vi "UNITEST MAIN v2.0.vi"() -> ()   [LabVIEW 2025]
uses:
  controls/LAB-IQ UI Data.ctl
  <vilib>/Platform/TimedLoop/XDataNode/timing_clust.ctl
  <vilib>/Platform/TimedLoop/XDataNode/nitl_modes.ctl
  <vilib>/Platform/TimedLoop/XDataNode/wakeup.ctl
  HEAVE vi's/Heave Write enum.ctl
  SWAY vi's/Sway Write enum.ctl
  SWAY vi's/Sway Right enum.ctl
  HEAVE vi's/Heave Right enum.ctl
  d081153b-36ca-4bc4-8478-749476f82ba4.vi
  1202965f-721d-4349-8d61-5de826f379ef.vi
  785ec975-e53d-4ed4-be48-2cc128d7a91f.vi
  02c5850b-52e8-4ed5-91f8-6f0ad62f4994.vi
  1223eb78-e4c4-4b69-bf80-185c82055158.vi
  e5651a45-6a49-4a3f-b503-ff1eaf449b4a.vi
  <vilib>/Utility/error.llb/Trim Whitespace One-Sided.vi
  support/Message Queue/Enqueue Message (Single).vi
  <vilib>/Utility/error.llb/Error Cluster From Error Code.vi
  <vilib>/Utility/file.llb/Read Delimited Spreadsheet (string).vi
  <vilib>/Utility/file.llb/Write Delimited Spreadsheet (string).vi
  <vilib>/ErrorRing/Error Ring.xnode
  <vilib>/platform/TimedLoop/XDataNode/XDataNode.xnode
  support/Message Queue/LAB-IQ Message Queue.lvlib
  support/User Event - Stop/LAB-IQ User Event - Stop.lvlib
  <vilib>/Platform/TimedLoop/XDataNode/XDNodeRunTimeDep.lvlib
panel:
  in  "DEPTH TRIP   ENABLE":bool
  in  "DEPTH TRIP VALUE":dbl
  in  "LOAD TRIP  ENABLE":bool
  in  "LOAD TRIP VALUE":dbl
  in  "CYCLIC COF TRIP  ENABLE":bool
  in  "CYCLIC FF TRIP  ENABLE":bool
  in  "FF TRIP  ENABLE":bool
  in  "COF TRIP  ENABLE":bool
  in  "CYCLIC CoF TRIP VALUE":dbl
  in  "CYCLIC FF TRIP VALUE":dbl
  in  "FF TRIP VALUE":dbl
  in  "COF TRIP VALUE":dbl
  in  "Dummy Run":bool
  in  "AutoTune":bool
  in  "reinit 3":bool=TRUE
  in  "output range delay":cluster{"output high":dbl, "output low":dbl}={"output high"=100.0, "output low"=-100.0} {"output low" format="%.2f"; "output high" format="%.2f"}
  in  "PID gains out delay":T1={"proportional gain (Kc)"=30.0, "integral time (Ti, min)"=0.00101, "derivative time (Td, min)"=0.0} {"derivative time (Td, min)" format="%.3f"; "integral time (Ti, min)" min=1e-05 max=100.0 step=0.0001 format="%.4f"; "proportional gain (Kc)" format="%.3f"}
  in  "PID gains out delay (microForce)":T1={"proportional gain (Kc)"=300.0, "integral time (Ti, min)"=0.00011, "derivative time (Td, min)"=0.0} {"derivative time (Td, min)" format="%.3f"; "integral time (Ti, min)" min=1e-05 max=100.0 step=1e-06 format="%.6f"; "proportional gain (Kc)" format="%.3f"}
  in  "Gain 2":dbl=0.016
  in  "Offset  3":dbl=1.5
  in  "Ramp MulFac":dbl=2.0
  out "actpid":dbl
  in  "pulses LoadDiffRamp(2..10)":dbl=9.0
  in  "PulseControlRamp(diff<=3N)":dbl=5.0 min=1.0 max=1000.0 step=1.0 format="%#.1f"
  in  "SetLoadDeadband(%) Load(0-10N)":dbl=0.1 min=0.0001 max=100.0 step=0.0001 format="%#.6f"
  in  "pulses LoadDiff(2..10)":dbl=10.0
  in  "pulses LoadDiff(11..50)":dbl=40.0
  in  "PulseControl(diff<=3N)":dbl=1.0 min=1.0 max=1000.0 step=1.0 format="%#.1f"
  out "SetLoadDeadband(%)  2":dbl=1.0 min=0.001 max=100.0 step=0.001 format="%#.6f"
  in  "pulsesSent":dbl=200.0
  out "pulses":dbl
  in  "pulses LoadDiff(21..1000)":dbl=40.0
  in  "Delay":dbl=1.5 min=0.001 max=5.0 step=0.001 format="%#.6f"
  in  "deadband":dbl=0.2
  in  "Checkbox 2":bool
  in  "Checkbox":bool=TRUE
  out "Scratch Start Recording":bool
  in  "SwaySpeed Set":bool
  in  "Update":bool
  in  "Analysis Home":bool
  in  "Installation/Replacement completed":bool
  in  "Loahead":bool
  in  "Heave and Surge COM Port:":refnum<visa-resource-name>="COM9"
  in  "Sway COM Port:":refnum<visa-resource-name>="COM10"
  out "Test Trip":bool
  out "Hymidity":bool
  in  "Humidity Disable trip":bool=TRUE
  in  "CoF Trip  2":dbl=540.0 min=100.0 max=540.0 step=1.0
  in  "File Path :  2":path
  out "Wear Track Diameter":dbl
  in  "Stribeck table":bool
  in  "seq":bool=TRUE
  out "Drive Error":string
  out "mm/s  Surge":dbl=7.0 caption="Jog" min=0.001 max=50.0 step=0.0001 format="%.2f"
  in  "Update Surge Speed":bool
  out "mm/s  Sway":dbl=7.0 caption="Jog" min=0.001 max=50.0 step=0.0001 format="%.2f"
  in  "Update Sway Speed":bool
  in  "Update Heave Speed":bool
  out "mm/s Heave":dbl=7.0 caption="Jog" min=0.001 max=30.0 step=0.0001 format="%.2f"
  in  "mm/sec":dbl=1.0 caption="Jog" min=0.001 max=50.0 step=0.001 format="%.2f"
  out "Scratch Start Test":bool
  in  "HomeScratch":bool
  in  "TEST SELECTION":enum32{"Time", "Cycle"}(radio)
  out "HEAVE ENABLE":bool
  in  "SPARE  5":u8
  in  "Manual Write SWAY":bool
  out "SWAY WRITE":string
  in  "SPARE  4":u8
  in  "SPARE  3":u8
  in  "SPARE 2":u8
  in  "SPARE 1":u8
  out "Spare 15":u8
  out "Spare 14":u8
  out "Spare 13":u8
  out "Spare 12":u8
  out "Spare 11":u8
  out "Spare 10":u8
  out "Spare 9":u8
  out "Spare 8":u8
  out "Spare 7":u8
  out "Spare 6":u8
  out "Spare 5":u8
  out "Spare 4":u8
  out "Spare 3":u8
  out "Spare 2":u8
  out "Spare 1":u8
  out "Node Id":u8
  out "Read SWAY Temp":bool
  out "fwMinor":u8
  out "fwMajor":u8
  out "faultCode":u16
  out "Rotary POSE":sgl format="%#.6f"
  out "SWAY POSE":sgl format="%#.6f"
  out "Homed":u8
  out "State":u8
  out "Ack ID":u16
  in  "SPEED":sgl=10000.0
  in  "Distance":sgl=10000.0
  in  "Mode Command":u8=2
  out "Sequence ID":u16
  out "error out Read SWAY":errorcluster
  out "error out Write  SWAY":errorcluster
  out "SWAY READ":string
  out "Start Test Temp":bool
  in  "AppLoadSeq scratch":bool
  in  "PID Delay (sec)":dbl=1.0 format="%#_6p"
  in  "Manual Write Heave & Surge":bool
  out "Heave and Surge Write":string
  in  "SPARE 4":u8
  in  "SPARE 3":u8
  in  "SPARE 2":u8
  in  "SPARE 1":u8
  out "Spare 15":u8
  out "Spare 14":u8
  out "Spare 13":u8
  out "Spare 12":u8
  out "Spare 11":u8
  out "Spare 10":u8
  out "Spare 9":u8
  out "Spare 8":u8
  out "Spare 7":u8
  out "Spare 6":u8
  out "Spare 5":u8
  out "Spare 4":u8
  out "Spare 3":u8
  out "Spare 2":u8
  out "Spare 1":u8
  out "Node Id":u8
  out "Read Heave Temp":bool
  out "fwMinor":u8
  out "fwMajor":u8
  out "faultCode":u16
  out "SURGE POSE":sgl format="%#.6f"
  out "HEAVE POSE":sgl format="%#.6f"
  out "Homed":u8
  out "State":u8
  out "Ack ID":u16
  in  "SPEED":sgl=10000.0
  in  "Distance":sgl=10000.0
  in  "Mode Command":u8=2
  out "Sequence ID":u16
  out "error out Read":errorcluster
  out "error out Write":errorcluster
  out "Heave and Surge Read":string
  out "Load Cell Temp":bool
  in  "Stop Scratch":bool
  in  "Enter Fixed SRR 2":dbl min=0.0 max=0.0 format="%.3f"
  in  "E.Velocity 2":bool=TRUE caption="SRR"
  in  "Tab Control 3":T2(tab)
  in  "Tab Control 5":enum32{""}(tab)
  in  "Tab Control 14":T3(tab)=enum."Motor Load"
  in  "Ramp":bool
  in  "apply load":bool
  in  "Enter ByPass Load":dbl
  in  "Bypass Load":bool
  out "gFF Rot 7":cluster{dbl, dbl, dbl}(graph)
  in  "Current Load":dbl
  in  "Set Load":dbl
  out "Current Position":dbl
  in  "Kp":dbl=1.0
  in  "Ki":dbl
  in  "Kd":dbl
  in  "Deadband":dbl=0.1
  in  "pct_scale":dbl=100.0
  in  "Init Step":dbl=10.0
  in  "Max Step Linit":dbl=10.0
  in  "i_limit":dbl=10.0
  in  "Min_pos_limit":dbl
  in  "Max_pos_limit":dbl=50000000.0
  in  "Fine Tune Zone":dbl=10.0
  in  "fine_tune_pct":dbl=100.0
  in  "min_deadband_floor":dbl=0.05
  in  "min_finetune_floor":dbl=0.15
  out "Pulse delta":dbl
  out "Vertical load (N)":dbl format="%#.3f"
  in  "Tab Control 26":enum32{"Page 1", "Page 2"}(tab)
  in  "ClearAll":bool
  out "Mz(Nm)":dbl[](array[numeric])
  out "My(Nm)":dbl[](array[numeric])
  out "Mx(Nm)":dbl[](array[numeric])
  in  "Save Dwell":dbl=0.015 caption="Save Dwell (sec)" min=0.0 max=5.0 step=0.001 format="%.3f"
  out "Mx":dbl[](graph)
  out "My":dbl[](graph)
  out "Mz":dbl[](graph)
  out "Fy(N)":dbl[](graph)
  out "Fz(N)":dbl[](graph)
  in  "ZeroAll":bool
  in  "Acq Delay (ms)":dbl=10.0
  in  "Burst Delay (ms)":dbl=10.0
  out "model":string
  out "SN":i32
  out "FFx(N)":dbl[](array[numeric])
  in  "Sensor IP":string="192.168.1.100"
  in  "Port":i32=8080
  out "FFy(N)":dbl[](array[numeric])
  out "Load(N)":dbl[](array[numeric])
  out "Fx(N)":dbl[](graph)
  out "AE":bool
  in  "delete Handle":bool
  in  "Create Handle":bool=TRUE
  out "ft_data":dbl[](array[numeric])=[1.0, 1.0, 1.0, 1.0, 1.0, 1.0]
  out "ft_range":dbl[](array[numeric])=[1.0, 1.0, 1.0, 1.0, 1.0, 1.0]
  in  "stop 6":bool
  out "running_flag":bool
  out "ft_udp_handle":i32
  out "get-data-return":i32
  out "get-range-return":i32
  out "zero-return":i32
  out "filter-return":i32
  out "initial-return":i32
  out "deleteHandle-result":i32
  in  "Tab Control 19":enum32{"Platform COM", "Config ", "DevInfo"}(tab)=enum."Config "
  in  "SAMPLES":dbl=100.0
  in  "Re-initilaize":bool
  in  "Filter ON/OFF":bool=TRUE
  in  "TracHomeSurgeOffsetCounts 10MM":dbl=505100.0
  in  "TracHomeSwayOffsetCounts 10MM":dbl=1432.0
  in  "Acoustic Emission:":dbl=1.0 min=0.0001 max=200.0 step=0.0001 format="%.4f"
  in  "Apply Filter (FF)":bool
  in  "Filter% 2":dbl=50.0 min=50.0 max=100.0 step=0.1 format="%.1f"
  in  "Apply Filter (Load)":bool=TRUE
  in  "Filter%":dbl=80.0 min=50.0 max=100.0 step=0.1 format="%.1f"
  in  "Sway distance (mm)":dbl=245.0
  in  "Surge distance (mm)":dbl=370.0
  in  "DataSavingLoopDelay(ms)":dbl=15.0
  in  "SAVE  2":bool
  in  "Enter Distance":bool caption="Enter Counts"
  in  "Sway Counts:":dbl=100.0 min=0.0 max=100000000.0 step=1.0 format="%.2f"
  in  "Distance (mm): 3":dbl=100.0 caption="Distance (mm):" min=0.0 max=1500.0 step=0.001 format="%.5f"
  in  "Surge Counts:":dbl=100.0 min=0.0 max=100000000.0 step=1.0 format="%.1f"
  in  "Distance (mm): 2":dbl=100.0 caption="Distance (mm):" min=0.0 max=1500.0 step=0.0001 format="%.3f"
  in  "Distance (mm):":dbl=100.0 min=0.0 max=1500.0 step=0.001 format="%.5f"
  in  "Heave Counts:":dbl=100.0 min=0.0 max=100000000.0 step=1.0
  in  "LRMHomeSurgeOffsetCounts":dbl=307197.0
  in  "LRMHomeSwayOffsetCounts":dbl=26880.0
  in  "TracHomeSurgeOffsetCounts 20MM":dbl=505100.0
  in  "TracHomeSwayOffsetCounts 20MM":dbl=1432.0
  in  "RotHomeSwayOffsetCounts":dbl=14656.0
  in  "RotHomeSurgeOffsetCounts":dbl=311465.0
  in  "Heave distance":dbl=340.0
  out "Zmm":dbl=1600.0
  out "Heave Pulses/mm":dbl=1600.0
  out "Surge Pulses/mm":dbl=1600.0
  out "Sway Pulses/mm":dbl=320.0
  in  "Heave Pitch":dbl=4.0
  in  "Surge Pitch":dbl=3.0
  in  "Sway Pitch":dbl=2.0
  in  "Heave PPR":dbl=6400.0
  in  "Surge PPR":dbl=6400.0
  in  "Sway PPR":dbl=6400.0
  in  "Heave Jog Speed":dbl=15.0
  in  "Surge Jog Speed":dbl=1.0 format="%.4f"
  in  "Heave PID Speed":dbl=15.0
  in  "Heave Loop Delay":dbl
  in  "Sway Jog Speed":dbl=1.0 format="%.4f"
  in  "Sway PID Speed":dbl=1.0 format="%.4f"
  in  "Sway Loop Delay":dbl
  in  "GUI":T4(tab)
  in  "Platform Settings":bool caption="Password"
  in  "Configure":bool caption="Password"
  in  "Home":bool caption="Password"
  in  "EXIT":bool
  in  "Analysis":bool caption="Password"
  in  "service 2":bool caption="Password"
  in  "MainPage":T5(tab)=enum."HOME"
  in  "Select Load Head":bool
  in  "Notes :":string
  in  "FILE":string
  in  "Sample ID :":string
  in  "Operator ID :":string
  in  "Operator Name :":string
  in  "Auto":bool caption="Power Status"
  in  "Disable Axis Jog Soft Limits m":bool
  out "Sway and Surge COM Status":bool=TRUE caption="Load COM Status"
  out "Heave COM Status":bool=TRUE caption="Load COM Status"
  in  "Enable Platform":bool
  in  "Surge Forward Main":bool
  in  "Surge Backward Main":bool
  in  "Sway Right Main":bool
  in  "Sway Left Main":bool
  in  "Heave Down Main":bool
  in  "Heave Up main":bool
  in  "mm":dbl=0.001 caption="Jog" min=1.0 max=100.0 step=0.01 format="%#.3f"
  in  "Surface Analysis":bool
  in  "Imaging":bool
  in  "Image Analysis":bool
  in  "Post Analysis":bool
  in  "SSP 0.75":bool
  in  "SSP 0.5":bool
  in  "SSP 0.3":bool
  in  "Warning":enum32{"Page 2"}(tab)
  in  "gui GIF":enum32{"Check", "Deca", "kilo", "Micro"}(tab)
  out "Communication is established":bool=TRUE caption="Load COM Status"
  in  "Reference Sample":u16(ring) items=["None", "Brass", "Aluminium", "Mild Steel"]
  out "Load Cell Communication Slide":u8(slide)=1 min=1 max=10 step=1 scale=0.0..10.0
  in  "com 3":bool
  out "com":bool
  out "DecaForce COM Status":bool caption="Load COM Status"
  in  "Loading Mode":u16(ring) items=["Constant", "Ramp", "Steps", "Indentation"]
  in  "Enter the CoF Trip":dbl=1.0
  in  "Enter the Friction Force Trip":dbl=520.0 min=500.0 max=500.0 step=1.0 format="%#.1f"
  in  "Enter the Normal load Trip":dbl=520.0 min=500.0 max=500.0 step=0.001 format="%.3f"
  in  "KiloForce":bool
  in  "DecaForce":bool
  in  "MicroForce":bool
  in  "LHBack":bool
  in  "LHNext":bool
  in  "Load Selection":T6(tab)
  in  "Enter the Load  (N)":dbl=2.0 caption="Enter the Load (N)" min=2.0 max=200.0 step=0.1 format="%#.4f"
  in  "Enter the Final Load (N)":dbl=1.0 min=0.0 max=500.0 step=1.0 format="%#.0f"
  in  "Enter the Loading Rate (N/min)":dbl=60.0 min=1.0 max=1200.0 step=0.1 format="%.2f"
  out "Warning 2":bool
  in  "Stribeck Table  For loading":string[][](table)
  in  "Clear 3":bool
  out "Message":string="Load Entered is out of range!!!"
  in  "Indentation":string[][](table)=[["Detection", "5", "2"], ["Unload", "0", "5"], ["Load", "10", "2"], ["Unload", "0", "5"], ["Detection", "5", "2"], ["Unload", "0", "5"]]
  in  "Multipoint":bool caption="Singlepoint"
  in  "AppLoad 4":bool
  in  "zNL":bool
  out "NL disp":dbl caption="Normal Load ( N )" min=-2000.0 max=2000.0 step=0.0001 format="%.1f"
  in  "Traction":bool
  in  "Surge Forward MM":bool
  in  "Surge Backward MM":bool
  in  "M3 Image":enum32{"Page 1", "Page 2"}(tab)
  in  "String 39":string="Jog heave to bring the upper sample closer to the lower sample within 1mm."
  in  "Sway Left MM":bool
  in  "Sway Right MM":bool
  in  "Disable Axis Jog Soft Limits":bool
  in  "mm":dbl=0.001 caption="Jog" min=0.001 max=5.0 step=0.0001 format="%#.3f"
  in  "Heave Down MM":bool
  in  "Heave Up MM":bool
  in  "Wear Track Diameter (mm)":dbl=30.0 caption="Wear Track Diameter (mm):" min=1.0 max=30.0 step=1.0 format="%.2f"
  in  "Set WTD":bool
  in  "HomeScratch":bool
  in  "HomeRot":bool
  in  "PlaceModule":bool
  in  "Motion Mode:":u16(ring) items=["Uniform Rotation", "Angular Oscillation", "Stribeck ", "Steps"]
  in  "LR Sway":bool
  in  "Rot Hor":bool
  in  "Rot Ver":bool
  in  "Scratch":bool
  in  "LR Cam":bool
  in  "MMBack":bool
  in  "MMNext":bool
  in  "Rotary Module Selection":T7(tab)
  in  "SPEED SELECTION :":enum32{"Speed in RPM", "Speed in m/sec"}(radio)=enum."Speed in m/sec"
  in  "Enter the Speed(mm/sec)":dbl=0.1 min=0.1 max=10.0 step=0.1 format="%.3f"
  in  "Enter the Speed (RPM)":dbl=45.0 min=1.0 max=3000.0 step=1.0
  in  "Enter the Frequency (Hz)":dbl=1.0 min=0.1 max=10.0 step=0.1 format="%.1f"
  in  "Enter the Angle (Deg)":dbl=45.0 min=5.0 max=300.0 step=1.0
  in  "Angular Oscillation Set":bool
  in  "Rotary Tab":enum32{"Page 1", "Page 2"}(tab)
  out "e.v/ssr 2":enum32{"E.V", "SSR"}(tab)
  in  "Enter the Final E.Velocity (m/s) 2":dbl=1.0 min=0.001 max=4.0 step=0.001 format="%.3f"
  in  "Enter initial E.Velocity (m/s) 2":dbl=2.0 min=0.001 max=4.0 step=0.001 format="%.3f"
  in  "Enter Fixed E.Velocity 2":dbl=1.0 min=0.001 max=2.0 step=0.001 format="%.3f"
  in  "Enter Final SRR 2":dbl=1.0 min=0.001 max=1.0 step=0.001 format="%.2f"
  in  "Enter initial SRR 2":dbl=1.0 min=0.001 max=1.0 step=0.001 format="%.2f"
  out "Final Speed (RPM) 3":dbl=1.0 min=0.1 max=3000.0 step=0.1 format="%.1f"
  out "Initial Speed (RPM) 2":dbl=100.0 min=0.1 max=3000.0 step=0.1 format="%.1f"
  in  "Enter the Final Velocity (m/s) 3":dbl=1.0 min=0.001 max=2.0 step=0.001 format="%.3f"
  in  "Enter initial Velocity (m/s)  3":dbl=2.0 min=0.001 max=2.0 step=0.001 format="%.3f"
  out "Ramp Up 2":bool caption="Ramp Down"
  in  "Import 2":bool
  in  "Save 2":bool
  in  "SPEED SELECTION : rotary":enum32{"Speed in Rpm", "Speed in m/sec"}(radio)=enum."Speed in m/sec"
  in  "calculate rotary":bool
  in  "String 45":string="File Path Location : C:-->LAB-IQ 150 --> User Defined\n                                       Protocol-->File.txt"
  in  "Step Speed":enum32{"Step Speed", "Step (load-Speed)"}(tab)
  in  "StepTable For Speed":string[][](table)
  in  "StepTable For Load-Speed":string[][](table)=[["", "", ""], ["", "", ""], ["", "", ""], ["", "", ""]]
  in  "StepTable For Speed 3":string[][](table)=[["", "", ""], ["", "", ""], ["", "", ""], ["", "", ""]]
  in  "Motion Direction:  3":u16(ring) items=["Clockwise", "Counter Clockwise"]
  in  "Enter Scratch length (mm):":dbl=1.0 min=1.0 max=50.0 step=0.0001 format="%.4f"
  in  "Enter Scratch Speed (mm/s):":dbl=1.0 min=0.003 max=10.0 step=0.0031 format="%.5f"
  in  "Scartch Offset":dbl=1.0 caption="Scratch Offset: (mm)" min=0.1 max=5.0 step=0.1 format="%.1f"
  in  "Motion type:":u16(ring) items=["Unidirection", "Bidirection"]
  in  "Scratch Mode":u16(ring) items=["Scratch", "Pre-Post Scan", "Multi Scratch"]
  in  "Rotary Speed Exced":string="Motor Speed Out of Range"
  in  "No of Scratch":dbl=1.0 min=1.0 max=50.0 step=0.0001
  out "Humidity  Status  3":bool caption="Communication Status"
  out "Low Temp  Status  2":bool=TRUE caption="Communication Status"
  out "TK4 status 2":bool=TRUE caption="Communication Status"
  in  "String 40":string="Before selecting Acoustic make sure the sensor output pin is connected to A4."
  in  "Stage Temperature":dbl[](array[numeric])=[150.0, 230.0, 300.0, 350.0, 400.0, 450.0, 500.0]
  in  "Sample Temperature":dbl[](array[numeric])=[100.0, 150.0, 200.0, 250.0, 300.0, 350.0, 400.0]
  in  "Humidity (Amb)":bool
  in  "Clear List":bool
  out "Sensors Picked":string
  in  "Add to list":bool
  in  "Wear":bool
  in  "Vibration":bool
  in  "Humidity (Chamber)":bool
  in  "Temperature (Chamber)":bool
  in  "ECR":bool
  in  "Temperature (Amb)":bool
  in  "Microphone":bool
  in  "Acoustic Emission 3":bool
  in  "SNext":bool
  in  "APBack":bool
  in  "Enter the Temperature (°C):":dbl
  in  "Enter the Stage \nTemperature (°C):":dbl=20.0 min=20.0 max=150.0 step=1.0 format="%#.0f"
  in  "Enter the Humidity (%Rh):":dbl=30.0 min=30.0 max=85.0 step=1.0
  in  "Low Temp":bool
  in  "High Temp":bool
  in  "Humidity":bool
  in  "Main Screen Tab":T8(tab)
  in  "ClrLog":bool
  out "Trip Log":string
  in  "Start Test":bool
  out "Test status":bool caption="Test Status"
  out "AR Led":bool caption="AR"
  out "Data":bool=TRUE
  out "Health":bool=TRUE
  out "Sway COM Status":bool=TRUE caption="Load COM Status"
  out "Heave COM Status":bool=TRUE caption="Load COM Status"
  in  "Grp Tab":enum32{"Rot/LRM", "FBT"}(tab)
  out "Depth Trip":dbl=600.0
  in  "Depth Trip":bool=TRUE
  out "Weart Deapth":bool
  in  "Depth Reset Graph":bool
  out "Weart":bool
  in  "Depthz":bool
  out "Depth (µm)":dbl min=-200.0 max=200.0 step=0.1 format="%.1f"
  out "WearGp":dbl(graph)=0.13298760003255525
  out "NL Trip 2":dbl=600.0
  out "Load pid":bool
  in  "Load Disable Trip":bool=TRUE
  in  "Load Reset Graph":bool
  out "NL Display 4":dbl caption="Normal Load ( N )" min=-2000.0 max=2000.0 step=0.0001 format="%.1f"
  out "Main Chart 3":cluster{dbl, "NL disp":dbl, dbl}(graph)
  in  "FF Tab":T9(tab)
  in  "COF Reset Graph":bool
  in  "COF Disable Trip":bool=TRUE
  out "COF TRIP":dbl=600.0
  out "Coefficient of Friction":dbl(graph)=0.13298760003255525
  in  "zFF":bool
  in  "FF Reset Graph":bool
  in  "FF Disable Trip":bool=TRUE
  out "FF TRIP":dbl=600.0
  out "Friction Force (N)":dbl min=-2000.0 max=2000.0 step=0.0001 format="%.3f"
  out "Friction Force (N) Graph":dbl(graph)=0.13298760003255525
  out "Cyclic FF TRIP":dbl=600.0
  in  "Cyclic FF Disable Trip":bool=TRUE
  in  "Cyclic FF Reset Graph":bool
  in  "CZ FF":bool
  out "Cyclic Friction Force (N) Graph":dbl(graph)=0.13298760003255525
  out "Cyclic Friction Force (N)":dbl min=-2000.0 max=2000.0 step=0.0001 format="%.3f"
  out "cyclic COF TRIP":dbl=600.0
  in  "cyclic COF Disable Trip":bool=TRUE
  in  "cyclic COF Reset Graph":bool
  out "Cyclic Coefficient of Friction":dbl(graph)=0.13298760003255525
  in  "Sub Graph":T10(tab)
  in  "Speed Tab":enum32{" Rotary Disc", "MTM Ball", "MTM Disc"}(tab)
  out "speed mm/sec":dbl(graph)=0.13298760003255525
  in  "Speed Reset Graph":bool
  out "MTM BALL SPEED":dbl(graph)=0.13298760003255525
  out "MTM DISC  SPEED":dbl(graph)=0.13298760003255525
  in  "Temperature Reset":bool
  out "Temperature (deg c)":dbl(graph)=0.13298760003255525
  in  "ECR RESET":bool
  out "ECR":dbl(graph)=0.13298760003255525
  out "Acoustic Emission (mV)":dbl min=0.0 max=5000.0 step=0.1
  in  "Aqucostic Reset Graph":bool
  out "gACQUOS":dbl(graph)=0.13298760003255525
  in  "Humidity Reset Graph":bool
  out "HumrGp":dbl(graph)=0.13298760003255525
  out "SD (mm)":dbl caption="Sliding Distance ( mm )" min=-200.0 max=200.0 step=0.1 format="%.4f"
  in  "Siliding distance Reset Graph":bool
  out "SDGp":dbl(graph)=0.13298760003255525
  in  "BACK":bool
  out "Ambient \nTemperature":dbl min=0.0 max=5000.0 step=0.1 format="%.1f"
  out "Ambient\n Humidity":dbl min=0.0 max=5000.0 step=0.1 format="%.2f"
  out "NL disp 2":dbl caption="Normal Load ( N )" min=-2000.0 max=2000.0 step=0.0001 format="%.1f"
  out "Set Humidity":dbl caption="Set Humidity  (% Rh)" min=-2000.0 max=2000.0 step=1.0 format="%.1f"
  out "humidity disp":dbl caption="Humidity (% Rh)" min=-2000.0 max=2000.0 step=1.0 format="%.1f"
  in  "Humidity On":bool
  in  "zNL 2":bool
  out "NLt":bool
  in  "Load En":bool
  out "Freq (Hz)":dbl min=0.0 max=5000.0 step=0.1 format="%.4f"
  out "HumCOMStatus":bool caption="Communication Status"
  out "Load Communication":bool
  in  "Temp Tabs":enum32{"Low Temp", "High Temp"}(tab)=enum."High Temp"
  out "Controller  Status":bool
  out "ChamberTemp":dbl format="%#.1f"
  in  "SetTmp":dbl=-190.0 caption="Set Temperature (Deg C)" min=-190.0 max=100.0 step=1.0 format="%.1f"
  in  "Cooling":bool
  in  "Heater":bool
  out "TK4 status":bool caption="Controller  Status"
  out "ChamberTemp":dbl format="%#.1f"
  in  "SetTmp":dbl caption="Set Temperature (Deg C)" min=0.0 max=1000.0 step=1.0 format="%.1f"
  in  "Set Load (N)":dbl=100.0 min=0.01 max=1500.0 step=0.01 format="%.1f"
  in  "Time Tab":enum32{"cycles", "duration"}(tab)=enum."duration"
  out "Test Duration 4":dbl=600.0 caption="Test Duration\n(HH:MM:SS)" min=0.0083 max=180000.0 step=0.0001 format="%<%H:%M:%S>t"
  out "TEST CYCLE":dbl min=0.0 max=5000.0 step=0.01 format="%.2f"
  in  "TOTAL CYCLES":dbl min=0.0 max=5000.0 step=0.1 format="%.4f"
  out "Time ( HH:MM:SS ) 2":dbl min=0.0 max=144000.0 step=1.0 format="%<%H:%M:%S>t"
  in  "Test Duration":dbl=600.0 caption="Test Duration\n(HH:MM:SS)" min=0.0083 max=180000.0 step=0.0001 format="%<%H:%M:%S>t"
  in  "Main Speed Tab":enum32{"ROTARY", "TRACTION"}(tab)
  in  "SPEED TAB":enum32{"RPM", "m/sec"}(tab)
  out "Speed (RPM)":dbl min=0.0 max=5000.0 step=0.1 format="%.1f"
  out "Set Speed":dbl caption="Set Speed (RPM)" min=0.0 max=1500.0 step=0.1 format="%.1f"
  out "Speed (m/sec)":dbl min=0.0 max=5000.0 step=0.001 format="%.4f"
  out "Set Speed (m/sec)":dbl min=0.0 max=1500.0 step=0.001 format="%.4f"
  in  "MTM MOTOR DISPLAY":enum32{"MTM RPM", "MTM m/sec"}(tab)
  out "Disc Speed (RPM)":dbl min=0.0 max=1500.0 step=0.1 format="%.1f"
  out "Ball Speed (RPM)":dbl min=0.0 max=1500.0 step=0.1 format="%.1f"
  out "Disc Speed (m/sec)":dbl min=0.0 max=1500.0 step=0.1 format="%.1f"
  out "Ball Speed (m/sec)":dbl min=0.0 max=1500.0 step=0.1 format="%.1f"
  in  "Angle and Frequency":enum32{"angular", "lrm"}(tab)
  out "Angle (Deg)":dbl min=0.0 max=5000.0 step=0.01 format="%.2f"
  out "Stroke (mm)":dbl min=0.0 max=5000.0 step=0.01 format="%.2f"
  in  "STOP":bool
  out "Multi Scratch Pass":dbl min=0.0 max=5000.0 step=0.1
  in  "X-AXIS":u16(ring) items=["None", "Time ( Sec )", "Normal Load ( N )", "Frictional Force ( N )", "Coefficient of Friction", "Depth ( Microns )", "Speed ( RPM )", "Frequency ( Hz )", "Angle ( Degree )", "Cyclic Friction Force ( N )", "Cyclic Co efficient Friction ", "Stage temperature ( Degree celcius )", "Sample temperature ( Degree celcius )", "Stroke Length ( mm )", "Scratch Speed ( mm/sec )", "Amb Humidity ( % Rh ) ", "Amb Temperature (Deg C)", "Acoustic (mV)", "Mx (Nm)", "My (Nm)", "Mz (Nm)", "Humidity ( % Rh )", "Sliding Distance (mm)", "Wear Track Diameter (mm)", "Fx(N)", "Fy(N)", "MTM BallSpeed (RPM)", "MTM DiscSpeed (RPM)", "Entrainment Speed", "Slide Role", "Slip(%)", "Rotary Speed (m/sec)", "MTM Ball Speed (m/sec)", "MTM Disc Speed (m/sec)", "ECR (ohms)"]
  in  "Y-AXIS":u16(ring) items=["None", "Time ( Sec )", "Normal Load ( N )", "Frictional Force ( N )", "Coefficient of Friction", "Depth ( Microns )", "Speed ( RPM )", "Frequency ( Hz )", "Angle ( Degree )", "Cyclic Friction Force ( N )", "Cyclic Co efficient Friction ", "Stage temperature ( Degree celcius )", "Sample temperature ( Degree celcius )", "Stroke Length ( mm )", "Scratch Speed ( mm/sec )", "Amb Humidity ( % Rh ) ", "Amb Temperature (Deg C)", "Acoustic (mV)", "Mx (Nm)", "My (Nm)", "Mz (Nm)", "Humidity ( % Rh )", "Sliding Distance (mm)", "Wear Track Diameter (mm)", "Fx(N)", "Fy(N)", "MTM BallSpeed (RPM)", "MTM DiscSpeed (RPM)", "Entrainment Speed", "Slide Role", "Slip(%)", "Rotary Speed (m/sec)", "MTM Ball Speed (m/sec)", "MTM Disc Speed (m/sec)", "ECR (ohms)"]
  out "XY Graph":cluster{"Array 2":dbl[], "Array 2":dbl[]}[](graph) caption="XY Graph 20"
  out "VARIANCE":dbl=-0.0 format="%0.2f"
  out "SD":dbl=-0.0 format="%.3f"
  out "MEAN":dbl format="%.3f"
  out "VARIANCE":dbl=-0.0 format="%0.2f"
  out "SD":dbl=-0.0 format="%.3f"
  out "MEAN":dbl format="%.3f"
  out "VARIANCE":dbl=-0.0 format="%0.2f"
  out "SD":dbl=-0.0 format="%.3f"
  out "MEAN":dbl format="%.3f"
  out "VARIANCE":dbl=-0.0 format="%0.2f"
  out "SD":dbl=-0.0 format="%.3f"
  out "MEAN":dbl format="%.3f"
  in  "Analysis Home new":bool
  out "File 2 Discription":string="\r"
  out "File 1 Discription":string="\r"
  in  "OPEN 1":bool
  in  "OPEN 2":bool
  out "File Name 1":string
  out "File Name 2":string
  in  "Refresh 2":bool
  in  "OPEN 3":bool
  out "File Name 3":string
  out "File Name 4":string
  in  "OPEN 4":bool
  out "File 4 Discription":string="\r"
  out "File 3 Discription":string="\r"
  in  "File Format":u16(ring) items=["csv", "txt", "duf"]
  in  "Export":bool
  in  "Report":bool
  in  "Password":string
  in  "Home Service":bool
  in  "Advanced Setting":bool
  in  "About Tab":enum32{"Primary"}(tab)
  in  "ECR Port:":refnum<visa-resource-name>="COM10"
  in  "Ramp Port:":refnum<visa-resource-name>="COM10"
  in  "Temp Modbus:":refnum<visa-resource-name>="COM14"
  in  "Humidity Port:":refnum<visa-resource-name>="COM10"
  in  "Edit Gain Constants":bool
  in  "Save Gain Constants":bool
  in  "Service About":bool
  # "SET JOG SPEED"
  # "Speed Exceed the limit of the Motor"
  # "Motor Speed Out of Range"
  # "NOTE: This operation needs to be done only when the machine is ON."
  # "load Aquisition off"
  # "load Aquisition On"
  # "Configuration"
  # "Limits for Heave Surge and Sway"
  # "Modules Offset Parameters"
  # "Counts-Distance Calculator"
  # "File Name :"
  # "Ensure the traction module is aligned\n horizontally with the stage before ENABLE."
  # "JOG MODE"
  # "Module Selection"
  # "Positioning Control"
  # "Connect the controller\ncable to M3"
  # "Environment"
  # "Sensors"
  # "Data Points"
  # "Data Points"
  # "Data Points"
  # "Data Points"
  # "ohms"
  # "Data Points"
  # "Data Points"
  # "Data Points"
  # "LAB-IQ 150 / UNITEST / WO2456 / UT150  v05 / AUGUST 2025"
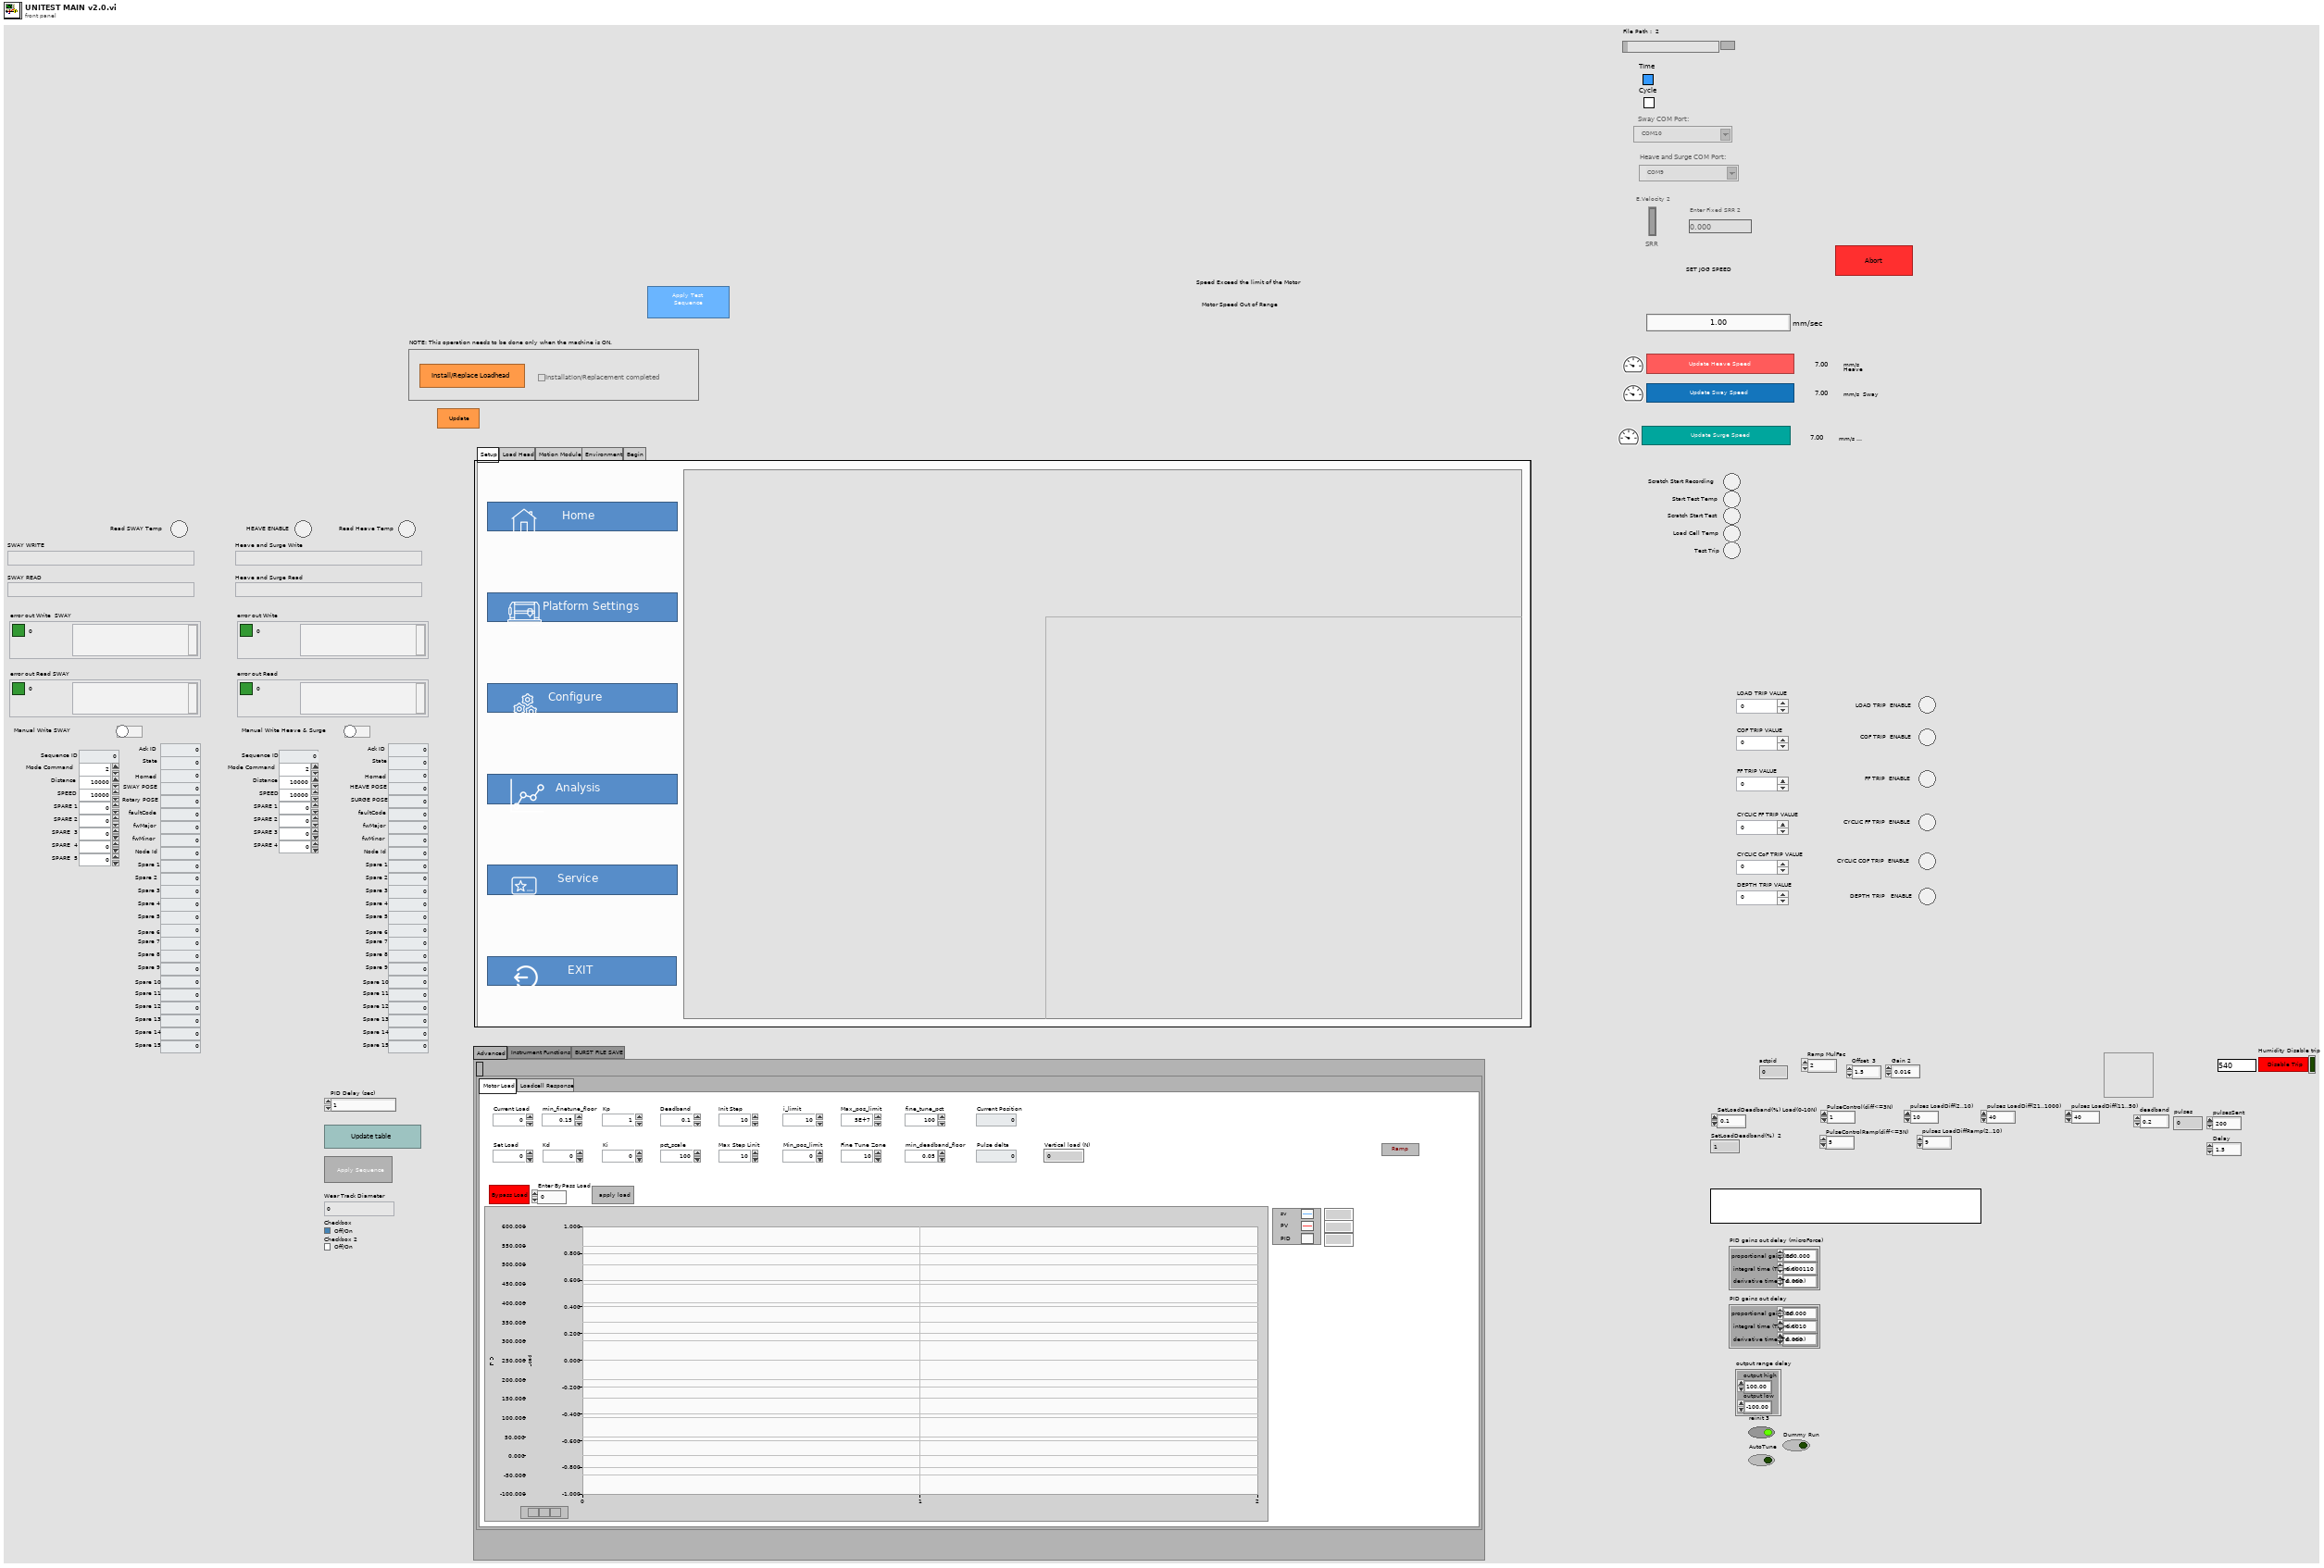
[diagram p1: front panel]
types:
  T1 = cluster{"proportional gain (Kc)":dbl, "integral time (Ti, min)":dbl, "derivative time (Td, min)":dbl}
  T2 = enum32{"Advanced", "Motor", "Depth_graph", "UIO Communicator", "Add to list parametrs", "Instrument Functions", "BURST FILE SAVE"}
  T3 = enum32{"LRM heating", "FBT_Heating", "Motor Load", "Loadcell Response", "Voice Load", "Step loading and speed ", "Depth"}
  T4 = enum32{"Setup", "Load Head", "Motion Module", "Environment", "Begin"}
  T5 = enum32{"Details", "PlatformSetting", "Analysis", "HOME"}
  T6 = enum32{"Constant", "Ramp", "Step", "Indentation"}
  T7 = enum32{"Uniform Rotation", "Angular Oscillation", "Speed Ramp", "Speed Step"}
  T8 = enum32{"  Acquire  ", "Compare Files Rot", "About", "Service"}
  T9 = enum32{"Coefficient of Friction ", "Friction Force (N)", "Cyclic Friction Force (N)", "Cyclic Coefficient of Friction "}
  T10 = enum32{"Speed", "Temperature", "ECR", "Acoustic Emission", "Humidity", "Sliding Distance"}
  T11 = typedef "LAB-IQ UI Data.ctl" = cluster{"Main Home Screen":cluster{"GUI":refnum<vi>, "Platform Settings":refnum<vi>, "Configure":refnum<vi>, "Home":refnum<vi>, "EXIT":refnum<vi>, "service 2":refnum<vi>, "MainPage":refnum<vi>, "Analysis":refnum<vi>}, "Platform Settings":cluster{"mm/s  Surge":refnum<vi>, "Update Surge Speed":refnum<vi>, "Drive Error":refnum<vi>, "Disable Axis Jog Soft Limits":refnum<vi>, "mm/s  Sway":refnum<vi>, "Sway and Surge COM Status":refnum<vi>, "Heave COM Status":refnum<vi>, "Enable Platform":refnum<vi>, "Surge Forward Main":refnum<vi>, "Sway Right Main":refnum<vi>, "Sway Left Main":refnum<vi>, "Heave Down Main":refnum<vi>, "Heave Up main":refnum<vi>, "Update Sway Speed":refnum<vi>, "Update Heave Speed":refnum<vi>, "mm/s Heave":refnum<vi>, "mm/sec":refnum<vi>, "mm":refnum<vi>, "Surge Backward Main":refnum<vi>}, "Analysis Screen":cluster{"Analysis Home":refnum<vi>, "Surface Analysis":refnum<vi>, "Imaging":refnum<vi>, "Image Analysis":refnum<vi>, "Post Analysis":refnum<vi>}, "Config Screen":cluster{"Select Load Head":refnum<vi>, "Notes :":refnum<vi>, "FILE":refnum<vi>, "Sample ID :":refnum<vi>, "Operator ID :":refnum<vi>, "Operator Name :":refnum<vi>, "Auto":refnum<vi>}, "Motion Module":cluster{"zNL":refnum<vi>, "NL disp":refnum<vi>, "Rotary Tab":refnum<vi>, "Motion Direction:  3":refnum<vi>, "E.Velocity 2":refnum<vi>, "e.v/ssr 2":refnum<vi>, "Enter Fixed E.Velocity 2":refnum<vi>, "Enter Final SRR 2":refnum<vi>, "Enter initial SRR 2":refnum<vi>, "Enter Fixed SRR 2":refnum<vi>, "Enter the Final E.Velocity (m/s) 2":refnum<vi>, "Enter initial E.Velocity (m/s) 2":refnum<vi>, "Final Speed (RPM) 3":refnum<vi>, "Initial Speed (RPM) 2":refnum<vi>, "Enter the Final Velocity (m/s) 3":refnum<vi>, "Enter initial Velocity (m/s)  3":refnum<vi>, "Ramp Up 2":refnum<vi>, "TEST SELECTION":refnum<vi>, "SPEED SELECTION : ":refnum<vi>, "Angular Oscillation Set":refnum<vi>, "Traction":refnum<vi>, "Step Speed":refnum<vi>, "StepTable For Load-Speed":refnum<vi>, "StepTable For Speed":refnum<vi>, "Surge Forward MM":refnum<vi>, "Surge Backward MM":refnum<vi>, "M3 Image":refnum<vi>, "String 39":refnum<vi>, "Sway Left MM":refnum<vi>, "Sway Right MM":refnum<vi>, "Disable Axis Jog Soft Limits":refnum<vi>, "mm":refnum<vi>, "Heave Down MM":refnum<vi>, "Heave Up MM":refnum<vi>, "Wear Track Diameter (mm)":refnum<vi>, "Set WTD":refnum<vi>, "HomeScratch":refnum<vi>, "HomeRot":refnum<vi>, "PlaceModule":refnum<vi>, "Enter the Angle (Deg)":refnum<vi>, "Enter the Frequency (Hz)":refnum<vi>, "Motion Mode:":refnum<vi>, "LR Sway":refnum<vi>, "Rot Hor":refnum<vi>, "Scratch":refnum<vi>, "LR Cam":refnum<vi>, "MMBack":refnum<vi>, "MMNext":refnum<vi>, "Rot Ver":refnum<vi>, "Rotary Module Selection":refnum<vi>, "calculate rotary":refnum<vi>, "SPEED SELECTION : rotary":refnum<vi>, "Import 2":refnum<vi>, "Save 2":refnum<vi>, "File Path :  2":refnum<vi>, "String 45":refnum<vi>, "StepTable For Speed 3":refnum<vi>, "Enter the Speed(mm/sec)":refnum<vi>, "Enter the Speed(RPM)":refnum<vi>, "Enter Scratch Speed (mm/s):":refnum<vi>, "SwaySpeed Set":refnum<vi>, "Scartch Offset":refnum<vi>, "Motion type:":refnum<vi>, "HomeScratch 2":refnum<vi>, "Enter Scratch length (mm):":refnum<vi>, "Wear Track Diameter":refnum<vi>, "Rotary Speed Exced":refnum<vi>, "Scratch Mode":refnum<vi>, "No of Scratch":refnum<vi>}, "Environmental control":cluster{"Humidity  Status  3":refnum<vi>, "Low Temp  Status  2":refnum<vi>, "TK4 status 2":refnum<vi>, "Stage Temperature":refnum<vi>, "Sample Temperature":refnum<vi>, "Humidity (Amb)":refnum<vi>, "Clear List":refnum<vi>, "Add to list":refnum<vi>, "Wear":refnum<vi>, "Vibration":refnum<vi>, "Humidity (Chamber)":refnum<vi>, "Temperature (Chamber)":refnum<vi>, "ECR ":refnum<vi>, "Temperature (Amb)":refnum<vi>, "Microphone":refnum<vi>, "Acoustic Emission 3":refnum<vi>, "SNext":refnum<vi>, "APBack":refnum<vi>, "Enter the Temperature (°C):":refnum<vi>, "Enter the Stage \nTemperature (°C):":refnum<vi>, "Enter the Humidity (%Rh):":refnum<vi>, "Low Temp":refnum<vi>, "High Temp":refnum<vi>, "Humidity":refnum<vi>, "Sensors Picked":refnum<vi>}, "About Screen":cluster{"Password":refnum<vi>, "Home Service":refnum<vi>, "Advanced Setting":refnum<vi>, "About Tab":refnum<vi>, "ECR Port:":refnum<vi>, "Ramp Port:":refnum<vi>, "Installation/Replacement completed":refnum<vi>, "Loahead":refnum<vi>, "Heave and Surge COM Port:":refnum<vi>, "Sway COM Port:":refnum<vi>, "Temp Modbus:":refnum<vi>, "Humidity Port:":refnum<vi>, "Edit Gain Constants":refnum<vi>, "Save Gain Constants":refnum<vi>}, "Main Screen":cluster{"Main Screen Tab":refnum<vi>, "Angle and Frequency":refnum<vi>, "Stroke (mm)":refnum<vi>, "Angle (Deg)":refnum<vi>, "Main Speed Tab":refnum<vi>, "MTM MOTOR DISPLAY":refnum<vi>, "Disc Speed (m/sec)":refnum<vi>, "Ball Speed (m/sec)":refnum<vi>, "Disc Speed (RPM)":refnum<vi>, "Ball Speed (RPM)":refnum<vi>, "SPEED TAB":refnum<vi>, "Speed (m/sec)":refnum<vi>, "Set Speed (m/sec)":refnum<vi>, "Speed (RPM)":refnum<vi>, "Set Speed":refnum<vi>, "Time Tab":refnum<vi>, "Time ( HH:MM:SS ) 2":refnum<vi>, "Test Duration":refnum<vi>, "Test Duration 4":refnum<vi>, "TEST CYCLE":refnum<vi>, "TOTAL CYCLES":refnum<vi>, "Set Load (N)":refnum<vi>, "Temp Tabs":refnum<vi>, "Heater":refnum<vi>, "TK4 status":refnum<vi>, "ChamberTemp":refnum<vi>, "SetTmp":refnum<vi>, "Controller  Status":refnum<vi>, "ChamberTemp 2":refnum<vi>, "SetTmp 2":refnum<vi>, "Controller  Status 2":refnum<vi>, "ChamberTemp 3":refnum<vi>, "SetTmp 3":refnum<vi>, "Cooling":refnum<vi>, "Load Communication":refnum<vi>, "Ambient \nTemperature":refnum<vi>, "HumCOMStatus":refnum<vi>, "Ambient\n Humidity":refnum<vi>, "Freq (Hz)":refnum<vi>, "Load En":refnum<vi>, "NLt":refnum<vi>, "zNL 2":refnum<vi>, "Humidity On":refnum<vi>, "humidity disp":refnum<vi>, "Set Humidity":refnum<vi>, "NL disp 2":refnum<vi>, "Humidity On 2":refnum<vi>, "humidity disp 2":refnum<vi>, "Set Humidity 2":refnum<vi>, "NL disp 3":refnum<vi>, "AppLoadSeq scratch":refnum<vi>, "Stop Scratch":refnum<vi>, "ClrLog":refnum<vi>, "Trip Log":refnum<vi>, "STOP":refnum<vi>, "Start Test":refnum<vi>, "Test status":refnum<vi>, "AR Led":refnum<vi>, "Data":refnum<vi>, "Health":refnum<vi>, "Sway COM Status":refnum<vi>, "Heave COM Status":refnum<vi>, "Grp Tab":refnum<vi>, "Sub Graph":refnum<vi>, "SD (mm)":refnum<vi>, "Siliding distance Reset Graph":refnum<vi>, "SDGp":refnum<vi>, "Humidity Reset Graph":refnum<vi>, "HumrGp":refnum<vi>, "Acoustic Emission (mV)":refnum<vi>, "Aqucostic Reset Graph":refnum<vi>, "gACQUOS":refnum<vi>, "ECR RESET":refnum<vi>, "ECR":refnum<vi>, "Temperature Reset":refnum<vi>, "Acoustic Emission (mV) 2":refnum<vi>, "Aqucostic Reset Graph 2":refnum<vi>, "gACQUOS 2":refnum<vi>, "ECR RESET 2":refnum<vi>, "ECR 2":refnum<vi>, "Temperature Reset 2":refnum<vi>, "Temperature (deg c)":refnum<vi>, "Speed Reset Graph":refnum<vi>, "Speed Tab":refnum<vi>, "MTM DISC  SPEED":refnum<vi>, "MTM BALL SPEED":refnum<vi>, "speed mm/sec":refnum<vi>, "Hymidity":refnum<vi>, "Humidity Disable trip":refnum<vi>, "CoF Trip  2":refnum<vi>, "Depth Trip":refnum<vi>, "Weart Deapth":refnum<vi>, "Depth Reset Graph":refnum<vi>, "Weart":refnum<vi>, "Depthz":refnum<vi>, "Depth (µm)":refnum<vi>, "WearGp":refnum<vi>, "NL Trip 2":refnum<vi>, "Load pid":refnum<vi>, "Load Disable Trip":refnum<vi>, "Load Reset Graph":refnum<vi>, "NL Display 4":refnum<vi>, "Main Chart 3":refnum<vi>, "BACK":refnum<vi>, "Depth Trip 2":refnum<vi>, "COF TRIP ":refnum<vi>, "Friction Force (N)":refnum<vi>, "FF Reset Graph":refnum<vi>, "FF Disable Trip":refnum<vi>, "FF TRIP":refnum<vi>, "COF Disable Trip":refnum<vi>, "COF Reset Graph":refnum<vi>, "Start Test Temp":refnum<vi>, "zFF":refnum<vi>, "Friction Force (N) Graph":refnum<vi>, "Coefficient of Friction":refnum<vi>, "Scratch Start Test":refnum<vi>, "FF Tab":refnum<vi>, "Cyclic Friction Force (N)":refnum<vi>, "CZ FF":refnum<vi>, "Cyclic Friction Force (N) Graph":refnum<vi>, "Cyclic Coefficient of Friction":refnum<vi>, "Cyclic FF TRIP":refnum<vi>, "Cyclic FF Disable Trip":refnum<vi>, "cyclic COF Disable Trip":refnum<vi>, "cyclic COF TRIP":refnum<vi>, "cyclic COF Reset Graph":refnum<vi>, "Cyclic FF Reset Graph":refnum<vi>, "Test Trip":refnum<vi>, "Multi Scratch Pass":refnum<vi>, "Scratch Start Recording":refnum<vi>}, "Loading":cluster{"Indentation":refnum<vi>, "Reference Sample":refnum<vi>, "Load Cell Communication Slide":refnum<vi>, "com 3":refnum<vi>, "com":refnum<vi>, "DecaForce COM Status":refnum<vi>, "Update":refnum<vi>, "Clear 3":refnum<vi>, "seq":refnum<vi>, "Stribeck table":refnum<vi>, "Stribeck Table  For loading":refnum<vi>, "Loading Mode":refnum<vi>, "Enter the Final Load (N)":refnum<vi>, "Enter the CoF Trip":refnum<vi>, "Enter the Friction Force Trip":refnum<vi>, "Enter the Normal load Trip":refnum<vi>, "Enter the Load  (N)":refnum<vi>, "KiloForce":refnum<vi>, "DecaForce ":refnum<vi>, "MicroForce":refnum<vi>, "LHBack":refnum<vi>, "LHNext":refnum<vi>, "Enter the Loading Rate (N/min)":refnum<vi>, "Message":refnum<vi>, "Warning 2":refnum<vi>, "SSP 0.75":refnum<vi>, "SSP 0.5":refnum<vi>, "SSP 0.3":refnum<vi>, "Warning":refnum<vi>, "gui GIF":refnum<vi>, "Communication is established":refnum<vi>, "AppLoad 4":refnum<vi>, "Multipoint":refnum<vi>, "Load Selection":refnum<vi>}, "PID":cluster{"Ramp MulFac":refnum<vi>, "pulses LoadDiffRamp(2..10)":refnum<vi>, "PulseControlRamp(diff<=3N)":refnum<vi>, "SetLoadDeadband(%) Load(0-10N)":refnum<vi>, "PID gains out delay (microForce)":refnum<vi>, "Ramp":refnum<vi>, "Gain 2":refnum<vi>, "pulses LoadDiff(2..10)":refnum<vi>, "pulses LoadDiff(11..50)":refnum<vi>, "PulseControl(diff<=3N)":refnum<vi>, "SetLoadDeadband(%)  2":refnum<vi>, "Dummy Run":refnum<vi>, "Vertical load (N)":refnum<vi>, "AutoTune":refnum<vi>, "Offset 3 ":refnum<vi>, "apply load":refnum<vi>, "Offset  3":refnum<vi>, "apply load 2":refnum<vi>, "Enter ByPass Load":refnum<vi>, "reinit 3":refnum<vi>, "output range delay":refnum<vi>, "PID gains out delay":refnum<vi>, "Bypass Load":refnum<vi>, "pulsesSent":refnum<vi>, "pulses ":refnum<vi>, "actpid":refnum<vi>, "gFF Rot":refnum<vi>, "pulses LoadDiff(21..1000)":refnum<vi>, "Delay":refnum<vi>, "deadband":refnum<vi>}, "Config Parameters":cluster{"Tab Control 3":refnum<vi>, "Tab Control 19":refnum<vi>, "SAMPLES":refnum<vi>, "Re-initilaize":refnum<vi>, "Filter ON/OFF":refnum<vi>, "TracHomeSurgeOffsetCounts 10MM":refnum<vi>, "TracHomeSwayOffsetCounts 10MM":refnum<vi>, "Acoustic Emission:":refnum<vi>, "Apply Filter (FF)":refnum<vi>, "Filter% 2":refnum<vi>, "Apply Filter (Load)":refnum<vi>, "Filter% ":refnum<vi>, "Sway distance (mm)":refnum<vi>, "Surge distance (mm)":refnum<vi>, "DataSavingLoopDelay(ms)":refnum<vi>, "SAVE 2":refnum<vi>, "Enter Distance":refnum<vi>, "Sway Counts:":refnum<vi>, "Distance (mm): 3":refnum<vi>, "Surge Counts:":refnum<vi>, "Distance (mm): 2":refnum<vi>, "Distance (mm):":refnum<vi>, "Heave Counts:":refnum<vi>, "LRMHomeSurgeOffsetCounts":refnum<vi>, "LRMHomeSwayOffsetCounts":refnum<vi>, "TracHomeSurgeOffsetCounts 20MM":refnum<vi>, "TracHomeSwayOffsetCounts 20MM":refnum<vi>, "RotHomeSwayOffsetCounts":refnum<vi>, "RotHomeSurgeOffsetCounts":refnum<vi>, "Heave distance":refnum<vi>, "Zmm":refnum<vi>, "Heave Pulses/mm":refnum<vi>, "Surge Pulses/mm":refnum<vi>, "Sway Pulses/mm":refnum<vi>, "Heave Pitch":refnum<vi>, "Surge Pitch":refnum<vi>, "Sway Pitch":refnum<vi>, "Heave PPR":refnum<vi>, "Surge PPR":refnum<vi>, "Sway PPR":refnum<vi>, "Tab Control 5":refnum<vi>, "Tab Control 14":refnum<vi>, "Tab Control 26":refnum<vi>, "AE":refnum<vi>, "Heave Loop Delay":refnum<vi>, "Heave PID Speed":refnum<vi>, "Surge Jog Speed":refnum<vi>, "Heave Jog Speed":refnum<vi>, "Sway Loop Delay":refnum<vi>, "Sway PID Speed":refnum<vi>, "Sway Jog Speed":refnum<vi>, "DEPTH TRIP VALUE":refnum<vi>, "LOAD TRIP VALUE":refnum<vi>, "DEPTH TRIP   ENABLE":refnum<vi>, "LOAD TRIP  ENABLE":refnum<vi>, "CYCLIC FF TRIP VALUE":refnum<vi>, "FF TRIP VALUE":refnum<vi>, "CYCLIC CoF TRIP VALUE":refnum<vi>, "COF TRIP VALUE":refnum<vi>, "CYCLIC COF TRIP  ENABLE":refnum<vi>, "CYCLIC FF TRIP  ENABLE":refnum<vi>, "FF TRIP  ENABLE":refnum<vi>, "COF TRIP  ENABLE":refnum<vi>}, "Loading Com Port":cluster{"ClearAll":refnum<vi>, "Mz(Nm)":refnum<vi>, "My(Nm)":refnum<vi>, "Mx(Nm)":refnum<vi>, "Save Dwell":refnum<vi>, "Mx ":refnum<vi>, "My ":refnum<vi>, "Mz":refnum<vi>, "Fx(N)":refnum<vi>, "Fy(N)":refnum<vi>, "Fz(N)":refnum<vi>, "ZeroAll":refnum<vi>, "Acq Delay (ms)":refnum<vi>, "Burst Delay (ms)":refnum<vi>, "model":refnum<vi>, "SN":refnum<vi>, "FFx(N)":refnum<vi>, "Sensor IP":refnum<vi>, "Port":refnum<vi>, "FFy(N)":refnum<vi>, "Load(N)":refnum<vi>, "delete Handle":refnum<vi>, "Create Handle":refnum<vi>, "ft_data":refnum<vi>, "ft_range":refnum<vi>, "ft_data 2":refnum<vi>, "stop 6":refnum<vi>, "running_flag":refnum<vi>, "ft_udp_handle":refnum<vi>, "get-data-return":refnum<vi>, "get-range-return":refnum<vi>, "zero-return":refnum<vi>, "filter-return":refnum<vi>, "initial-return":refnum<vi>, "deleteHandle-result":refnum<vi>, "Load Cell Temp":refnum<vi>}, "Heave AND Surge":cluster{"SURGE POSE":refnum<vi>, "error out Read":refnum<vi>, "HEAVE POSE":refnum<vi>, "State":refnum<vi>, "Homed":refnum<vi>, "Sequence ID":refnum<vi>, "error out Write":refnum<vi>, "faultCode":refnum<vi>, "Ack ID":refnum<vi>, "SPEED":refnum<vi>, "Distance":refnum<vi>, "Mode Command":refnum<vi>, "Heave and Surge Read":refnum<vi>, "Read Heave Temp":refnum<vi>, "Spare 15":refnum<vi>, "Spare 14":refnum<vi>, "Spare 13":refnum<vi>, "Spare 12":refnum<vi>, "Spare 11":refnum<vi>, "Spare 10":refnum<vi>, "Spare 9":refnum<vi>, "Spare 8":refnum<vi>, "Spare 7":refnum<vi>, "Spare 6":refnum<vi>, "Spare 5":refnum<vi>, "Spare 4":refnum<vi>, "Spare 2":refnum<vi>, "Spare 1":refnum<vi>, "Node Id":refnum<vi>, "Spare 3":refnum<vi>, "SPARE 4":refnum<vi>, "SPARE 3":refnum<vi>, "SPARE 2":refnum<vi>, "SPARE 1":refnum<vi>, "fwMajor":refnum<vi>, "fwMinor":refnum<vi>, "Manual Write":refnum<vi>, "Heave and Surge Write":refnum<vi>}, "New PID LOGIC":cluster{"Fine Tune Zone":refnum<vi>, "PID SDelay":refnum<vi>, "Max_pos_limit":refnum<vi>, "Min_pos_limit":refnum<vi>, "i_limit":refnum<vi>, "pct_scale":refnum<vi>, "Deadband":refnum<vi>, "Kd":refnum<vi>, "Ki":refnum<vi>, "Kp":refnum<vi>, "Current Position":refnum<vi>, "Set Load":refnum<vi>, "Current Load":refnum<vi>, "Pulse delta":refnum<vi>, "Init Step":refnum<vi>, "Max Step Linit":refnum<vi>}, "SWAY ":cluster{"fwMajor":refnum<vi>, "Homed":refnum<vi>, "Rotary POSE":refnum<vi>, "State":refnum<vi>, "SWAY POSE":refnum<vi>, "Ack ID":refnum<vi>, "faultCode":refnum<vi>, "Node Id":refnum<vi>, "fwMinor":refnum<vi>, "Spare 6":refnum<vi>, "Spare 5":refnum<vi>, "Spare 4":refnum<vi>, "Spare 3":refnum<vi>, "Spare 2":refnum<vi>, "Spare 1":refnum<vi>, "Spare 7":refnum<vi>, "SPARE  5":refnum<vi>, "error out Write  SWAY ":refnum<vi>, "error out Read SWAY ":refnum<vi>, "Manual Write SWAY ":refnum<vi>, "SWAY WRITE":refnum<vi>, "SPARE  4":refnum<vi>, "SPARE  3":refnum<vi>, "SPARE 2":refnum<vi>, "SPARE 1":refnum<vi>, "Spare 15":refnum<vi>, "Spare 14":refnum<vi>, "Spare 13":refnum<vi>, "Spare 12":refnum<vi>, "Spare 11":refnum<vi>, "Spare 9":refnum<vi>, "Spare 8":refnum<vi>, "SPEED":refnum<vi>, "Distance":refnum<vi>, "Mode Command":refnum<vi>, "Sequence ID":refnum<vi>, "SWAY READ":refnum<vi>, "Spare 10":refnum<vi>, "Read SWAY Temp":refnum<vi>}, "Analysis Screen":cluster{"Analysis Home":refnum<vi>, "Refresh 2":refnum<vi>, "MEAN 4":refnum<vi>, "SD 4":refnum<vi>, "VARIANCE 4":refnum<vi>, "MEAN  3":refnum<vi>, "SD  3":refnum<vi>, "VARIANCE  3":refnum<vi>, "MEAN 2":refnum<vi>, "SD  2":refnum<vi>, "VARIANCE 2":refnum<vi>, "MEAN":refnum<vi>, "SD":refnum<vi>, "VARIANCE":refnum<vi>, "File 4 Discription":refnum<vi>, "OPEN 4":refnum<vi>, "File Name 4":refnum<vi>, "OPEN 3":refnum<vi>, "File 3 Discription":refnum<vi>, "File Name 3":refnum<vi>, "Y-AXIS":refnum<vi>, "X-AXIS":refnum<vi>, "XY Graph":refnum<vi>, "File Name 2":refnum<vi>, "File Name 1":refnum<vi>, "OPEN 2":refnum<vi>, "OPEN 1":refnum<vi>, "File 1 Discription ":refnum<vi>, "File 2 Discription":refnum<vi>, "Export":refnum<vi>, "File Format":refnum<vi>}}
  T12 = typedef "init queue out loop.ctl" = cluster{"UI Loop":refnum<queue>, "LOAD COM LOOP ":refnum<queue>, "SWAY MOTOR COM LOOP":refnum<queue>, "HEAVE MOTOR COM LOOP":refnum<queue>, "TEMPERATURE COM LOOP":refnum<queue>, "RAMP MOTOR COM LOOP":refnum<queue>, "ECR PORT":refnum<queue>, "HUMIDITY COM PORT":refnum<queue>, "PROGRAM LOOP":refnum<queue>, "MONITOR LOOP":refnum<queue>, "REPORT":refnum<queue>, "LOAD PID":refnum<queue>}
  T13 = typedef "XDNodeRunTimeDep.lvlib/timing_clust.ctl" = cluster{"Expected End [f-1]":u64, "Actual End [f-1]":u64, "Finished Late? [f-1]":bool, "Expected End [i-1]":u64, "Actual End [i-1]":u64, "Finished Late? [i-1]":bool, "Expected Start [i]":u64, "Actual Start [i]":u64, "Expected Start [f]":u64, "Actual Start [f]":u64, "Source Name":string, "Structure Name":string, "Period":i64, "Deadline":i64, "Offset":i64, "Start":i64, "Priority":i32, "Timeout":i32, "Mode":T14, "Wakeup Reason":T15, "Error":errorcluster, "Source Type":string, "Secondary Source Type":string, "Global End Time":u64, "Global Start Time":u64, "Frame Duration":u64, "Iteration Duration":u64, "Assigned CPU":i32, "I/O Scan Engine Mode":u32}
  T14 = typedef "XDNodeRunTimeDep.lvlib/nitl_modes.ctl" = enum32{"No Change", "Process missed periods, maintain original phase", "Discard missed periods, maintain original phase", "Process missed periods, ignore original phase", "Discard missed periods, ignore original phase"}
  T15 = typedef "XDNodeRunTimeDep.lvlib/wakeup.ctl" = enum32{"Normal", "Aborted", "Asynchronous wakeup", "Timing source error", "Timed loop error", "Timeout"}
  T16 = enum8{"Enabled", "Disabled", "Disabled and Grayed Out"}
  T17 = enum16{"INIT", "SETLOWPASSFILTER", "SETZERO", "GETSENSORINFO", "GETRANGE", "ZEROALL", "READDATA", "UNINITIAL", "DELETEHANDLE"}
  T18 = typedef "Heave Write enum.ctl" = enum16{"INIT", "WRITE", "CLOSE", "REINIT"}
  T19 = typedef "Sway Write enum.ctl" = enum16{"INIT", "WRITE", "CLOSE", "REINIT"}
  T20 = typedef "Sway Right enum.ctl" = enum16{"INIT", "READ", "CLOSE", "REINIT", ""}
  T21 = typedef "Heave Right enum.ctl" = enum16{"INIT", "READ", "CLOSE", "REINIT", ""}
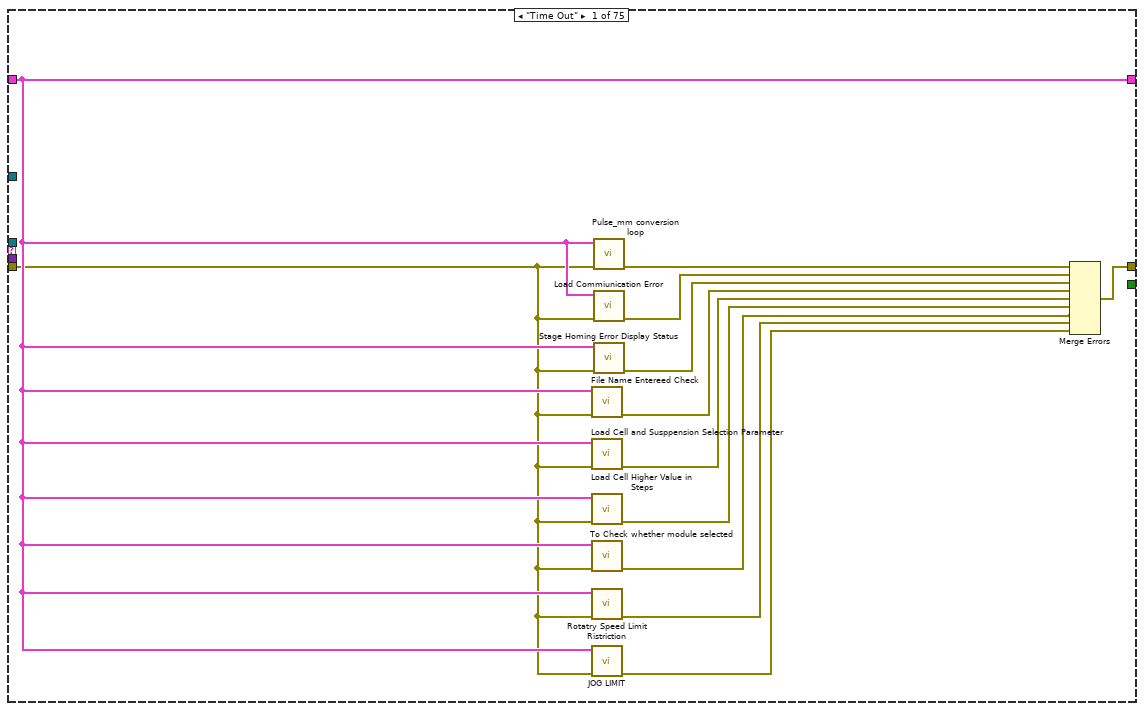
[diagram p2: hidden frame]
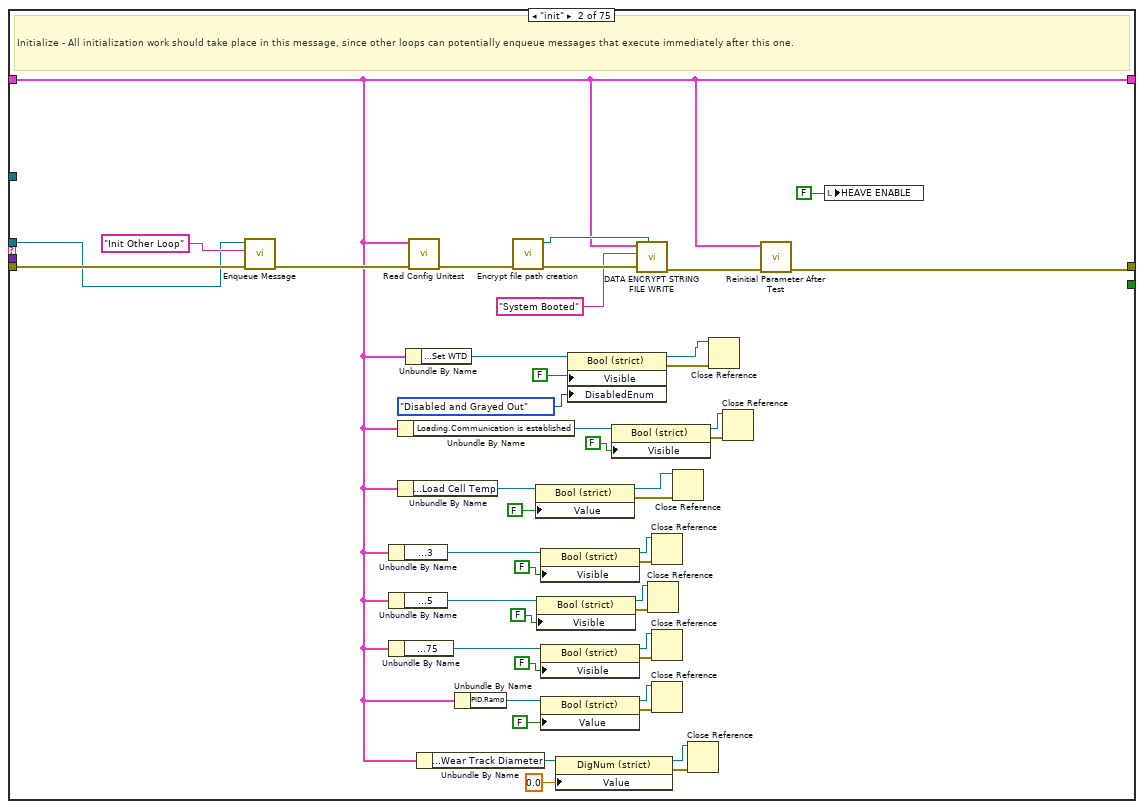
[diagram p3: hidden frame]
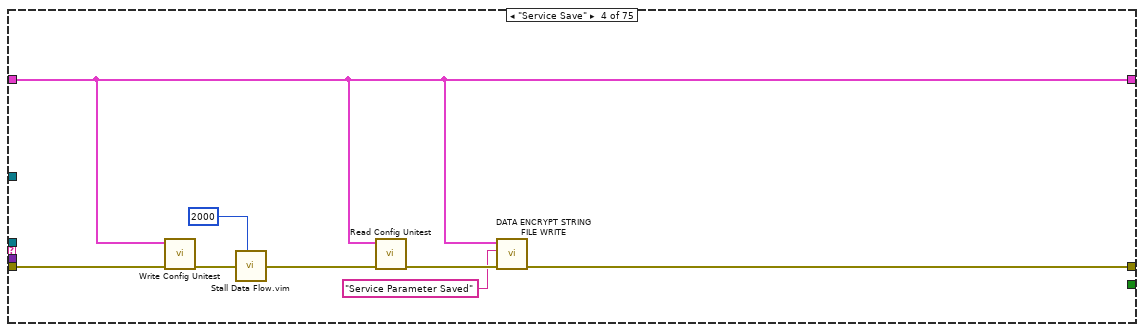
[diagram p5: hidden frame]
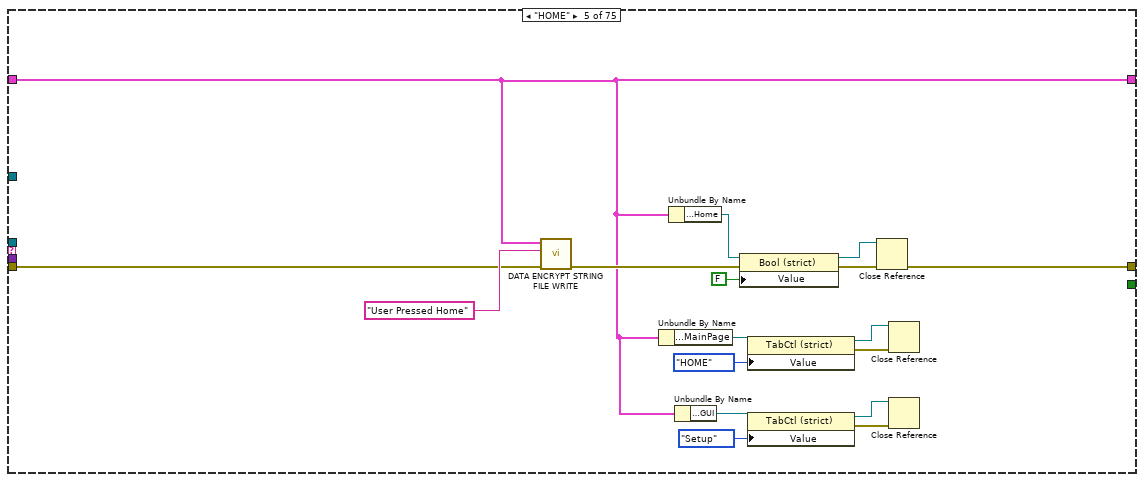
[diagram p6: hidden frame]
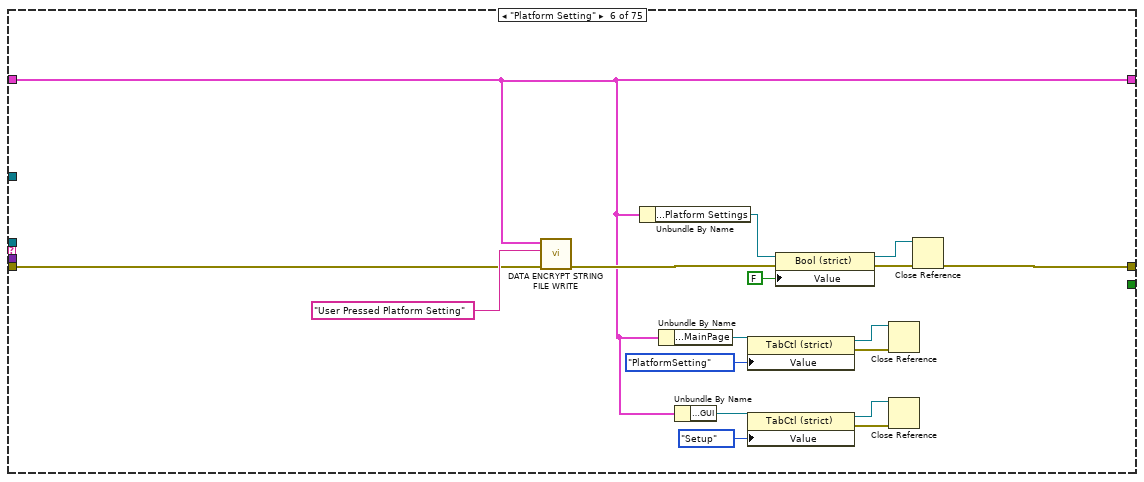
[diagram p7: hidden frame]
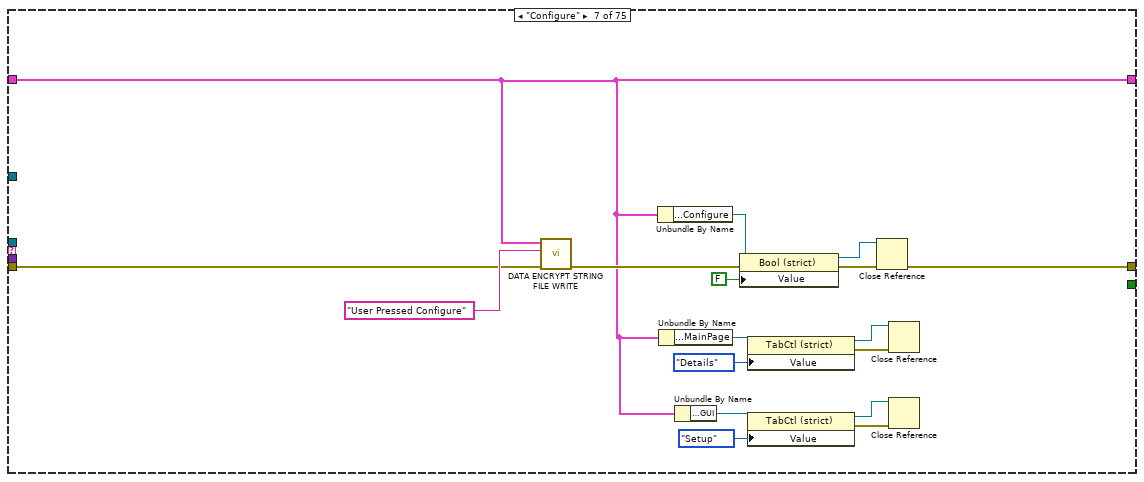
[diagram p8: hidden frame]
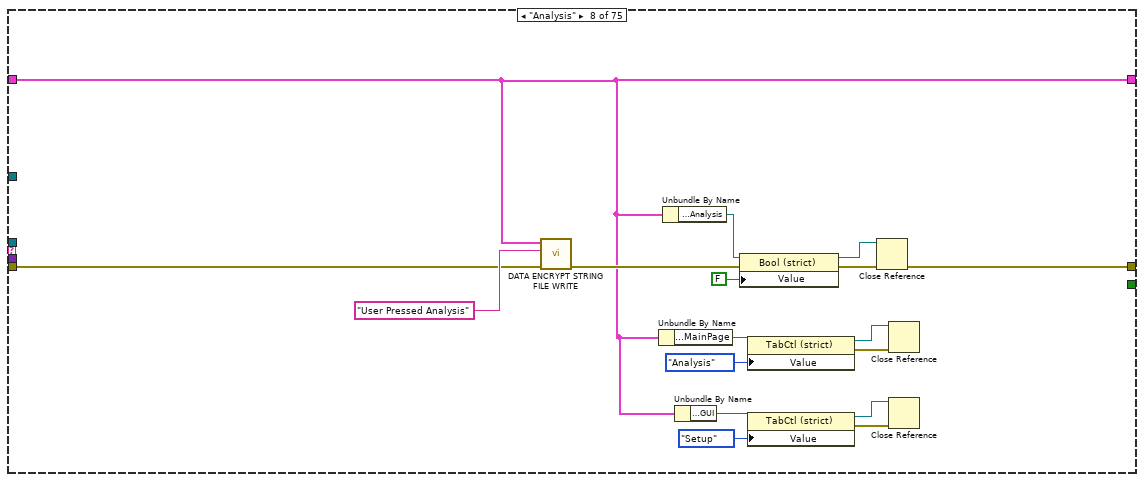
[diagram p9: hidden frame]
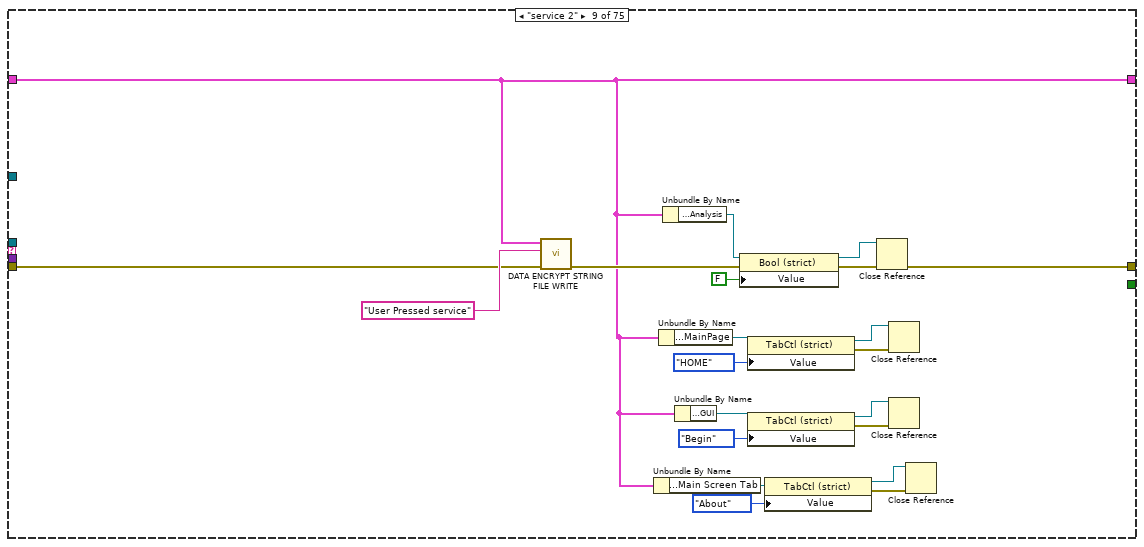
[diagram p10: hidden frame]
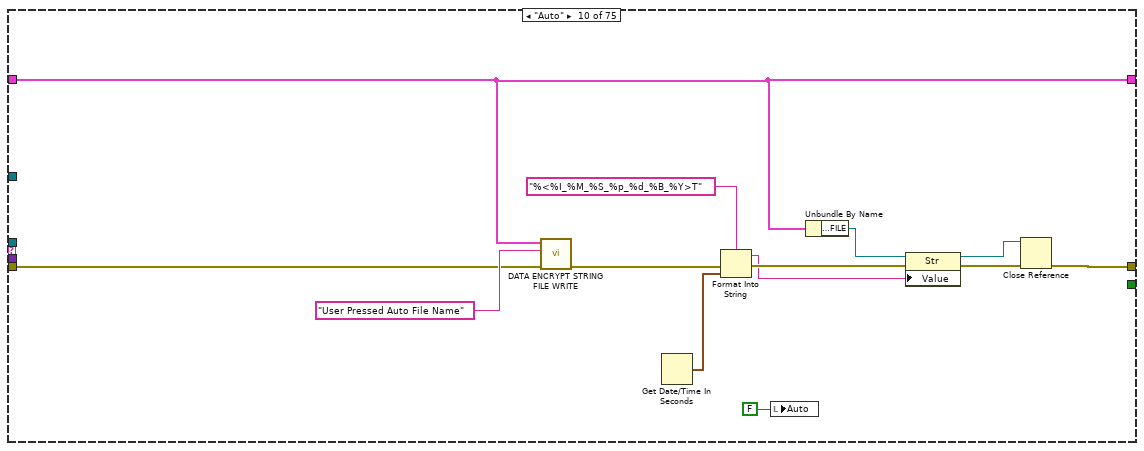
[diagram p11: hidden frame]
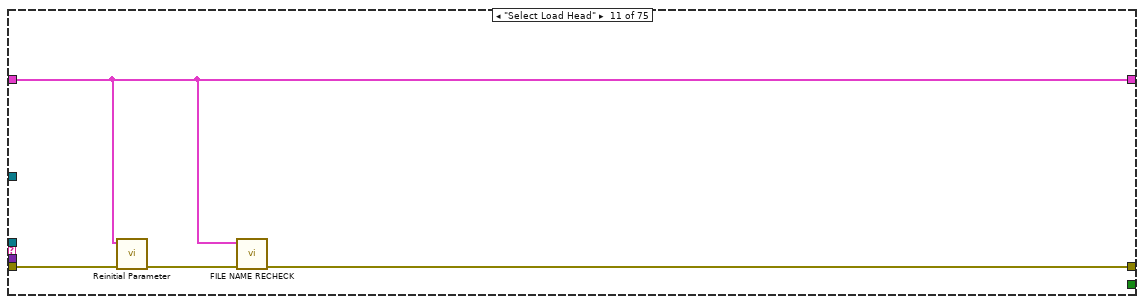
[diagram p12: hidden frame]
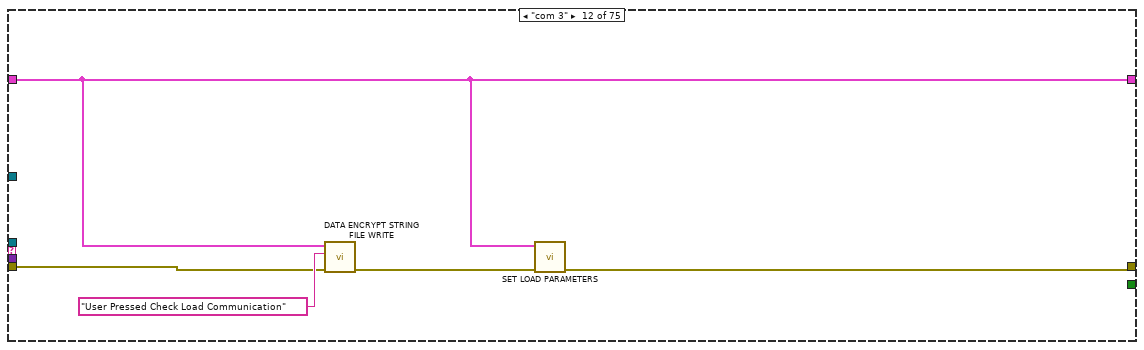
[diagram p13: hidden frame]
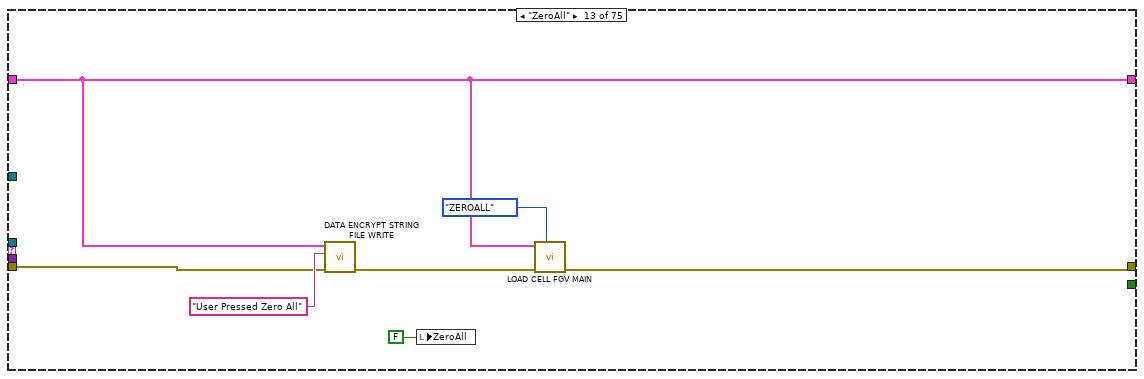
[diagram p14: hidden frame]
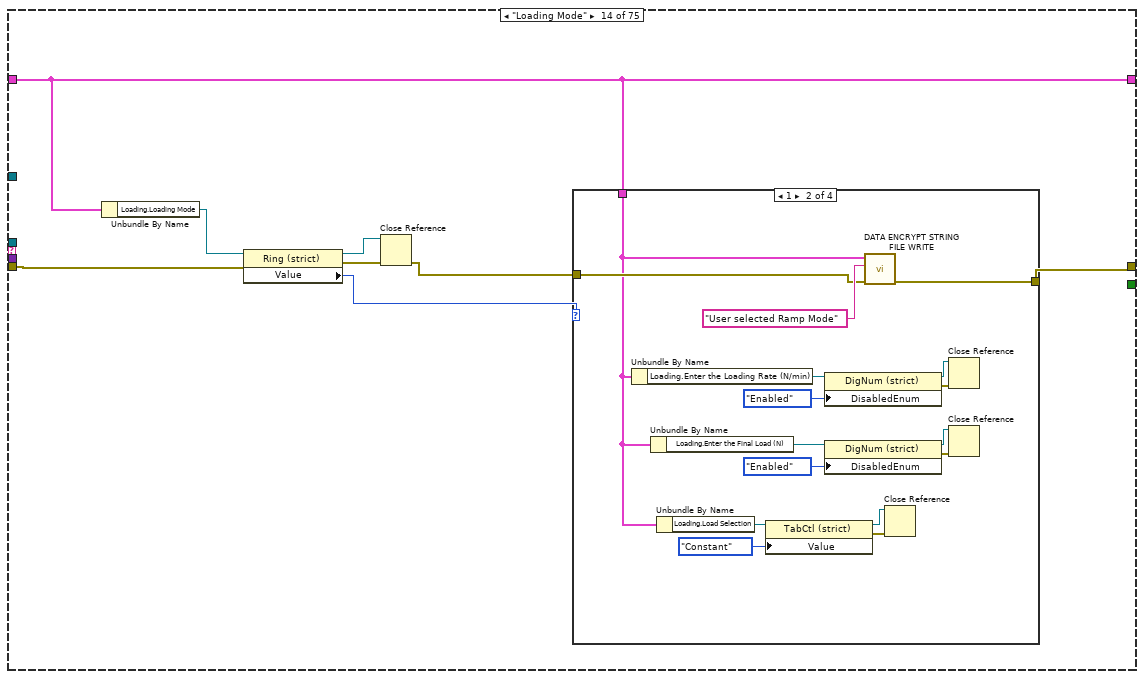
[diagram p15: hidden frame]
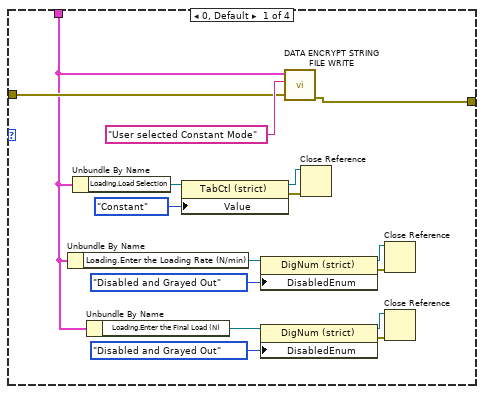
[diagram p16: hidden frame]
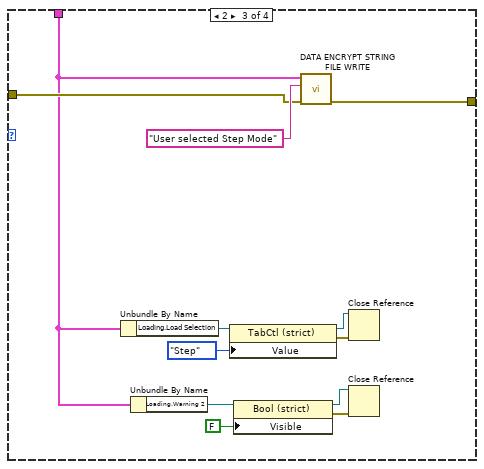
[diagram p17: hidden frame]
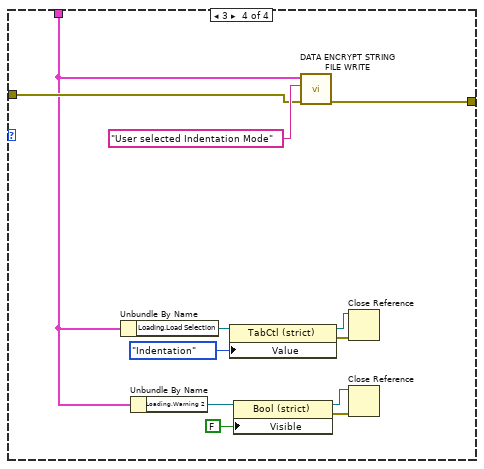
[diagram p18: hidden frame]
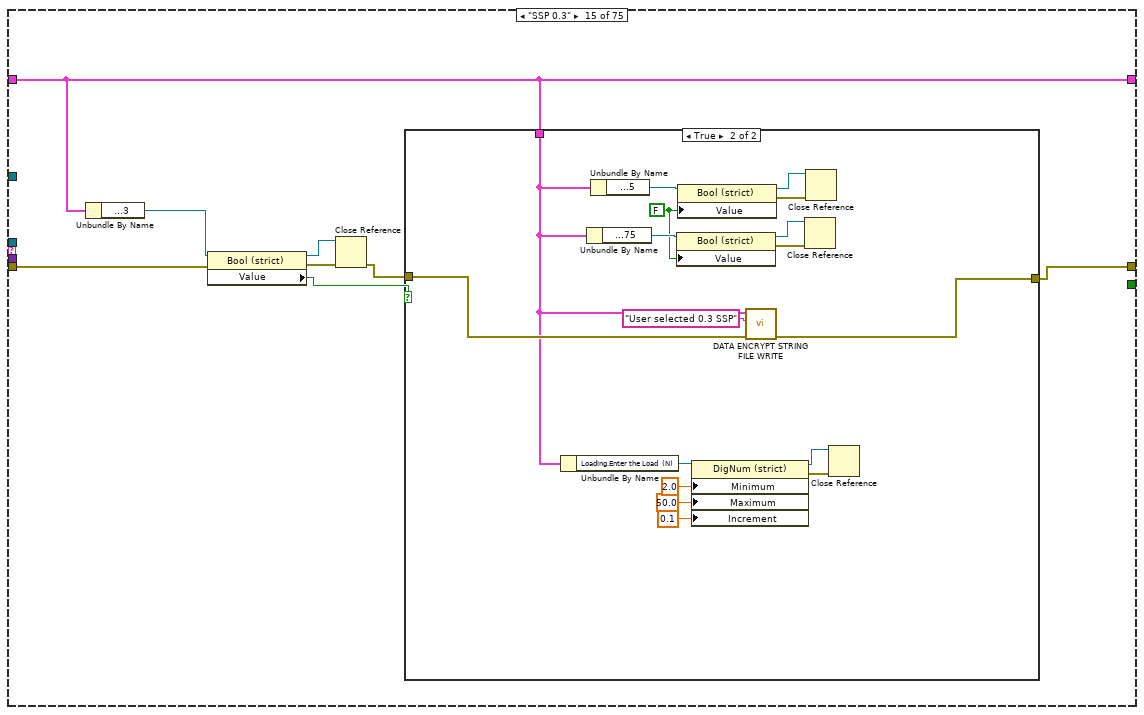
[diagram p19: hidden frame]
diagram:
  w1 = 0.0 ("prev_error_out")
  n1 = flat-sequence {
    tunnel: [w69] -> w56
    tunnel: T11 {"Main Home Screen"={"GUI"=refnum, "Platform Settings"=refnum, "Configure"=refnum, "Home"=refnum, "EXIT"=refnum, "service 2"=refnum, "MainPage"=refnum, "Analysis"=refnum}, "Platform Settings"={"mm/s  Surge"=refnum, "Update Surge Speed"=refnum, "Drive Error"=refnum, "Disable Axis Jog Soft Limits"=refnum, "mm/s  Sway"=refnum, "Sway and Surge COM Status"=refnum, "Heave COM Status"=refnum, "Enable Platform"=refnum, "Surge Forward Main"=refnum, "Sway Right Main"=refnum, "Sway Left Main"=refnum, "Heave Down Main"=refnum, "Heave Up main"=refnum, "Update Sway Speed"=refnum, "Update Heave Speed"=refnum, "mm/s Heave"=refnum, "mm/sec"=refnum, "mm"=refnum, "Surge Backward Main"=refnum}, "Analysis Screen"={"Analysis Home"=refnum, "Surface Analysis"=refnum, "Imaging"=refnum, "Image Analysis"=refnum, "Post Analysis"=refnum}, "Config Screen"={"Select Load Head"=refnum, "Notes :"=refnum, "FILE"=refnum, "Sample ID :"=refnum, "Operator ID :"=refnum, "Operator Name :"=refnum, "Auto"=refnum}, "Motion Module"={"zNL"=refnum, "NL disp"=refnum, "Rotary Tab"=refnum, "Motion Direction:  3"=refnum, "E.Velocity 2"=refnum, "e.v/ssr 2"=refnum, "Enter Fixed E.Velocity 2"=refnum, "Enter Final SRR 2"=refnum, "Enter initial SRR 2"=refnum, "Enter Fixed SRR 2"=refnum, "Enter the Final E.Velocity (m/s) 2"=refnum, "Enter initial E.Velocity (m/s) 2"=refnum, "Final Speed (RPM) 3"=refnum, "Initial Speed (RPM) 2"=refnum, "Enter the Final Velocity (m/s) 3"=refnum, "Enter initial Velocity (m/s)  3"=refnum, "Ramp Up 2"=refnum, "TEST SELECTION"=refnum, "SPEED SELECTION : "=refnum, "Angular Oscillation Set"=refnum, "Traction"=refnum, "Step Speed"=refnum, "StepTable For Load-Speed"=refnum, "StepTable For Speed"=refnum, "Surge Forward MM"=refnum, "Surge Backward MM"=refnum, "M3 Image"=refnum, "String 39"=refnum, "Sway Left MM"=refnum, "Sway Right MM"=refnum, "Disable Axis Jog Soft Limits"=refnum, "mm"=refnum, "Heave Down MM"=refnum, "Heave Up MM"=refnum, "Wear Track Diameter (mm)"=refnum, "Set WTD"=refnum, "HomeScratch"=refnum, "HomeRot"=refnum, "PlaceModule"=refnum, "Enter the Angle (Deg)"=refnum, "Enter the Frequency (Hz)"=refnum, "Motion Mode:"=refnum, "LR Sway"=refnum, "Rot Hor"=refnum, "Scratch"=refnum, "LR Cam"=refnum, "MMBack"=refnum, "MMNext"=refnum, "Rot Ver"=refnum, "Rotary Module Selection"=refnum, "calculate rotary"=refnum, "SPEED SELECTION : rotary"=refnum, "Import 2"=refnum, "Save 2"=refnum, "File Path :  2"=refnum, "String 45"=refnum, "StepTable For Speed 3"=refnum, "Enter the Speed(mm/sec)"=refnum, "Enter the Speed(RPM)"=refnum, "Enter Scratch Speed (mm/s):"=refnum, "SwaySpeed Set"=refnum, "Scartch Offset"=refnum, "Motion type:"=refnum, "HomeScratch 2"=refnum, "Enter Scratch length (mm):"=refnum, "Wear Track Diameter"=refnum, "Rotary Speed Exced"=refnum, "Scratch Mode"=refnum, "No of Scratch"=refnum}, "Environmental control"={"Humidity  Status  3"=refnum, "Low Temp  Status  2"=refnum, "TK4 status 2"=refnum, "Stage Temperature"=refnum, "Sample Temperature"=refnum, "Humidity (Amb)"=refnum, "Clear List"=refnum, "Add to list"=refnum, "Wear"=refnum, "Vibration"=refnum, "Humidity (Chamber)"=refnum, "Temperature (Chamber)"=refnum, "ECR "=refnum, "Temperature (Amb)"=refnum, "Microphone"=refnum, "Acoustic Emission 3"=refnum, "SNext"=refnum, "APBack"=refnum, "Enter the Temperature (°C):"=refnum, "Enter the Stage \nTemperature (°C):"=refnum, "Enter the Humidity (%Rh):"=refnum, "Low Temp"=refnum, "High Temp"=refnum, "Humidity"=refnum, "Sensors Picked"=refnum}, "About Screen"={"Password"=refnum, "Home Service"=refnum, "Advanced Setting"=refnum, "About Tab"=refnum, "ECR Port:"=refnum, "Ramp Port:"=refnum, "Installation/Replacement completed"=refnum, "Loahead"=refnum, "Heave and Surge COM Port:"=refnum, "Sway COM Port:"=refnum, "Temp Modbus:"=refnum, "Humidity Port:"=refnum, "Edit Gain Constants"=refnum, "Save Gain Constants"=refnum}, "Main Screen"={"Main Screen Tab"=refnum, "Angle and Frequency"=refnum, "Stroke (mm)"=refnum, "Angle (Deg)"=refnum, "Main Speed Tab"=refnum, "MTM MOTOR DISPLAY"=refnum, "Disc Speed (m/sec)"=refnum, "Ball Speed (m/sec)"=refnum, "Disc Speed (RPM)"=refnum, "Ball Speed (RPM)"=refnum, "SPEED TAB"=refnum, "Speed (m/sec)"=refnum, "Set Speed (m/sec)"=refnum, "Speed (RPM)"=refnum, "Set Speed"=refnum, "Time Tab"=refnum, "Time ( HH:MM:SS ) 2"=refnum, "Test Duration"=refnum, "Test Duration 4"=refnum, "TEST CYCLE"=refnum, "TOTAL CYCLES"=refnum, "Set Load (N)"=refnum, "Temp Tabs"=refnum, "Heater"=refnum, "TK4 status"=refnum, "ChamberTemp"=refnum, "SetTmp"=refnum, "Controller  Status"=refnum, "ChamberTemp 2"=refnum, "SetTmp 2"=refnum, "Controller  Status 2"=refnum, "ChamberTemp 3"=refnum, "SetTmp 3"=refnum, "Cooling"=refnum, "Load Communication"=refnum, "Ambient \nTemperature"=refnum, "HumCOMStatus"=refnum, "Ambient\n Humidity"=refnum, "Freq (Hz)"=refnum, "Load En"=refnum, "NLt"=refnum, "zNL 2"=refnum, "Humidity On"=refnum, "humidity disp"=refnum, "Set Humidity"=refnum, "NL disp 2"=refnum, "Humidity On 2"=refnum, "humidity disp 2"=refnum, "Set Humidity 2"=refnum, "NL disp 3"=refnum, "AppLoadSeq scratch"=refnum, "Stop Scratch"=refnum, "ClrLog"=refnum, "Trip Log"=refnum, "STOP"=refnum, "Start Test"=refnum, "Test status"=refnum, "AR Led"=refnum, "Data"=refnum, "Health"=refnum, "Sway COM Status"=refnum, "Heave COM Status"=refnum, "Grp Tab"=refnum, "Sub Graph"=refnum, "SD (mm)"=refnum, "Siliding distance Reset Graph"=refnum, "SDGp"=refnum, "Humidity Reset Graph"=refnum, "HumrGp"=refnum, "Acoustic Emission (mV)"=refnum, "Aqucostic Reset Graph"=refnum, "gACQUOS"=refnum, "ECR RESET"=refnum, "ECR"=refnum, "Temperature Reset"=refnum, "Acoustic Emission (mV) 2"=refnum, "Aqucostic Reset Graph 2"=refnum, "gACQUOS 2"=refnum, "ECR RESET 2"=refnum, "ECR 2"=refnum, "Temperature Reset 2"=refnum, "Temperature (deg c)"=refnum, "Speed Reset Graph"=refnum, "Speed Tab"=refnum, "MTM DISC  SPEED"=refnum, "MTM BALL SPEED"=refnum, "speed mm/sec"=refnum, "Hymidity"=refnum, "Humidity Disable trip"=refnum, "CoF Trip  2"=refnum, "Depth Trip"=refnum, "Weart Deapth"=refnum, "Depth Reset Graph"=refnum, "Weart"=refnum, "Depthz"=refnum, "Depth (µm)"=refnum, "WearGp"=refnum, "NL Trip 2"=refnum, "Load pid"=refnum, "Load Disable Trip"=refnum, "Load Reset Graph"=refnum, "NL Display 4"=refnum, "Main Chart 3"=refnum, "BACK"=refnum, "Depth Trip 2"=refnum, "COF TRIP "=refnum, "Friction Force (N)"=refnum, "FF Reset Graph"=refnum, "FF Disable Trip"=refnum, "FF TRIP"=refnum, "COF Disable Trip"=refnum, "COF Reset Graph"=refnum, "Start Test Temp"=refnum, "zFF"=refnum, "Friction Force (N) Graph"=refnum, "Coefficient of Friction"=refnum, "Scratch Start Test"=refnum, "FF Tab"=refnum, "Cyclic Friction Force (N)"=refnum, "CZ FF"=refnum, "Cyclic Friction Force (N) Graph"=refnum, "Cyclic Coefficient of Friction"=refnum, "Cyclic FF TRIP"=refnum, "Cyclic FF Disable Trip"=refnum, "cyclic COF Disable Trip"=refnum, "cyclic COF TRIP"=refnum, "cyclic COF Reset Graph"=refnum, "Cyclic FF Reset Graph"=refnum, "Test Trip"=refnum, "Multi Scratch Pass"=refnum, "Scratch Start Recording"=refnum}, "Loading"={"Indentation"=refnum, "Reference Sample"=refnum, "Load Cell Communication Slide"=refnum, "com 3"=refnum, "com"=refnum, "DecaForce COM Status"=refnum, "Update"=refnum, "Clear 3"=refnum, "seq"=refnum, "Stribeck table"=refnum, "Stribeck Table  For loading"=refnum, "Loading Mode"=refnum, "Enter the Final Load (N)"=refnum, "Enter the CoF Trip"=refnum, "Enter the Friction Force Trip"=refnum, "Enter the Normal load Trip"=refnum, "Enter the Load  (N)"=refnum, "KiloForce"=refnum, "DecaForce "=refnum, "MicroForce"=refnum, "LHBack"=refnum, "LHNext"=refnum, "Enter the Loading Rate (N/min)"=refnum, "Message"=refnum, "Warning 2"=refnum, "SSP 0.75"=refnum, "SSP 0.5"=refnum, "SSP 0.3"=refnum, "Warning"=refnum, "gui GIF"=refnum, "Communication is established"=refnum, "AppLoad 4"=refnum, "Multipoint"=refnum, "Load Selection"=refnum}, "PID"={"Ramp MulFac"=refnum, "pulses LoadDiffRamp(2..10)"=refnum, "PulseControlRamp(diff<=3N)"=refnum, "SetLoadDeadband(%) Load(0-10N)"=refnum, "PID gains out delay (microForce)"=refnum, "Ramp"=refnum, "Gain 2"=refnum, "pulses LoadDiff(2..10)"=refnum, "pulses LoadDiff(11..50)"=refnum, "PulseControl(diff<=3N)"=refnum, "SetLoadDeadband(%)  2"=refnum, "Dummy Run"=refnum, "Vertical load (N)"=refnum, "AutoTune"=refnum, "Offset 3 "=refnum, "apply load"=refnum, "Offset  3"=refnum, "apply load 2"=refnum, "Enter ByPass Load"=refnum, "reinit 3"=refnum, "output range delay"=refnum, "PID gains out delay"=refnum, "Bypass Load"=refnum, "pulsesSent"=refnum, "pulses "=refnum, "actpid"=refnum, "gFF Rot"=refnum, "pulses LoadDiff(21..1000)"=refnum, "Delay"=refnum, "deadband"=refnum}, "Config Parameters"={"Tab Control 3"=refnum, "Tab Control 19"=refnum, "SAMPLES"=refnum, "Re-initilaize"=refnum, "Filter ON/OFF"=refnum, "TracHomeSurgeOffsetCounts 10MM"=refnum, "TracHomeSwayOffsetCounts 10MM"=refnum, "Acoustic Emission:"=refnum, "Apply Filter (FF)"=refnum, "Filter% 2"=refnum, "Apply Filter (Load)"=refnum, "Filter% "=refnum, "Sway distance (mm)"=refnum, "Surge distance (mm)"=refnum, "DataSavingLoopDelay(ms)"=refnum, "SAVE 2"=refnum, "Enter Distance"=refnum, "Sway Counts:"=refnum, "Distance (mm): 3"=refnum, "Surge Counts:"=refnum, "Distance (mm): 2"=refnum, "Distance (mm):"=refnum, "Heave Counts:"=refnum, "LRMHomeSurgeOffsetCounts"=refnum, "LRMHomeSwayOffsetCounts"=refnum, "TracHomeSurgeOffsetCounts 20MM"=refnum, "TracHomeSwayOffsetCounts 20MM"=refnum, "RotHomeSwayOffsetCounts"=refnum, "RotHomeSurgeOffsetCounts"=refnum, "Heave distance"=refnum, "Zmm"=refnum, "Heave Pulses/mm"=refnum, "Surge Pulses/mm"=refnum, "Sway Pulses/mm"=refnum, "Heave Pitch"=refnum, "Surge Pitch"=refnum, "Sway Pitch"=refnum, "Heave PPR"=refnum, "Surge PPR"=refnum, "Sway PPR"=refnum, "Tab Control 5"=refnum, "Tab Control 14"=refnum, "Tab Control 26"=refnum, "AE"=refnum, "Heave Loop Delay"=refnum, "Heave PID Speed"=refnum, "Surge Jog Speed"=refnum, "Heave Jog Speed"=refnum, "Sway Loop Delay"=refnum, "Sway PID Speed"=refnum, "Sway Jog Speed"=refnum, "DEPTH TRIP VALUE"=refnum, "LOAD TRIP VALUE"=refnum, "DEPTH TRIP   ENABLE"=refnum, "LOAD TRIP  ENABLE"=refnum, "CYCLIC FF TRIP VALUE"=refnum, "FF TRIP VALUE"=refnum, "CYCLIC CoF TRIP VALUE"=refnum, "COF TRIP VALUE"=refnum, "CYCLIC COF TRIP  ENABLE"=refnum, "CYCLIC FF TRIP  ENABLE"=refnum, "FF TRIP  ENABLE"=refnum, "COF TRIP  ENABLE"=refnum}, "Loading Com Port"={"ClearAll"=refnum, "Mz(Nm)"=refnum, "My(Nm)"=refnum, "Mx(Nm)"=refnum, "Save Dwell"=refnum, "Mx "=refnum, "My "=refnum, "Mz"=refnum, "Fx(N)"=refnum, "Fy(N)"=refnum, "Fz(N)"=refnum, "ZeroAll"=refnum, "Acq Delay (ms)"=refnum, "Burst Delay (ms)"=refnum, "model"=refnum, "SN"=refnum, "FFx(N)"=refnum, "Sensor IP"=refnum, "Port"=refnum, "FFy(N)"=refnum, "Load(N)"=refnum, "delete Handle"=refnum, "Create Handle"=refnum, "ft_data"=refnum, "ft_range"=refnum, "ft_data 2"=refnum, "stop 6"=refnum, "running_flag"=refnum, "ft_udp_handle"=refnum, "get-data-return"=refnum, "get-range-return"=refnum, "zero-return"=refnum, "filter-return"=refnum, "initial-return"=refnum, "deleteHandle-result"=refnum, "Load Cell Temp"=refnum}, "Heave AND Surge"={"SURGE POSE"=refnum, "error out Read"=refnum, "HEAVE POSE"=refnum, "State"=refnum, "Homed"=refnum, "Sequence ID"=refnum, "error out Write"=refnum, "faultCode"=refnum, "Ack ID"=refnum, "SPEED"=refnum, "Distance"=refnum, "Mode Command"=refnum, "Heave and Surge Read"=refnum, "Read Heave Temp"=refnum, "Spare 15"=refnum, "Spare 14"=refnum, "Spare 13"=refnum, "Spare 12"=refnum, "Spare 11"=refnum, "Spare 10"=refnum, "Spare 9"=refnum, "Spare 8"=refnum, "Spare 7"=refnum, "Spare 6"=refnum, "Spare 5"=refnum, "Spare 4"=refnum, "Spare 2"=refnum, "Spare 1"=refnum, "Node Id"=refnum, "Spare 3"=refnum, "SPARE 4"=refnum, "SPARE 3"=refnum, "SPARE 2"=refnum, "SPARE 1"=refnum, "fwMajor"=refnum, "fwMinor"=refnum, "Manual Write"=refnum, "Heave and Surge Write"=refnum}, "New PID LOGIC"={"Fine Tune Zone"=refnum, "PID SDelay"=refnum, "Max_pos_limit"=refnum, "Min_pos_limit"=refnum, "i_limit"=refnum, "pct_scale"=refnum, "Deadband"=refnum, "Kd"=refnum, "Ki"=refnum, "Kp"=refnum, "Current Position"=refnum, "Set Load"=refnum, "Current Load"=refnum, "Pulse delta"=refnum, "Init Step"=refnum, "Max Step Linit"=refnum}, "SWAY "={"fwMajor"=refnum, "Homed"=refnum, "Rotary POSE"=refnum, "State"=refnum, "SWAY POSE"=refnum, "Ack ID"=refnum, "faultCode"=refnum, "Node Id"=refnum, "fwMinor"=refnum, "Spare 6"=refnum, "Spare 5"=refnum, "Spare 4"=refnum, "Spare 3"=refnum, "Spare 2"=refnum, "Spare 1"=refnum, "Spare 7"=refnum, "SPARE  5"=refnum, "error out Write  SWAY "=refnum, "error out Read SWAY "=refnum, "Manual Write SWAY "=refnum, "SWAY WRITE"=refnum, "SPARE  4"=refnum, "SPARE  3"=refnum, "SPARE 2"=refnum, "SPARE 1"=refnum, "Spare 15"=refnum, "Spare 14"=refnum, "Spare 13"=refnum, "Spare 12"=refnum, "Spare 11"=refnum, "Spare 9"=refnum, "Spare 8"=refnum, "SPEED"=refnum, "Distance"=refnum, "Mode Command"=refnum, "Sequence ID"=refnum, "SWAY READ"=refnum, "Spare 10"=refnum, "Read SWAY Temp"=refnum}, "Analysis Screen"={"Analysis Home"=refnum, "Refresh 2"=refnum, "MEAN 4"=refnum, "SD 4"=refnum, "VARIANCE 4"=refnum, "MEAN  3"=refnum, "SD  3"=refnum, "VARIANCE  3"=refnum, "MEAN 2"=refnum, "SD  2"=refnum, "VARIANCE 2"=refnum, "MEAN"=refnum, "SD"=refnum, "VARIANCE"=refnum, "File 4 Discription"=refnum, "OPEN 4"=refnum, "File Name 4"=refnum, "OPEN 3"=refnum, "File 3 Discription"=refnum, "File Name 3"=refnum, "Y-AXIS"=refnum, "X-AXIS"=refnum, "XY Graph"=refnum, "File Name 2"=refnum, "File Name 1"=refnum, "OPEN 2"=refnum, "OPEN 1"=refnum, "File 1 Discription "=refnum, "File 2 Discription"=refnum, "Export"=refnum, "File Format"=refnum}} ("Data Cluster") -> [w68]
    tunnel: w56 -> [w98]
    tunnel: [w78] -> w55
    tunnel: w55 -> [w105]
    tunnel: [w99] -> w54
    tunnel: w54 -> [w114]
    tunnel: [w113] -> w53
    tunnel: w53 -> [w150]
    tunnel: [w149] -> w51
    tunnel: w51 -> [w221]
    tunnel: [w220] -> w50
    tunnel: w50 -> [w248]
    tunnel: [w247] -> w49
    tunnel: w49 -> [w264]
    tunnel: [w263] -> w48
    tunnel: w48 -> [w384]
    tunnel: [w383] -> w23
    tunnel: w23 -> [w414]
    tunnel: [w413] -> w22
    tunnel: w22 -> [w479]
    tunnel: [w478] -> w21
    tunnel: w21 -> [w516]
    tunnel: [w515] -> w20
    tunnel: w20 -> [w556]
    tunnel: [w555] -> w17
    tunnel: w17 -> [w574]
    tunnel: [w573] -> w16
    tunnel: w16 -> [w615]
    tunnel: [w614] -> w14
    tunnel: [w647] -> w28
    tunnel: w14 -> [w648]
    frame #0 {
      n2 = control-ref of="GUI"() -> (w77:refnum<vi>)
      n3 = control-ref of="MainPage"() -> (w71:refnum<vi>)
      n4 = control-ref of="Platform Settings"() -> (w76:refnum<vi>)
      n5 = control-ref of="Configure"() -> (w75:refnum<vi>)
      n6 = control-ref of="Home"() -> (w74:refnum<vi>)
      n7 = control-ref of="EXIT"() -> (w73:refnum<vi>)
      n8 = control-ref of="service 2"() -> (w72:refnum<vi>)
      n9 = control-ref of="Analysis"() -> (w70:refnum<vi>)
      n10 = Bundle By Name(cluster=w68, "Main Home Screen.GUI"=w77, "Main Home Screen.Platform Settings"=w76, "Main Home Screen.Configure"=w75, "Main Home Screen.Home"=w74, "Main Home Screen.EXIT"=w73, "Main Home Screen.service 2"=w72, "Main Home Screen.MainPage"=w71, "Main Home Screen.Analysis"=w70) -> (w69:T11)
    }
    frame #1 {
      n11 = control-ref of="Sway Right Main"() -> (w88:refnum<vi>)
      n12 = control-ref of="Sway Left Main"() -> (w87:refnum<vi>)
      n13 = control-ref of="Heave Down Main"() -> (w86:refnum<vi>)
      n14 = control-ref of="Heave Up main"() -> (w85:refnum<vi>)
      n15 = control-ref of="Update Sway Speed"() -> (w84:refnum<vi>)
      n16 = control-ref of="Update Heave Speed"() -> (w83:refnum<vi>)
      n17 = control-ref of="Surge Backward Main"() -> (w79:refnum<vi>)
      n18 = control-ref of="Update Surge Speed"() -> (w96:refnum<vi>)
      n19 = control-ref of="Disable Axis Jog Soft Limits m"() -> (w94:refnum<vi>)
      n20 = control-ref of="Sway and Surge COM Status"() -> (w92:refnum<vi>)
      n21 = control-ref of="Heave COM Status"() -> (w91:refnum<vi>)
      n22 = control-ref of="Enable Platform"() -> (w90:refnum<vi>)
      n23 = control-ref of="Surge Forward Main"() -> (w89:refnum<vi>)
      n24 = control-ref of="mm/s Heave"() -> (w82:refnum<vi>)
      n25 = control-ref of="mm/sec"() -> (w81:refnum<vi>)
      n26 = control-ref of="mm"() -> (w80:refnum<vi>)
      n27 = control-ref of="mm/s  Surge"() -> (w97:refnum<vi>)
      n28 = control-ref of="mm/s  Sway"() -> (w93:refnum<vi>)
      n29 = control-ref of="Drive Error"() -> (w95:refnum<vi>)
      n30 = Bundle By Name(cluster=w98, "Platform Settings.mm/s  Surge"=w97, "Platform Settings.Update Surge Speed"=w96, "Platform Settings.Drive Error"=w95, "Platform Settings.Disable Axis Jog Soft Limits"=w94, "Platform Settings.mm/s  Sway"=w93, "Platform Settings.Sway and Surge COM Status"=w92, "Platform Settings.Heave COM Status"=w91, "Platform Settings.Enable Platform"=w90, "Platform Settings.Surge Forward Main"=w89, "Platform Settings.Sway Right Main"=w88, "Platform Settings.Sway Left Main"=w87, "Platform Settings.Heave Down Main"=w86, "Platform Settings.Heave Up main"=w85, "Platform Settings.Update Sway Speed"=w84, "Platform Settings.Update Heave Speed"=w83, "Platform Settings.mm/s Heave"=w82, "Platform Settings.mm/sec"=w81, "Platform Settings.mm"=w80, "Platform Settings.Surge Backward Main"=w79) -> (w78:T11)
    }
    frame #2 {
      n31 = control-ref of="Analysis Home"() -> (w104:refnum<vi>)
      n32 = control-ref of="Surface Analysis"() -> (w103:refnum<vi>)
      n33 = control-ref of="Imaging"() -> (w102:refnum<vi>)
      n34 = control-ref of="Image Analysis"() -> (w101:refnum<vi>)
      n35 = control-ref of="Post Analysis"() -> (w100:refnum<vi>)
      n36 = Bundle By Name(cluster=w105, "Analysis Screen.Analysis Home"=w104, "Analysis Screen.Surface Analysis"=w103, "Analysis Screen.Imaging"=w102, "Analysis Screen.Image Analysis"=w101, "Analysis Screen.Post Analysis"=w100) -> (w99:T11)
    }
    frame #3 {
      n37 = control-ref of="Select Load Head"() -> (w112:refnum<vi>)
      n38 = control-ref of="Auto"() -> (w106:refnum<vi>)
      n39 = control-ref of="Notes :"() -> (w111:refnum<vi>)
      n40 = control-ref of="FILE"() -> (w110:refnum<vi>)
      n41 = control-ref of="Sample ID :"() -> (w109:refnum<vi>)
      n42 = control-ref of="Operator ID :"() -> (w108:refnum<vi>)
      n43 = control-ref of="Operator Name :"() -> (w107:refnum<vi>)
      n44 = Bundle By Name(cluster=w114, "Config Screen.Select Load Head"=w112, "Config Screen.Notes :"=w111, "Config Screen.FILE"=w110, "Config Screen.Sample ID :"=w109, "Config Screen.Operator ID :"=w108, "Config Screen.Operator Name :"=w107, "Config Screen.Auto"=w106) -> (w113:T11)
    }
    frame #4 {
      n45 = control-ref of="Warning"() -> (w142:refnum<vi>)
      n46 = control-ref of="gui GIF"() -> (w141:refnum<vi>)
      n47 = control-ref of="Load Selection"() -> (w115:refnum<vi>)
      n48 = control-ref of="Warning 2"() -> (w146:refnum<vi>)
      n49 = control-ref of="SSP 0.75"() -> (w145:refnum<vi>)
      n50 = control-ref of="SSP 0.5"() -> (w144:refnum<vi>)
      n51 = control-ref of="SSP 0.3"() -> (w143:refnum<vi>)
      n52 = control-ref of="Communication is established"() -> (w140:refnum<vi>)
      n53 = control-ref of="AppLoad 4"() -> (w139:refnum<vi>)
      n54 = control-ref of="Multipoint"() -> (w138:refnum<vi>)
      n55 = control-ref of="com 3"() -> (w134:refnum<vi>)
      n56 = control-ref of="com"() -> (w133:refnum<vi>)
      n57 = control-ref of="DecaForce COM Status"() -> (w132:refnum<vi>)
      n58 = control-ref of="Update"() -> (w131:refnum<vi>)
      n59 = control-ref of="Clear 3"() -> (w130:refnum<vi>)
      n60 = control-ref of="seq"() -> (w129:refnum<vi>)
      n61 = control-ref of="Stribeck table"() -> (w128:refnum<vi>)
      n62 = control-ref of="KiloForce"() -> (w120:refnum<vi>)
      n63 = control-ref of="DecaForce"() -> (w119:refnum<vi>)
      n64 = control-ref of="MicroForce"() -> (w118:refnum<vi>)
      n65 = control-ref of="LHBack"() -> (w117:refnum<vi>)
      n66 = control-ref of="LHNext"() -> (w116:refnum<vi>)
      n67 = control-ref of="Enter the Loading Rate (N/min)"() -> (w148:refnum<vi>)
      n68 = control-ref of="Enter the Final Load (N)"() -> (w125:refnum<vi>)
      n69 = control-ref of="Enter the CoF Trip"() -> (w124:refnum<vi>)
      n70 = control-ref of="Enter the Friction Force Trip"() -> (w123:refnum<vi>)
      n71 = control-ref of="Enter the Normal load Trip"() -> (w122:refnum<vi>)
      n72 = control-ref of="Enter the Load  (N)"() -> (w121:refnum<vi>)
      n73 = control-ref of="Message"() -> (w147:refnum<vi>)
      n74 = control-ref of="Indentation"() -> (w137:refnum<vi>)
      n75 = control-ref of="Stribeck Table  For loading"() -> (w127:refnum<vi>)
      n76 = control-ref of="Reference Sample"() -> (w136:refnum<vi>)
      n77 = control-ref of="Load Cell Communication Slide"() -> (w135:refnum<vi>)
      n78 = control-ref of="Loading Mode"() -> (w126:refnum<vi>)
      n79 = Bundle By Name(cluster=w150, "Loading.Enter the Loading Rate (N/min)"=w148, "Loading.Message"=w147, "Loading.Warning 2"=w146, "Loading.SSP 0.75"=w145, "Loading.SSP 0.5"=w144, "Loading.SSP 0.3"=w143, "Loading.Warning"=w142, "Loading.gui GIF"=w141, "Loading.Communication is established"=w140, "Loading.AppLoad 4"=w139, "Loading.Multipoint"=w138, "Loading.Indentation"=w137, "Loading.Reference Sample"=w136, "Loading.Load Cell Communication Slide"=w135, "Loading.com 3"=w134, "Loading.com"=w133, "Loading.DecaForce COM Status"=w132, "Loading.Update"=w131, "Loading.Clear 3"=w130, "Loading.seq"=w129, "Loading.Stribeck table"=w128, "Loading.Stribeck Table  For loading"=w127, "Loading.Loading Mode"=w126, "Loading.Enter the Final Load (N)"=w125, "Loading.Enter the CoF Trip"=w124, "Loading.Enter the Friction Force Trip"=w123, "Loading.Enter the Normal load Trip"=w122, "Loading.Enter the Load  (N)"=w121, "Loading.KiloForce"=w120, "Loading.DecaForce"=w119, "Loading.MicroForce"=w118, "Loading.LHBack"=w117, "Loading.LHNext"=w116, "Loading.Load Selection"=w115) -> (w149:T11)
    }
    frame #5 {
      n80 = control-ref of="TEST SELECTION"() -> (w202:refnum<vi>)
      n81 = control-ref of="SPEED SELECTION :"() -> (w201:refnum<vi>)
      n82 = control-ref of="SPEED SELECTION : rotary"() -> (w168:refnum<vi>)
      n83 = control-ref of="Rotary Tab"() -> (w217:refnum<vi>)
      n84 = control-ref of="e.v/ssr 2"() -> (w214:refnum<vi>)
      n85 = control-ref of="Step Speed"() -> (w198:refnum<vi>)
      n86 = control-ref of="M3 Image"() -> (w193:refnum<vi>)
      n87 = control-ref of="Rotary Module Selection"() -> (w170:refnum<vi>)
      n88 = control-ref of="zNL"() -> (w219:refnum<vi>)
      n89 = control-ref of="E.Velocity 2"() -> (w215:refnum<vi>)
      n90 = control-ref of="Ramp Up 2"() -> (w203:refnum<vi>)
      n91 = control-ref of="Angular Oscillation Set"() -> (w200:refnum<vi>)
      n92 = control-ref of="Traction"() -> (w199:refnum<vi>)
      n93 = control-ref of="Surge Forward MM"() -> (w195:refnum<vi>)
      n94 = control-ref of="Surge Backward MM"() -> (w194:refnum<vi>)
      n95 = control-ref of="Sway Left MM"() -> (w191:refnum<vi>)
      n96 = control-ref of="Sway Right MM"() -> (w190:refnum<vi>)
      n97 = control-ref of="Disable Axis Jog Soft Limits"() -> (w189:refnum<vi>)
      n98 = control-ref of="Heave Down MM"() -> (w187:refnum<vi>)
      n99 = control-ref of="Heave Up MM"() -> (w186:refnum<vi>)
      n100 = control-ref of="Set WTD"() -> (w184:refnum<vi>)
      n101 = control-ref of="HomeScratch"() -> (w183:refnum<vi>)
      n102 = control-ref of="HomeRot"() -> (w182:refnum<vi>)
      n103 = control-ref of="PlaceModule"() -> (w181:refnum<vi>)
      n104 = control-ref of="LR Sway"() -> (w177:refnum<vi>)
      n105 = control-ref of="Rot Hor"() -> (w176:refnum<vi>)
      n106 = control-ref of="Scratch"() -> (w175:refnum<vi>)
      n107 = control-ref of="LR Cam"() -> (w174:refnum<vi>)
      n108 = control-ref of="MMBack"() -> (w173:refnum<vi>)
      n109 = control-ref of="MMNext"() -> (w172:refnum<vi>)
      n110 = control-ref of="Rot Ver"() -> (w171:refnum<vi>)
      n111 = control-ref of="calculate rotary"() -> (w169:refnum<vi>)
      n112 = control-ref of="Import 2"() -> (w167:refnum<vi>)
      n113 = control-ref of="Save 2"() -> (w166:refnum<vi>)
      n114 = control-ref of="SwaySpeed Set"() -> (w159:refnum<vi>)
      n115 = control-ref of="HomeScratch"() -> (w155:refnum<vi>)
      n116 = control-ref of="NL disp"() -> (w218:refnum<vi>)
      n117 = control-ref of="Enter Fixed E.Velocity 2"() -> (w213:refnum<vi>)
      n118 = control-ref of="Enter Final SRR 2"() -> (w212:refnum<vi>)
      n119 = control-ref of="Enter initial SRR 2"() -> (w211:refnum<vi>)
      n120 = control-ref of="Enter Fixed SRR 2"() -> (w210:refnum<vi>)
      n121 = control-ref of="Enter the Final E.Velocity (m/s) 2"() -> (w209:refnum<vi>)
      n122 = control-ref of="Enter initial E.Velocity (m/s) 2"() -> (w208:refnum<vi>)
      n123 = control-ref of="Final Speed (RPM) 3"() -> (w207:refnum<vi>)
      n124 = control-ref of="Initial Speed (RPM) 2"() -> (w206:refnum<vi>)
      n125 = control-ref of="Enter the Final Velocity (m/s) 3"() -> (w205:refnum<vi>)
      n126 = control-ref of="Enter initial Velocity (m/s)  3"() -> (w204:refnum<vi>)
      n127 = control-ref of="mm"() -> (w188:refnum<vi>)
      n128 = control-ref of="Wear Track Diameter (mm)"() -> (w185:refnum<vi>)
      n129 = control-ref of="Enter the Angle (Deg)"() -> (w180:refnum<vi>)
      n130 = control-ref of="Enter the Frequency (Hz)"() -> (w179:refnum<vi>)
      n131 = control-ref of="Enter the Speed(mm/sec)"() -> (w162:refnum<vi>)
      n132 = control-ref of="Enter the Speed (RPM)"() -> (w161:refnum<vi>)
      n133 = control-ref of="Enter Scratch Speed (mm/s):"() -> (w160:refnum<vi>)
      n134 = control-ref of="Scartch Offset"() -> (w158:refnum<vi>)
      n135 = control-ref of="Enter Scratch length (mm):"() -> (w154:refnum<vi>)
      n136 = control-ref of="Wear Track Diameter"() -> (w153:refnum<vi>)
      n137 = control-ref of="No of Scratch"() -> (w151:refnum<vi>)
      n138 = control-ref of="String 39"() -> (w192:refnum<vi>)
      n139 = control-ref of="String 45"() -> (w164:refnum<vi>)
      n140 = control-ref of="Rotary Speed Exced"() -> (w152:refnum<vi>)
      n141 = control-ref of="StepTable For Load-Speed"() -> (w197:refnum<vi>)
      n142 = control-ref of="StepTable For Speed"() -> (w196:refnum<vi>)
      n143 = control-ref of="StepTable For Speed 3"() -> (w163:refnum<vi>)
      n144 = control-ref of="Motion Direction:  3"() -> (w216:refnum<vi>)
      n145 = control-ref of="Motion Mode:"() -> (w178:refnum<vi>)
      n146 = control-ref of="Scratch Mode"() -> (w157:refnum<vi>)
      n147 = control-ref of="Motion type:"() -> (w156:refnum<vi>)
      n148 = control-ref of="File Path :  2"() -> (w165:refnum<vi>)
      n149 = Bundle By Name(cluster=w221, "Motion Module.zNL"=w219, "Motion Module.NL disp"=w218, "Motion Module.Rotary Tab"=w217, "Motion Module.Motion Direction:  3"=w216, "Motion Module.E.Velocity 2"=w215, "Motion Module.e.v/ssr 2"=w214, "Motion Module.Enter Fixed E.Velocity 2"=w213, "Motion Module.Enter Final SRR 2"=w212, "Motion Module.Enter initial SRR 2"=w211, "Motion Module.Enter Fixed SRR 2"=w210, "Motion Module.Enter the Final E.Velocity (m/s) 2"=w209, "Motion Module.Enter initial E.Velocity (m/s) 2"=w208, "Motion Module.Final Speed (RPM) 3"=w207, "Motion Module.Initial Speed (RPM) 2"=w206, "Motion Module.Enter the Final Velocity (m/s) 3"=w205, "Motion Module.Enter initial Velocity (m/s)  3"=w204, "Motion Module.Ramp Up 2"=w203, "Motion Module.TEST SELECTION"=w202, "Motion Module.SPEED SELECTION :"=w201, "Motion Module.Angular Oscillation Set"=w200, "Motion Module.Traction"=w199, "Motion Module.Step Speed"=w198, "Motion Module.StepTable For Load-Speed"=w197, "Motion Module.StepTable For Speed"=w196, "Motion Module.Surge Forward MM"=w195, "Motion Module.Surge Backward MM"=w194, "Motion Module.M3 Image"=w193, "Motion Module.String 39"=w192, "Motion Module.Sway Left MM"=w191, "Motion Module.Sway Right MM"=w190, "Motion Module.Disable Axis Jog Soft Limits"=w189, "Motion Module.mm"=w188, "Motion Module.Heave Down MM"=w187, "Motion Module.Heave Up MM"=w186, "Motion Module.Wear Track Diameter (mm)"=w185, "Motion Module.Set WTD"=w184, "Motion Module.HomeScratch"=w183, "Motion Module.HomeRot"=w182, "Motion Module.PlaceModule"=w181, "Motion Module.Enter the Angle (Deg)"=w180, "Motion Module.Enter the Frequency (Hz)"=w179, "Motion Module.Motion Mode:"=w178, "Motion Module.LR Sway"=w177, "Motion Module.Rot Hor"=w176, "Motion Module.Scratch"=w175, "Motion Module.LR Cam"=w174, "Motion Module.MMBack"=w173, "Motion Module.MMNext"=w172, "Motion Module.Rot Ver"=w171, "Motion Module.Rotary Module Selection"=w170, "Motion Module.calculate rotary"=w169, "Motion Module.SPEED SELECTION : rotary"=w168, "Motion Module.Import 2"=w167, "Motion Module.Save 2"=w166, "Motion Module.File Path :  2"=w165, "Motion Module.String 45"=w164, "Motion Module.StepTable For Speed 3"=w163, "Motion Module.Enter the Speed(mm/sec)"=w162, "Motion Module.Enter the Speed(RPM)"=w161, "Motion Module.Enter Scratch Speed (mm/s):"=w160, "Motion Module.SwaySpeed Set"=w159, "Motion Module.Scartch Offset"=w158, "Motion Module.Scratch Mode"=w157, "Motion Module.Motion type:"=w156, "Motion Module.HomeScratch 2"=w155, "Motion Module.Enter Scratch length (mm):"=w154, "Motion Module.Wear Track Diameter"=w153, "Motion Module.Rotary Speed Exced"=w152, "Motion Module.No of Scratch"=w151) -> (w220:T11)
    }
    frame #6 {
      n150 = control-ref of="Add to list"() -> (w239:refnum<vi>)
      n151 = control-ref of="Wear"() -> (w238:refnum<vi>)
      n152 = control-ref of="Vibration"() -> (w237:refnum<vi>)
      n153 = control-ref of="Humidity (Chamber)"() -> (w236:refnum<vi>)
      n154 = control-ref of="Temperature (Chamber)"() -> (w235:refnum<vi>)
      n155 = control-ref of="ECR"() -> (w234:refnum<vi>)
      n156 = control-ref of="Temperature (Amb)"() -> (w233:refnum<vi>)
      n157 = control-ref of="Microphone"() -> (w232:refnum<vi>)
      n158 = control-ref of="Acoustic Emission 3"() -> (w231:refnum<vi>)
      n159 = control-ref of="SNext"() -> (w230:refnum<vi>)
      n160 = control-ref of="APBack"() -> (w229:refnum<vi>)
      n161 = control-ref of="Low Temp"() -> (w225:refnum<vi>)
      n162 = control-ref of="High Temp"() -> (w224:refnum<vi>)
      n163 = control-ref of="Humidity"() -> (w223:refnum<vi>)
      n164 = control-ref of="Humidity  Status  3"() -> (w246:refnum<vi>)
      n165 = control-ref of="Low Temp  Status  2"() -> (w245:refnum<vi>)
      n166 = control-ref of="TK4 status 2"() -> (w244:refnum<vi>)
      n167 = control-ref of="Humidity (Amb)"() -> (w241:refnum<vi>)
      n168 = control-ref of="Clear List"() -> (w240:refnum<vi>)
      n169 = control-ref of="Enter the Temperature (°C):"() -> (w228:refnum<vi>)
      n170 = control-ref of="Enter the Stage \nTemperature (°C):"() -> (w227:refnum<vi>)
      n171 = control-ref of="Enter the Humidity (%Rh):"() -> (w226:refnum<vi>)
      n172 = control-ref of="Sensors Picked"() -> (w222:refnum<vi>)
      n173 = control-ref of="Stage Temperature"() -> (w243:refnum<vi>)
      n174 = control-ref of="Sample Temperature"() -> (w242:refnum<vi>)
      n175 = Bundle By Name(cluster=w248, "Environmental control.Humidity  Status  3"=w246, "Environmental control.Low Temp  Status  2"=w245, "Environmental control.TK4 status 2"=w244, "Environmental control.Stage Temperature"=w243, "Environmental control.Sample Temperature"=w242, "Environmental control.Humidity (Amb)"=w241, "Environmental control.Clear List"=w240, "Environmental control.Add to list"=w239, "Environmental control.Wear"=w238, "Environmental control.Vibration"=w237, "Environmental control.Humidity (Chamber)"=w236, "Environmental control.Temperature (Chamber)"=w235, "Environmental control.ECR"=w234, "Environmental control.Temperature (Amb)"=w233, "Environmental control.Microphone"=w232, "Environmental control.Acoustic Emission 3"=w231, "Environmental control.SNext"=w230, "Environmental control.APBack"=w229, "Environmental control.Enter the Temperature (°C):"=w228, "Environmental control.Enter the Stage \nTemperature (°C):"=w227, "Environmental control.Enter the Humidity (%Rh):"=w226, "Environmental control.Low Temp"=w225, "Environmental control.High Temp"=w224, "Environmental control.Humidity"=w223, "Environmental control.Sensors Picked"=w222) -> (w247:T11)
    }
    frame #7 {
      n176 = control-ref of="ECR Port:"() -> (w258:refnum<vi>)
      n177 = control-ref of="Ramp Port:"() -> (w257:refnum<vi>)
      n178 = control-ref of="Heave and Surge COM Port:"() -> (w254:refnum<vi>)
      n179 = control-ref of="Sway COM Port:"() -> (w253:refnum<vi>)
      n180 = control-ref of="Temp Modbus:"() -> (w252:refnum<vi>)
      n181 = control-ref of="Humidity Port:"() -> (w251:refnum<vi>)
      n182 = control-ref of="About Tab"() -> (w259:refnum<vi>)
      n183 = control-ref of="Home Service"() -> (w261:refnum<vi>)
      n184 = control-ref of="Advanced Setting"() -> (w260:refnum<vi>)
      n185 = control-ref of="Installation/Replacement completed"() -> (w256:refnum<vi>)
      n186 = control-ref of="Loahead"() -> (w255:refnum<vi>)
      n187 = control-ref of="Edit Gain Constants"() -> (w250:refnum<vi>)
      n188 = control-ref of="Save Gain Constants"() -> (w249:refnum<vi>)
      n189 = control-ref of="Password"() -> (w262:refnum<vi>)
      n190 = Bundle By Name(cluster=w264, "About Screen.Password"=w262, "About Screen.Home Service"=w261, "About Screen.Advanced Setting"=w260, "About Screen.About Tab"=w259, "About Screen.ECR Port:"=w258, "About Screen.Ramp Port:"=w257, "About Screen.Installation/Replacement completed"=w256, "About Screen.Loahead"=w255, "About Screen.Heave and Surge COM Port:"=w254, "About Screen.Sway COM Port:"=w253, "About Screen.Temp Modbus:"=w252, "About Screen.Humidity Port:"=w251, "About Screen.Edit Gain Constants"=w250, "About Screen.Save Gain Constants"=w249) -> (w263:T11)
    }
    frame #8 {
      n191 = control-ref of="Cyclic Friction Force (N) Graph"() -> (w275:refnum<vi>)
      n192 = control-ref of="Cyclic Coefficient of Friction"() -> (w274:refnum<vi>)
      n193 = control-ref of="SDGp"() -> (w323:refnum<vi>)
      n194 = control-ref of="HumrGp"() -> (w321:refnum<vi>)
      n195 = control-ref of="gACQUOS"() -> (w318:refnum<vi>)
      n196 = control-ref of="ECR"() -> (w316:refnum<vi>)
      n197 = control-ref of="Temperature (deg c)"() -> (w314:refnum<vi>)
      n198 = control-ref of="MTM DISC  SPEED"() -> (w311:refnum<vi>)
      n199 = control-ref of="MTM BALL SPEED"() -> (w310:refnum<vi>)
      n200 = control-ref of="speed mm/sec"() -> (w309:refnum<vi>)
      n201 = control-ref of="WearGp"() -> (w299:refnum<vi>)
      n202 = control-ref of="Main Chart 3"() -> (w293:refnum<vi>)
      n203 = control-ref of="Friction Force (N) Graph"() -> (w281:refnum<vi>)
      n204 = control-ref of="Coefficient of Friction"() -> (w280:refnum<vi>)
      n205 = control-ref of="Main Screen Tab"() -> (w382:refnum<vi>)
      n206 = control-ref of="Angle and Frequency"() -> (w381:refnum<vi>)
      n207 = control-ref of="Main Speed Tab"() -> (w378:refnum<vi>)
      n208 = control-ref of="MTM MOTOR DISPLAY"() -> (w377:refnum<vi>)
      n209 = control-ref of="SPEED TAB"() -> (w372:refnum<vi>)
      n210 = control-ref of="Time Tab"() -> (w367:refnum<vi>)
      n211 = control-ref of="Temp Tabs"() -> (w360:refnum<vi>)
      n212 = control-ref of="Grp Tab"() -> (w327:refnum<vi>)
      n213 = control-ref of="Sub Graph"() -> (w326:refnum<vi>)
      n214 = control-ref of="Speed Tab"() -> (w312:refnum<vi>)
      n215 = control-ref of="FF Tab"() -> (w278:refnum<vi>)
      n216 = control-ref of="CZ FF"() -> (w276:refnum<vi>)
      n217 = control-ref of="Cyclic FF Disable Trip"() -> (w272:refnum<vi>)
      n218 = control-ref of="cyclic COF Disable Trip"() -> (w271:refnum<vi>)
      n219 = control-ref of="cyclic COF Reset Graph"() -> (w269:refnum<vi>)
      n220 = control-ref of="Cyclic FF Reset Graph"() -> (w268:refnum<vi>)
      n221 = control-ref of="Test Trip"() -> (w267:refnum<vi>)
      n222 = control-ref of="Scratch Start Test"() -> (w279:refnum<vi>)
      n223 = control-ref of="Scratch Start Recording"() -> (w265:refnum<vi>)
      n224 = control-ref of="Heater"() -> (w359:refnum<vi>)
      n225 = control-ref of="TK4 status"() -> (w358:refnum<vi>)
      n226 = control-ref of="Controller  Status"() -> (w355:refnum<vi>)
      n227 = control-ref of="Cooling"() -> (w352:refnum<vi>)
      n228 = control-ref of="Load Communication"() -> (w351:refnum<vi>)
      n229 = control-ref of="HumCOMStatus"() -> (w349:refnum<vi>)
      n230 = control-ref of="Load En"() -> (w346:refnum<vi>)
      n231 = control-ref of="NLt"() -> (w345:refnum<vi>)
      n232 = control-ref of="zNL 2"() -> (w344:refnum<vi>)
      n233 = control-ref of="Humidity On"() -> (w343:refnum<vi>)
      n234 = control-ref of="AppLoadSeq scratch"() -> (w339:refnum<vi>)
      n235 = control-ref of="Stop Scratch"() -> (w338:refnum<vi>)
      n236 = control-ref of="ClrLog"() -> (w337:refnum<vi>)
      n237 = control-ref of="STOP"() -> (w335:refnum<vi>)
      n238 = control-ref of="Start Test"() -> (w334:refnum<vi>)
      n239 = control-ref of="Test status"() -> (w333:refnum<vi>)
      n240 = control-ref of="AR Led"() -> (w332:refnum<vi>)
      n241 = control-ref of="Data"() -> (w331:refnum<vi>)
      n242 = control-ref of="Health"() -> (w330:refnum<vi>)
      n243 = control-ref of="Sway COM Status"() -> (w329:refnum<vi>)
      n244 = control-ref of="Heave COM Status"() -> (w328:refnum<vi>)
      n245 = control-ref of="Siliding distance Reset Graph"() -> (w324:refnum<vi>)
      n246 = control-ref of="Humidity Reset Graph"() -> (w322:refnum<vi>)
      n247 = control-ref of="Aqucostic Reset Graph"() -> (w319:refnum<vi>)
      n248 = control-ref of="ECR RESET"() -> (w317:refnum<vi>)
      n249 = control-ref of="Temperature Reset"() -> (w315:refnum<vi>)
      n250 = control-ref of="Speed Reset Graph"() -> (w313:refnum<vi>)
      n251 = control-ref of="Hymidity"() -> (w308:refnum<vi>)
      n252 = control-ref of="Humidity Disable trip"() -> (w307:refnum<vi>)
      n253 = control-ref of="Weart Deapth"() -> (w304:refnum<vi>)
      n254 = control-ref of="Depth Reset Graph"() -> (w303:refnum<vi>)
      n255 = control-ref of="Weart"() -> (w302:refnum<vi>)
      n256 = control-ref of="Depthz"() -> (w301:refnum<vi>)
      n257 = control-ref of="Load pid"() -> (w297:refnum<vi>)
      n258 = control-ref of="Load Disable Trip"() -> (w296:refnum<vi>)
      n259 = control-ref of="Load Reset Graph"() -> (w295:refnum<vi>)
      n260 = control-ref of="BACK"() -> (w292:refnum<vi>)
      n261 = control-ref of="zFF"() -> (w282:refnum<vi>)
      n262 = control-ref of="FF Reset Graph"() -> (w288:refnum<vi>)
      n263 = control-ref of="FF Disable Trip"() -> (w287:refnum<vi>)
      n264 = control-ref of="COF Disable Trip"() -> (w285:refnum<vi>)
      n265 = control-ref of="COF Reset Graph"() -> (w284:refnum<vi>)
      n266 = control-ref of="Start Test Temp"() -> (w283:refnum<vi>)
      n267 = control-ref of="Depth Trip"() -> (w291:refnum<vi>)
      n268 = control-ref of="Multi Scratch Pass"() -> (w266:refnum<vi>)
      n269 = control-ref of="Cyclic Friction Force (N)"() -> (w277:refnum<vi>)
      n270 = control-ref of="Cyclic FF TRIP"() -> (w273:refnum<vi>)
      n271 = control-ref of="cyclic COF TRIP"() -> (w270:refnum<vi>)
      n272 = control-ref of="Stroke (mm)"() -> (w380:refnum<vi>)
      n273 = control-ref of="Angle (Deg)"() -> (w379:refnum<vi>)
      n274 = control-ref of="Disc Speed (m/sec)"() -> (w376:refnum<vi>)
      n275 = control-ref of="Ball Speed (m/sec)"() -> (w375:refnum<vi>)
      n276 = control-ref of="Disc Speed (RPM)"() -> (w374:refnum<vi>)
      n277 = control-ref of="Ball Speed (RPM)"() -> (w373:refnum<vi>)
      n278 = control-ref of="Speed (m/sec)"() -> (w371:refnum<vi>)
      n279 = control-ref of="Set Speed (m/sec)"() -> (w370:refnum<vi>)
      n280 = control-ref of="Speed (RPM)"() -> (w369:refnum<vi>)
      n281 = control-ref of="Set Speed"() -> (w368:refnum<vi>)
      n282 = control-ref of="Time ( HH:MM:SS ) 2"() -> (w366:refnum<vi>)
      n283 = control-ref of="Test Duration"() -> (w365:refnum<vi>)
      n284 = control-ref of="Test Duration 4"() -> (w364:refnum<vi>)
      n285 = control-ref of="TEST CYCLE"() -> (w363:refnum<vi>)
      n286 = control-ref of="TOTAL CYCLES"() -> (w362:refnum<vi>)
      n287 = control-ref of="Set Load (N)"() -> (w361:refnum<vi>)
      n288 = control-ref of="ChamberTemp"() -> (w357:refnum<vi>)
      n289 = control-ref of="SetTmp"() -> (w356:refnum<vi>)
      n290 = control-ref of="ChamberTemp"() -> (w354:refnum<vi>)
      n291 = control-ref of="SetTmp"() -> (w353:refnum<vi>)
      n292 = control-ref of="Ambient \nTemperature"() -> (w350:refnum<vi>)
      n293 = control-ref of="Ambient\n Humidity"() -> (w348:refnum<vi>)
      n294 = control-ref of="Freq (Hz)"() -> (w347:refnum<vi>)
      n295 = control-ref of="humidity disp"() -> (w342:refnum<vi>)
      n296 = control-ref of="Set Humidity"() -> (w341:refnum<vi>)
      n297 = control-ref of="NL disp 2"() -> (w340:refnum<vi>)
      n298 = control-ref of="SD (mm)"() -> (w325:refnum<vi>)
      n299 = control-ref of="Acoustic Emission (mV)"() -> (w320:refnum<vi>)
      n300 = control-ref of="CoF Trip  2"() -> (w306:refnum<vi>)
      n301 = control-ref of="Depth Trip"() -> (w305:refnum<vi>)
      n302 = control-ref of="Depth (µm)"() -> (w300:refnum<vi>)
      n303 = control-ref of="NL Trip 2"() -> (w298:refnum<vi>)
      n304 = control-ref of="NL Display 4"() -> (w294:refnum<vi>)
      n305 = control-ref of="COF TRIP"() -> (w290:refnum<vi>)
      n306 = control-ref of="Friction Force (N)"() -> (w289:refnum<vi>)
      n307 = control-ref of="FF TRIP"() -> (w286:refnum<vi>)
      n308 = control-ref of="Trip Log"() -> (w336:refnum<vi>)
      n309 = Bundle By Name(cluster=w384, "Main Screen.Test Trip"=w267, "Main Screen.Main Screen Tab"=w382, "Main Screen.Angle and Frequency"=w381, "Main Screen.Stroke (mm)"=w380, "Main Screen.Angle (Deg)"=w379, "Main Screen.Main Speed Tab"=w378, "Main Screen.MTM MOTOR DISPLAY"=w377, "Main Screen.Disc Speed (m/sec)"=w376, "Main Screen.Ball Speed (m/sec)"=w375, "Main Screen.Disc Speed (RPM)"=w374, "Main Screen.Ball Speed (RPM)"=w373, "Main Screen.SPEED TAB"=w372, "Main Screen.Speed (m/sec)"=w371, "Main Screen.Set Speed (m/sec)"=w370, "Main Screen.Speed (RPM)"=w369, "Main Screen.Set Speed"=w368, "Main Screen.Time Tab"=w367, "Main Screen.Time ( HH:MM:SS ) 2"=w366, "Main Screen.Test Duration"=w365, "Main Screen.Test Duration 4"=w364, "Main Screen.TEST CYCLE"=w363, "Main Screen.TOTAL CYCLES"=w362, "Main Screen.Set Load (N)"=w361, "Main Screen.Temp Tabs"=w360, "Main Screen.Heater"=w359, "Main Screen.TK4 status"=w358, "Main Screen.ChamberTemp"=w357, "Main Screen.SetTmp"=w356, "Main Screen.Controller  Status"=w355, "Main Screen.ChamberTemp 2"=w354, "Main Screen.SetTmp 2"=w353, "Main Screen.Cooling"=w352, "Main Screen.Load Communication"=w351, "Main Screen.Ambient \nTemperature"=w350, "Main Screen.HumCOMStatus"=w349, "Main Screen.Ambient\n Humidity"=w348, "Main Screen.Freq (Hz)"=w347, "Main Screen.Load En"=w346, "Main Screen.NLt"=w345, "Main Screen.zNL 2"=w344, "Main Screen.Humidity On"=w343, "Main Screen.humidity disp"=w342, "Main Screen.Set Humidity"=w341, "Main Screen.NL disp 2"=w340, "Main Screen.AppLoadSeq scratch"=w339, "Main Screen.Stop Scratch"=w338, "Main Screen.ClrLog"=w337, "Main Screen.Trip Log"=w336, "Main Screen.STOP"=w335, "Main Screen.Start Test"=w334, "Main Screen.Test status"=w333, "Main Screen.AR Led"=w332, "Main Screen.Data"=w331, "Main Screen.Health"=w330, "Main Screen.Sway COM Status"=w329, "Main Screen.Heave COM Status"=w328, "Main Screen.Grp Tab"=w327, "Main Screen.Sub Graph"=w326, "Main Screen.SD (mm)"=w325, "Main Screen.Siliding distance Reset Graph"=w324, "Main Screen.SDGp"=w323, "Main Screen.Humidity Reset Graph"=w322, "Main Screen.HumrGp"=w321, "Main Screen.Acoustic Emission (mV)"=w320, "Main Screen.Aqucostic Reset Graph"=w319, "Main Screen.gACQUOS"=w318, "Main Screen.ECR RESET"=w317, "Main Screen.ECR"=w316, "Main Screen.Temperature Reset"=w315, "Main Screen.Temperature (deg c)"=w314, "Main Screen.Speed Reset Graph"=w313, "Main Screen.Speed Tab"=w312, "Main Screen.MTM DISC  SPEED"=w311, "Main Screen.MTM BALL SPEED"=w310, "Main Screen.speed mm/sec"=w309, "Main Screen.Hymidity"=w308, "Main Screen.Humidity Disable trip"=w307, "Main Screen.CoF Trip  2"=w306, "Main Screen.Depth Trip"=w305, "Main Screen.Weart Deapth"=w304, "Main Screen.Depth Reset Graph"=w303, "Main Screen.Weart"=w302, "Main Screen.Depthz"=w301, "Main Screen.Depth (µm)"=w300, "Main Screen.WearGp"=w299, "Main Screen.NL Trip 2"=w298, "Main Screen.Load pid"=w297, "Main Screen.Load Disable Trip"=w296, "Main Screen.Load Reset Graph"=w295, "Main Screen.NL Display 4"=w294, "Main Screen.Main Chart 3"=w293, "Main Screen.BACK"=w292, "Main Screen.Depth Trip 2"=w291, "Main Screen.COF TRIP"=w290, "Main Screen.Friction Force (N)"=w289, "Main Screen.FF Reset Graph"=w288, "Main Screen.FF Disable Trip"=w287, "Main Screen.FF TRIP"=w286, "Main Screen.COF Disable Trip"=w285, "Main Screen.COF Reset Graph"=w284, "Main Screen.FF Tab"=w278, "Main Screen.Start Test Temp"=w283, "Main Screen.zFF"=w282, "Main Screen.Friction Force (N) Graph"=w281, "Main Screen.Coefficient of Friction"=w280, "Main Screen.Scratch Start Test"=w279, "Main Screen.Cyclic Friction Force (N)"=w277, "Main Screen.CZ FF"=w276, "Main Screen.Cyclic Friction Force (N) Graph"=w275, "Main Screen.Cyclic Coefficient of Friction"=w274, "Main Screen.Cyclic FF TRIP"=w273, "Main Screen.Cyclic FF Disable Trip"=w272, "Main Screen.cyclic COF Disable Trip"=w271, "Main Screen.cyclic COF TRIP"=w270, "Main Screen.cyclic COF Reset Graph"=w269, "Main Screen.Cyclic FF Reset Graph"=w268, "Main Screen.Multi Scratch Pass"=w266, "Main Screen.Scratch Start Recording"=w265) -> (w383:T11)
    }
    frame #9 {
      n310 = control-ref of="gFF Rot 7"() -> (w388:refnum<vi>)
      n311 = control-ref of="Ramp"() -> (w407:refnum<vi>)
      n312 = control-ref of="Dummy Run"() -> (w401:refnum<vi>)
      n313 = control-ref of="AutoTune"() -> (w399:refnum<vi>)
      n314 = control-ref of="apply load"() -> (w397:refnum<vi>)
      n315 = control-ref of="reinit 3"() -> (w395:refnum<vi>)
      n316 = control-ref of="Bypass Load"() -> (w392:refnum<vi>)
      n317 = control-ref of="PID gains out delay (microForce)"() -> (w408:refnum<vi>)
      n318 = control-ref of="output range delay"() -> (w394:refnum<vi>)
      n319 = control-ref of="PID gains out delay"() -> (w393:refnum<vi>)
      n320 = control-ref of="Ramp MulFac"() -> (w412:refnum<vi>)
      n321 = control-ref of="pulses LoadDiffRamp(2..10)"() -> (w411:refnum<vi>)
      n322 = control-ref of="PulseControlRamp(diff<=3N)"() -> (w410:refnum<vi>)
      n323 = control-ref of="SetLoadDeadband(%) Load(0-10N)"() -> (w409:refnum<vi>)
      n324 = control-ref of="Gain 2"() -> (w406:refnum<vi>)
      n325 = control-ref of="pulses LoadDiff(2..10)"() -> (w405:refnum<vi>)
      n326 = control-ref of="pulses LoadDiff(11..50)"() -> (w404:refnum<vi>)
      n327 = control-ref of="PulseControl(diff<=3N)"() -> (w403:refnum<vi>)
      n328 = control-ref of="SetLoadDeadband(%)  2"() -> (w402:refnum<vi>)
      n329 = control-ref of="Vertical load (N)"() -> (w400:refnum<vi>)
      n330 = control-ref of="Offset  3"() -> (w398:refnum<vi>)
      n331 = control-ref of="Enter ByPass Load"() -> (w396:refnum<vi>)
      n332 = control-ref of="pulsesSent"() -> (w391:refnum<vi>)
      n333 = control-ref of="pulses"() -> (w390:refnum<vi>)
      n334 = control-ref of="actpid"() -> (w389:refnum<vi>)
      n335 = control-ref of="pulses LoadDiff(21..1000)"() -> (w387:refnum<vi>)
      n336 = control-ref of="Delay"() -> (w386:refnum<vi>)
      n337 = control-ref of="deadband"() -> (w385:refnum<vi>)
      n338 = Bundle By Name(cluster=w414, "PID.Ramp MulFac"=w412, "PID.pulses LoadDiffRamp(2..10)"=w411, "PID.PulseControlRamp(diff<=3N)"=w410, "PID.SetLoadDeadband(%) Load(0-10N)"=w409, "PID.PID gains out delay (microForce)"=w408, "PID.Ramp"=w407, "PID.Gain 2"=w406, "PID.pulses LoadDiff(2..10)"=w405, "PID.pulses LoadDiff(11..50)"=w404, "PID.PulseControl(diff<=3N)"=w403, "PID.SetLoadDeadband(%)  2"=w402, "PID.Dummy Run"=w401, "PID.Vertical load (N)"=w400, "PID.AutoTune"=w399, "PID.Offset 3"=w398, "PID.apply load"=w397, "PID.Enter ByPass Load"=w396, "PID.reinit 3"=w395, "PID.output range delay"=w394, "PID.PID gains out delay"=w393, "PID.Bypass Load"=w392, "PID.pulsesSent"=w391, "PID.pulses"=w390, "PID.actpid"=w389, "PID.gFF Rot"=w388, "PID.pulses LoadDiff(21..1000)"=w387, "PID.Delay"=w386, "PID.deadband"=w385) -> (w413:T11)
    }
    frame #10 {
      n339 = control-ref of="Tab Control 3"() -> (w477:refnum<vi>)
      n340 = control-ref of="Tab Control 19"() -> (w476:refnum<vi>)
      n341 = control-ref of="Tab Control 5"() -> (w437:refnum<vi>)
      n342 = control-ref of="Tab Control 14"() -> (w436:refnum<vi>)
      n343 = control-ref of="Tab Control 26"() -> (w435:refnum<vi>)
      n344 = control-ref of="DEPTH TRIP   ENABLE"() -> (w424:refnum<vi>)
      n345 = control-ref of="LOAD TRIP  ENABLE"() -> (w423:refnum<vi>)
      n346 = control-ref of="CYCLIC COF TRIP  ENABLE"() -> (w418:refnum<vi>)
      n347 = control-ref of="CYCLIC FF TRIP  ENABLE"() -> (w417:refnum<vi>)
      n348 = control-ref of="FF TRIP  ENABLE"() -> (w416:refnum<vi>)
      n349 = control-ref of="COF TRIP  ENABLE"() -> (w415:refnum<vi>)
      n350 = control-ref of="Re-initilaize"() -> (w474:refnum<vi>)
      n351 = control-ref of="Filter ON/OFF"() -> (w473:refnum<vi>)
      n352 = control-ref of="Apply Filter (FF)"() -> (w469:refnum<vi>)
      n353 = control-ref of="Apply Filter (Load)"() -> (w467:refnum<vi>)
      n354 = control-ref of="SAVE  2"() -> (w462:refnum<vi>)
      n355 = control-ref of="Enter Distance"() -> (w461:refnum<vi>)
      n356 = control-ref of="AE"() -> (w434:refnum<vi>)
      n357 = control-ref of="Heave Loop Delay"() -> (w433:refnum<vi>)
      n358 = control-ref of="Heave PID Speed"() -> (w432:refnum<vi>)
      n359 = control-ref of="Surge Jog Speed"() -> (w431:refnum<vi>)
      n360 = control-ref of="Heave Jog Speed"() -> (w430:refnum<vi>)
      n361 = control-ref of="Sway Loop Delay"() -> (w429:refnum<vi>)
      n362 = control-ref of="Sway PID Speed"() -> (w428:refnum<vi>)
      n363 = control-ref of="Sway Jog Speed"() -> (w427:refnum<vi>)
      n364 = control-ref of="DEPTH TRIP VALUE"() -> (w426:refnum<vi>)
      n365 = control-ref of="LOAD TRIP VALUE"() -> (w425:refnum<vi>)
      n366 = control-ref of="CYCLIC FF TRIP VALUE"() -> (w422:refnum<vi>)
      n367 = control-ref of="FF TRIP VALUE"() -> (w421:refnum<vi>)
      n368 = control-ref of="CYCLIC CoF TRIP VALUE"() -> (w420:refnum<vi>)
      n369 = control-ref of="COF TRIP VALUE"() -> (w419:refnum<vi>)
      n370 = control-ref of="SAMPLES"() -> (w475:refnum<vi>)
      n371 = control-ref of="TracHomeSurgeOffsetCounts 10MM"() -> (w472:refnum<vi>)
      n372 = control-ref of="TracHomeSwayOffsetCounts 10MM"() -> (w471:refnum<vi>)
      n373 = control-ref of="Acoustic Emission:"() -> (w470:refnum<vi>)
      n374 = control-ref of="Filter% 2"() -> (w468:refnum<vi>)
      n375 = control-ref of="Filter%"() -> (w466:refnum<vi>)
      n376 = control-ref of="Sway distance (mm)"() -> (w465:refnum<vi>)
      n377 = control-ref of="Surge distance (mm)"() -> (w464:refnum<vi>)
      n378 = control-ref of="DataSavingLoopDelay(ms)"() -> (w463:refnum<vi>)
      n379 = control-ref of="Sway Counts:"() -> (w460:refnum<vi>)
      n380 = control-ref of="Distance (mm): 3"() -> (w459:refnum<vi>)
      n381 = control-ref of="Surge Counts:"() -> (w458:refnum<vi>)
      n382 = control-ref of="Distance (mm): 2"() -> (w457:refnum<vi>)
      n383 = control-ref of="Distance (mm):"() -> (w456:refnum<vi>)
      n384 = control-ref of="Heave Counts:"() -> (w455:refnum<vi>)
      n385 = control-ref of="LRMHomeSurgeOffsetCounts"() -> (w454:refnum<vi>)
      n386 = control-ref of="LRMHomeSwayOffsetCounts"() -> (w453:refnum<vi>)
      n387 = control-ref of="TracHomeSurgeOffsetCounts 20MM"() -> (w452:refnum<vi>)
      n388 = control-ref of="TracHomeSwayOffsetCounts 20MM"() -> (w451:refnum<vi>)
      n389 = control-ref of="RotHomeSwayOffsetCounts"() -> (w450:refnum<vi>)
      n390 = control-ref of="RotHomeSurgeOffsetCounts"() -> (w449:refnum<vi>)
      n391 = control-ref of="Heave distance"() -> (w448:refnum<vi>)
      n392 = control-ref of="Zmm"() -> (w447:refnum<vi>)
      n393 = control-ref of="Heave Pulses/mm"() -> (w446:refnum<vi>)
      n394 = control-ref of="Surge Pulses/mm"() -> (w445:refnum<vi>)
      n395 = control-ref of="Sway Pulses/mm"() -> (w444:refnum<vi>)
      n396 = control-ref of="Heave Pitch"() -> (w443:refnum<vi>)
      n397 = control-ref of="Surge Pitch"() -> (w442:refnum<vi>)
      n398 = control-ref of="Sway Pitch"() -> (w441:refnum<vi>)
      n399 = control-ref of="Heave PPR"() -> (w440:refnum<vi>)
      n400 = control-ref of="Surge PPR"() -> (w439:refnum<vi>)
      n401 = control-ref of="Sway PPR"() -> (w438:refnum<vi>)
      n402 = Bundle By Name(cluster=w479, "Config Parameters.Tab Control 3"=w477, "Config Parameters.Tab Control 19"=w476, "Config Parameters.SAMPLES"=w475, "Config Parameters.Re-initilaize"=w474, "Config Parameters.Filter ON/OFF"=w473, "Config Parameters.TracHomeSurgeOffsetCounts 10MM"=w472, "Config Parameters.TracHomeSwayOffsetCounts 10MM"=w471, "Config Parameters.Acoustic Emission:"=w470, "Config Parameters.Apply Filter (FF)"=w469, "Config Parameters.Filter% 2"=w468, "Config Parameters.Apply Filter (Load)"=w467, "Config Parameters.Filter%"=w466, "Config Parameters.Sway distance (mm)"=w465, "Config Parameters.Surge distance (mm)"=w464, "Config Parameters.DataSavingLoopDelay(ms)"=w463, "Config Parameters.SAVE 2"=w462, "Config Parameters.Enter Distance"=w461, "Config Parameters.Sway Counts:"=w460, "Config Parameters.Distance (mm): 3"=w459, "Config Parameters.Surge Counts:"=w458, "Config Parameters.Distance (mm): 2"=w457, "Config Parameters.Distance (mm):"=w456, "Config Parameters.Heave Counts:"=w455, "Config Parameters.LRMHomeSurgeOffsetCounts"=w454, "Config Parameters.LRMHomeSwayOffsetCounts"=w453, "Config Parameters.TracHomeSurgeOffsetCounts 20MM"=w452, "Config Parameters.TracHomeSwayOffsetCounts 20MM"=w451, "Config Parameters.RotHomeSwayOffsetCounts"=w450, "Config Parameters.RotHomeSurgeOffsetCounts"=w449, "Config Parameters.Heave distance"=w448, "Config Parameters.Zmm"=w447, "Config Parameters.Heave Pulses/mm"=w446, "Config Parameters.Surge Pulses/mm"=w445, "Config Parameters.Sway Pulses/mm"=w444, "Config Parameters.Heave Pitch"=w443, "Config Parameters.Surge Pitch"=w442, "Config Parameters.Sway Pitch"=w441, "Config Parameters.Heave PPR"=w440, "Config Parameters.Surge PPR"=w439, "Config Parameters.Sway PPR"=w438, "Config Parameters.Tab Control 5"=w437, "Config Parameters.Tab Control 14"=w436, "Config Parameters.Tab Control 26"=w435, "Config Parameters.AE"=w434, "Config Parameters.Heave Loop Delay"=w433, "Config Parameters.Heave PID Speed"=w432, "Config Parameters.Surge Jog Speed"=w431, "Config Parameters.Heave Jog Speed"=w430, "Config Parameters.Sway Loop Delay"=w429, "Config Parameters.Sway PID Speed"=w428, "Config Parameters.Sway Jog Speed"=w427, "Config Parameters.DEPTH TRIP VALUE"=w426, "Config Parameters.LOAD TRIP VALUE"=w425, "Config Parameters.DEPTH TRIP   ENABLE"=w424, "Config Parameters.LOAD TRIP  ENABLE"=w423, "Config Parameters.CYCLIC FF TRIP VALUE"=w422, "Config Parameters.FF TRIP VALUE"=w421, "Config Parameters.CYCLIC CoF TRIP VALUE"=w420, "Config Parameters.COF TRIP VALUE"=w419, "Config Parameters.CYCLIC COF TRIP  ENABLE"=w418, "Config Parameters.CYCLIC FF TRIP  ENABLE"=w417, "Config Parameters.FF TRIP  ENABLE"=w416, "Config Parameters.COF TRIP  ENABLE"=w415) -> (w478:T11)
    }
    frame #11 {
      n403 = control-ref of="Mx"() -> (w509:refnum<vi>)
      n404 = control-ref of="My"() -> (w508:refnum<vi>)
      n405 = control-ref of="Mz"() -> (w507:refnum<vi>)
      n406 = control-ref of="Fx(N)"() -> (w506:refnum<vi>)
      n407 = control-ref of="Fy(N)"() -> (w505:refnum<vi>)
      n408 = control-ref of="Fz(N)"() -> (w504:refnum<vi>)
      n409 = control-ref of="Load Cell Temp"() -> (w480:refnum<vi>)
      n410 = control-ref of="ClearAll"() -> (w514:refnum<vi>)
      n411 = control-ref of="ZeroAll"() -> (w503:refnum<vi>)
      n412 = control-ref of="delete Handle"() -> (w493:refnum<vi>)
      n413 = control-ref of="Create Handle"() -> (w492:refnum<vi>)
      n414 = control-ref of="stop 6"() -> (w489:refnum<vi>)
      n415 = control-ref of="running_flag"() -> (w488:refnum<vi>)
      n416 = control-ref of="Save Dwell"() -> (w510:refnum<vi>)
      n417 = control-ref of="Acq Delay (ms)"() -> (w502:refnum<vi>)
      n418 = control-ref of="Burst Delay (ms)"() -> (w501:refnum<vi>)
      n419 = control-ref of="SN"() -> (w499:refnum<vi>)
      n420 = control-ref of="Port"() -> (w496:refnum<vi>)
      n421 = control-ref of="ft_udp_handle"() -> (w487:refnum<vi>)
      n422 = control-ref of="get-data-return"() -> (w486:refnum<vi>)
      n423 = control-ref of="get-range-return"() -> (w485:refnum<vi>)
      n424 = control-ref of="zero-return"() -> (w484:refnum<vi>)
      n425 = control-ref of="filter-return"() -> (w483:refnum<vi>)
      n426 = control-ref of="initial-return"() -> (w482:refnum<vi>)
      n427 = control-ref of="deleteHandle-result"() -> (w481:refnum<vi>)
      n428 = control-ref of="model"() -> (w500:refnum<vi>)
      n429 = control-ref of="Sensor IP"() -> (w497:refnum<vi>)
      n430 = control-ref of="Mz(Nm)"() -> (w513:refnum<vi>)
      n431 = control-ref of="My(Nm)"() -> (w512:refnum<vi>)
      n432 = control-ref of="Mx(Nm)"() -> (w511:refnum<vi>)
      n433 = control-ref of="FFx(N)"() -> (w498:refnum<vi>)
      n434 = control-ref of="FFy(N)"() -> (w495:refnum<vi>)
      n435 = control-ref of="Load(N)"() -> (w494:refnum<vi>)
      n436 = control-ref of="ft_data"() -> (w491:refnum<vi>)
      n437 = control-ref of="ft_range"() -> (w490:refnum<vi>)
      n438 = Bundle By Name(cluster=w516, "Loading Com Port.ClearAll"=w514, "Loading Com Port.Mz(Nm)"=w513, "Loading Com Port.My(Nm)"=w512, "Loading Com Port.Mx(Nm)"=w511, "Loading Com Port.Save Dwell"=w510, "Loading Com Port.Mx"=w509, "Loading Com Port.My"=w508, "Loading Com Port.Mz"=w507, "Loading Com Port.Fx(N)"=w506, "Loading Com Port.Fy(N)"=w505, "Loading Com Port.Fz(N)"=w504, "Loading Com Port.ZeroAll"=w503, "Loading Com Port.Acq Delay (ms)"=w502, "Loading Com Port.Burst Delay (ms)"=w501, "Loading Com Port.model"=w500, "Loading Com Port.SN"=w499, "Loading Com Port.FFx(N)"=w498, "Loading Com Port.Sensor IP"=w497, "Loading Com Port.Port"=w496, "Loading Com Port.FFy(N)"=w495, "Loading Com Port.Load(N)"=w494, "Loading Com Port.delete Handle"=w493, "Loading Com Port.Create Handle"=w492, "Loading Com Port.ft_data"=w491, "Loading Com Port.ft_range"=w490, "Loading Com Port.stop 6"=w489, "Loading Com Port.running_flag"=w488, "Loading Com Port.ft_udp_handle"=w487, "Loading Com Port.get-data-return"=w486, "Loading Com Port.get-range-return"=w485, "Loading Com Port.zero-return"=w484, "Loading Com Port.filter-return"=w483, "Loading Com Port.initial-return"=w482, "Loading Com Port.deleteHandle-result"=w481, "Loading Com Port.Load Cell Temp"=w480) -> (w515:T11)
    }
    frame #12 {
      n439 = control-ref of="Manual Write Heave & Surge"() -> (w518:refnum<vi>)
      n440 = control-ref of="Read Heave Temp"() -> (w541:refnum<vi>)
      n441 = control-ref of="error out Read"() -> (w553:refnum<vi>)
      n442 = control-ref of="error out Write"() -> (w548:refnum<vi>)
      n443 = control-ref of="SURGE POSE"() -> (w554:refnum<vi>)
      n444 = control-ref of="HEAVE POSE"() -> (w552:refnum<vi>)
      n445 = control-ref of="State"() -> (w551:refnum<vi>)
      n446 = control-ref of="Homed"() -> (w550:refnum<vi>)
      n447 = control-ref of="Sequence ID"() -> (w549:refnum<vi>)
      n448 = control-ref of="faultCode"() -> (w547:refnum<vi>)
      n449 = control-ref of="Ack ID"() -> (w546:refnum<vi>)
      n450 = control-ref of="SPEED"() -> (w545:refnum<vi>)
      n451 = control-ref of="Distance"() -> (w544:refnum<vi>)
      n452 = control-ref of="Mode Command"() -> (w543:refnum<vi>)
      n453 = control-ref of="SPARE 2"() -> (w540:refnum<vi>)
      n454 = control-ref of="SPARE 1"() -> (w539:refnum<vi>)
      n455 = control-ref of="Spare 15"() -> (w538:refnum<vi>)
      n456 = control-ref of="Spare 14"() -> (w537:refnum<vi>)
      n457 = control-ref of="Spare 13"() -> (w536:refnum<vi>)
      n458 = control-ref of="Spare 12"() -> (w535:refnum<vi>)
      n459 = control-ref of="Spare 11"() -> (w534:refnum<vi>)
      n460 = control-ref of="Spare 10"() -> (w533:refnum<vi>)
      n461 = control-ref of="Spare 9"() -> (w532:refnum<vi>)
      n462 = control-ref of="Spare 8"() -> (w531:refnum<vi>)
      n463 = control-ref of="Spare 7"() -> (w530:refnum<vi>)
      n464 = control-ref of="Spare 6"() -> (w529:refnum<vi>)
      n465 = control-ref of="Spare 5"() -> (w528:refnum<vi>)
      n466 = control-ref of="Spare 4"() -> (w527:refnum<vi>)
      n467 = control-ref of="Spare 3"() -> (w526:refnum<vi>)
      n468 = control-ref of="Spare 2"() -> (w525:refnum<vi>)
      n469 = control-ref of="Spare 1"() -> (w524:refnum<vi>)
      n470 = control-ref of="Node Id"() -> (w523:refnum<vi>)
      n471 = control-ref of="SPARE 3"() -> (w522:refnum<vi>)
      n472 = control-ref of="SPARE 4"() -> (w521:refnum<vi>)
      n473 = control-ref of="fwMajor"() -> (w520:refnum<vi>)
      n474 = control-ref of="fwMinor"() -> (w519:refnum<vi>)
      n475 = control-ref of="Heave and Surge Write"() -> (w517:refnum<vi>)
      n476 = control-ref of="Heave and Surge Read"() -> (w542:refnum<vi>)
      n477 = Bundle By Name(cluster=w556, "Heave AND Surge.SURGE POSE"=w554, "Heave AND Surge.error out Read"=w553, "Heave AND Surge.HEAVE POSE"=w552, "Heave AND Surge.State"=w551, "Heave AND Surge.Homed"=w550, "Heave AND Surge.Sequence ID"=w549, "Heave AND Surge.error out Write"=w548, "Heave AND Surge.faultCode"=w547, "Heave AND Surge.Ack ID"=w546, "Heave AND Surge.SPEED"=w545, "Heave AND Surge.Distance"=w544, "Heave AND Surge.Mode Command"=w543, "Heave AND Surge.Heave and Surge Read"=w542, "Heave AND Surge.Read Heave Temp"=w541, "Heave AND Surge.SPARE 2"=w540, "Heave AND Surge.SPARE 1"=w539, "Heave AND Surge.Spare 15"=w538, "Heave AND Surge.Spare 14"=w537, "Heave AND Surge.Spare 13"=w536, "Heave AND Surge.Spare 12"=w535, "Heave AND Surge.Spare 11"=w534, "Heave AND Surge.Spare 10"=w533, "Heave AND Surge.Spare 9"=w532, "Heave AND Surge.Spare 8"=w531, "Heave AND Surge.Spare 7"=w530, "Heave AND Surge.Spare 6"=w529, "Heave AND Surge.Spare 5"=w528, "Heave AND Surge.Spare 4"=w527, "Heave AND Surge.Spare 3"=w526, "Heave AND Surge.Spare 2"=w525, "Heave AND Surge.Spare 1"=w524, "Heave AND Surge.Node Id"=w523, "Heave AND Surge.SPARE 3"=w522, "Heave AND Surge.SPARE 4"=w521, "Heave AND Surge.fwMajor"=w520, "Heave AND Surge.fwMinor"=w519, "Heave AND Surge.Manual Write"=w518, "Heave AND Surge.Heave and Surge Write"=w517) -> (w555:T11)
    }
    frame #13 {
      n478 = control-ref of="Fine Tune Zone"() -> (w572:refnum<vi>)
      n479 = control-ref of="PID Delay (sec)"() -> (w571:refnum<vi>)
      n480 = control-ref of="Max_pos_limit"() -> (w570:refnum<vi>)
      n481 = control-ref of="Min_pos_limit"() -> (w569:refnum<vi>)
      n482 = control-ref of="i_limit"() -> (w568:refnum<vi>)
      n483 = control-ref of="pct_scale"() -> (w559:refnum<vi>)
      n484 = control-ref of="Deadband"() -> (w567:refnum<vi>)
      n485 = control-ref of="Kd"() -> (w566:refnum<vi>)
      n486 = control-ref of="Ki"() -> (w565:refnum<vi>)
      n487 = control-ref of="Kp"() -> (w564:refnum<vi>)
      n488 = control-ref of="Current Position"() -> (w563:refnum<vi>)
      n489 = control-ref of="Set Load"() -> (w562:refnum<vi>)
      n490 = control-ref of="Current Load"() -> (w561:refnum<vi>)
      n491 = control-ref of="Pulse delta"() -> (w560:refnum<vi>)
      n492 = control-ref of="Init Step"() -> (w558:refnum<vi>)
      n493 = control-ref of="Max Step Linit"() -> (w557:refnum<vi>)
      n494 = Bundle By Name(cluster=w574, "New PID LOGIC.Fine Tune Zone"=w572, "New PID LOGIC.PID SDelay"=w571, "New PID LOGIC.Max_pos_limit"=w570, "New PID LOGIC.Min_pos_limit"=w569, "New PID LOGIC.i_limit"=w568, "New PID LOGIC.pct_scale"=w559, "New PID LOGIC.Deadband"=w567, "New PID LOGIC.Kd"=w566, "New PID LOGIC.Ki"=w565, "New PID LOGIC.Kp"=w564, "New PID LOGIC.Current Position"=w563, "New PID LOGIC.Set Load"=w562, "New PID LOGIC.Current Load"=w561, "New PID LOGIC.Pulse delta"=w560, "New PID LOGIC.Init Step"=w558, "New PID LOGIC.Max Step Linit"=w557) -> (w573:T11)
    }
    frame #14 {
      n495 = control-ref of="Manual Write SWAY"() -> (w594:refnum<vi>)
      n496 = control-ref of="Read SWAY Temp"() -> (w575:refnum<vi>)
      n497 = control-ref of="error out Write  SWAY"() -> (w596:refnum<vi>)
      n498 = control-ref of="error out Read SWAY"() -> (w595:refnum<vi>)
      n499 = control-ref of="fwMajor"() -> (w613:refnum<vi>)
      n500 = control-ref of="Homed"() -> (w612:refnum<vi>)
      n501 = control-ref of="Rotary POSE"() -> (w611:refnum<vi>)
      n502 = control-ref of="State"() -> (w610:refnum<vi>)
      n503 = control-ref of="SWAY POSE"() -> (w609:refnum<vi>)
      n504 = control-ref of="Ack ID"() -> (w608:refnum<vi>)
      n505 = control-ref of="faultCode"() -> (w607:refnum<vi>)
      n506 = control-ref of="Node Id"() -> (w606:refnum<vi>)
      n507 = control-ref of="fwMinor"() -> (w605:refnum<vi>)
      n508 = control-ref of="Spare 6"() -> (w604:refnum<vi>)
      n509 = control-ref of="Spare 5"() -> (w603:refnum<vi>)
      n510 = control-ref of="Spare 4"() -> (w602:refnum<vi>)
      n511 = control-ref of="Spare 3"() -> (w601:refnum<vi>)
      n512 = control-ref of="Spare 2"() -> (w600:refnum<vi>)
      n513 = control-ref of="Spare 1"() -> (w599:refnum<vi>)
      n514 = control-ref of="Spare 7"() -> (w598:refnum<vi>)
      n515 = control-ref of="SPARE  5"() -> (w597:refnum<vi>)
      n516 = control-ref of="SPARE  4"() -> (w592:refnum<vi>)
      n517 = control-ref of="SPARE  3"() -> (w591:refnum<vi>)
      n518 = control-ref of="SPARE 2"() -> (w590:refnum<vi>)
      n519 = control-ref of="SPARE 1"() -> (w589:refnum<vi>)
      n520 = control-ref of="Spare 15"() -> (w588:refnum<vi>)
      n521 = control-ref of="Spare 14"() -> (w587:refnum<vi>)
      n522 = control-ref of="Spare 13"() -> (w586:refnum<vi>)
      n523 = control-ref of="Spare 12"() -> (w585:refnum<vi>)
      n524 = control-ref of="Spare 11"() -> (w584:refnum<vi>)
      n525 = control-ref of="Spare 9"() -> (w583:refnum<vi>)
      n526 = control-ref of="Spare 8"() -> (w582:refnum<vi>)
      n527 = control-ref of="SPEED"() -> (w581:refnum<vi>)
      n528 = control-ref of="Distance"() -> (w580:refnum<vi>)
      n529 = control-ref of="Mode Command"() -> (w579:refnum<vi>)
      n530 = control-ref of="Sequence ID"() -> (w578:refnum<vi>)
      n531 = control-ref of="Spare 10"() -> (w576:refnum<vi>)
      n532 = control-ref of="SWAY WRITE"() -> (w593:refnum<vi>)
      n533 = control-ref of="SWAY READ"() -> (w577:refnum<vi>)
      n534 = Bundle By Name(cluster=w615, "SWAY.fwMajor"=w613, "SWAY.Homed"=w612, "SWAY.Rotary POSE"=w611, "SWAY.State"=w610, "SWAY.SWAY POSE"=w609, "SWAY.Ack ID"=w608, "SWAY.faultCode"=w607, "SWAY.Node Id"=w606, "SWAY.fwMinor"=w605, "SWAY.Spare 6"=w604, "SWAY.Spare 5"=w603, "SWAY.Spare 4"=w602, "SWAY.Spare 3"=w601, "SWAY.Spare 2"=w600, "SWAY.Spare 1"=w599, "SWAY.Spare 7"=w598, "SWAY.SPARE  5"=w597, "SWAY.error out Write  SWAY"=w596, "SWAY.error out Read SWAY"=w595, "SWAY.Manual Write SWAY"=w594, "SWAY.SWAY WRITE"=w593, "SWAY.SPARE  4"=w592, "SWAY.SPARE  3"=w591, "SWAY.SPARE 2"=w590, "SWAY.SPARE 1"=w589, "SWAY.Spare 15"=w588, "SWAY.Spare 14"=w587, "SWAY.Spare 13"=w586, "SWAY.Spare 12"=w585, "SWAY.Spare 11"=w584, "SWAY.Spare 9"=w583, "SWAY.Spare 8"=w582, "SWAY.SPEED"=w581, "SWAY.Distance"=w580, "SWAY.Mode Command"=w579, "SWAY.Sequence ID"=w578, "SWAY.SWAY READ"=w577, "SWAY.Spare 10"=w576, "SWAY.Read SWAY Temp"=w575) -> (w614:T11)
    }
    frame #15 {
      n535 = control-ref of="Analysis Home new"() -> (w646:refnum<vi>)
      n536 = control-ref of="Refresh 2"() -> (w645:refnum<vi>)
      n537 = control-ref of="OPEN 4"() -> (w631:refnum<vi>)
      n538 = control-ref of="OPEN 3"() -> (w629:refnum<vi>)
      n539 = control-ref of="XY Graph"() -> (w624:refnum<vi>)
      n540 = control-ref of="OPEN 2"() -> (w621:refnum<vi>)
      n541 = control-ref of="OPEN 1"() -> (w620:refnum<vi>)
      n542 = control-ref of="Export"() -> (w617:refnum<vi>)
      n543 = control-ref of="MEAN"() -> (w644:refnum<vi>)
      n544 = control-ref of="SD"() -> (w643:refnum<vi>)
      n545 = control-ref of="VARIANCE"() -> (w642:refnum<vi>)
      n546 = control-ref of="MEAN"() -> (w641:refnum<vi>)
      n547 = control-ref of="SD"() -> (w640:refnum<vi>)
      n548 = control-ref of="VARIANCE"() -> (w639:refnum<vi>)
      n549 = control-ref of="MEAN"() -> (w638:refnum<vi>)
      n550 = control-ref of="SD"() -> (w637:refnum<vi>)
      n551 = control-ref of="VARIANCE"() -> (w636:refnum<vi>)
      n552 = control-ref of="MEAN"() -> (w635:refnum<vi>)
      n553 = control-ref of="SD"() -> (w634:refnum<vi>)
      n554 = control-ref of="VARIANCE"() -> (w633:refnum<vi>)
      n555 = control-ref of="File 4 Discription"() -> (w632:refnum<vi>)
      n556 = control-ref of="File Name 4"() -> (w630:refnum<vi>)
      n557 = control-ref of="File 3 Discription"() -> (w628:refnum<vi>)
      n558 = control-ref of="File Name 3"() -> (w627:refnum<vi>)
      n559 = control-ref of="File Name 2"() -> (w623:refnum<vi>)
      n560 = control-ref of="File Name 1"() -> (w622:refnum<vi>)
      n561 = control-ref of="File 1 Discription"() -> (w619:refnum<vi>)
      n562 = control-ref of="File 2 Discription"() -> (w618:refnum<vi>)
      n563 = control-ref of="Y-AXIS"() -> (w626:refnum<vi>)
      n564 = control-ref of="X-AXIS"() -> (w625:refnum<vi>)
      n565 = control-ref of="File Format"() -> (w616:refnum<vi>)
      n566 = Bundle By Name(cluster=w648, "Analysis Screen.Analysis Home"=w646, "Analysis Screen.Refresh 2"=w645, "Analysis Screen.MEAN 4"=w644, "Analysis Screen.SD 4"=w643, "Analysis Screen.VARIANCE 4"=w642, "Analysis Screen.MEAN  3"=w641, "Analysis Screen.SD  3"=w640, "Analysis Screen.VARIANCE  3"=w639, "Analysis Screen.MEAN 2"=w638, "Analysis Screen.SD  2"=w637, "Analysis Screen.VARIANCE 2"=w636, "Analysis Screen.MEAN"=w635, "Analysis Screen.SD"=w634, "Analysis Screen.VARIANCE"=w633, "Analysis Screen.File 4 Discription"=w632, "Analysis Screen.OPEN 4"=w631, "Analysis Screen.File Name 4"=w630, "Analysis Screen.OPEN 3"=w629, "Analysis Screen.File 3 Discription"=w628, "Analysis Screen.File Name 3"=w627, "Analysis Screen.Y-AXIS"=w626, "Analysis Screen.X-AXIS"=w625, "Analysis Screen.XY Graph"=w624, "Analysis Screen.File Name 2"=w623, "Analysis Screen.File Name 1"=w622, "Analysis Screen.OPEN 2"=w621, "Analysis Screen.OPEN 1"=w620, "Analysis Screen.File 1 Discription"=w619, "Analysis Screen.File 2 Discription"=w618, "Analysis Screen.Export"=w617, "Analysis Screen.File Format"=w616) -> (w647:T11)
    }
  }
  n567 = call <userlib>:"Fit VI window to Largest Dec.vi"() -> ("error out"=w44:errorcluster, "dup VI Ref"=w41:refnum<vi>)  [unwired: 6 in]
  n568 = invoke on="Invoke Node" class="VI" method="FP.Run-Time Position.Maximized"(reference=w41, error in=w44) -> (error out=w43:errorcluster)  [unwired: 2 in, 3 out]
  n569 = call <vilib>:"Clear Errors.vi"("error in (no error)"=w43) -> ("error out"=w42:errorcluster)  [unwired: 5 in, 1 out]
  n570 = control-ref of="This VI"() -> (w47:refnum<vi>)
  n571 = invoke on="Invoke Node" class="VI" method="Default Vals.Reinit All"(reference=w47, error in=w42) -> (reference out=w45:refnum<vi>, error out=w46:errorcluster)  [unwired: 1 in, 1 out]
  n572 = Close Reference(reference=w45, error in (no error)=w46) -> (error out=w40:errorcluster)
  n573 = call "Create User Event - Stop.vi"("error in (no error)"=w40) -> ("error out"=w18:errorcluster, "User Event - Stop"=w27:refnum<user-event>)  [unwired: 9 in]
  n574 = call "main screen queue out Unitest.vi"("error in (no error)"=w18) -> ("error out"=w67:errorcluster, "output Queue"=w39:T12)  [unwired: 9 in]
  n575 = Unbundle By Name(w39) -> ("RAMP MOTOR COM LOOP"=w32:refnum<queue>)
  n576 = Unbundle By Name(w39) -> ("TEMPERATURE COM LOOP"=w34:refnum<queue>)
  n577 = Unbundle By Name(w39) -> ("ECR PORT"=w31:refnum<queue>)
  n578 = Unbundle By Name(w39) -> ("SWAY MOTOR COM LOOP"=w36:refnum<queue>)
  n579 = Unbundle By Name(w39) -> ("UI Loop"=w65:refnum<queue>)
  n580 = Unbundle By Name(w39) -> ("LOAD COM LOOP"=w37:refnum<queue>)
  n581 = Unbundle By Name(w39) -> ("HEAVE MOTOR COM LOOP"=w19:refnum<queue>)
  n582 = Unbundle By Name(w39) -> ("HUMIDITY COM PORT"=w30:refnum<queue>)
  n583 = Unbundle By Name(w39) -> ("PROGRAM LOOP"=w29:refnum<queue>)
  n584 = Unbundle By Name(w39) -> ("MONITOR LOOP"=w26:refnum<queue>)
  n585 = Unbundle By Name(w39) -> ("LOAD PID"=w25:refnum<queue>)
  n586 = Unbundle By Name(w39) -> ("REPORT"=w24:refnum<queue>)
  n587 = register-events(w27) -> (reference out=w59:refnum<event-registration>, error out=w57:errorcluster)  [unwired: 2 in]
  n588 = Merge Errors(w57, w67) -> (w58:errorcluster)
  n589 = node-c288() -> (w3:T13)  [unwired: 4 in]
  n590 = node-c288() -> (w5:T13)  [unwired: 4 in]
  n591 = node-c288() -> (w7:T13)  [unwired: 4 in]
  n592 = node-c288() -> (w9:T13)  [unwired: 4 in]
  n593 = node-c288() -> (w11:T13)  [unwired: 4 in]
  n594 = node-c288() -> (w13:T13)  [unwired: 4 in]
  n595 = disable-structure shown="Disabled" {
    disable-tunnel: w30 -> [w652 _]
    disable-tunnel: w28 -> [w651 _]
    disable-tunnel: w27 -> [w650 _]
    disable-tunnel: w18 -> [w649 _]
    frame Disabled {
      n596 = while {
        shift-right: [w663] -> _
        shift-left: w651 -> [w664]
        tunnel: [w657] -> _
        tunnel: w652 -> [w655]
        tunnel: w649 -> [w654]
        tunnel: w650 -> [w653]
        stop <- w662 stop-if-true
        # "Humidity  Handling Loop"
        n597 = call "Dequeue Message.vi"("error in (no error)"=w654, "Message Queue"=w655) -> ("error out"=w661:errorcluster, "Message Data"=w659:variant, "Message"=w660:string, "dup Message Queue"=w658:refnum<queue>)  [unwired: 6 in]
        n598 = case "Message Cases" shown="\"Humidity Main\"" w660 {
          selector: w660 -> [_ _ _ _ _ w708]
          tunnel: w658 -> [w665 w676 _ w695 w707 _]
          tunnel: w661 -> [w668 w673 w692 w699 w701 _]
          tunnel: [w669 w677 w686 w697 w703 w709] -> w656
          tunnel: w664 -> [w667 w675 w691 w698 w706 w710]
          tunnel: [w667 w675 w691 w698 w706 w710] -> w663
          tunnel: [_ _ _ _ TRUE _] -> w662
          tunnel: w659 -> [_ _ w690 _ _ _]
          tunnel: w653 -> [_ _ _ _ w700 _]
          frame "init" {
            # "Initialize - All initialization work should take place in this message, since other loops can potentially enqueue messages that execute immediately after this one."
            n599 = call-poly "Enqueue Message.vi"("error in (no error)"=w668, "Message"="Humidity Main", "Message Queue"=w665) -> ("error out"=w669:errorcluster)  [unwired: 7 in, 1 out]
          }
          frame "Humidity Main" {
            n600 = Unbundle By Name(w675) -> ("Main Home Screen.EXIT"=w674:refnum<vi>)
            n601 = property class="Bool (strict)"(reference=w674) -> (reference out=w671:refnum<vi>, error out=w672:errorcluster, "Value"=w670:bool)  [unwired: 1 in]
            n602 = case shown="False" w670 {
              tunnel: [w680 w684] -> w677
              tunnel: w676 -> [w679 w683]
              tunnel: w673 -> [w678 w682]
              frame True {
                n603 = call-poly "Enqueue Message.vi"("error in (no error)"=w678, "Message"="Confirm Quit", "Message Queue"=w679) -> ("error out"=w680:errorcluster)  [unwired: 7 in, 1 out]
              }
              frame False {
                n604 = call-poly "Enqueue Message.vi"("error in (no error)"=w682, "Message"="Humidity Main", "Message Queue"=w683) -> ("error out"=w684:errorcluster)  [unwired: 7 in, 1 out]
              }
            }
            n605 = Close Reference(reference=w671, error in (no error)=w672) -> ()  [unwired: 1 out]
          }
          frame "Error" {
            # "#CodeRecommended - If you ever change the name of this \"Error\" message, you'll need to update the name in the Check Loop Error.vi as well."
            # "#CodeRecommended - Consider creating a system for logging errors in some way. These errors are for notification purposes only. Handling of specific errors should be performed in the message frames that generated the error."
            # "Error - Display an error dialog. This message is sent by the \"Error Handler\" VIs at the end of other loops in this application."
            n606 = Variant To Data(error in=w692, type=errorcluster {"status"=FALSE, "code"=0, "source"=""} ("error constant"), Variant=w690) -> (data=w688:errorcluster, error out=w687:errorcluster)
            n607 = call <vilib>:"Simple Error Handler.vi"("error in (no error)"=w688) -> ()  [unwired: 4 in, 5 out]
            n608 = Merge Errors(w687) -> (w686:errorcluster)
          }
          frame "Confirm Quit" {
            # "#CodeNeeded - If you want to provide an \"Are you sure\" dialog (or some other notification) before the application exits, place that code here. This message is typically sent from a Panel Close? event."
            # "Confirm Quit - Message that can confirm whether or not the user wants to exit the application."
            n609 = call-poly "Enqueue Message.vi"("Priority Message? (F)"=TRUE, "error in (no error)"=w699, "Message"="Exit", "Message Queue"=w695) -> ("error out"=w696:errorcluster)  [unwired: 6 in, 1 out]
            n610 = Merge Errors(w696) -> (w697:errorcluster)
          }
          frame "Exit" {
            # "Stop the VI"
            # "Release the message queue reference"
            # "#CodeNeeded - Add any required cleanup code here. Note that if 'Exit' was called as a result of an error, an error dialog will be displayed. Add any custom error handling for an 'Exit' condition here as well."
            # "Exit - Exit the application."
            n611 = call "Fire User Event - Stop.vi"("User Event - Stop"=w700) -> ("error out"=w702:errorcluster)  [unwired: 10 in]
            n612 = Release Queue(queue=w707, error in (no error)=w701) -> (error out=w704:errorcluster)  [unwired: 1 in, 2 out]
            n613 = Merge Errors(w702, w704) -> (w703:errorcluster)
          }
          frame Default {
            # "'Default' case only runs if there is a message that isn't defined in any of the other cases.  Output a programming error."
            n614 = xnode "Error Ring"("parameter 0"=w708) -> ("error out"=w709:errorcluster)
          }
        }
        n615 = call "LAB-IQ Error Handler - Message Handling Loop.vi"("error in (no error)"=w656, "Message Queue"=w658) -> ("dup error in"=w657:errorcluster)  [unwired: 8 in, 1 out]
      }
    }
    frame Enabled {
    }
  }
  n616 = disable-structure shown="Disabled" {
    disable-tunnel: w31 -> [w721 _]
    disable-tunnel: w28 -> [w720 _]
    disable-tunnel: w27 -> [w719 _]
    disable-tunnel: w18 -> [w718 _]
    frame Disabled {
      n617 = while {
        shift-right: [w732] -> _
        shift-left: w720 -> [w733]
        tunnel: [w726] -> _
        tunnel: w721 -> [w724]
        tunnel: w718 -> [w723]
        tunnel: w719 -> [w722]
        stop <- w731 stop-if-true
        # "ECR  Handling Loop"
        n618 = call "Dequeue Message.vi"("error in (no error)"=w723, "Message Queue"=w724) -> ("error out"=w730:errorcluster, "Message Data"=w728:variant, "Message"=w729:string, "dup Message Queue"=w727:refnum<queue>)  [unwired: 6 in]
        n619 = case "Message Cases" shown="\"ECR Main\"" w729 {
          selector: w729 -> [_ _ _ _ _ w777]
          tunnel: w727 -> [w734 w745 _ w764 w776 _]
          tunnel: w730 -> [w737 w742 w761 w768 w770 _]
          tunnel: [w738 w746 w755 w766 w772 w778] -> w725
          tunnel: w733 -> [w736 w744 w760 w767 w775 w779]
          tunnel: [w736 w744 w760 w767 w775 w779] -> w732
          tunnel: [_ _ _ _ TRUE _] -> w731
          tunnel: w728 -> [_ _ w759 _ _ _]
          tunnel: w722 -> [_ _ _ _ w769 _]
          frame "init" {
            # "Initialize - All initialization work should take place in this message, since other loops can potentially enqueue messages that execute immediately after this one."
            n620 = call-poly "Enqueue Message.vi"("error in (no error)"=w737, "Message"="ECR Main", "Message Queue"=w734) -> ("error out"=w738:errorcluster)  [unwired: 7 in, 1 out]
          }
          frame "ECR Main" {
            n621 = Unbundle By Name(w744) -> ("Main Home Screen.EXIT"=w743:refnum<vi>)
            n622 = property class="Bool (strict)"(reference=w743) -> (reference out=w740:refnum<vi>, error out=w741:errorcluster, "Value"=w739:bool)  [unwired: 1 in]
            n623 = case shown="False" w739 {
              tunnel: [w749 w753] -> w746
              tunnel: w745 -> [w748 w752]
              tunnel: w742 -> [w747 w751]
              frame True {
                n624 = call-poly "Enqueue Message.vi"("error in (no error)"=w747, "Message"="Confirm Quit", "Message Queue"=w748) -> ("error out"=w749:errorcluster)  [unwired: 7 in, 1 out]
              }
              frame False {
                n625 = call-poly "Enqueue Message.vi"("error in (no error)"=w751, "Message"="ECR Main", "Message Queue"=w752) -> ("error out"=w753:errorcluster)  [unwired: 7 in, 1 out]
              }
            }
            n626 = Close Reference(reference=w740, error in (no error)=w741) -> ()  [unwired: 1 out]
          }
          frame "Error" {
            # "#CodeRecommended - If you ever change the name of this \"Error\" message, you'll need to update the name in the Check Loop Error.vi as well."
            # "#CodeRecommended - Consider creating a system for logging errors in some way. These errors are for notification purposes only. Handling of specific errors should be performed in the message frames that generated the error."
            # "Error - Display an error dialog. This message is sent by the \"Error Handler\" VIs at the end of other loops in this application."
            n627 = Variant To Data(error in=w761, type=errorcluster {"status"=FALSE, "code"=0, "source"=""} ("error constant"), Variant=w759) -> (data=w757:errorcluster, error out=w756:errorcluster)
            n628 = call <vilib>:"Simple Error Handler.vi"("error in (no error)"=w757) -> ()  [unwired: 4 in, 5 out]
            n629 = Merge Errors(w756) -> (w755:errorcluster)
          }
          frame "Confirm Quit" {
            # "#CodeNeeded - If you want to provide an \"Are you sure\" dialog (or some other notification) before the application exits, place that code here. This message is typically sent from a Panel Close? event."
            # "Confirm Quit - Message that can confirm whether or not the user wants to exit the application."
            n630 = call-poly "Enqueue Message.vi"("Priority Message? (F)"=TRUE, "error in (no error)"=w768, "Message"="Exit", "Message Queue"=w764) -> ("error out"=w765:errorcluster)  [unwired: 6 in, 1 out]
            n631 = Merge Errors(w765) -> (w766:errorcluster)
          }
          frame "Exit" {
            # "Stop the VI"
            # "Release the message queue reference"
            # "#CodeNeeded - Add any required cleanup code here. Note that if 'Exit' was called as a result of an error, an error dialog will be displayed. Add any custom error handling for an 'Exit' condition here as well."
            # "Exit - Exit the application."
            n632 = call "Fire User Event - Stop.vi"("User Event - Stop"=w769) -> ("error out"=w771:errorcluster)  [unwired: 10 in]
            n633 = Release Queue(queue=w776, error in (no error)=w770) -> (error out=w773:errorcluster)  [unwired: 1 in, 2 out]
            n634 = Merge Errors(w771, w773) -> (w772:errorcluster)
          }
          frame Default {
            # "'Default' case only runs if there is a message that isn't defined in any of the other cases.  Output a programming error."
            n635 = xnode "Error Ring"("parameter 0"=w777) -> ("error out"=w778:errorcluster)
          }
        }
        n636 = call "LAB-IQ Error Handler - Message Handling Loop.vi"("error in (no error)"=w725, "Message Queue"=w727) -> ("dup error in"=w726:errorcluster)  [unwired: 8 in, 1 out]
      }
    }
    frame Enabled {
    }
  }
  n637 = while {
    tunnel: w65 -> [w794]
    shift-right: [w792] -> w62
    shift-left: w59 -> [w793]
    tunnel: [w788] -> w60
    stop <- w790 stop-if-true
    # "Event Handling Loop"
    n638 = event shown="[66] \"Analysis Home new\": Value Change" {
      selector: w793 -> [_ _ _ _ _ _ _ _ _ _ _ _ _ _ _ _ _ _ _ _ _ _ _ _ _ _ _ _ _ _ _ _ _ _ _ _ _ _ _ _ _ _ _ _ _ _ _ _ _ _ _ _ _ _ _ _ _ _ _ _ _ _ _ _ _ _ _ _ _ _ _ _ _]
      dyn-events: [_ _ _ _ _ _ _ _ _ _ _ _ _ _ _ _ _ _ _ _ _ _ _ _ _ _ _ _ _ _ _ _ _ _ _ _ _ _ _ _ _ _ _ _ _ _ _ _ _ _ _ _ _ _ _ _ _ _ _ _ _ _ _ _ _ _ _ _ _ _ _ _ _] -> w792
      timeout: 50 -> [_ _ _ _ _ _ _ _ _ _ _ _ _ _ _ _ _ _ _ _ _ _ _ _ _ _ _ _ _ _ _ _ _ _ _ _ _ _ _ _ _ _ _ _ _ _ _ _ _ _ _ _ _ _ _ _ _ _ _ _ _ _ _ _ _ _ _ _ _ _ _ _ _]
      tunnel: [_ _ _ _ _ _ _ _ _ _ _ _ _ _ _ _ _ _ _ _ _ _ _ _ _ _ _ _ _ _ _ _ _ _ _ _ _ _ _ _ _ _ _ _ _ _ _ _ _ _ _ _ _ _ _ _ _ _ _ _ _ _ _ _ _ _ _ _ _ _ _ _ TRUE ("Discard?")] -> w790
      tunnel: w794 -> [w799 w803 w808 w813 w818 w823 w828 w833 w838 w843 w848 w853 w858 w863 w868 w873 w878 w883 w888 w893 w898 w903 w908 w913 w918 w923 w928 w933 w938 w943 w948 w953 w958 w963 w968 w973 w978 w983 w988 w993 w998 w1003 w1008 w1013 w1018 w1023 w1028 w1033 w1038 w1043 w1048 w1053 w1058 w1063 w1068 w1073 w1078 w1083 w1088 w1093 w1098 w1103 w1108 w1113 w1118 w1123 w1128 w1133 w1138 w1143 w1146 w1151 w1153]
      tunnel: [w798 w801 w806 w811 w816 w821 w826 w831 w836 w841 w846 w851 w856 w861 w866 w871 w876 w881 w886 w891 w896 w901 w906 w911 w916 w921 w926 w931 w936 w941 w946 w951 w956 w961 w966 w971 w976 w981 w986 w991 w996 w1001 w1006 w1011 w1016 w1021 w1026 w1031 w1036 w1041 w1046 w1051 w1056 w1061 w1066 w1071 w1076 w1081 w1086 w1091 w1096 w1101 w1106 w1111 w1116 w1121 w1126 w1131 w1136 w1141 _ w1150 _] -> w791
      tunnel: [w797 w802 w807 w812 w817 w822 w827 w832 w837 w842 w847 w852 w857 w862 w867 w872 w877 w882 w887 w892 w897 w902 w907 w912 w917 w922 w927 w932 w937 w942 w947 w952 w957 w962 w967 w972 w977 w982 w987 w992 w997 w1002 w1007 w1012 w1017 w1022 w1027 w1032 w1037 w1042 w1047 w1052 w1057 w1062 w1067 w1072 w1077 w1082 w1087 w1092 w1097 w1102 w1107 w1112 w1117 w1122 w1127 w1132 w1137 w1142 w1146 w1149 w1153] -> w789
      event Panel Close? {
        n639 = event-data() -> ()  [unwired: 1 in, 1 out]
        n640 = call-poly "Enqueue Message.vi"("Priority Message? (F)"=TRUE, "Message"="Confirm Quit", "Message Queue"=w799) -> ("error out"=w798:errorcluster, "dup Message Queue"=w797:refnum<queue>)  [unwired: 7 in]
        n641 = event-data("Discard?"=TRUE) -> ()  [unwired: 1 in, 1 out]
      }
      event Timeout {
        n642 = event-data() -> ()  [unwired: 1 in, 1 out]
        n643 = call-poly "Enqueue Message.vi"("Priority Message? (F)"=TRUE, "Message"="Time Out", "Message Queue"=w803) -> ("error out"=w801:errorcluster, "dup Message Queue"=w802:refnum<queue>)  [unwired: 7 in]
      }
      event "SAVE  2": Value Change {
        n644 = event-data() -> ()  [unwired: 1 in, 1 out]
        n645 = call-poly "Enqueue Message.vi"("Priority Message? (F)"=TRUE, "Message"="Service Save", "Message Queue"=w808) -> ("error out"=w806:errorcluster, "dup Message Queue"=w807:refnum<queue>)  [unwired: 7 in]
      }
      event "Home": Value Change {
        n646 = event-data() -> ()  [unwired: 1 in, 1 out]
        n647 = call-poly "Enqueue Message.vi"("Priority Message? (F)"=TRUE, "Message"="HOME", "Message Queue"=w813) -> ("error out"=w811:errorcluster, "dup Message Queue"=w812:refnum<queue>)  [unwired: 7 in]
      }
      event "Platform Settings": Value Change {
        n648 = event-data() -> ()  [unwired: 1 in, 1 out]
        n649 = call-poly "Enqueue Message.vi"("Priority Message? (F)"=TRUE, "Message"="Platform Setting", "Message Queue"=w818) -> ("error out"=w816:errorcluster, "dup Message Queue"=w817:refnum<queue>)  [unwired: 7 in]
      }
      event "Configure": Value Change {
        n650 = event-data() -> ()  [unwired: 1 in, 1 out]
        n651 = call-poly "Enqueue Message.vi"("Priority Message? (F)"=TRUE, "Message"="Configure", "Message Queue"=w823) -> ("error out"=w821:errorcluster, "dup Message Queue"=w822:refnum<queue>)  [unwired: 7 in]
      }
      event "Analysis": Value Change {
        n652 = event-data() -> ()  [unwired: 1 in, 1 out]
        n653 = call-poly "Enqueue Message.vi"("Priority Message? (F)"=TRUE, "Message"="Analysis", "Message Queue"=w828) -> ("error out"=w826:errorcluster, "dup Message Queue"=w827:refnum<queue>)  [unwired: 7 in]
      }
      event "service 2": Value Change {
        n654 = event-data() -> ()  [unwired: 1 in, 1 out]
        n655 = call-poly "Enqueue Message.vi"("Priority Message? (F)"=TRUE, "Message"="service 2", "Message Queue"=w833) -> ("error out"=w831:errorcluster, "dup Message Queue"=w832:refnum<queue>)  [unwired: 7 in]
      }
      event "Auto": Value Change {
        n656 = event-data() -> ()  [unwired: 1 in, 1 out]
        n657 = call-poly "Enqueue Message.vi"("Priority Message? (F)"=TRUE, "Message"="Auto", "Message Queue"=w838) -> ("error out"=w836:errorcluster, "dup Message Queue"=w837:refnum<queue>)  [unwired: 7 in]
      }
      event "Select Load Head": Value Change {
        n658 = event-data() -> ()  [unwired: 1 in, 1 out]
        n659 = call-poly "Enqueue Message.vi"("Priority Message? (F)"=TRUE, "Message"="Select Load Head", "Message Queue"=w843) -> ("error out"=w841:errorcluster, "dup Message Queue"=w842:refnum<queue>)  [unwired: 7 in]
      }
      event "com 3": Value Change {
        n660 = event-data() -> ()  [unwired: 1 in, 1 out]
        n661 = call-poly "Enqueue Message.vi"("Priority Message? (F)"=TRUE, "Message"="com 3", "Message Queue"=w848) -> ("error out"=w846:errorcluster, "dup Message Queue"=w847:refnum<queue>)  [unwired: 7 in]
      }
      event "Loading Mode": Value Change {
        n662 = event-data() -> ()  [unwired: 1 in, 1 out]
        n663 = call-poly "Enqueue Message.vi"("Priority Message? (F)"=TRUE, "Message"="Loading Mode", "Message Queue"=w853) -> ("error out"=w851:errorcluster, "dup Message Queue"=w852:refnum<queue>)  [unwired: 7 in]
      }
      event "SSP 0.3": Value Change {
        n664 = event-data() -> ()  [unwired: 1 in, 1 out]
        n665 = call-poly "Enqueue Message.vi"("Priority Message? (F)"=TRUE, "Message"="SSP 0.3", "Message Queue"=w858) -> ("error out"=w856:errorcluster, "dup Message Queue"=w857:refnum<queue>)  [unwired: 7 in]
      }
      event "SSP 0.5": Value Change {
        n666 = event-data() -> ()  [unwired: 1 in, 1 out]
        n667 = call-poly "Enqueue Message.vi"("Priority Message? (F)"=TRUE, "Message"="SSP 0.5", "Message Queue"=w863) -> ("error out"=w861:errorcluster, "dup Message Queue"=w862:refnum<queue>)  [unwired: 7 in]
      }
      event "SSP 0.75": Value Change {
        n668 = event-data() -> ()  [unwired: 1 in, 1 out]
        n669 = call-poly "Enqueue Message.vi"("Priority Message? (F)"=TRUE, "Message"="SSP 0.75", "Message Queue"=w868) -> ("error out"=w866:errorcluster, "dup Message Queue"=w867:refnum<queue>)  [unwired: 7 in]
      }
      event "LHBack": Value Change {
        n670 = event-data() -> ()  [unwired: 1 in, 1 out]
        n671 = call-poly "Enqueue Message.vi"("Priority Message? (F)"=TRUE, "Message"="LHBack", "Message Queue"=w873) -> ("error out"=w871:errorcluster, "dup Message Queue"=w872:refnum<queue>)  [unwired: 7 in]
      }
      event "LHNext": Value Change {
        n672 = event-data() -> ()  [unwired: 1 in, 1 out]
        n673 = call-poly "Enqueue Message.vi"("Priority Message? (F)"=TRUE, "Message"="LHNext", "Message Queue"=w878) -> ("error out"=w876:errorcluster, "dup Message Queue"=w877:refnum<queue>)  [unwired: 7 in]
      }
      event "Rot Ver": Value Change {
        n674 = event-data() -> ()  [unwired: 1 in, 1 out]
        n675 = call-poly "Enqueue Message.vi"("Priority Message? (F)"=TRUE, "Message"="Rot Ver", "Message Queue"=w883) -> ("error out"=w881:errorcluster, "dup Message Queue"=w882:refnum<queue>)  [unwired: 7 in]
      }
      event "Scratch": Value Change {
        n676 = event-data() -> ()  [unwired: 1 in, 1 out]
        n677 = call-poly "Enqueue Message.vi"("Priority Message? (F)"=TRUE, "Message"="Scratch", "Message Queue"=w888) -> ("error out"=w886:errorcluster, "dup Message Queue"=w887:refnum<queue>)  [unwired: 7 in]
      }
      event "Motion Mode:": Value Change {
        n678 = event-data() -> ()  [unwired: 1 in, 1 out]
        n679 = call-poly "Enqueue Message.vi"("Priority Message? (F)"=TRUE, "Message"="Motion Mode:", "Message Queue"=w893) -> ("error out"=w891:errorcluster, "dup Message Queue"=w892:refnum<queue>)  [unwired: 7 in]
      }
      event "MMBack": Value Change {
        n680 = event-data() -> ()  [unwired: 1 in, 1 out]
        n681 = call-poly "Enqueue Message.vi"("Priority Message? (F)"=TRUE, "Message"="MMBack", "Message Queue"=w898) -> ("error out"=w896:errorcluster, "dup Message Queue"=w897:refnum<queue>)  [unwired: 7 in]
      }
      event "MMNext": Value Change {
        n682 = event-data() -> ()  [unwired: 1 in, 1 out]
        n683 = call-poly "Enqueue Message.vi"("Priority Message? (F)"=TRUE, "Message"="MMNext", "Message Queue"=w903) -> ("error out"=w901:errorcluster, "dup Message Queue"=w902:refnum<queue>)  [unwired: 7 in]
      }
      event "APBack": Value Change {
        n684 = event-data() -> ()  [unwired: 1 in, 1 out]
        n685 = call-poly "Enqueue Message.vi"("Priority Message? (F)"=TRUE, "Message"="APBack", "Message Queue"=w908) -> ("error out"=w906:errorcluster, "dup Message Queue"=w907:refnum<queue>)  [unwired: 7 in]
      }
      event "SNext": Value Change {
        n686 = event-data() -> ()  [unwired: 1 in, 1 out]
        n687 = call-poly "Enqueue Message.vi"("Priority Message? (F)"=TRUE, "Message"="SNext", "Message Queue"=w913) -> ("error out"=w911:errorcluster, "dup Message Queue"=w912:refnum<queue>)  [unwired: 7 in]
      }
      event "ZeroAll": Value Change {
        n688 = event-data() -> ()  [unwired: 1 in, 1 out]
        n689 = call-poly "Enqueue Message.vi"("Priority Message? (F)"=TRUE, "Message"="ZeroAll", "Message Queue"=w918) -> ("error out"=w916:errorcluster, "dup Message Queue"=w917:refnum<queue>)  [unwired: 7 in]
      }
      event "Enable Platform": Value Change {
        n690 = event-data() -> ()  [unwired: 1 in, 1 out]
        n691 = call-poly "Enqueue Message.vi"("Priority Message? (F)"=TRUE, "Message"="Enable Platform", "Message Queue"=w923) -> ("error out"=w921:errorcluster, "dup Message Queue"=w922:refnum<queue>)  [unwired: 7 in]
      }
      event "Heave Up main": Value Change {
        n692 = event-data() -> ()  [unwired: 1 in, 1 out]
        n693 = call-poly "Enqueue Message.vi"("Priority Message? (F)"=TRUE, "Message"="Heave Up main", "Message Queue"=w928) -> ("error out"=w926:errorcluster, "dup Message Queue"=w927:refnum<queue>)  [unwired: 7 in]
      }
      event "Heave Up MM": Value Change {
        n694 = event-data() -> ()  [unwired: 1 in, 1 out]
        n695 = call-poly "Enqueue Message.vi"("Priority Message? (F)"=TRUE, "Message"="Heave Up MM", "Message Queue"=w933) -> ("error out"=w931:errorcluster, "dup Message Queue"=w932:refnum<queue>)  [unwired: 7 in]
      }
      event "Heave Down Main": Value Change {
        n696 = event-data() -> ()  [unwired: 1 in, 1 out]
        n697 = call-poly "Enqueue Message.vi"("Priority Message? (F)"=TRUE, "Message"="Heave Down Main", "Message Queue"=w938) -> ("error out"=w936:errorcluster, "dup Message Queue"=w937:refnum<queue>)  [unwired: 7 in]
      }
      event "Heave Down MM": Value Change {
        n698 = event-data() -> ()  [unwired: 1 in, 1 out]
        n699 = call-poly "Enqueue Message.vi"("Priority Message? (F)"=TRUE, "Message"="Heave Down MM", "Message Queue"=w943) -> ("error out"=w941:errorcluster, "dup Message Queue"=w942:refnum<queue>)  [unwired: 7 in]
      }
      event "Manual Write Heave & Surge": Value Change {
        n700 = event-data() -> ()  [unwired: 1 in, 1 out]
        n701 = call-poly "Enqueue Message.vi"("Priority Message? (F)"=TRUE, "Message"="Manual Write Heave & Surge", "Message Queue"=w948) -> ("error out"=w946:errorcluster, "dup Message Queue"=w947:refnum<queue>)  [unwired: 7 in]
      }
      event "Manual Write SWAY": Value Change {
        n702 = event-data() -> ()  [unwired: 1 in, 1 out]
        n703 = call-poly "Enqueue Message.vi"("Priority Message? (F)"=TRUE, "Message"="Manual Write SWAY", "Message Queue"=w953) -> ("error out"=w951:errorcluster, "dup Message Queue"=w952:refnum<queue>)  [unwired: 7 in]
      }
      event "Surge Backward Main": Value Change {
        n704 = event-data() -> ()  [unwired: 1 in, 1 out]
        n705 = call-poly "Enqueue Message.vi"("Priority Message? (F)"=TRUE, "Message"="Surge Backward Main", "Message Queue"=w958) -> ("error out"=w956:errorcluster, "dup Message Queue"=w957:refnum<queue>)  [unwired: 7 in]
      }
      event "Surge Backward MM": Value Change {
        n706 = event-data() -> ()  [unwired: 1 in, 1 out]
        n707 = call-poly "Enqueue Message.vi"("Priority Message? (F)"=TRUE, "Message"="Surge Backward MM", "Message Queue"=w963) -> ("error out"=w961:errorcluster, "dup Message Queue"=w962:refnum<queue>)  [unwired: 7 in]
      }
      event "Surge Forward Main": Value Change {
        n708 = event-data() -> ()  [unwired: 1 in, 1 out]
        n709 = call-poly "Enqueue Message.vi"("Priority Message? (F)"=TRUE, "Message"="Surge Forward Main", "Message Queue"=w968) -> ("error out"=w966:errorcluster, "dup Message Queue"=w967:refnum<queue>)  [unwired: 7 in]
      }
      event "Surge Forward MM": Value Change {
        n710 = event-data() -> ()  [unwired: 1 in, 1 out]
        n711 = call-poly "Enqueue Message.vi"("Priority Message? (F)"=TRUE, "Message"="Surge Forward MM", "Message Queue"=w973) -> ("error out"=w971:errorcluster, "dup Message Queue"=w972:refnum<queue>)  [unwired: 7 in]
      }
      event "Sway Left Main": Value Change {
        n712 = event-data() -> ()  [unwired: 1 in, 1 out]
        n713 = call-poly "Enqueue Message.vi"("Priority Message? (F)"=TRUE, "Message"="Sway Left Main", "Message Queue"=w978) -> ("error out"=w976:errorcluster, "dup Message Queue"=w977:refnum<queue>)  [unwired: 7 in]
      }
      event "Sway Left MM": Value Change {
        n714 = event-data() -> ()  [unwired: 1 in, 1 out]
        n715 = call-poly "Enqueue Message.vi"("Priority Message? (F)"=TRUE, "Message"="Sway Left MM", "Message Queue"=w983) -> ("error out"=w981:errorcluster, "dup Message Queue"=w982:refnum<queue>)  [unwired: 7 in]
      }
      event "Sway Right MM": Value Change {
        n716 = event-data() -> ()  [unwired: 1 in, 1 out]
        n717 = call-poly "Enqueue Message.vi"("Priority Message? (F)"=TRUE, "Message"="Sway Right MM", "Message Queue"=w988) -> ("error out"=w986:errorcluster, "dup Message Queue"=w987:refnum<queue>)  [unwired: 7 in]
      }
      event "Sway Right Main": Value Change {
        n718 = event-data() -> ()  [unwired: 1 in, 1 out]
        n719 = call-poly "Enqueue Message.vi"("Priority Message? (F)"=TRUE, "Message"="Sway Right Main", "Message Queue"=w993) -> ("error out"=w991:errorcluster, "dup Message Queue"=w992:refnum<queue>)  [unwired: 7 in]
      }
      event "Load En": Value Change {
        n720 = event-data() -> ()  [unwired: 1 in, 1 out]
        n721 = call-poly "Enqueue Message.vi"("Priority Message? (F)"=TRUE, "Message"="Load En", "Message Queue"=w998) -> ("error out"=w996:errorcluster, "dup Message Queue"=w997:refnum<queue>)  [unwired: 7 in]
      }
      event "apply load": Value Change {
        n722 = event-data() -> ()  [unwired: 1 in, 1 out]
        n723 = call-poly "Enqueue Message.vi"("Priority Message? (F)"=TRUE, "Message"="apply load", "Message Queue"=w1003) -> ("error out"=w1001:errorcluster, "dup Message Queue"=w1002:refnum<queue>)  [unwired: 7 in]
      }
      event "BACK": Value Change {
        n724 = event-data() -> ()  [unwired: 1 in, 1 out]
        n725 = call-poly "Enqueue Message.vi"("Priority Message? (F)"=TRUE, "Message"="BACK", "Message Queue"=w1008) -> ("error out"=w1006:errorcluster, "dup Message Queue"=w1007:refnum<queue>)  [unwired: 7 in]
      }
      event "Start Test": Value Change {
        n726 = event-data() -> ()  [unwired: 1 in, 1 out]
        n727 = call-poly "Enqueue Message.vi"("Priority Message? (F)"=TRUE, "Message"="Start Test", "Message Queue"=w1013) -> ("error out"=w1011:errorcluster, "dup Message Queue"=w1012:refnum<queue>)  [unwired: 7 in]
      }
      event "STOP": Value Change {
        n728 = event-data() -> ()  [unwired: 1 in, 1 out]
        n729 = call-poly "Enqueue Message.vi"("Priority Message? (F)"=TRUE, "Message"="STOP", "Message Queue"=w1018) -> ("error out"=w1016:errorcluster, "dup Message Queue"=w1017:refnum<queue>)  [unwired: 7 in]
      }
      event "PlaceModule": Value Change {
        n730 = event-data() -> ()  [unwired: 1 in, 1 out]
        n731 = call-poly "Enqueue Message.vi"("Priority Message? (F)"=TRUE, "Message"="PlaceModule", "Message Queue"=w1023) -> ("error out"=w1021:errorcluster, "dup Message Queue"=w1022:refnum<queue>)  [unwired: 7 in]
      }
      event "HomeRot", "HomeScratch", "HomeScratch": Value Change {
        n732 = event-data() -> ()  [unwired: 1 in, 1 out]
        n733 = call-poly "Enqueue Message.vi"("Priority Message? (F)"=TRUE, "Message"="Stage Homing", "Message Queue"=w1028) -> ("error out"=w1026:errorcluster, "dup Message Queue"=w1027:refnum<queue>)  [unwired: 7 in]
      }
      event "Clear 3": Value Change {
        n734 = event-data() -> ()  [unwired: 1 in, 1 out]
        n735 = call-poly "Enqueue Message.vi"("Priority Message? (F)"=TRUE, "Message"="Clear 3", "Message Queue"=w1033) -> ("error out"=w1031:errorcluster, "dup Message Queue"=w1032:refnum<queue>)  [unwired: 7 in]
      }
      event "Set WTD": Value Change {
        n736 = event-data() -> ()  [unwired: 1 in, 1 out]
        n737 = call-poly "Enqueue Message.vi"("Priority Message? (F)"=TRUE, "Message"="Set WTD", "Message Queue"=w1038) -> ("error out"=w1036:errorcluster, "dup Message Queue"=w1037:refnum<queue>)  [unwired: 7 in]
      }
      event "Import 2": Value Change {
        n738 = event-data() -> ()  [unwired: 1 in, 1 out]
        n739 = call-poly "Enqueue Message.vi"("Priority Message? (F)"=TRUE, "Message"="Import 2", "Message Queue"=w1043) -> ("error out"=w1041:errorcluster, "dup Message Queue"=w1042:refnum<queue>)  [unwired: 7 in]
      }
      event "Save 2": Value Change {
        n740 = event-data() -> ()  [unwired: 1 in, 1 out]
        n741 = call-poly "Enqueue Message.vi"("Priority Message? (F)"=TRUE, "Message"="Save 2", "Message Queue"=w1048) -> ("error out"=w1046:errorcluster, "dup Message Queue"=w1047:refnum<queue>)  [unwired: 7 in]
      }
      event "calculate rotary": Value Change {
        n742 = event-data() -> ()  [unwired: 1 in, 1 out]
        n743 = call-poly "Enqueue Message.vi"("Priority Message? (F)"=TRUE, "Message"="Calculate Rotary", "Message Queue"=w1053) -> ("error out"=w1051:errorcluster, "dup Message Queue"=w1052:refnum<queue>)  [unwired: 7 in]
      }
      event "Clear List": Value Change {
        n744 = event-data() -> ()  [unwired: 1 in, 1 out]
        n745 = call-poly "Enqueue Message.vi"("Priority Message? (F)"=TRUE, "Message"="Clear List", "Message Queue"=w1058) -> ("error out"=w1056:errorcluster, "dup Message Queue"=w1057:refnum<queue>)  [unwired: 7 in]
      }
      event "Add to list": Value Change {
        n746 = event-data() -> ()  [unwired: 1 in, 1 out]
        n747 = call-poly "Enqueue Message.vi"("Priority Message? (F)"=TRUE, "Message"="Add to list", "Message Queue"=w1063) -> ("error out"=w1061:errorcluster, "dup Message Queue"=w1062:refnum<queue>)  [unwired: 7 in]
      }
      event "ClrLog": Value Change {
        n748 = event-data() -> ()  [unwired: 1 in, 1 out]
        n749 = call-poly "Enqueue Message.vi"("Priority Message? (F)"=TRUE, "Message"="ClrLog", "Message Queue"=w1068) -> ("error out"=w1066:errorcluster, "dup Message Queue"=w1067:refnum<queue>)  [unwired: 7 in]
      }
      event "Disable Axis Jog Soft Limits m": Value Change {
        n750 = event-data() -> ()  [unwired: 1 in, 1 out]
        n751 = call-poly "Enqueue Message.vi"("Priority Message? (F)"=TRUE, "Message"="Disable Axis Jog Soft Limits", "Message Queue"=w1073) -> ("error out"=w1071:errorcluster, "dup Message Queue"=w1072:refnum<queue>)  [unwired: 7 in]
      }
      event "Home Service": Value Change {
        n752 = event-data() -> ()  [unwired: 1 in, 1 out]
        n753 = call-poly "Enqueue Message.vi"("Priority Message? (F)"=TRUE, "Message"="Home Service", "Message Queue"=w1078) -> ("error out"=w1076:errorcluster, "dup Message Queue"=w1077:refnum<queue>)  [unwired: 7 in]
      }
      event "Edit Gain Constants": Value Change {
        n754 = event-data() -> ()  [unwired: 1 in, 1 out]
        n755 = call-poly "Enqueue Message.vi"("Priority Message? (F)"=TRUE, "Message"="Edit Gain Constants", "Message Queue"=w1083) -> ("error out"=w1081:errorcluster, "dup Message Queue"=w1082:refnum<queue>)  [unwired: 7 in]
      }
      event "Advanced Setting": Value Change {
        n756 = event-data() -> ()  [unwired: 1 in, 1 out]
        n757 = call-poly "Enqueue Message.vi"("Priority Message? (F)"=TRUE, "Message"="Advanced Setting", "Message Queue"=w1088) -> ("error out"=w1086:errorcluster, "dup Message Queue"=w1087:refnum<queue>)  [unwired: 7 in]
      }
      event "Password": Value Change {
        n758 = event-data() -> ()  [unwired: 1 in, 1 out]
        n759 = call-poly "Enqueue Message.vi"("Priority Message? (F)"=TRUE, "Message"="Password", "Message Queue"=w1093) -> ("error out"=w1091:errorcluster, "dup Message Queue"=w1092:refnum<queue>)  [unwired: 7 in]
      }
      event "Service About": Value Change {
        n760 = event-data() -> ()  [unwired: 1 in, 1 out]
        n761 = call-poly "Enqueue Message.vi"("Priority Message? (F)"=TRUE, "Message"="Service About", "Message Queue"=w1098) -> ("error out"=w1096:errorcluster, "dup Message Queue"=w1097:refnum<queue>)  [unwired: 7 in]
      }
      event "OPEN 1": Value Change {
        n762 = event-data() -> ()  [unwired: 1 in, 1 out]
        n763 = call-poly "Enqueue Message.vi"("Priority Message? (F)"=TRUE, "Message"="OPEN 1", "Message Queue"=w1103) -> ("error out"=w1101:errorcluster, "dup Message Queue"=w1102:refnum<queue>)  [unwired: 7 in]
      }
      event "OPEN 2": Value Change {
        n764 = event-data() -> ()  [unwired: 1 in, 1 out]
        n765 = call-poly "Enqueue Message.vi"("Priority Message? (F)"=TRUE, "Message"="OPEN 2", "Message Queue"=w1108) -> ("error out"=w1106:errorcluster, "dup Message Queue"=w1107:refnum<queue>)  [unwired: 7 in]
      }
      event "OPEN 3": Value Change {
        n766 = event-data() -> ()  [unwired: 1 in, 1 out]
        n767 = call-poly "Enqueue Message.vi"("Priority Message? (F)"=TRUE, "Message"="OPEN 3", "Message Queue"=w1113) -> ("error out"=w1111:errorcluster, "dup Message Queue"=w1112:refnum<queue>)  [unwired: 7 in]
      }
      event "OPEN 4": Value Change {
        n768 = event-data() -> ()  [unwired: 1 in, 1 out]
        n769 = call-poly "Enqueue Message.vi"("Priority Message? (F)"=TRUE, "Message"="OPEN 4", "Message Queue"=w1118) -> ("error out"=w1116:errorcluster, "dup Message Queue"=w1117:refnum<queue>)  [unwired: 7 in]
      }
      event "Refresh 2": Value Change {
        n770 = event-data() -> ()  [unwired: 1 in, 1 out]
        n771 = call-poly "Enqueue Message.vi"("Priority Message? (F)"=TRUE, "Message"="Refresh 2", "Message Queue"=w1123) -> ("error out"=w1121:errorcluster, "dup Message Queue"=w1122:refnum<queue>)  [unwired: 7 in]
      }
      event "Analysis Home new": Value Change {
        n772 = event-data() -> ()  [unwired: 1 in, 1 out]
        n773 = call-poly "Enqueue Message.vi"("Priority Message? (F)"=TRUE, "Message"="Analysis Home", "Message Queue"=w1128) -> ("error out"=w1126:errorcluster, "dup Message Queue"=w1127:refnum<queue>)  [unwired: 7 in]
      }
      event "Post Analysis": Value Change {
        n774 = event-data() -> ()  [unwired: 1 in, 1 out]
        n775 = call-poly "Enqueue Message.vi"("Priority Message? (F)"=TRUE, "Message"="Post Analysis", "Message Queue"=w1133) -> ("error out"=w1131:errorcluster, "dup Message Queue"=w1132:refnum<queue>)  [unwired: 7 in]
      }
      event "Scratch Mode": Value Change {
        n776 = event-data() -> ()  [unwired: 1 in, 1 out]
        n777 = call-poly "Enqueue Message.vi"("Priority Message? (F)"=TRUE, "Message"="Scratch Mode", "Message Queue"=w1138) -> ("error out"=w1136:errorcluster, "dup Message Queue"=w1137:refnum<queue>)  [unwired: 7 in]
      }
      event "Export": Value Change {
        n778 = event-data() -> ()  [unwired: 1 in, 1 out]
        n779 = call-poly "Enqueue Message.vi"("Priority Message? (F)"=TRUE, "Message"="Export", "Message Queue"=w1143) -> ("error out"=w1141:errorcluster, "dup Message Queue"=w1142:refnum<queue>)  [unwired: 7 in]
      }
      event Application Instance Close {
        # "#CodeRecommended - When a project closes, all VIs within that project are aborted and leave memory. However, any code placed in this event frame is guaranteed to run to completion, so add any cleanup code that absolutely must happen here."
        n780 = event-data() -> ()  [unwired: 1 in, 1 out]
      }
      event "EXIT": Value Change {
        n781 = event-data() -> ()  [unwired: 1 in, 1 out]
        n782 = call-poly "Enqueue Message.vi"("Priority Message? (F)"=TRUE, "Message"="Exit", "Message Queue"=w1151) -> ("error out"=w1150:errorcluster, "dup Message Queue"=w1149:refnum<queue>)  [unwired: 7 in]
      }
      event User Event {
        # "The Message Handling Loop processed an \"Exit\" message, which fired this event to stop the Event Handling Loop."
        n783 = event-data() -> ()  [unwired: 1 in, 1 out]
      }
    }
    n784 = call "LAB-IQ Error Handler - Event Handling Loop.vi"("error in (no error)"=w791, "Message Queue"=w789) -> ("dup error in"=w788:errorcluster)  [unwired: 8 in, 1 out]
  }
  n785 = disable-structure shown="Disabled" {
    disable-tunnel: w34 -> [w1158 _]
    disable-tunnel: w28 -> [w1157 _]
    disable-tunnel: w27 -> [w1156 _]
    disable-tunnel: w18 -> [w1155 w1224]
    disable-tunnel: [w1154 w1224] -> w15
    frame Disabled {
      n786 = while {
        shift-right: [w1169] -> _
        shift-left: w1157 -> [w1170]
        tunnel: [w1163] -> w1154
        tunnel: w1158 -> [w1161]
        tunnel: w1155 -> [w1160]
        tunnel: w1156 -> [w1159]
        stop <- w1168 stop-if-true
        # "Temperature  Handling Loop"
        n787 = call "Dequeue Message.vi"("error in (no error)"=w1160, "Message Queue"=w1161) -> ("error out"=w1167:errorcluster, "Message Data"=w1165:variant, "Message"=w1166:string, "dup Message Queue"=w1164:refnum<queue>)  [unwired: 6 in]
        n788 = case "Message Cases" shown="\"Temperature Main\"" w1166 {
          selector: w1166 -> [_ _ _ _ _ w1214]
          tunnel: w1164 -> [w1171 w1182 _ w1201 w1213 _]
          tunnel: w1167 -> [w1174 w1179 w1198 w1205 w1207 _]
          tunnel: [w1175 w1183 w1192 w1203 w1209 w1215] -> w1162
          tunnel: w1170 -> [w1173 w1181 w1197 w1204 w1212 w1216]
          tunnel: [w1173 w1181 w1197 w1204 w1212 w1216] -> w1169
          tunnel: [_ _ _ _ TRUE _] -> w1168
          tunnel: w1165 -> [_ _ w1196 _ _ _]
          tunnel: w1159 -> [_ _ _ _ w1206 _]
          frame "init" {
            # "Initialize - All initialization work should take place in this message, since other loops can potentially enqueue messages that execute immediately after this one."
            n789 = call-poly "Enqueue Message.vi"("error in (no error)"=w1174, "Message"="Temperature Main", "Message Queue"=w1171) -> ("error out"=w1175:errorcluster)  [unwired: 7 in, 1 out]
          }
          frame "Temperature Main" {
            n790 = Unbundle By Name(w1181) -> ("Main Home Screen.EXIT"=w1180:refnum<vi>)
            n791 = property class="Bool (strict)"(reference=w1180) -> (reference out=w1177:refnum<vi>, error out=w1178:errorcluster, "Value"=w1176:bool)  [unwired: 1 in]
            n792 = case shown="False" w1176 {
              tunnel: [w1186 w1190] -> w1183
              tunnel: w1182 -> [w1185 w1189]
              tunnel: w1179 -> [w1184 w1188]
              frame True {
                n793 = call-poly "Enqueue Message.vi"("error in (no error)"=w1184, "Message"="Confirm Quit", "Message Queue"=w1185) -> ("error out"=w1186:errorcluster)  [unwired: 7 in, 1 out]
              }
              frame False {
                n794 = call-poly "Enqueue Message.vi"("error in (no error)"=w1188, "Message"="Temperature Main", "Message Queue"=w1189) -> ("error out"=w1190:errorcluster)  [unwired: 7 in, 1 out]
              }
            }
            n795 = Close Reference(reference=w1177, error in (no error)=w1178) -> ()  [unwired: 1 out]
          }
          frame "Error" {
            # "#CodeRecommended - If you ever change the name of this \"Error\" message, you'll need to update the name in the Check Loop Error.vi as well."
            # "#CodeRecommended - Consider creating a system for logging errors in some way. These errors are for notification purposes only. Handling of specific errors should be performed in the message frames that generated the error."
            # "Error - Display an error dialog. This message is sent by the \"Error Handler\" VIs at the end of other loops in this application."
            n796 = Variant To Data(error in=w1198, type=errorcluster {"status"=FALSE, "code"=0, "source"=""} ("error constant"), Variant=w1196) -> (data=w1194:errorcluster, error out=w1193:errorcluster)
            n797 = call <vilib>:"Simple Error Handler.vi"("error in (no error)"=w1194) -> ()  [unwired: 4 in, 5 out]
            n798 = Merge Errors(w1193) -> (w1192:errorcluster)
          }
          frame "Confirm Quit" {
            # "#CodeNeeded - If you want to provide an \"Are you sure\" dialog (or some other notification) before the application exits, place that code here. This message is typically sent from a Panel Close? event."
            # "Confirm Quit - Message that can confirm whether or not the user wants to exit the application."
            n799 = call-poly "Enqueue Message.vi"("Priority Message? (F)"=TRUE, "error in (no error)"=w1205, "Message"="Exit", "Message Queue"=w1201) -> ("error out"=w1202:errorcluster)  [unwired: 6 in, 1 out]
            n800 = Merge Errors(w1202) -> (w1203:errorcluster)
          }
          frame "Exit" {
            # "Stop the VI"
            # "Release the message queue reference"
            # "#CodeNeeded - Add any required cleanup code here. Note that if 'Exit' was called as a result of an error, an error dialog will be displayed. Add any custom error handling for an 'Exit' condition here as well."
            # "Exit - Exit the application."
            n801 = call "Fire User Event - Stop.vi"("User Event - Stop"=w1206) -> ("error out"=w1208:errorcluster)  [unwired: 10 in]
            n802 = Release Queue(queue=w1213, error in (no error)=w1207) -> (error out=w1210:errorcluster)  [unwired: 1 in, 2 out]
            n803 = Merge Errors(w1208, w1210) -> (w1209:errorcluster)
          }
          frame Default {
            # "'Default' case only runs if there is a message that isn't defined in any of the other cases.  Output a programming error."
            n804 = xnode "Error Ring"("parameter 0"=w1214) -> ("error out"=w1215:errorcluster)
          }
        }
        n805 = call "LAB-IQ Error Handler - Message Handling Loop.vi"("error in (no error)"=w1162, "Message Queue"=w1164) -> ("dup error in"=w1163:errorcluster)  [unwired: 8 in, 1 out]
      }
    }
    frame Enabled {
    }
  }
  n806 = disable-structure shown="Disabled" {
    disable-tunnel: w32 -> [w1228 _]
    disable-tunnel: w28 -> [w1227 _]
    disable-tunnel: w27 -> [w1226 _]
    disable-tunnel: w18 -> [w1225 _]
    frame Disabled {
      n807 = while {
        shift-right: [w1239] -> _
        shift-left: w1227 -> [w1240]
        tunnel: [w1233] -> _
        tunnel: w1228 -> [w1231]
        tunnel: w1225 -> [w1230]
        tunnel: w1226 -> [w1229]
        stop <- w1238 stop-if-true
        # "Ramp Motor  Handling Loop"
        n808 = call "Dequeue Message.vi"("error in (no error)"=w1230, "Message Queue"=w1231) -> ("error out"=w1237:errorcluster, "Message Data"=w1235:variant, "Message"=w1236:string, "dup Message Queue"=w1234:refnum<queue>)  [unwired: 6 in]
        n809 = case "Message Cases" shown="\"Ramp Main\"" w1236 {
          selector: w1236 -> [_ _ _ _ _ w1284]
          tunnel: w1234 -> [w1241 w1252 _ w1271 w1283 _]
          tunnel: w1237 -> [w1244 w1249 w1268 w1275 w1277 _]
          tunnel: [w1245 w1253 w1262 w1273 w1279 w1285] -> w1232
          tunnel: w1240 -> [w1243 w1251 w1267 w1274 w1282 w1286]
          tunnel: [w1243 w1251 w1267 w1274 w1282 w1286] -> w1239
          tunnel: [_ _ _ _ TRUE _] -> w1238
          tunnel: w1235 -> [_ _ w1266 _ _ _]
          tunnel: w1229 -> [_ _ _ _ w1276 _]
          frame "init" {
            # "Initialize - All initialization work should take place in this message, since other loops can potentially enqueue messages that execute immediately after this one."
            n810 = call-poly "Enqueue Message.vi"("error in (no error)"=w1244, "Message"="Ramp Main", "Message Queue"=w1241) -> ("error out"=w1245:errorcluster)  [unwired: 7 in, 1 out]
          }
          frame "Ramp Main" {
            n811 = Unbundle By Name(w1251) -> ("Main Home Screen.EXIT"=w1250:refnum<vi>)
            n812 = property class="Bool (strict)"(reference=w1250) -> (reference out=w1247:refnum<vi>, error out=w1248:errorcluster, "Value"=w1246:bool)  [unwired: 1 in]
            n813 = case shown="False" w1246 {
              tunnel: [w1256 w1260] -> w1253
              tunnel: w1252 -> [w1255 w1259]
              tunnel: w1249 -> [w1254 w1258]
              frame True {
                n814 = call-poly "Enqueue Message.vi"("error in (no error)"=w1254, "Message"="Confirm Quit", "Message Queue"=w1255) -> ("error out"=w1256:errorcluster)  [unwired: 7 in, 1 out]
              }
              frame False {
                n815 = call-poly "Enqueue Message.vi"("error in (no error)"=w1258, "Message"="Ramp Main", "Message Queue"=w1259) -> ("error out"=w1260:errorcluster)  [unwired: 7 in, 1 out]
              }
            }
            n816 = Close Reference(reference=w1247, error in (no error)=w1248) -> ()  [unwired: 1 out]
          }
          frame "Error" {
            # "#CodeRecommended - If you ever change the name of this \"Error\" message, you'll need to update the name in the Check Loop Error.vi as well."
            # "#CodeRecommended - Consider creating a system for logging errors in some way. These errors are for notification purposes only. Handling of specific errors should be performed in the message frames that generated the error."
            # "Error - Display an error dialog. This message is sent by the \"Error Handler\" VIs at the end of other loops in this application."
            n817 = Variant To Data(error in=w1268, type=errorcluster {"status"=FALSE, "code"=0, "source"=""} ("error constant"), Variant=w1266) -> (data=w1264:errorcluster, error out=w1263:errorcluster)
            n818 = call <vilib>:"Simple Error Handler.vi"("error in (no error)"=w1264) -> ()  [unwired: 4 in, 5 out]
            n819 = Merge Errors(w1263) -> (w1262:errorcluster)
          }
          frame "Confirm Quit" {
            # "#CodeNeeded - If you want to provide an \"Are you sure\" dialog (or some other notification) before the application exits, place that code here. This message is typically sent from a Panel Close? event."
            # "Confirm Quit - Message that can confirm whether or not the user wants to exit the application."
            n820 = call-poly "Enqueue Message.vi"("Priority Message? (F)"=TRUE, "error in (no error)"=w1275, "Message"="Exit", "Message Queue"=w1271) -> ("error out"=w1272:errorcluster)  [unwired: 6 in, 1 out]
            n821 = Merge Errors(w1272) -> (w1273:errorcluster)
          }
          frame "Exit" {
            # "Stop the VI"
            # "Release the message queue reference"
            # "#CodeNeeded - Add any required cleanup code here. Note that if 'Exit' was called as a result of an error, an error dialog will be displayed. Add any custom error handling for an 'Exit' condition here as well."
            # "Exit - Exit the application."
            n822 = call "Fire User Event - Stop.vi"("User Event - Stop"=w1276) -> ("error out"=w1278:errorcluster)  [unwired: 10 in]
            n823 = Release Queue(queue=w1283, error in (no error)=w1277) -> (error out=w1280:errorcluster)  [unwired: 1 in, 2 out]
            n824 = Merge Errors(w1278, w1280) -> (w1279:errorcluster)
          }
          frame Default {
            # "'Default' case only runs if there is a message that isn't defined in any of the other cases.  Output a programming error."
            n825 = xnode "Error Ring"("parameter 0"=w1284) -> ("error out"=w1285:errorcluster)
          }
        }
        n826 = call "LAB-IQ Error Handler - Message Handling Loop.vi"("error in (no error)"=w1232, "Message Queue"=w1234) -> ("dup error in"=w1233:errorcluster)  [unwired: 8 in, 1 out]
      }
    }
    frame Enabled {
    }
  }
  n827 = timed-loop {
    shift-right: [w1308] -> _
    shift-left: w28 -> [w1309]
    tunnel: [w1302] -> _
    tunnel: w25 -> [w1300]
    tunnel: w18 -> [w1299]
    tunnel: w27 -> [w1298]
    timing: w3 -> [_]
    timing-out: [_] -> w2
    shift-right: [w1296] -> _
    shift-left: w1 -> [w1297]
    shift-right: [w1294] -> _
    shift-left: w1 -> [w1295]
    stop <- w1307 stop-if-true
    # "Load Pid  Handling Loop"
    n828 = node-c288() -> ()  [unwired: 1 in, 1 out]
    n829 = call "Dequeue Message.vi"("error in (no error)"=w1299, "Message Queue"=w1300) -> ("error out"=w1306:errorcluster, "Message Data"=w1304:variant, "Message"=w1305:string, "dup Message Queue"=w1303:refnum<queue>)  [unwired: 6 in]
    n830 = case "Message Cases" shown="\"Load Pid Main\"" w1305 {
      selector: w1305 -> [_ _ _ _ _ w1397]
      tunnel: w1303 -> [w1314 w1339 _ w1380 w1394 _]
      tunnel: w1306 -> [w1317 w1337 w1375 w1384 w1388 _]
      tunnel: [w1318 w1340 w1369 w1382 w1390 w1398] -> w1301
      tunnel: w1309 -> [w1316 w1326 w1374 w1383 w1393 w1399]
      tunnel: [w1316 w1326 w1374 w1383 w1393 w1399] -> w1308
      tunnel: [_ _ _ _ TRUE _] -> w1307
      tunnel: w1304 -> [_ _ w1373 _ _ _]
      tunnel: w1298 -> [_ _ _ _ w1387 _]
      tunnel: w1297 -> [w1312 w1322 w1368 w1377 w1386 w1395]
      tunnel: [w1312 w1321 w1368 w1377 w1386 w1395] -> w1296
      tunnel: w1295 -> [w1313 w1320 w1367 w1376 w1385 w1396]
      tunnel: [w1313 w1319 w1367 w1376 w1385 w1396] -> w1294
      frame "init" {
        # "Initialize - All initialization work should take place in this message, since other loops can potentially enqueue messages that execute immediately after this one."
        n831 = call-poly "Enqueue Message.vi"("error in (no error)"=w1317, "Message"="Load Pid Main", "Message Queue"=w1314) -> ("error out"=w1318:errorcluster)  [unwired: 7 in, 1 out]
      }
      frame "Load Pid Main" {
        n832 = Unbundle By Name(w1326) -> ("Main Screen.Load En"=w1332:refnum<vi>)
        n833 = Unbundle By Name(w1326) -> ("PID.apply load"=w1327:refnum<vi>)
        n834 = property class="Bool (strict)"(reference=w1332) -> (reference out=w1330:refnum<vi>, error out=w1331:errorcluster, "Value"=w1325:bool)  [unwired: 1 in]
        n835 = property class="Bool (strict)"(reference=w1327) -> (reference out=w1329:refnum<vi>, error out=w1328:errorcluster, "Value"=w1324:bool)  [unwired: 1 in]
        n836 = Close Reference(reference=w1330, error in (no error)=w1331) -> ()  [unwired: 1 out]
        n837 = Close Reference(reference=w1329, error in (no error)=w1328) -> ()  [unwired: 1 out]
        n838 = Or(x=w1325, y=w1324) -> (x .or. y?=w1323:bool)
        n839 = case shown="True" w1323 {
          tunnel: w1337 -> [w1345 w1354]
          tunnel: [w1345 w1353] -> w1333
          tunnel: w1326 -> [_ w1352]
          tunnel: w1322 -> [w1344 w1351]
          tunnel: [w1344 w1350] -> w1321
          tunnel: w1320 -> [w1343 w1349]
          tunnel: [w1343 w1348] -> w1319
          frame False {
            n840 = local write "Checkbox 2"(TRUE ("Checkbox 2")) -> ()
            n841 = local write "Checkbox"(TRUE ("Checkbox")) -> ()
          }
          frame True {
            n842 = case shown="True" "Checkbox 2" {
              selector: "Checkbox 2" -> [_ w1357]
              tunnel: [FALSE ("Checkbox") "Checkbox"] -> w1347
              frame False {
              }
              frame True {
                n843 = Not(x=w1357) -> (.not. x?=w1356:bool)
                n844 = local write "Checkbox 2"(w1356) -> ()
              }
            }
            n845 = call "NEW LOAD CELL PID.vi"("integral_out"=w1349, "error in (no error)"=w1354, "prev_error_out"=w1351, "Checkbox"=w1347, "main ref"=w1352) -> ("error out"=w1353:errorcluster, "prev_error_out"=w1350:dbl, "integral_out"=w1348:dbl)  [unwired: 4 in]
          }
        }
        n846 = Unbundle By Name(w1326) -> ("Main Home Screen.EXIT"=w1338:refnum<vi>)
        n847 = property class="Bool (strict)"(reference=w1338) -> (reference out=w1335:refnum<vi>, error out=w1336:errorcluster, "Value"=w1334:bool)  [unwired: 1 in]
        n848 = case shown="False" w1334 {
          tunnel: [w1361 w1365] -> w1340
          tunnel: w1339 -> [w1360 w1364]
          tunnel: w1333 -> [w1359 w1363]
          frame True {
            n849 = call-poly "Enqueue Message.vi"("error in (no error)"=w1359, "Message"="Confirm Quit", "Message Queue"=w1360) -> ("error out"=w1361:errorcluster)  [unwired: 7 in, 1 out]
          }
          frame False {
            n850 = call-poly "Enqueue Message.vi"("error in (no error)"=w1363, "Message"="Load Pid Main", "Message Queue"=w1364) -> ("error out"=w1365:errorcluster)  [unwired: 7 in, 1 out]
          }
        }
        n851 = Close Reference(reference=w1335, error in (no error)=w1336) -> ()  [unwired: 1 out]
      }
      frame "Error" {
        # "#CodeRecommended - If you ever change the name of this \"Error\" message, you'll need to update the name in the Check Loop Error.vi as well."
        # "#CodeRecommended - Consider creating a system for logging errors in some way. These errors are for notification purposes only. Handling of specific errors should be performed in the message frames that generated the error."
        # "Error - Display an error dialog. This message is sent by the \"Error Handler\" VIs at the end of other loops in this application."
        n852 = Variant To Data(error in=w1375, type=errorcluster {"status"=FALSE, "code"=0, "source"=""} ("error constant"), Variant=w1373) -> (data=w1371:errorcluster, error out=w1370:errorcluster)
        n853 = call <vilib>:"Simple Error Handler.vi"("error in (no error)"=w1371) -> ()  [unwired: 4 in, 5 out]
        n854 = Merge Errors(w1370) -> (w1369:errorcluster)
      }
      frame "Confirm Quit" {
        # "#CodeNeeded - If you want to provide an \"Are you sure\" dialog (or some other notification) before the application exits, place that code here. This message is typically sent from a Panel Close? event."
        # "Confirm Quit - Message that can confirm whether or not the user wants to exit the application."
        n855 = call-poly "Enqueue Message.vi"("Priority Message? (F)"=TRUE, "error in (no error)"=w1384, "Message"="Exit", "Message Queue"=w1380) -> ("error out"=w1381:errorcluster)  [unwired: 6 in, 1 out]
        n856 = Merge Errors(w1381) -> (w1382:errorcluster)
      }
      frame "Exit" {
        # "Stop the VI"
        # "Release the message queue reference"
        # "#CodeNeeded - Add any required cleanup code here. Note that if 'Exit' was called as a result of an error, an error dialog will be displayed. Add any custom error handling for an 'Exit' condition here as well."
        # "Exit - Exit the application."
        n857 = call "Fire User Event - Stop.vi"("User Event - Stop"=w1387) -> ("error out"=w1389:errorcluster)  [unwired: 10 in]
        n858 = Release Queue(queue=w1394, error in (no error)=w1388) -> (error out=w1391:errorcluster)  [unwired: 1 in, 2 out]
        n859 = Merge Errors(w1389, w1391) -> (w1390:errorcluster)
      }
      frame Default {
        # "'Default' case only runs if there is a message that isn't defined in any of the other cases.  Output a programming error."
        n860 = xnode "Error Ring"("parameter 0"=w1397) -> ("error out"=w1398:errorcluster)
      }
    }
    n861 = call "LAB-IQ Error Handler - Message Handling Loop.vi"("error in (no error)"=w1301, "Message Queue"=w1303) -> ("dup error in"=w1302:errorcluster)  [unwired: 8 in, 1 out]
    n862 = node-c288() -> ()  [unwired: 1 in, 1 out]
  }
  n863 = while {
    tunnel: w65 -> [w1410]
    shift-right: [w1417] -> _
    shift-left: w28 -> [w1418]
    tunnel: w27 -> [w1415]
    tunnel: w58 -> [w1414]
    tunnel: [w1408] -> w66
    stop <- w1416 stop-if-true
    # "Message Handling Loop"
    n864 = call "Dequeue Message.vi"("error in (no error)"=w1414, "Message Queue"=w1410) -> ("error out"=w1413:errorcluster, "Message Data"=w1411:variant, "Message"=w1412:string, "dup Message Queue"=w1409:refnum<queue>)  [unwired: 6 in]
    n865 = case "Message Cases" shown="\"Analysis Home\"" w1412 {
      selector: w1412 -> [_ _ _ _ _ _ _ _ _ _ _ _ _ _ _ _ _ _ _ _ _ _ _ _ _ _ _ _ _ _ _ _ _ _ _ _ _ _ _ _ _ _ _ _ _ _ _ _ _ _ _ _ _ _ _ _ _ _ _ _ _ _ _ _ _ _ _ _ _ _ _ _ _ _ w2723]
      tunnel: w1409 -> [_ w1472 _ _ _ _ _ _ _ _ _ _ _ _ _ _ _ _ _ _ _ _ _ _ _ _ _ _ _ _ _ _ _ _ _ _ _ _ _ _ _ _ _ _ _ _ _ _ _ _ _ _ _ _ _ _ _ _ _ _ _ _ _ _ _ _ _ _ _ _ _ _ w2711 w2722 _]
      tunnel: w1413 -> [w1420 w1474 w1476 w1480 w1501 w1518 w1535 w1552 w1573 w1586 w1591 w1595 w1602 w1607 w1672 w1698 w1724 w1759 w1775 w1827 w1831 w1834 w1841 w1884 w1896 w1925 w1955 w1974 w1985 w1996 w2007 w2018 w2029 w2040 w2051 w2063 w2074 w2085 w2096 w2105 w2116 w2127 w2157 w2198 w2204 w2220 w2224 w2227 w2235 w2247 w2256 w2276 w2290 w2300 w2310 w2312 w2327 w2340 w2357 w2374 w2410 w2418 w2477 w2501 w2511 w2552 w2595 w2638 w2674 w2681 w2700 w2707 w2714 w2715 _]
      tunnel: [w1429 w1441 w1476 w1481 w1496 w1513 w1530 w1547 w1568 w1578 w1589 w1593 w1600 w1611 w1668 w1694 w1720 w1760 w1776 w1791 w1830 w1833 w1840 w1883 w1895 w1924 w1942 w1976 w1987 w1998 w2009 w2020 w2031 w2042 w2053 w2064 w2075 w2086 w2097 w2107 w2117 w2126 w2156 w2177 w2203 w2221 w2223 w2226 w2234 w2241 w2251 w2269 w2289 w2300 w2310 w2318 w2326 w2339 w2356 w2373 w2409 w2417 w2477 w2501 w2508 w2549 w2592 w2635 w2675 w2681 w2694 w2701 w2713 w2718 w2724] -> w1407
      tunnel: w1418 -> [w1421 w1432 w1477 w1479 w1487 w1504 w1521 w1538 w1556 w1576 w1588 w1592 w1598 w1606 w1670 w1696 w1722 w1747 w1762 w1778 w1829 w1832 w1835 w1878 w1894 w1907 w1937 w1972 w1983 w1994 w2005 w2016 w2027 w2038 w2049 w2061 w2072 w2083 w2094 w2104 w2115 w2125 w2155 w2176 w2202 w2206 w2222 w2225 w2229 w2240 w2249 w2271 w2288 w2292 w2302 w2311 w2325 w2329 w2342 w2360 w2376 w2412 w2469 w2492 w2504 w2545 w2588 w2631 w2673 w2676 w2693 w2706 w2708 w2721 w2725]
      tunnel: [w1421 w1432 w1477 w1479 w1487 w1504 w1521 w1538 w1556 w1576 w1588 w1592 w1598 w1606 w1670 w1696 w1722 w1747 w1762 w1778 w1829 w1832 w1835 w1878 w1894 w1907 w1937 w1972 w1983 w1994 w2005 w2016 w2027 w2038 w2049 w2061 w2072 w2083 w2094 w2104 w2115 w2125 w2155 w2176 w2202 w2206 w2222 w2225 w2229 w2240 w2249 w2271 w2288 w2292 w2302 w2311 w2325 w2329 w2342 w2360 w2376 w2412 w2469 w2492 w2504 w2545 w2588 w2631 w2673 w2676 w2693 w2706 w2708 w2721 w2725] -> w1417
      tunnel: [_ _ _ _ _ _ _ _ _ _ _ _ _ _ _ _ _ _ _ _ _ _ _ _ _ _ _ _ _ _ _ _ _ _ _ _ _ _ _ _ _ _ _ _ _ _ _ _ _ _ _ _ _ _ _ _ _ _ _ _ _ _ _ _ _ _ _ _ _ _ _ _ _ TRUE _] -> w1416
      tunnel: w1411 -> [_ _ _ _ _ _ _ _ _ _ _ _ _ _ _ _ _ _ _ _ _ _ _ _ _ _ _ _ _ _ _ _ _ _ _ _ _ _ _ _ _ _ _ _ _ _ _ _ _ _ _ _ _ _ _ _ _ _ _ _ _ _ _ _ _ _ _ _ _ _ _ w2705 _ _ _]
      tunnel: w1415 -> [_ _ _ _ _ _ _ _ _ _ _ _ _ _ _ _ _ _ _ _ _ _ _ _ _ _ _ _ _ _ _ _ _ _ _ _ _ _ _ _ _ _ _ _ _ _ _ _ _ _ _ _ _ _ _ _ _ _ _ _ _ _ _ _ _ _ _ _ _ _ _ _ _ w2717 _]
      frame "Time Out" {
        n866 = call "File Name Entereed Check.vi"("error in (no error)"=w1420, "Data Cluster"=w1421) -> ("error out"=w1426:errorcluster)  [unwired: 9 in]
        n867 = call "Load Cell and Susppension Selection Parameter.vi"("error in (no error)"=w1420, "Data Cluster"=w1421) -> ("error out"=w1425:errorcluster)  [unwired: 9 in]
        n868 = call "Load Cell Higher Value in Steps.vi"("error in (no error)"=w1420, "main ref"=w1421) -> ("error out"=w1424:errorcluster)  [unwired: 9 in]
        n869 = call "To Check whether module selected.vi"("error in (no error)"=w1420, "main ref"=w1421) -> ("error out"=w1423:errorcluster)  [unwired: 9 in]
        n870 = call "Rotatry Speed Limit Ristriction.vi"("error in (no error)"=w1420, "main ref"=w1421) -> ("error out"=w1422:errorcluster)  [unwired: 9 in]
        n871 = call "JOG LIMIT.vi"("error in (no error)"=w1420, "main ref"=w1421) -> ("error out"=w1419:errorcluster)  [unwired: 9 in]
        n872 = call "Pulse_mm conversion loop.vi"("error in (no error)"=w1420, "main ref"=w1421) -> ("error out"=w1430:errorcluster)  [unwired: 9 in]
        n873 = call "Load Commiunication Error.vi"("error in (no error)"=w1420, "main ref"=w1421) -> ("error out"=w1427:errorcluster)  [unwired: 9 in]
        n874 = call "Stage Homing Error Display Status.vi"("error in (no error)"=w1420, "Data Cluster"=w1421) -> ("error out"=w1428:errorcluster)  [unwired: 9 in]
        n875 = Merge Errors(w1430, w1427, w1428, w1426, w1425, w1424, w1423, w1422, w1419) -> (w1429:errorcluster)
      }
      frame "init" {
        # "Initialize - All initialization work should take place in this message, since other loops can potentially enqueue messages that execute immediately after this one."
        n876 = call-poly "Enqueue Message.vi"("error in (no error)"=w1474, "Message"="Init Other Loop", "Message Queue"=w1472) -> ("error out"=w1475:errorcluster)  [unwired: 7 in, 1 out]
        n877 = Unbundle By Name(w1432) -> ("Loading.SSP 0.3"=w1460:refnum<vi>)
        n878 = Unbundle By Name(w1432) -> ("Loading.SSP 0.5"=w1457:refnum<vi>)
        n879 = Unbundle By Name(w1432) -> ("Loading.SSP 0.75"=w1452:refnum<vi>)
        n880 = Unbundle By Name(w1432) -> ("Loading.Communication is established"=w1447:refnum<vi>)
        n881 = Unbundle By Name(w1432) -> ("Loading Com Port.Load Cell Temp"=w1466:refnum<vi>)
        n882 = Unbundle By Name(w1432) -> ("Motion Module.Set WTD"=w1440:refnum<vi>)
        n883 = call "Read Config Unitest.vi"("error in (no error)"=w1475, "main ref"=w1432) -> ("error out"=w1470:errorcluster)  [unwired: 9 in]
        n884 = Unbundle By Name(w1432) -> ("Motion Module.Wear Track Diameter"=w1434:refnum<vi>)
        n885 = Unbundle By Name(w1432) -> ("PID.Ramp"=w1444:refnum<vi>)
        n886 = call "Encrypt file path creation.vi"("error in (no error)"=w1470) -> ("error out"=w1469:errorcluster, "File Path"=w1468:path)  [unwired: 9 in]
        n887 = property class="Bool (strict)"(reference=w1466, "Value"=FALSE) -> (reference out=w1464:refnum<vi>, error out=w1465:errorcluster)  [unwired: 1 in]
        n888 = property class="Bool (strict)"(reference=w1457, "Visible"=FALSE) -> (reference out=w1455:refnum<vi>, error out=w1456:errorcluster)  [unwired: 1 in]
        n889 = property class="Bool (strict)"(reference=w1460, "Visible"=FALSE) -> (reference out=w1462:refnum<vi>, error out=w1461:errorcluster)  [unwired: 1 in]
        n890 = property class="Bool (strict)"(reference=w1452, "Visible"=FALSE) -> (reference out=w1454:refnum<vi>, error out=w1453:errorcluster)  [unwired: 1 in]
        n891 = property class="Bool (strict)"(reference=w1444, "Value"=FALSE) -> (reference out=w1446:refnum<vi>, error out=w1445:errorcluster)  [unwired: 1 in]
        n892 = property class="DigNum (strict)"(reference=w1434, "Value"=0.0) -> (reference out=w1433:refnum<vi>, error out=w1435:errorcluster)  [unwired: 1 in]
        n893 = property class="Bool (strict)"(reference=w1440, "Visible"=FALSE, "DisabledEnum"=T16."Disabled and Grayed Out" ("Disabled")) -> (reference out=w1437:refnum<vi>, error out=w1439:errorcluster)  [unwired: 1 in]
        n894 = property class="Bool (strict)"(reference=w1447, "Visible"=FALSE ("Value")) -> (reference out=w1449:refnum<vi>, error out=w1448:errorcluster)  [unwired: 1 in]
        n895 = call "DATA ENCRYPT STRING FILE WRITE.vi"("file path (dialog if empty)"=w1468, "error in (no error)"=w1469, "User Action"="System Booted", "main ref"=w1432) -> ("error out"=w1471:errorcluster)  [unwired: 5 in, 1 out]
        n896 = Close Reference(reference=w1455, error in (no error)=w1456) -> ()  [unwired: 1 out]
        n897 = Close Reference(reference=w1462, error in (no error)=w1461) -> ()  [unwired: 1 out]
        n898 = Close Reference(reference=w1454, error in (no error)=w1453) -> ()  [unwired: 1 out]
        n899 = Close Reference(reference=w1446, error in (no error)=w1445) -> ()  [unwired: 1 out]
        n900 = Close Reference(reference=w1464, error in (no error)=w1465) -> ()  [unwired: 1 out]
        n901 = Close Reference(reference=w1433, error in (no error)=w1435) -> ()  [unwired: 1 out]
        n902 = Close Reference(reference=w1437, error in (no error)=w1439) -> ()  [unwired: 1 out]
        n903 = Close Reference(reference=w1449, error in (no error)=w1448) -> ()  [unwired: 1 out]
        n904 = call "Reinitial Parameter After Test.vi"("error in (no error)"=w1471, "main ref"=w1432) -> ("error out"=w1441:errorcluster)  [unwired: 9 in]
        n905 = local write "HEAVE ENABLE"(FALSE ("HEAVE ENABLE")) -> ()
      }
      frame "Init Other Loop" {
      }
      frame "Service Save" {
        n906 = call "Write Config Unitest.vi"("error in (no error)"=w1480, "main ref"=w1479) -> ("error out"=w1485:errorcluster)  [unwired: 9 in]
        n907 = call "Stall Data Flow.vim"("value in"=w1485, "milliseconds to wait"=u32 2000) -> ("value out"=w1484:errorcluster)  [unwired: 1 out]
        n908 = call "Read Config Unitest.vi"("error in (no error)"=w1484, "main ref"=w1479) -> ("error out"=w1482:errorcluster)  [unwired: 9 in]
        n909 = call "DATA ENCRYPT STRING FILE WRITE.vi"("error in (no error)"=w1482, "User Action"="Service Parameter Saved", "main ref"=w1479) -> ("error out"=w1481:errorcluster)  [unwired: 6 in, 1 out]
      }
      frame "HOME" {
        n910 = call "DATA ENCRYPT STRING FILE WRITE.vi"("error in (no error)"=w1501, "User Action"="User Pressed Home", "main ref"=w1487) -> ("error out"=w1497:errorcluster)  [unwired: 6 in, 1 out]
        n911 = Unbundle By Name(w1487) -> ("Main Home Screen.MainPage"=w1492:refnum<vi>)
        n912 = Unbundle By Name(w1487) -> ("Main Home Screen.Home"=w1500:refnum<vi>)
        n913 = Unbundle By Name(w1487) -> ("Main Home Screen.GUI"=w1490:refnum<vi>)
        n914 = property class="Bool (strict)"(reference=w1500, error in=w1497, "Value"=FALSE) -> (reference out=w1498:refnum<vi>, error out=w1499:errorcluster)
        n915 = property class="TabCtl (strict)"(reference=w1492, "Value"=T5."HOME") -> (reference out=w1494:refnum<vi>, error out=w1493:errorcluster)  [unwired: 1 in]
        n916 = property class="TabCtl (strict)"(reference=w1490, "Value"=T4."Setup") -> (reference out=w1488:refnum<vi>, error out=w1489:errorcluster)  [unwired: 1 in]
        n917 = Close Reference(reference=w1498, error in (no error)=w1499) -> (error out=w1496:errorcluster)
        n918 = Close Reference(reference=w1494, error in (no error)=w1493) -> ()  [unwired: 1 out]
        n919 = Close Reference(reference=w1488, error in (no error)=w1489) -> ()  [unwired: 1 out]
      }
      frame "Platform Setting" {
        n920 = call "DATA ENCRYPT STRING FILE WRITE.vi"("error in (no error)"=w1518, "User Action"="User Pressed Platform Setting", "main ref"=w1504) -> ("error out"=w1514:errorcluster)  [unwired: 6 in, 1 out]
        n921 = Unbundle By Name(w1504) -> ("Main Home Screen.Platform Settings"=w1517:refnum<vi>)
        n922 = Unbundle By Name(w1504) -> ("Main Home Screen.MainPage"=w1509:refnum<vi>)
        n923 = Unbundle By Name(w1504) -> ("Main Home Screen.GUI"=w1507:refnum<vi>)
        n924 = property class="TabCtl (strict)"(reference=w1509, "Value"=T5."PlatformSetting") -> (reference out=w1511:refnum<vi>, error out=w1510:errorcluster)  [unwired: 1 in]
        n925 = property class="TabCtl (strict)"(reference=w1507, "Value"=T4."Setup") -> (reference out=w1505:refnum<vi>, error out=w1506:errorcluster)  [unwired: 1 in]
        n926 = property class="Bool (strict)"(reference=w1517, error in=w1514, "Value"=FALSE) -> (reference out=w1515:refnum<vi>, error out=w1516:errorcluster)
        n927 = Close Reference(reference=w1511, error in (no error)=w1510) -> ()  [unwired: 1 out]
        n928 = Close Reference(reference=w1505, error in (no error)=w1506) -> ()  [unwired: 1 out]
        n929 = Close Reference(reference=w1515, error in (no error)=w1516) -> (error out=w1513:errorcluster)
      }
      frame "Configure" {
        n930 = call "DATA ENCRYPT STRING FILE WRITE.vi"("error in (no error)"=w1535, "User Action"="User Pressed Configure", "main ref"=w1521) -> ("error out"=w1531:errorcluster)  [unwired: 6 in, 1 out]
        n931 = Unbundle By Name(w1521) -> ("Main Home Screen.Configure"=w1534:refnum<vi>)
        n932 = Unbundle By Name(w1521) -> ("Main Home Screen.MainPage"=w1526:refnum<vi>)
        n933 = Unbundle By Name(w1521) -> ("Main Home Screen.GUI"=w1524:refnum<vi>)
        n934 = property class="Bool (strict)"(reference=w1534, error in=w1531, "Value"=FALSE) -> (reference out=w1532:refnum<vi>, error out=w1533:errorcluster)
        n935 = property class="TabCtl (strict)"(reference=w1526, "Value"=T5."Details") -> (reference out=w1528:refnum<vi>, error out=w1527:errorcluster)  [unwired: 1 in]
        n936 = property class="TabCtl (strict)"(reference=w1524, "Value"=T4."Setup") -> (reference out=w1522:refnum<vi>, error out=w1523:errorcluster)  [unwired: 1 in]
        n937 = Close Reference(reference=w1532, error in (no error)=w1533) -> (error out=w1530:errorcluster)
        n938 = Close Reference(reference=w1528, error in (no error)=w1527) -> ()  [unwired: 1 out]
        n939 = Close Reference(reference=w1522, error in (no error)=w1523) -> ()  [unwired: 1 out]
      }
      frame "Analysis" {
        n940 = call "DATA ENCRYPT STRING FILE WRITE.vi"("error in (no error)"=w1552, "User Action"="User Pressed Analysis", "main ref"=w1538) -> ("error out"=w1548:errorcluster)  [unwired: 6 in, 1 out]
        n941 = Unbundle By Name(w1538) -> ("Main Home Screen.MainPage"=w1543:refnum<vi>)
        n942 = Unbundle By Name(w1538) -> ("Main Home Screen.Analysis"=w1551:refnum<vi>)
        n943 = Unbundle By Name(w1538) -> ("Main Home Screen.GUI"=w1541:refnum<vi>)
        n944 = property class="Bool (strict)"(reference=w1551, error in=w1548, "Value"=FALSE) -> (reference out=w1549:refnum<vi>, error out=w1550:errorcluster)
        n945 = property class="TabCtl (strict)"(reference=w1543, "Value"=T5."Analysis") -> (reference out=w1545:refnum<vi>, error out=w1544:errorcluster)  [unwired: 1 in]
        n946 = property class="TabCtl (strict)"(reference=w1541, "Value"=T4."Setup") -> (reference out=w1539:refnum<vi>, error out=w1540:errorcluster)  [unwired: 1 in]
        n947 = Close Reference(reference=w1549, error in (no error)=w1550) -> (error out=w1547:errorcluster)
        n948 = Close Reference(reference=w1545, error in (no error)=w1544) -> ()  [unwired: 1 out]
        n949 = Close Reference(reference=w1539, error in (no error)=w1540) -> ()  [unwired: 1 out]
      }
      frame "service 2" {
        n950 = call "DATA ENCRYPT STRING FILE WRITE.vi"("error in (no error)"=w1573, "User Action"="User Pressed service", "main ref"=w1556) -> ("error out"=w1569:errorcluster)  [unwired: 6 in, 1 out]
        n951 = Unbundle By Name(w1556) -> ("Main Screen.Main Screen Tab"=w1557:refnum<vi>)
        n952 = Unbundle By Name(w1556) -> ("Main Home Screen.MainPage"=w1564:refnum<vi>)
        n953 = Unbundle By Name(w1556) -> ("Main Home Screen.Analysis"=w1572:refnum<vi>)
        n954 = Unbundle By Name(w1556) -> ("Main Home Screen.GUI"=w1562:refnum<vi>)
        n955 = property class="Bool (strict)"(reference=w1572, error in=w1569, "Value"=FALSE) -> (reference out=w1570:refnum<vi>, error out=w1571:errorcluster)
        n956 = property class="TabCtl (strict)"(reference=w1564, "Value"=T5."HOME") -> (reference out=w1566:refnum<vi>, error out=w1565:errorcluster)  [unwired: 1 in]
        n957 = property class="TabCtl (strict)"(reference=w1562, "Value"=T4."Begin") -> (reference out=w1560:refnum<vi>, error out=w1561:errorcluster)  [unwired: 1 in]
        n958 = property class="TabCtl (strict)"(reference=w1557, "Value"=T8."About") -> (reference out=w1554:refnum<vi>, error out=w1558:errorcluster)  [unwired: 1 in]
        n959 = Close Reference(reference=w1570, error in (no error)=w1571) -> (error out=w1568:errorcluster)
        n960 = Close Reference(reference=w1566, error in (no error)=w1565) -> ()  [unwired: 1 out]
        n961 = Close Reference(reference=w1560, error in (no error)=w1561) -> ()  [unwired: 1 out]
        n962 = Close Reference(reference=w1554, error in (no error)=w1558) -> ()  [unwired: 1 out]
      }
      frame "Auto" {
        n963 = call "DATA ENCRYPT STRING FILE WRITE.vi"("error in (no error)"=w1586, "User Action"="User Pressed Auto File Name", "main ref"=w1576) -> ("error out"=w1583:errorcluster)  [unwired: 6 in, 1 out]
        n964 = Get Date/Time In Seconds() -> (seconds since 1Jan1904=w1584:timestamp)
        n965 = Format Into String(format string="%<%I_%M_%S_%p_%d_%B_%Y>T", error in=w1583, w1584) -> (resulting string=w1577:string, error out=w1579:errorcluster)  [unwired: 1 in]
        n966 = local write "Auto"(FALSE ("Auto")) -> ()
        n967 = Unbundle By Name(w1576) -> ("Config Screen.FILE"=w1582:refnum<vi>)
        n968 = property class="Str"(reference=w1582, error in=w1579, "Value"=w1577) -> (reference out=w1580:refnum<vi>, error out=w1581:errorcluster)
        n969 = Close Reference(reference=w1580, error in (no error)=w1581) -> (error out=w1578:errorcluster)
      }
      frame "Select Load Head" {
        n970 = call "Reinitial Parameter.vi"("error in (no error)"=w1591, "Data Cluster"=w1588) -> ("error out"=w1590:errorcluster)  [unwired: 9 in]
        n971 = call "FILE NAME RECHECK.vi"("error in (no error)"=w1590, "main ref"=w1588) -> ("error out"=w1589:errorcluster)  [unwired: 9 in]
      }
      frame "com 3" {
        n972 = call "DATA ENCRYPT STRING FILE WRITE.vi"("error in (no error)"=w1595, "User Action"="User Pressed Check Load Communication", "main ref"=w1592) -> ("error out"=w1594:errorcluster)  [unwired: 6 in, 1 out]
        n973 = call "SET LOAD PARAMETERS.vi"("error in (no error)"=w1594, "main ref"=w1592) -> ("error out"=w1593:errorcluster)  [unwired: 9 in]
      }
      frame "ZeroAll" {
        n974 = call "DATA ENCRYPT STRING FILE WRITE.vi"("error in (no error)"=w1602, "User Action"="User Pressed Zero All", "main ref"=w1598) -> ("error out"=w1601:errorcluster)  [unwired: 6 in, 1 out]
        n975 = local write "ZeroAll"(FALSE ("ZeroAll")) -> ()
        n976 = call "LOAD CELL FGV MAIN.vi"("Enum"=T17."ZEROALL", "error in (no error)"=w1601, "main ref"=w1598) -> ("error IO"=w1600:errorcluster)  [unwired: 8 in]
      }
      frame "Loading Mode" {
        n977 = Unbundle By Name(w1606) -> ("Loading.Loading Mode"=w1608:refnum<vi>)
        n978 = property class="Ring (strict)"(reference=w1608, error in=w1607) -> (reference out=w1610:refnum<vi>, error out=w1609:errorcluster, "Value"=w1604:u16)
        n979 = Close Reference(reference=w1610, error in (no error)=w1609) -> (error out=w1605:errorcluster)
        n980 = case shown="1" w1604 {
          tunnel: [w1625 w1642 w1654 w1666] -> w1611
          tunnel: w1606 -> [w1612 w1628 w1646 w1658]
          tunnel: w1605 -> [w1626 w1641 w1653 w1665]
          frame 0, Default {
            n981 = Unbundle By Name(w1612) -> ("Loading.Enter the Loading Rate (N/min)"=w1619:refnum<vi>)
            n982 = Unbundle By Name(w1612) -> ("Loading.Load Selection"=w1622:refnum<vi>)
            n983 = Unbundle By Name(w1612) -> ("Loading.Enter the Final Load (N)"=w1614:refnum<vi>)
            n984 = property class="TabCtl (strict)"(reference=w1622, "Value"=T6."Constant") -> (reference out=w1624:refnum<vi>, error out=w1623:errorcluster)  [unwired: 1 in]
            n985 = property class="DigNum (strict)"(reference=w1619, "DisabledEnum"=T16."Disabled and Grayed Out" ("Disabled")) -> (reference out=w1618:refnum<vi>, error out=w1620:errorcluster)  [unwired: 1 in]
            n986 = property class="DigNum (strict)"(reference=w1614, "DisabledEnum"=T16."Disabled and Grayed Out" ("Disabled")) -> (reference out=w1615:refnum<vi>, error out=w1613:errorcluster)  [unwired: 1 in]
            n987 = call "DATA ENCRYPT STRING FILE WRITE.vi"("error in (no error)"=w1626, "User Action"="User selected Constant Mode", "main ref"=w1612) -> ("error out"=w1625:errorcluster)  [unwired: 6 in, 1 out]
            n988 = Close Reference(reference=w1624, error in (no error)=w1623) -> ()  [unwired: 1 out]
            n989 = Close Reference(reference=w1618, error in (no error)=w1620) -> ()  [unwired: 1 out]
            n990 = Close Reference(reference=w1615, error in (no error)=w1613) -> ()  [unwired: 1 out]
          }
          frame 1 {
            n991 = Unbundle By Name(w1628) -> ("Loading.Enter the Loading Rate (N/min)"=w1639:refnum<vi>)
            n992 = Unbundle By Name(w1628) -> ("Loading.Enter the Final Load (N)"=w1634:refnum<vi>)
            n993 = Unbundle By Name(w1628) -> ("Loading.Load Selection"=w1630:refnum<vi>)
            n994 = property class="TabCtl (strict)"(reference=w1630, "Value"=T6."Constant") -> (reference out=w1632:refnum<vi>, error out=w1631:errorcluster)  [unwired: 1 in]
            n995 = property class="DigNum (strict)"(reference=w1639, "DisabledEnum"=T16."Enabled" ("Disabled")) -> (reference out=w1638:refnum<vi>, error out=w1640:errorcluster)  [unwired: 1 in]
            n996 = property class="DigNum (strict)"(reference=w1634, "DisabledEnum"=T16."Enabled" ("Disabled")) -> (reference out=w1635:refnum<vi>, error out=w1633:errorcluster)  [unwired: 1 in]
            n997 = call "DATA ENCRYPT STRING FILE WRITE.vi"("error in (no error)"=w1641, "User Action"="User selected Ramp Mode", "main ref"=w1628) -> ("error out"=w1642:errorcluster)  [unwired: 6 in, 1 out]
            n998 = Close Reference(reference=w1632, error in (no error)=w1631) -> ()  [unwired: 1 out]
            n999 = Close Reference(reference=w1638, error in (no error)=w1640) -> ()  [unwired: 1 out]
            n1000 = Close Reference(reference=w1635, error in (no error)=w1633) -> ()  [unwired: 1 out]
          }
          frame 2 {
            n1001 = Unbundle By Name(w1646) -> ("Loading.Load Selection"=w1650:refnum<vi>)
            n1002 = Unbundle By Name(w1646) -> ("Loading.Warning 2"=w1648:refnum<vi>)
            n1003 = property class="TabCtl (strict)"(reference=w1650, "Value"=T6."Step") -> (reference out=w1652:refnum<vi>, error out=w1651:errorcluster)  [unwired: 1 in]
            n1004 = property class="Bool (strict)"(reference=w1648, "Visible"=FALSE) -> (reference out=w1644:refnum<vi>, error out=w1647:errorcluster)  [unwired: 1 in]
            n1005 = call "DATA ENCRYPT STRING FILE WRITE.vi"("error in (no error)"=w1653, "User Action"="User selected Step Mode", "main ref"=w1646) -> ("error out"=w1654:errorcluster)  [unwired: 6 in, 1 out]
            n1006 = Close Reference(reference=w1652, error in (no error)=w1651) -> ()  [unwired: 1 out]
            n1007 = Close Reference(reference=w1644, error in (no error)=w1647) -> ()  [unwired: 1 out]
          }
          frame 3 {
            n1008 = Unbundle By Name(w1658) -> ("Loading.Load Selection"=w1662:refnum<vi>)
            n1009 = Unbundle By Name(w1658) -> ("Loading.Warning 2"=w1660:refnum<vi>)
            n1010 = property class="TabCtl (strict)"(reference=w1662, "Value"=T6."Indentation") -> (reference out=w1664:refnum<vi>, error out=w1663:errorcluster)  [unwired: 1 in]
            n1011 = property class="Bool (strict)"(reference=w1660, "Visible"=FALSE) -> (reference out=w1656:refnum<vi>, error out=w1659:errorcluster)  [unwired: 1 in]
            n1012 = call "DATA ENCRYPT STRING FILE WRITE.vi"("error in (no error)"=w1665, "User Action"="User selected Indentation Mode", "main ref"=w1658) -> ("error out"=w1666:errorcluster)  [unwired: 6 in, 1 out]
            n1013 = Close Reference(reference=w1664, error in (no error)=w1663) -> ()  [unwired: 1 out]
            n1014 = Close Reference(reference=w1656, error in (no error)=w1659) -> ()  [unwired: 1 out]
          }
        }
      }
      frame "SSP 0.3" {
        n1015 = Unbundle By Name(w1670) -> ("Loading.SSP 0.3"=w1673:refnum<vi>)
        n1016 = property class="Bool (strict)"(reference=w1673, error in=w1672) -> (reference out=w1675:refnum<vi>, error out=w1674:errorcluster, "Value"=w1671:bool)
        n1017 = Close Reference(reference=w1675, error in (no error)=w1674) -> (error out=w1669:errorcluster)
        n1018 = case shown="True" w1671 {
          tunnel: w1670 -> [_ w1677]
          tunnel: w1669 -> [w1676 w1685]
          tunnel: [w1676 w1684] -> w1668
          frame False {
          }
          frame True {
            w1687 = FALSE ("Value")
            n1019 = Unbundle By Name(w1677) -> ("Loading.Enter the Load  (N)"=w1683:refnum<vi>)
            n1020 = Unbundle By Name(w1677) -> ("Loading.SSP 0.75"=w1688:refnum<vi>)
            n1021 = Unbundle By Name(w1677) -> ("Loading.SSP 0.5"=w1693:refnum<vi>)
            n1022 = property class="Bool (strict)"(reference=w1688, "Value"=w1687) -> (reference out=w1690:refnum<vi>, error out=w1689:errorcluster)  [unwired: 1 in]
            n1023 = property class="Bool (strict)"(reference=w1693, "Value"=w1687) -> (reference out=w1691:refnum<vi>, error out=w1692:errorcluster)  [unwired: 1 in]
            n1024 = property class="DigNum (strict)"(reference=w1683, "Minimum"=2.0 ("Data Entry Limits:Minimum"), "Maximum"=50.0 ("Data Entry Limits:Maximum"), "Increment"=0.1 ("Data Entry Limits:Increment")) -> (reference out=w1681:refnum<vi>, error out=w1682:errorcluster)  [unwired: 1 in]
            n1025 = call "DATA ENCRYPT STRING FILE WRITE.vi"("error in (no error)"=w1685, "User Action"="User selected 0.3 SSP", "main ref"=w1677) -> ("error out"=w1684:errorcluster)  [unwired: 6 in, 1 out]
            n1026 = Close Reference(reference=w1690, error in (no error)=w1689) -> ()  [unwired: 1 out]
            n1027 = Close Reference(reference=w1691, error in (no error)=w1692) -> ()  [unwired: 1 out]
            n1028 = Close Reference(reference=w1681, error in (no error)=w1682) -> ()  [unwired: 1 out]
          }
        }
      }
      frame "SSP 0.5" {
        n1029 = Unbundle By Name(w1696) -> ("Loading.SSP 0.5"=w1699:refnum<vi>)
        n1030 = property class="Bool (strict)"(reference=w1699, error in=w1698) -> (reference out=w1701:refnum<vi>, error out=w1700:errorcluster, "Value"=w1697:bool)
        n1031 = Close Reference(reference=w1701, error in (no error)=w1700) -> (error out=w1695:errorcluster)
        n1032 = case shown="True" w1697 {
          tunnel: w1696 -> [_ w1703]
          tunnel: w1695 -> [w1702 w1711]
          tunnel: [w1702 w1710] -> w1694
          frame False {
          }
          frame True {
            w1713 = FALSE ("Value")
            n1033 = Unbundle By Name(w1703) -> ("Loading.Enter the Load  (N)"=w1709:refnum<vi>)
            n1034 = Unbundle By Name(w1703) -> ("Loading.SSP 0.75"=w1719:refnum<vi>)
            n1035 = Unbundle By Name(w1703) -> ("Loading.SSP 0.3"=w1714:refnum<vi>)
            n1036 = property class="Bool (strict)"(reference=w1714, "Value"=w1713) -> (reference out=w1716:refnum<vi>, error out=w1715:errorcluster)  [unwired: 1 in]
            n1037 = property class="Bool (strict)"(reference=w1719, "Value"=w1713) -> (reference out=w1717:refnum<vi>, error out=w1718:errorcluster)  [unwired: 1 in]
            n1038 = property class="DigNum (strict)"(reference=w1709, "Minimum"=2.0 ("Data Entry Limits:Minimum"), "Maximum"=200.0 ("Data Entry Limits:Maximum"), "Increment"=0.1 ("Data Entry Limits:Increment")) -> (reference out=w1707:refnum<vi>, error out=w1708:errorcluster)  [unwired: 1 in]
            n1039 = call "DATA ENCRYPT STRING FILE WRITE.vi"("error in (no error)"=w1711, "User Action"="User selected 0.5 SSP", "main ref"=w1703) -> ("error out"=w1710:errorcluster)  [unwired: 6 in, 1 out]
            n1040 = Close Reference(reference=w1716, error in (no error)=w1715) -> ()  [unwired: 1 out]
            n1041 = Close Reference(reference=w1717, error in (no error)=w1718) -> ()  [unwired: 1 out]
            n1042 = Close Reference(reference=w1707, error in (no error)=w1708) -> ()  [unwired: 1 out]
          }
        }
      }
      frame "SSP 0.75" {
        n1043 = Unbundle By Name(w1722) -> ("Loading.SSP 0.75"=w1725:refnum<vi>)
        n1044 = property class="Bool (strict)"(reference=w1725, error in=w1724) -> (reference out=w1727:refnum<vi>, error out=w1726:errorcluster, "Value"=w1723:bool)
        n1045 = Close Reference(reference=w1727, error in (no error)=w1726) -> (error out=w1721:errorcluster)
        n1046 = case shown="True" w1723 {
          tunnel: w1722 -> [_ w1729]
          tunnel: w1721 -> [w1728 w1737]
          tunnel: [w1728 w1736] -> w1720
          frame False {
          }
          frame True {
            w1739 = FALSE ("Value")
            n1047 = Unbundle By Name(w1729) -> ("Loading.SSP 0.3"=w1740:refnum<vi>)
            n1048 = Unbundle By Name(w1729) -> ("Loading.SSP 0.5"=w1745:refnum<vi>)
            n1049 = Unbundle By Name(w1729) -> ("Loading.Enter the Load  (N)"=w1735:refnum<vi>)
            n1050 = property class="Bool (strict)"(reference=w1740, "Value"=w1739) -> (reference out=w1742:refnum<vi>, error out=w1741:errorcluster)  [unwired: 1 in]
            n1051 = property class="Bool (strict)"(reference=w1745, "Value"=w1739) -> (reference out=w1743:refnum<vi>, error out=w1744:errorcluster)  [unwired: 1 in]
            n1052 = property class="DigNum (strict)"(reference=w1735, "Minimum"=200.0 ("Data Entry Limits:Minimum"), "Maximum"=500.0 ("Data Entry Limits:Maximum"), "Increment"=0.1 ("Data Entry Limits:Increment")) -> (reference out=w1733:refnum<vi>, error out=w1734:errorcluster)  [unwired: 1 in]
            n1053 = call "DATA ENCRYPT STRING FILE WRITE.vi"("error in (no error)"=w1737, "User Action"="User selected 0.75 SSP", "main ref"=w1729) -> ("error out"=w1736:errorcluster)  [unwired: 6 in, 1 out]
            n1054 = Close Reference(reference=w1742, error in (no error)=w1741) -> ()  [unwired: 1 out]
            n1055 = Close Reference(reference=w1743, error in (no error)=w1744) -> ()  [unwired: 1 out]
            n1056 = Close Reference(reference=w1733, error in (no error)=w1734) -> ()  [unwired: 1 out]
          }
        }
      }
      frame "LHBack" {
        # "Back to Configure"
        n1057 = Unbundle By Name(w1747) -> ("Main Home Screen.GUI"=w1756:refnum<vi>)
        n1058 = Unbundle By Name(w1747) -> ("Main Home Screen.MainPage"=w1752:refnum<vi>)
        n1059 = Unbundle By Name(w1747) -> ("Loading.LHBack"=w1750:refnum<vi>)
        n1060 = property class="TabCtl (strict)"(reference=w1752, "Value"=T5."HOME") -> (reference out=w1754:refnum<vi>, error out=w1753:errorcluster)  [unwired: 1 in]
        n1061 = property class="Bool (strict)"(reference=w1750, "Value"=FALSE) -> (reference out=w1748:refnum<vi>, error out=w1749:errorcluster)  [unwired: 1 in]
        n1062 = property class="TabCtl (strict)"(reference=w1756, "Value"=T4."Setup") -> (reference out=w1758:refnum<vi>, error out=w1757:errorcluster)  [unwired: 1 in]
        n1063 = Close Reference(reference=w1754, error in (no error)=w1753) -> ()  [unwired: 1 out]
        n1064 = Close Reference(reference=w1748, error in (no error)=w1749) -> ()  [unwired: 1 out]
        n1065 = Close Reference(reference=w1758, error in (no error)=w1757) -> ()  [unwired: 1 out]
        n1066 = call "DATA ENCRYPT STRING FILE WRITE.vi"("error in (no error)"=w1759, "User Action"="User selected Back to Configure", "main ref"=w1747) -> ("error out"=w1760:errorcluster)  [unwired: 6 in, 1 out]
      }
      frame "MMBack" {
        # "Back to Configure"
        n1067 = Unbundle By Name(w1762) -> ("Motion Module.MMBack"=w1766:refnum<vi>)
        n1068 = Unbundle By Name(w1762) -> ("Main Home Screen.GUI"=w1772:refnum<vi>)
        n1069 = Unbundle By Name(w1762) -> ("Main Home Screen.MainPage"=w1768:refnum<vi>)
        n1070 = property class="Bool (strict)"(reference=w1766, "Value"=FALSE) -> (reference out=w1764:refnum<vi>, error out=w1765:errorcluster)  [unwired: 1 in]
        n1071 = property class="TabCtl (strict)"(reference=w1768, "Value"=T5."HOME") -> (reference out=w1770:refnum<vi>, error out=w1769:errorcluster)  [unwired: 1 in]
        n1072 = property class="TabCtl (strict)"(reference=w1772, "Value"=T4."Load Head") -> (reference out=w1774:refnum<vi>, error out=w1773:errorcluster)  [unwired: 1 in]
        n1073 = Close Reference(reference=w1764, error in (no error)=w1765) -> ()  [unwired: 1 out]
        n1074 = Close Reference(reference=w1770, error in (no error)=w1769) -> ()  [unwired: 1 out]
        n1075 = Close Reference(reference=w1774, error in (no error)=w1773) -> ()  [unwired: 1 out]
        n1076 = call "DATA ENCRYPT STRING FILE WRITE.vi"("error in (no error)"=w1775, "User Action"="User selected Back to Load Selection", "main ref"=w1762) -> ("error out"=w1776:errorcluster)  [unwired: 6 in, 1 out]
      }
      frame "LHNext" {
        w1812 = FALSE ("Visible")
        n1077 = Unbundle By Name(w1778) -> ("Motion Module.HomeRot"=w1818:refnum<vi>)
        n1078 = Unbundle By Name(w1778) -> ("Motion Module.HomeScratch"=w1813:refnum<vi>)
        n1079 = Unbundle By Name(w1778) -> ("Motion Module.PlaceModule"=w1811:refnum<vi>)
        n1080 = Unbundle By Name(w1778) -> ("Motion Module.Motion Mode:"=w1804:refnum<vi>)
        n1081 = Unbundle By Name(w1778) -> ("Motion Module.Motion Direction:  3"=w1803:refnum<vi>)
        n1082 = Unbundle By Name(w1778) -> ("Motion Module.Wear Track Diameter (mm)"=w1797:refnum<vi>)
        n1083 = Unbundle By Name(w1778) -> ("Motion Module.Set WTD"=w1794:refnum<vi>)
        n1084 = Unbundle By Name(w1778) -> ("Motion Module.Rotary Module Selection"=w1788:refnum<vi>)
        n1085 = call "DATA ENCRYPT STRING FILE WRITE.vi"("error in (no error)"=w1827, "User Action"="User selected Select Module", "main ref"=w1778) -> ("error out"=w1791:errorcluster)  [unwired: 6 in, 1 out]
        n1086 = property class="TabCtl (strict)"(reference=w1788, "Visible"=FALSE) -> (reference out=w1787:refnum<vi>, error out=w1789:errorcluster)  [unwired: 1 in]
        n1087 = property class="Bool (strict)"(reference=w1818, error in=w1791, "Visible"=w1812) -> (reference out=w1816:refnum<vi>, error out=w1817:errorcluster)
        n1088 = property class="Bool (strict)"(reference=w1813, error in=w1791, "Visible"=w1812) -> (reference out=w1815:refnum<vi>, error out=w1814:errorcluster)
        n1089 = property class="Bool (strict)"(reference=w1811, error in=w1791, "Visible"=TRUE) -> (reference out=w1809:refnum<vi>, error out=w1810:errorcluster)
        n1090 = property class="Ring (strict)"(reference=w1804, error in=w1791, "Visible"=FALSE) -> (reference out=w1806:refnum<vi>, error out=w1805:errorcluster)
        n1091 = property class="Ring (strict)"(reference=w1803, error in=w1791, "Visible"=FALSE) -> (reference out=w1800:refnum<vi>, error out=w1802:errorcluster)
        n1092 = property class="DigNum (strict)"(reference=w1797, "Visible"=FALSE) -> (reference out=w1796:refnum<vi>, error out=w1798:errorcluster)  [unwired: 1 in]
        n1093 = property class="Bool (strict)"(reference=w1794, "Visible"=FALSE) -> (reference out=w1795:refnum<vi>, error out=w1793:errorcluster)  [unwired: 1 in]
        n1094 = Close Reference(reference=w1816, error in (no error)=w1817) -> ()  [unwired: 1 out]
        n1095 = Close Reference(reference=w1815, error in (no error)=w1814) -> ()  [unwired: 1 out]
        n1096 = Close Reference(reference=w1809, error in (no error)=w1810) -> ()  [unwired: 1 out]
        n1097 = Close Reference(reference=w1806, error in (no error)=w1805) -> ()  [unwired: 1 out]
        n1098 = Close Reference(reference=w1800, error in (no error)=w1802) -> ()  [unwired: 1 out]
        n1099 = Close Reference(reference=w1796, error in (no error)=w1798) -> ()  [unwired: 1 out]
        n1100 = Close Reference(reference=w1787, error in (no error)=w1789) -> ()  [unwired: 1 out]
        n1101 = Close Reference(reference=w1795, error in (no error)=w1793) -> ()  [unwired: 1 out]
        n1102 = Unbundle By Name(w1778) -> ("Motion Module.M3 Image"=w1786:refnum<vi>)
        n1103 = Unbundle By Name(w1778) -> ("Main Home Screen.GUI"=w1824:refnum<vi>)
        n1104 = Unbundle By Name(w1778) -> ("Main Home Screen.MainPage"=w1820:refnum<vi>)
        n1105 = Unbundle By Name(w1778) -> ("Loading.LHNext"=w1782:refnum<vi>)
        n1106 = property class="TabCtl (strict)"(reference=w1786, "Value"=enum32{"Page 1", "Page 2"}."Page 2") -> (reference out=w1784:refnum<vi>, error out=w1785:errorcluster)  [unwired: 1 in]
        n1107 = property class="TabCtl (strict)"(reference=w1820, "Value"=T5."HOME") -> (reference out=w1822:refnum<vi>, error out=w1821:errorcluster)  [unwired: 1 in]
        n1108 = property class="TabCtl (strict)"(reference=w1824, "Value"=T4."Motion Module") -> (reference out=w1826:refnum<vi>, error out=w1825:errorcluster)  [unwired: 1 in]
        n1109 = property class="Bool (strict)"(reference=w1782, "Value"=FALSE ("Visible")) -> (reference out=w1779:refnum<vi>, error out=w1781:errorcluster)  [unwired: 1 in]
        n1110 = Close Reference(reference=w1784, error in (no error)=w1785) -> ()  [unwired: 1 out]
        n1111 = Close Reference(reference=w1779, error in (no error)=w1781) -> ()  [unwired: 1 out]
        n1112 = Close Reference(reference=w1822, error in (no error)=w1821) -> ()  [unwired: 1 out]
        n1113 = Close Reference(reference=w1826, error in (no error)=w1825) -> ()  [unwired: 1 out]
      }
      frame "Rot Ver" {
        n1114 = call "Rotory Module Selection.vi"("error in (no error)"=w1831, "Data Cluster"=w1829) -> ("error out"=w1830:errorcluster)  [unwired: 9 in]
      }
      frame "Scratch" {
        n1115 = call "Scratch Module Selection.vi"("error in (no error)"=w1834, "Data Cluster"=w1832) -> ("error out"=w1833:errorcluster)  [unwired: 9 in]
      }
      frame "Motion Mode:" {
        n1116 = Unbundle By Name(w1835) -> ("Motion Module.Motion Mode:"=w1837:refnum<vi>)
        n1117 = property class="Ring (strict)"(reference=w1837) -> (reference out=w1839:refnum<vi>, error out=w1838:errorcluster, "Value"=w1836:u16)  [unwired: 1 in]
        n1118 = Close Reference(reference=w1839, error in (no error)=w1838) -> ()  [unwired: 1 out]
        n1119 = case shown="3" w1836 {
          tunnel: w1841 -> [w1850 w1859 w1868 w1877]
          tunnel: [w1849 w1858 w1867 w1876] -> w1840
          tunnel: w1835 -> [w1848 w1857 w1866 w1875]
          tunnel: w1835 -> [w1843 w1852 w1861 w1870]
          frame 0, Default {
            n1120 = Unbundle By Name(w1843) -> ("Motion Module.Rotary Module Selection"=w1844:refnum<vi>)
            n1121 = property class="TabCtl (strict)"(reference=w1844, "Value"=T7."Uniform Rotation") -> (reference out=w1846:refnum<vi>, error out=w1845:errorcluster)  [unwired: 1 in]
            n1122 = Close Reference(reference=w1846, error in (no error)=w1845) -> ()  [unwired: 1 out]
            n1123 = call "DATA ENCRYPT STRING FILE WRITE.vi"("error in (no error)"=w1850, "User Action"="User Selected Uniform Rotation", "main ref"=w1848) -> ("error out"=w1849:errorcluster)  [unwired: 6 in, 1 out]
          }
          frame 1 {
            n1124 = Unbundle By Name(w1852) -> ("Motion Module.Rotary Module Selection"=w1853:refnum<vi>)
            n1125 = property class="TabCtl (strict)"(reference=w1853, "Value"=T7."Angular Oscillation") -> (reference out=w1855:refnum<vi>, error out=w1854:errorcluster)  [unwired: 1 in]
            n1126 = Close Reference(reference=w1855, error in (no error)=w1854) -> ()  [unwired: 1 out]
            n1127 = call "DATA ENCRYPT STRING FILE WRITE.vi"("error in (no error)"=w1859, "User Action"="User Selected Angular Oscillation", "main ref"=w1857) -> ("error out"=w1858:errorcluster)  [unwired: 6 in, 1 out]
          }
          frame 2 {
            n1128 = Unbundle By Name(w1861) -> ("Motion Module.Rotary Module Selection"=w1862:refnum<vi>)
            n1129 = property class="TabCtl (strict)"(reference=w1862, "Value"=T7."Speed Ramp") -> (reference out=w1864:refnum<vi>, error out=w1863:errorcluster)  [unwired: 1 in]
            n1130 = Close Reference(reference=w1864, error in (no error)=w1863) -> ()  [unwired: 1 out]
            n1131 = call "DATA ENCRYPT STRING FILE WRITE.vi"("error in (no error)"=w1868, "User Action"="User Selected Ramp Mode", "main ref"=w1866) -> ("error out"=w1867:errorcluster)  [unwired: 6 in, 1 out]
          }
          frame 3 {
            n1132 = Unbundle By Name(w1870) -> ("Motion Module.Rotary Module Selection"=w1871:refnum<vi>)
            n1133 = property class="TabCtl (strict)"(reference=w1871, "Value"=T7."Speed Step") -> (reference out=w1873:refnum<vi>, error out=w1872:errorcluster)  [unwired: 1 in]
            n1134 = Close Reference(reference=w1873, error in (no error)=w1872) -> ()  [unwired: 1 out]
            n1135 = call "DATA ENCRYPT STRING FILE WRITE.vi"("error in (no error)"=w1877, "User Action"="User Selected Step Mode", "main ref"=w1875) -> ("error out"=w1876:errorcluster)  [unwired: 6 in, 1 out]
          }
        }
      }
      frame "MMNext" {
        n1136 = Unbundle By Name(w1878) -> ("Motion Module.MMNext"=w1882:refnum<vi>)
        n1137 = Unbundle By Name(w1878) -> ("Motion Module.MMNext"=w1889:refnum<vi>)
        n1138 = Unbundle By Name(w1878) -> ("Main Home Screen.GUI"=w1891:refnum<vi>)
        n1139 = property class="Bool (strict)"(reference=w1882, "Value"=FALSE ("Visible")) -> (reference out=w1879:refnum<vi>, error out=w1881:errorcluster)  [unwired: 1 in]
        n1140 = property class="TabCtl (strict)"(reference=w1891, "Value"=T4."Environment") -> (reference out=w1893:refnum<vi>, error out=w1892:errorcluster)  [unwired: 1 in]
        n1141 = property class="Bool (strict)"(reference=w1889, "Value"=FALSE) -> (reference out=w1887:refnum<vi>, error out=w1888:errorcluster)  [unwired: 1 in]
        n1142 = Close Reference(reference=w1879, error in (no error)=w1881) -> ()  [unwired: 1 out]
        n1143 = Close Reference(reference=w1887, error in (no error)=w1888) -> ()  [unwired: 1 out]
        n1144 = Close Reference(reference=w1893, error in (no error)=w1892) -> ()  [unwired: 1 out]
        n1145 = call "DATA ENCRYPT STRING FILE WRITE.vi"("error in (no error)"=w1884, "User Action"="User Selected SetUp Module", "main ref"=w1878) -> ("error out"=w1883:errorcluster)  [unwired: 6 in, 1 out]
      }
      frame "APBack" {
        n1146 = Unbundle By Name(w1894) -> ("Environmental control.APBack"=w1901:refnum<vi>)
        n1147 = Unbundle By Name(w1894) -> ("Main Home Screen.GUI"=w1903:refnum<vi>)
        n1148 = property class="TabCtl (strict)"(reference=w1903, "Value"=T4."Motion Module") -> (reference out=w1905:refnum<vi>, error out=w1904:errorcluster)  [unwired: 1 in]
        n1149 = property class="Bool (strict)"(reference=w1901, "Value"=FALSE) -> (reference out=w1899:refnum<vi>, error out=w1900:errorcluster)  [unwired: 1 in]
        n1150 = Close Reference(reference=w1899, error in (no error)=w1900) -> ()  [unwired: 1 out]
        n1151 = Close Reference(reference=w1905, error in (no error)=w1904) -> ()  [unwired: 1 out]
        n1152 = call "DATA ENCRYPT STRING FILE WRITE.vi"("error in (no error)"=w1896, "User Action"="User Selected Back to Module", "main ref"=w1894) -> ("error out"=w1895:errorcluster)  [unwired: 6 in, 1 out]
      }
      frame "SNext" {
        w1918 = FALSE ("Value")
        n1153 = Unbundle By Name(w1907) -> ("Main Screen.zNL 2"=w1910:refnum<vi>)
        n1154 = Unbundle By Name(w1907) -> ("Main Screen.Start Test"=w1921:refnum<vi>)
        n1155 = Unbundle By Name(w1907) -> ("Main Screen.STOP"=w1920:refnum<vi>)
        n1156 = Unbundle By Name(w1907) -> ("Environmental control.SNext"=w1930:refnum<vi>)
        n1157 = Unbundle By Name(w1907) -> ("Main Home Screen.GUI"=w1932:refnum<vi>)
        n1158 = Unbundle By Name(w1907) -> ("PID.Ramp"=w1913:refnum<vi>)
        n1159 = property class="Bool (strict)"(reference=w1910, "DisabledEnum"=T16."Enabled" ("Disabled")) -> (reference out=w1908:refnum<vi>, error out=w1909:errorcluster)  [unwired: 1 in]
        n1160 = property class="Bool (strict)"(reference=w1913, "Value"=FALSE) -> (reference out=w1911:refnum<vi>, error out=w1914:errorcluster)  [unwired: 1 in]
        n1161 = property class="Bool (strict)"(reference=w1921, "Visible"=TRUE ("Value"), "Value"=FALSE) -> (reference out=w1916:refnum<vi>, error out=w1922:errorcluster)  [unwired: 1 in]
        n1162 = property class="Bool (strict)"(reference=w1920, "Value"=w1918, "Visible"=w1918) -> (reference out=w1915:refnum<vi>, error out=w1919:errorcluster)  [unwired: 1 in]
        n1163 = property class="TabCtl (strict)"(reference=w1932, "Value"=T4."Begin") -> (reference out=w1934:refnum<vi>, error out=w1933:errorcluster)  [unwired: 1 in]
        n1164 = property class="Bool (strict)"(reference=w1930, "Value"=FALSE) -> (reference out=w1928:refnum<vi>, error out=w1929:errorcluster)  [unwired: 1 in]
        n1165 = Close Reference(reference=w1908, error in (no error)=w1909) -> ()  [unwired: 1 out]
        n1166 = Close Reference(reference=w1911, error in (no error)=w1914) -> ()  [unwired: 1 out]
        n1167 = Close Reference(reference=w1916, error in (no error)=w1922) -> ()  [unwired: 1 out]
        n1168 = Close Reference(reference=w1915, error in (no error)=w1919) -> ()  [unwired: 1 out]
        n1169 = Close Reference(reference=w1928, error in (no error)=w1929) -> ()  [unwired: 1 out]
        n1170 = Close Reference(reference=w1934, error in (no error)=w1933) -> ()  [unwired: 1 out]
        n1171 = call "DATA ENCRYPT STRING FILE WRITE.vi"("error in (no error)"=w1925, "User Action"="User Pressed Setup", "main ref"=w1907) -> ("error out"=w1924:errorcluster)  [unwired: 6 in, 1 out]
      }
      frame "Enable Platform" {
        n1172 = Unbundle By Name(w1937) -> ("Heave AND Surge.Sequence ID"=w1939:refnum<vi>)
        n1173 = Unbundle By Name(w1937) -> ("Heave AND Surge.Mode Command"=w1963:refnum<vi>)
        n1174 = Unbundle By Name(w1937) -> ("Heave AND Surge.Distance"=w1960:refnum<vi>)
        n1175 = Unbundle By Name(w1937) -> ("Heave AND Surge.SPEED"=w1957:refnum<vi>)
        n1176 = Unbundle By Name(w1937) -> ("Platform Settings.Enable Platform"=w1971:refnum<vi>)
        n1177 = property class="DigNum (strict)"(reference=w1939, "Value"=u16 0) -> (reference out=w1938:refnum<vi>, error out=w1940:errorcluster)  [unwired: 1 in]
        n1178 = property class="DigNum (strict)"(reference=w1960, error in=w1955, "Value"=sgl 0.0) -> (reference out=w1961:refnum<vi>, error out=w1959:errorcluster)
        n1179 = property class="DigNum (strict)"(reference=w1957, error in=w1955, "Value"=sgl 0.0) -> (reference out=w1958:refnum<vi>, error out=w1956:errorcluster)
        n1180 = property class="DigNum (strict)"(reference=w1963, error in=w1955, "Value"=u8 1) -> (reference out=w1962:refnum<vi>, error out=w1964:errorcluster)
        n1181 = property class="Bool (strict)"(reference=w1971, "Value"=FALSE) -> (reference out=w1969:refnum<vi>, error out=w1970:errorcluster)  [unwired: 1 in]
        n1182 = Close Reference(reference=w1938, error in (no error)=w1940) -> (error out=w1936:errorcluster)
        n1183 = Close Reference(reference=w1961, error in (no error)=w1959) -> (error out=w1952:errorcluster)
        n1184 = Close Reference(reference=w1958, error in (no error)=w1956) -> (error out=w1951:errorcluster)
        n1185 = Close Reference(reference=w1962, error in (no error)=w1964) -> (error out=w1953:errorcluster)
        n1186 = Close Reference(reference=w1969, error in (no error)=w1970) -> ()  [unwired: 1 out]
        n1187 = Merge Errors(w1955, w1953, w1952, w1951, w1936) -> (w1954:errorcluster)
        n1188 = call "DATA ENCRYPT STRING FILE WRITE.vi"("error in (no error)"=w1954, "User Action"="User Pressed Enable Platform", "main ref"=w1937) -> ("error out"=w1966:errorcluster)  [unwired: 6 in, 1 out]
        n1189 = call "HEAVE WRITE FGV.vi"("Enum - Menu"=Heave_Write_enum."WRITE", "error in (no error)"=w1966, "main ref"=w1937) -> ("error out"=w1943:errorcluster)  [unwired: 8 in]
        n1190 = Unbundle By Name(w1937) -> ("Heave AND Surge.Read Heave Temp"=w1947:refnum<vi>)
        n1191 = property class="Bool (strict)"(reference=w1947, error in=w1943, "Value"=TRUE) -> (reference out=w1945:refnum<vi>, error out=w1946:errorcluster)
        n1192 = Close Reference(reference=w1945, error in (no error)=w1946) -> (error out=w1942:errorcluster)
        "HEAVE ENABLE" <- TRUE ("HEAVE ENABLE")
      }
      frame "Heave Up main" {
        n1193 = Unbundle By Name(w1972) -> ("Platform Settings.Heave Up main"=w1982:refnum<vi>)
        n1194 = call "Heave Up Main.vi"("error in (no error)"=w1974, "main ref"=w1972) -> ("error out"=w1973:errorcluster)  [unwired: 9 in]
        n1195 = property class="Bool (strict)"(reference=w1982, "Value"=FALSE) -> (reference out=w1980:refnum<vi>, error out=w1981:errorcluster)  [unwired: 1 in]
        n1196 = Close Reference(reference=w1980, error in (no error)=w1981) -> ()  [unwired: 1 out]
        n1197 = call "DATA ENCRYPT STRING FILE WRITE.vi"("error in (no error)"=w1973, "User Action"="User Pressed Heave UP", "main ref"=w1972) -> ("error out"=w1977:errorcluster)  [unwired: 6 in, 1 out]
        n1198 = call "HEAVE WRITE FGV.vi"("Enum - Menu"=Heave_Write_enum."WRITE", "error in (no error)"=w1977, "main ref"=w1972) -> ("error out"=w1976:errorcluster)  [unwired: 8 in]
      }
      frame "Heave Up MM" {
        n1199 = Unbundle By Name(w1983) -> ("Motion Module.Heave Up MM"=w1993:refnum<vi>)
        n1200 = call "Heave Up Motion Module.vi"("error in (no error)"=w1985, "main ref"=w1983) -> ("error out"=w1984:errorcluster)  [unwired: 9 in]
        n1201 = property class="Bool (strict)"(reference=w1993, "Value"=FALSE) -> (reference out=w1991:refnum<vi>, error out=w1992:errorcluster)  [unwired: 1 in]
        n1202 = Close Reference(reference=w1991, error in (no error)=w1992) -> ()  [unwired: 1 out]
        n1203 = call "DATA ENCRYPT STRING FILE WRITE.vi"("error in (no error)"=w1984, "User Action"="User Pressed Heave UP in Motion Module", "main ref"=w1983) -> ("error out"=w1988:errorcluster)  [unwired: 6 in, 1 out]
        n1204 = call "HEAVE WRITE FGV.vi"("Enum - Menu"=Heave_Write_enum."WRITE", "error in (no error)"=w1988, "main ref"=w1983) -> ("error out"=w1987:errorcluster)  [unwired: 8 in]
      }
      frame "Heave Down Main" {
        n1205 = call "Heave Down Main.vi"("error in (no error)"=w1996, "main ref"=w1994) -> ("error out"=w1995:errorcluster)  [unwired: 9 in]
        n1206 = Unbundle By Name(w1994) -> ("Platform Settings.Heave Down Main"=w2004:refnum<vi>)
        n1207 = property class="Bool (strict)"(reference=w2004, "Value"=FALSE) -> (reference out=w2002:refnum<vi>, error out=w2003:errorcluster)  [unwired: 1 in]
        n1208 = Close Reference(reference=w2002, error in (no error)=w2003) -> ()  [unwired: 1 out]
        n1209 = call "DATA ENCRYPT STRING FILE WRITE.vi"("error in (no error)"=w1995, "User Action"="User Pressed Heave DOWN", "main ref"=w1994) -> ("error out"=w1999:errorcluster)  [unwired: 6 in, 1 out]
        n1210 = call "HEAVE WRITE FGV.vi"("Enum - Menu"=Heave_Write_enum."WRITE", "error in (no error)"=w1999, "main ref"=w1994) -> ("error out"=w1998:errorcluster)  [unwired: 8 in]
      }
      frame "Heave Down MM" {
        n1211 = call "Heave Down Motion Module.vi"("error in (no error)"=w2007, "main ref"=w2005) -> ("error out"=w2006:errorcluster)  [unwired: 9 in]
        n1212 = Unbundle By Name(w2005) -> ("Motion Module.Heave Down MM"=w2015:refnum<vi>)
        n1213 = property class="Bool (strict)"(reference=w2015, "Value"=FALSE) -> (reference out=w2013:refnum<vi>, error out=w2014:errorcluster)  [unwired: 1 in]
        n1214 = Close Reference(reference=w2013, error in (no error)=w2014) -> ()  [unwired: 1 out]
        n1215 = call "DATA ENCRYPT STRING FILE WRITE.vi"("error in (no error)"=w2006, "User Action"="User Pressed Heave DOWN in Motion Module", "main ref"=w2005) -> ("error out"=w2010:errorcluster)  [unwired: 6 in, 1 out]
        n1216 = call "HEAVE WRITE FGV.vi"("Enum - Menu"=Heave_Write_enum."WRITE", "error in (no error)"=w2010, "main ref"=w2005) -> ("error out"=w2009:errorcluster)  [unwired: 8 in]
      }
      frame "Surge Backward Main" {
        n1217 = Unbundle By Name(w2016) -> ("Platform Settings.Surge Backward Main"=w2026:refnum<vi>)
        n1218 = call "Surge Backward Main.vi"("error in (no error)"=w2018, "main ref"=w2016) -> ("error out"=w2017:errorcluster)  [unwired: 9 in]
        n1219 = property class="Bool (strict)"(reference=w2026, "Value"=FALSE) -> (reference out=w2024:refnum<vi>, error out=w2025:errorcluster)  [unwired: 1 in]
        n1220 = Close Reference(reference=w2024, error in (no error)=w2025) -> ()  [unwired: 1 out]
        n1221 = call "DATA ENCRYPT STRING FILE WRITE.vi"("error in (no error)"=w2017, "User Action"="User Pressed Surge Backward", "main ref"=w2016) -> ("error out"=w2021:errorcluster)  [unwired: 6 in, 1 out]
        n1222 = call "HEAVE WRITE FGV.vi"("Enum - Menu"=Heave_Write_enum."WRITE", "error in (no error)"=w2021, "main ref"=w2016) -> ("error out"=w2020:errorcluster)  [unwired: 8 in]
      }
      frame "Surge Backward MM" {
        n1223 = Unbundle By Name(w2027) -> ("Motion Module.Surge Backward MM"=w2037:refnum<vi>)
        n1224 = call "Surge Backward Main.vi"("error in (no error)"=w2029, "main ref"=w2027) -> ("error out"=w2028:errorcluster)  [unwired: 9 in]
        n1225 = property class="Bool (strict)"(reference=w2037, "Value"=FALSE) -> (reference out=w2035:refnum<vi>, error out=w2036:errorcluster)  [unwired: 1 in]
        n1226 = Close Reference(reference=w2035, error in (no error)=w2036) -> ()  [unwired: 1 out]
        n1227 = call "DATA ENCRYPT STRING FILE WRITE.vi"("error in (no error)"=w2028, "User Action"="User Pressed Surge Backward in Motion Module", "main ref"=w2027) -> ("error out"=w2032:errorcluster)  [unwired: 6 in, 1 out]
        n1228 = call "HEAVE WRITE FGV.vi"("Enum - Menu"=Heave_Write_enum."WRITE", "error in (no error)"=w2032, "main ref"=w2027) -> ("error out"=w2031:errorcluster)  [unwired: 8 in]
      }
      frame "Surge Forward Main" {
        n1229 = Unbundle By Name(w2038) -> ("Platform Settings.Surge Forward Main"=w2048:refnum<vi>)
        n1230 = call "Surge Forward Main.vi"("error in (no error)"=w2040, "main ref"=w2038) -> ("error out"=w2039:errorcluster)  [unwired: 9 in]
        n1231 = property class="Bool (strict)"(reference=w2048, "Value"=FALSE) -> (reference out=w2046:refnum<vi>, error out=w2047:errorcluster)  [unwired: 1 in]
        n1232 = Close Reference(reference=w2046, error in (no error)=w2047) -> ()  [unwired: 1 out]
        n1233 = call "DATA ENCRYPT STRING FILE WRITE.vi"("error in (no error)"=w2039, "User Action"="User Pressed Surge Forward", "main ref"=w2038) -> ("error out"=w2043:errorcluster)  [unwired: 6 in, 1 out]
        n1234 = call "HEAVE WRITE FGV.vi"("Enum - Menu"=Heave_Write_enum."WRITE", "error in (no error)"=w2043, "main ref"=w2038) -> ("error out"=w2042:errorcluster)  [unwired: 8 in]
      }
      frame "Surge Forward MM" {
        n1235 = Unbundle By Name(w2049) -> ("Motion Module.Surge Forward MM"=w2059:refnum<vi>)
        n1236 = call "Surge Forward MM.vi"("error in (no error)"=w2051, "main ref"=w2049) -> ("error out"=w2050:errorcluster)  [unwired: 9 in]
        n1237 = property class="Bool (strict)"(reference=w2059, "Value"=FALSE) -> (reference out=w2057:refnum<vi>, error out=w2058:errorcluster)  [unwired: 1 in]
        n1238 = Close Reference(reference=w2057, error in (no error)=w2058) -> ()  [unwired: 1 out]
        n1239 = call "DATA ENCRYPT STRING FILE WRITE.vi"("error in (no error)"=w2050, "User Action"="User Pressed Surge Forward in Motion Module", "main ref"=w2049) -> ("error out"=w2054:errorcluster)  [unwired: 6 in, 1 out]
        n1240 = call "HEAVE WRITE FGV.vi"("Enum - Menu"=Heave_Write_enum."WRITE", "error in (no error)"=w2054, "main ref"=w2049) -> ("error out"=w2053:errorcluster)  [unwired: 8 in]
      }
      frame "Sway Left Main" {
        n1241 = call "Sway Left Main.vi"("error in (no error)"=w2063, "main ref"=w2061) -> ("error out"=w2062:errorcluster)  [unwired: 9 in]
        n1242 = Unbundle By Name(w2061) -> ("Platform Settings.Sway Left Main"=w2070:refnum<vi>)
        n1243 = property class="Bool (strict)"(reference=w2070, "Value"=FALSE) -> (reference out=w2068:refnum<vi>, error out=w2069:errorcluster)  [unwired: 1 in]
        n1244 = Close Reference(reference=w2068, error in (no error)=w2069) -> ()  [unwired: 1 out]
        n1245 = call "DATA ENCRYPT STRING FILE WRITE.vi"("error in (no error)"=w2062, "User Action"="User Pressed Sway Left ", "main ref"=w2061) -> ("error out"=w2065:errorcluster)  [unwired: 6 in, 1 out]
        n1246 = call "SWAY WRITE FGV.vi"("Enum - Menu"=Sway_Write_enum."WRITE", "error in (no error)"=w2065, "main ref"=w2061) -> ("error out"=w2064:errorcluster)  [unwired: 8 in]
      }
      frame "Sway Left MM" {
        n1247 = call "Sway Left MM.vi"("error in (no error)"=w2074, "main ref"=w2072) -> ("error out"=w2073:errorcluster)  [unwired: 9 in]
        n1248 = Unbundle By Name(w2072) -> ("Motion Module.Sway Left MM"=w2081:refnum<vi>)
        n1249 = property class="Bool (strict)"(reference=w2081, "Value"=FALSE) -> (reference out=w2079:refnum<vi>, error out=w2080:errorcluster)  [unwired: 1 in]
        n1250 = Close Reference(reference=w2079, error in (no error)=w2080) -> ()  [unwired: 1 out]
        n1251 = call "DATA ENCRYPT STRING FILE WRITE.vi"("error in (no error)"=w2073, "User Action"="User Pressed Sway Left in MM", "main ref"=w2072) -> ("error out"=w2076:errorcluster)  [unwired: 6 in, 1 out]
        n1252 = call "SWAY WRITE FGV.vi"("Enum - Menu"=Sway_Write_enum."WRITE", "error in (no error)"=w2076, "main ref"=w2072) -> ("error out"=w2075:errorcluster)  [unwired: 8 in]
      }
      frame "Sway Right MM" {
        n1253 = call "Sway Right MM.vi"("error in (no error)"=w2085, "main ref"=w2083) -> ("error out"=w2084:errorcluster)  [unwired: 9 in]
        n1254 = Unbundle By Name(w2083) -> ("Motion Module.Sway Right MM"=w2092:refnum<vi>)
        n1255 = property class="Bool (strict)"(reference=w2092, "Value"=FALSE) -> (reference out=w2090:refnum<vi>, error out=w2091:errorcluster)  [unwired: 1 in]
        n1256 = Close Reference(reference=w2090, error in (no error)=w2091) -> ()  [unwired: 1 out]
        n1257 = call "DATA ENCRYPT STRING FILE WRITE.vi"("error in (no error)"=w2084, "User Action"="User Pressed Sway Right in MM", "main ref"=w2083) -> ("error out"=w2087:errorcluster)  [unwired: 6 in, 1 out]
        n1258 = call "SWAY WRITE FGV.vi"("Enum - Menu"=Sway_Write_enum."WRITE", "error in (no error)"=w2087, "main ref"=w2083) -> ("error out"=w2086:errorcluster)  [unwired: 8 in]
      }
      frame "Sway Right Main" {
        n1259 = call "Sway Right Main.vi"("error in (no error)"=w2096, "main ref"=w2094) -> ("error out"=w2095:errorcluster)  [unwired: 9 in]
        n1260 = Unbundle By Name(w2094) -> ("Platform Settings.Sway Right Main"=w2103:refnum<vi>)
        n1261 = property class="Bool (strict)"(reference=w2103, "Value"=FALSE) -> (reference out=w2101:refnum<vi>, error out=w2102:errorcluster)  [unwired: 1 in]
        n1262 = Close Reference(reference=w2101, error in (no error)=w2102) -> ()  [unwired: 1 out]
        n1263 = call "DATA ENCRYPT STRING FILE WRITE.vi"("error in (no error)"=w2095, "User Action"="User Pressed Sway Right", "main ref"=w2094) -> ("error out"=w2098:errorcluster)  [unwired: 6 in, 1 out]
        n1264 = call "SWAY WRITE FGV.vi"("Enum - Menu"=Sway_Write_enum."WRITE", "error in (no error)"=w2098, "main ref"=w2094) -> ("error out"=w2097:errorcluster)  [unwired: 8 in]
      }
      frame "Manual Write Heave & Surge" {
        n1265 = Unbundle By Name(w2104) -> ("Heave AND Surge.Manual Write"=w2113:refnum<vi>)
        n1266 = property class="Bool (strict)"(reference=w2113, "Value"=FALSE) -> (reference out=w2111:refnum<vi>, error out=w2112:errorcluster)  [unwired: 1 in]
        n1267 = Close Reference(reference=w2111, error in (no error)=w2112) -> ()  [unwired: 1 out]
        n1268 = call "DATA ENCRYPT STRING FILE WRITE.vi"("error in (no error)"=w2105, "User Action"="User Pressed Manual Write Heave and Surge", "main ref"=w2104) -> ("error out"=w2108:errorcluster)  [unwired: 6 in, 1 out]
        n1269 = call "HEAVE WRITE FGV.vi"("Enum - Menu"=Heave_Write_enum."WRITE", "error in (no error)"=w2108, "main ref"=w2104) -> ("error out"=w2107:errorcluster)  [unwired: 8 in]
      }
      frame "Manual Write SWAY" {
        n1270 = Unbundle By Name(w2115) -> ("SWAY.Manual Write SWAY"=w2123:refnum<vi>)
        n1271 = property class="Bool (strict)"(reference=w2123, "Value"=FALSE) -> (reference out=w2121:refnum<vi>, error out=w2122:errorcluster)  [unwired: 1 in]
        n1272 = Close Reference(reference=w2121, error in (no error)=w2122) -> ()  [unwired: 1 out]
        n1273 = call "DATA ENCRYPT STRING FILE WRITE.vi"("error in (no error)"=w2116, "User Action"="User Pressed Manual Write Sway", "main ref"=w2115) -> ("error out"=w2118:errorcluster)  [unwired: 6 in, 1 out]
        n1274 = call "SWAY WRITE FGV.vi"("Enum - Menu"=Sway_Write_enum."WRITE", "error in (no error)"=w2118, "main ref"=w2115) -> ("error out"=w2117:errorcluster)  [unwired: 8 in]
      }
      frame "Load En" {
        # "zNL 2"
        n1275 = Unbundle By Name(w2125) -> ("Main Screen.Load En"=w2130:refnum<vi>)
        n1276 = property class="Bool (strict)"(reference=w2130) -> (reference out=w2128:refnum<vi>, error out=w2129:errorcluster, "Value"=w2124:bool)  [unwired: 1 in]
        n1277 = Close Reference(reference=w2128, error in (no error)=w2129) -> ()  [unwired: 1 out]
        n1278 = case shown="False" w2124 {
          tunnel: [w2142 w2152] -> w2126
          tunnel: w2127 -> [w2144 w2151]
          tunnel: w2125 -> [w2132 w2146]
          tunnel: w2125 -> [w2140 _]
          tunnel: w2125 -> [w2139 _]
          frame False {
            n1279 = call "DATA ENCRYPT STRING FILE WRITE.vi"("error in (no error)"=w2144, "User Action"="User Pressed UnLoad on Main Screen", "main ref"=w2132) -> ("error out"=w2133:errorcluster)  [unwired: 6 in, 1 out]
            n1280 = call "Stall Data Flow.vim"("value in"=w2133, "milliseconds to wait"=u32 2000) -> ("value out"=w2138:errorcluster)  [unwired: 1 out]
            n1281 = Unbundle By Name(w2132) -> ("Main Screen.zNL 2"=w2136:refnum<vi>)
            n1282 = property class="Bool (strict)"(reference=w2136, "DisabledEnum"=T16."Enabled" ("Disabled")) -> (reference out=w2134:refnum<vi>, error out=w2135:errorcluster)  [unwired: 1 in]
            n1283 = call "PID UNLOAD.vi"("error in (no error)"=w2138, "main ref"=w2139) -> ("error out"=w2141:errorcluster)  [unwired: 9 in]
            n1284 = Close Reference(reference=w2134, error in (no error)=w2135) -> ()  [unwired: 1 out]
            n1285 = call "HEAVE WRITE FGV.vi"("Enum - Menu"=Heave_Write_enum."WRITE", "error in (no error)"=w2141, "main ref"=w2140) -> ("error out"=w2142:errorcluster)  [unwired: 8 in]
          }
          frame True {
            n1286 = call "DATA ENCRYPT STRING FILE WRITE.vi"("error in (no error)"=w2151, "User Action"="User Pressed Load on Main Screen", "main ref"=w2146) -> ("error out"=w2152:errorcluster)  [unwired: 6 in, 1 out]
            n1287 = Unbundle By Name(w2146) -> ("Main Screen.zNL 2"=w2150:refnum<vi>)
            n1288 = property class="Bool (strict)"(reference=w2150, "DisabledEnum"=T16."Disabled and Grayed Out" ("Disabled")) -> (reference out=w2148:refnum<vi>, error out=w2149:errorcluster)  [unwired: 1 in]
            n1289 = Close Reference(reference=w2148, error in (no error)=w2149) -> ()  [unwired: 1 out]
          }
        }
      }
      frame "apply load" {
        n1290 = Unbundle By Name(w2155) -> ("Main Screen.Load En"=w2160:refnum<vi>)
        n1291 = property class="Bool (strict)"(reference=w2160) -> (reference out=w2158:refnum<vi>, error out=w2159:errorcluster, "Value"=w2154:bool)  [unwired: 1 in]
        n1292 = Close Reference(reference=w2158, error in (no error)=w2159) -> ()  [unwired: 1 out]
        n1293 = case shown="False" w2154 {
          tunnel: [w2167 w2174] -> w2156
          tunnel: w2157 -> [w2170 w2173]
          tunnel: w2155 -> [w2169 w2172]
          tunnel: w2155 -> [w2164 _]
          tunnel: w2155 -> [w2163 _]
          frame False {
            n1294 = call "DATA ENCRYPT STRING FILE WRITE.vi"("error in (no error)"=w2170, "User Action"="User Pressed UnLoad on Service Screen", "main ref"=w2169) -> ("error out"=w2166:errorcluster)  [unwired: 6 in, 1 out]
            n1295 = call "Stall Data Flow.vim"("value in"=w2166, "milliseconds to wait"=u32 2000) -> ("value out"=w2162:errorcluster)  [unwired: 1 out]
            n1296 = call "PID UNLOAD.vi"("error in (no error)"=w2162, "main ref"=w2163) -> ("error out"=w2165:errorcluster)  [unwired: 9 in]
            n1297 = call "HEAVE WRITE FGV.vi"("Enum - Menu"=Heave_Write_enum."WRITE", "error in (no error)"=w2165, "main ref"=w2164) -> ("error out"=w2167:errorcluster)  [unwired: 8 in]
          }
          frame True {
            n1298 = call "DATA ENCRYPT STRING FILE WRITE.vi"("error in (no error)"=w2173, "User Action"="User Pressed Load on Service Screen", "main ref"=w2172) -> ("error out"=w2174:errorcluster)  [unwired: 6 in, 1 out]
          }
        }
      }
      frame "BACK" {
        w2181 = FALSE ("Value")
        n1299 = Unbundle By Name(w2176) -> ("Main Screen.BACK"=w2201:refnum<vi>)
        n1300 = property class="Bool (strict)"(reference=w2201, "Value"=FALSE) -> (reference out=w2199:refnum<vi>, error out=w2200:errorcluster)  [unwired: 1 in]
        n1301 = Close Reference(reference=w2199, error in (no error)=w2200) -> ()  [unwired: 1 out]
        n1302 = call "DATA ENCRYPT STRING FILE WRITE.vi"("error in (no error)"=w2198, "User Action"="User Pressed Back on Main Screen", "main ref"=w2176) -> ("error out"=w2196:errorcluster)  [unwired: 6 in, 1 out]
        n1303 = Unbundle By Name(w2176) -> ("Main Home Screen.MainPage"=w2188:refnum<vi>)
        n1304 = Unbundle By Name(w2176) -> ("Main Screen.Start Test"=w2184:refnum<vi>)
        n1305 = Unbundle By Name(w2176) -> ("Main Screen.STOP"=w2183:refnum<vi>)
        n1306 = Unbundle By Name(w2176) -> ("Main Home Screen.GUI"=w2192:refnum<vi>)
        n1307 = property class="TabCtl (strict)"(reference=w2188, "Value"=T5."HOME") -> (reference out=w2190:refnum<vi>, error out=w2189:errorcluster)  [unwired: 1 in]
        n1308 = property class="TabCtl (strict)"(reference=w2192, "Value"=T4."Setup") -> (reference out=w2194:refnum<vi>, error out=w2193:errorcluster)  [unwired: 1 in]
        n1309 = property class="Bool (strict)"(reference=w2184, "Visible"=TRUE ("Value"), "Value"=FALSE) -> (reference out=w2179:refnum<vi>, error out=w2185:errorcluster)  [unwired: 1 in]
        n1310 = property class="Bool (strict)"(reference=w2183, "Value"=w2181, "Visible"=w2181) -> (reference out=w2178:refnum<vi>, error out=w2182:errorcluster)  [unwired: 1 in]
        n1311 = Close Reference(reference=w2194, error in (no error)=w2193) -> ()  [unwired: 1 out]
        n1312 = Close Reference(reference=w2190, error in (no error)=w2189) -> ()  [unwired: 1 out]
        n1313 = Close Reference(reference=w2179, error in (no error)=w2185) -> ()  [unwired: 1 out]
        n1314 = Close Reference(reference=w2178, error in (no error)=w2182) -> ()  [unwired: 1 out]
        n1315 = call "Reinitial Parameter After Test.vi"("error in (no error)"=w2196, "main ref"=w2176) -> ("error out"=w2177:errorcluster)  [unwired: 9 in]
      }
      frame "Start Test" {
        n1316 = call "Test Start Sequence.vi"("error in (no error)"=w2204, "Data Cluster"=w2202) -> ("error out"=w2203:errorcluster)  [unwired: 9 in]
      }
      frame "STOP" {
        n1317 = Unbundle By Name(w2206) -> ("Main Screen.Load En"=w2219:refnum<vi>)
        n1318 = Unbundle By Name(w2206) -> ("Main Screen.CZ FF"=w2214:refnum<vi>)
        n1319 = Unbundle By Name(w2206) -> ("Main Screen.zFF"=w2211:refnum<vi>)
        n1320 = property class="Bool (strict)"(reference=w2219, "DisabledEnum"=T16."Disabled and Grayed Out" ("Disabled")) -> (reference out=w2207:refnum<vi>, error out=w2218:errorcluster)  [unwired: 1 in]
        n1321 = property class="Bool (strict)"(reference=w2214, "DisabledEnum"=T16."Disabled and Grayed Out" ("Disabled"), "Value"=FALSE ("Visible")) -> (reference out=w2213:refnum<vi>, error out=w2215:errorcluster)  [unwired: 1 in]
        n1322 = property class="Bool (strict)"(reference=w2211, "DisabledEnum"=T16."Disabled and Grayed Out" ("Disabled"), "Value"=FALSE ("Visible")) -> (reference out=w2212:refnum<vi>, error out=w2210:errorcluster)  [unwired: 1 in]
        n1323 = Close Reference(reference=w2207, error in (no error)=w2218) -> ()  [unwired: 1 out]
        n1324 = Close Reference(reference=w2213, error in (no error)=w2215) -> ()  [unwired: 1 out]
        n1325 = Close Reference(reference=w2212, error in (no error)=w2210) -> ()  [unwired: 1 out]
        n1326 = call "Test Stop.vi"("error in (no error)"=w2220, "Data Cluster"=w2206) -> ("error out"=w2221:errorcluster)  [unwired: 9 in]
      }
      frame "PlaceModule" {
        n1327 = call "Place Module.vi"("error in (no error)"=w2224, "main ref"=w2222) -> ("error out"=w2223:errorcluster)  [unwired: 9 in]
      }
      frame "Stage Homing" {
        n1328 = call "HOMINING.vi"("error in (no error)"=w2227, "main ref"=w2225) -> ("error out"=w2226:errorcluster)  [unwired: 9 in]
      }
      frame "Clear 3" {
        n1329 = Unbundle By Name(w2229) -> ("Loading.Stribeck Table  For loading"=w2239:refnum<vi>)
        n1330 = Unbundle By Name(w2229) -> ("Loading.Clear 3"=w2230:refnum<vi>)
        n1331 = property class="Bool (strict)"(reference=w2230, "Value"=FALSE) -> (reference out=w2232:refnum<vi>, error out=w2231:errorcluster)  [unwired: 1 in]
        n1332 = call "DATA ENCRYPT STRING FILE WRITE.vi"("error in (no error)"=w2235, "User Action"="User Pressed Clear  on Step Load Sequence", "main ref"=w2229) -> ("error out"=w2234:errorcluster)  [unwired: 6 in, 1 out]
        n1333 = property class="Tbl (strict)"(reference=w2239, "Value"=string[][] []) -> (reference out=w2237:refnum<vi>, error out=w2238:errorcluster)  [unwired: 1 in]
        n1334 = Close Reference(reference=w2232, error in (no error)=w2231) -> ()  [unwired: 1 out]
        n1335 = Close Reference(reference=w2237, error in (no error)=w2238) -> ()  [unwired: 1 out]
      }
      frame "Set WTD" {
        n1336 = Unbundle By Name(w2240) -> ("Motion Module.Set WTD"=w2243:refnum<vi>)
        n1337 = property class="Bool (strict)"(reference=w2243, "Value"=FALSE) -> (reference out=w2245:refnum<vi>, error out=w2244:errorcluster)  [unwired: 1 in]
        n1338 = call "DATA ENCRYPT STRING FILE WRITE.vi"("error in (no error)"=w2247, "User Action"="User Pressed  on Set Wear Track", "main ref"=w2240) -> ("error out"=w2246:errorcluster)  [unwired: 6 in, 1 out]
        n1339 = call "Sway wear trac set.vi"("error in (no error)"=w2246, "main ref"=w2240) -> ("error out"=w2241:errorcluster)  [unwired: 9 in]
        n1340 = Close Reference(reference=w2245, error in (no error)=w2244) -> ()  [unwired: 1 out]
      }
      frame "Import 2" {
        n1341 = call "File Dialog"("start path"=path "C:/LAB-IQ 150/User Defined Protocol", "error in"=w2256) -> ("selected path"=w2250:path, "cancelled"=w2253:bool, "error out"=w2255:errorcluster)  [unwired: 10 in, 1 out]
        n1342 = call <vilib>:"Clear Errors.vi"("error in (no error)"=w2255) -> ("error out"=w2252:errorcluster)  [unwired: 5 in, 1 out]
        n1343 = case shown="False" w2253 {
          tunnel: w2252 -> [w2266 w2267]
          tunnel: [w2258 w2267] -> w2251
          tunnel: w2250 -> [w2265 _]
          tunnel: w2249 -> [w2260 _]
          frame False {
            n1344 = call-poly <vilib>:"Read Delimited Spreadsheet.vi"("file path (dialog if empty)"=w2265, "error in (no error)"=w2266, "delimiter (\\t)"=":" ("delimiter (\\t)")) -> ("all rows"=w2257:string[][], "error out"=w2259:errorcluster)  [unwired: 7 in, 4 out]
            n1345 = Unbundle By Name(w2260) -> ("Motion Module.StepTable For Speed"=w2263:refnum<vi>)
            n1346 = property class="Tbl (strict)"(reference=w2263, error in=w2259, "Value"=w2257) -> (reference out=w2261:refnum<vi>, error out=w2262:errorcluster)
            n1347 = Close Reference(reference=w2261, error in (no error)=w2262) -> (error out=w2258:errorcluster)
          }
          frame True {
          }
        }
      }
      frame "Save 2" {
        n1348 = Unbundle By Name(w2271) -> ("Motion Module.StepTable For Speed"=w2286:refnum<vi>)
        n1349 = property class="Tbl (strict)"(reference=w2286) -> (reference out=w2284:refnum<vi>, error out=w2285:errorcluster, "Value"=w2282:string[][])  [unwired: 1 in]
        n1350 = call "File Dialog2"("start path"=path "C:/LAB-IQ 150/User Defined Protocol", "error in"=w2276) -> ("selected path"=w2279:path, "error out"=w2278:errorcluster)  [unwired: 10 in, 2 out]
        n1351 = call <vilib>:"Clear Errors.vi"("error in (no error)"=w2278) -> ("error out"=w2277:errorcluster)  [unwired: 5 in, 1 out]
        n1352 = Close Reference(reference=w2284, error in (no error)=w2285) -> ()  [unwired: 1 out]
        n1353 = call-poly <vilib>:"Write Delimited Spreadsheet.vi"("file path (dialog if empty)"=w2279, "2D data"=w2282, "append to file? (new file:F)"=TRUE, "error in (no error)"=w2277, "delimiter (\\t)"=":" ("delimiter (\\t)")) -> ("error out"=w2275:errorcluster)  [unwired: 9 in, 1 out]
        n1354 = call <vilib>:"Clear Errors.vi"("error in (no error)"=w2275) -> ("error out"=w2270:errorcluster)  [unwired: 5 in, 1 out]
        n1355 = Unbundle By Name(w2271) -> ("Motion Module.Save 2"=w2272:refnum<vi>)
        n1356 = property class="Bool (strict)"(reference=w2272, error in=w2270, "Value"=FALSE) -> (reference out=w2274:refnum<vi>, error out=w2273:errorcluster)
        n1357 = Close Reference(reference=w2274, error in (no error)=w2273) -> (error out=w2269:errorcluster)
      }
      frame "Calculate Rotary" {
        n1358 = call "STEP LOAD MM_SEC AND RPM CONVERSION.vi"("error in (no error)"=w2290, "Data Cluster"=w2288) -> ("error out"=w2289:errorcluster)  [unwired: 9 in]
        n1359 = local write "calculate rotary"(FALSE) -> ()
      }
      frame "Clear List" {
        n1360 = Unbundle By Name(w2292) -> ("Environmental control.Sensors Picked"=w2299:refnum<vi>)
        n1361 = Unbundle By Name(w2292) -> ("Environmental control.Clear List"=w2293:refnum<vi>)
        n1362 = property class="Bool (strict)"(reference=w2293, "Value"=FALSE) -> (reference out=w2295:refnum<vi>, error out=w2294:errorcluster)  [unwired: 1 in]
        n1363 = property class="Str"(reference=w2299, "Value"="") -> (reference out=w2297:refnum<vi>, error out=w2298:errorcluster)  [unwired: 1 in]
        n1364 = Close Reference(reference=w2295, error in (no error)=w2294) -> ()  [unwired: 1 out]
        n1365 = Close Reference(reference=w2297, error in (no error)=w2298) -> ()  [unwired: 1 out]
      }
      frame "ClrLog" {
        n1366 = Unbundle By Name(w2302) -> ("Main Screen.ClrLog"=w2303:refnum<vi>)
        n1367 = Unbundle By Name(w2302) -> ("Main Screen.Trip Log"=w2309:refnum<vi>)
        n1368 = property class="Bool (strict)"(reference=w2303, "Value"=FALSE) -> (reference out=w2305:refnum<vi>, error out=w2304:errorcluster)  [unwired: 1 in]
        n1369 = property class="Str"(reference=w2309, "Value"="") -> (reference out=w2307:refnum<vi>, error out=w2308:errorcluster)  [unwired: 1 in]
        n1370 = Close Reference(reference=w2305, error in (no error)=w2304) -> ()  [unwired: 1 out]
        n1371 = Close Reference(reference=w2307, error in (no error)=w2308) -> ()  [unwired: 1 out]
      }
      frame "Add to list" {
        n1372 = Unbundle By Name(w2311) -> ("Environmental control.Sensors Picked"=w2317:refnum<vi>)
        n1373 = property class="Str"(reference=w2317, error in=w2312, "Value"="") -> (reference out=w2315:refnum<vi>, error out=w2316:errorcluster)
        n1374 = Close Reference(reference=w2315, error in (no error)=w2316) -> (error out=w2313:errorcluster)
        n1375 = call "Add  to List Loop.vi"("error in (no error)"=w2313, "Data Cluster"=w2311) -> ("error out"=w2319:errorcluster)  [unwired: 9 in]
        n1376 = Unbundle By Name(w2311) -> ("Environmental control.Add to list"=w2321:refnum<vi>)
        n1377 = property class="Bool (strict)"(reference=w2321, error in=w2319, "Value"=FALSE) -> (reference out=w2323:refnum<vi>, error out=w2322:errorcluster)
        n1378 = Close Reference(reference=w2323, error in (no error)=w2322) -> (error out=w2318:errorcluster)
      }
      frame "Disable Axis Jog Soft Limits" {
        n1379 = call "DATA ENCRYPT STRING FILE WRITE.vi"("error in (no error)"=w2327, "User Action"="User Pressed Disable Axis Jog Soft Limits in Main Screen", "main ref"=w2325) -> ("error out"=w2326:errorcluster)  [unwired: 6 in, 1 out]
      }
      frame "Home Service" {
        n1380 = Unbundle By Name(w2329) -> ("Main Home Screen.MainPage"=w2335:refnum<vi>)
        n1381 = Unbundle By Name(w2329) -> ("Main Home Screen.GUI"=w2333:refnum<vi>)
        n1382 = local write "Home Service"(FALSE ("Home Service")) -> ()
        n1383 = property class="TabCtl (strict)"(reference=w2335, "Value"=T5."HOME") -> (reference out=w2337:refnum<vi>, error out=w2336:errorcluster)  [unwired: 1 in]
        n1384 = property class="TabCtl (strict)"(reference=w2333, "Value"=T4."Setup") -> (reference out=w2331:refnum<vi>, error out=w2332:errorcluster)  [unwired: 1 in]
        n1385 = Close Reference(reference=w2337, error in (no error)=w2336) -> ()  [unwired: 1 out]
        n1386 = Close Reference(reference=w2331, error in (no error)=w2332) -> ()  [unwired: 1 out]
        n1387 = call "DATA ENCRYPT STRING FILE WRITE.vi"("error in (no error)"=w2340, "User Action"="User Pressed Home Service from Service Screen", "main ref"=w2329) -> ("error out"=w2339:errorcluster)  [unwired: 6 in, 1 out]
      }
      frame "Analysis Home" {
        n1388 = Unbundle By Name(w2342) -> ("Main Screen.Main Screen Tab"=w2345:refnum<vi>)
        n1389 = Unbundle By Name(w2342) -> ("Main Home Screen.MainPage"=w2352:refnum<vi>)
        n1390 = Unbundle By Name(w2342) -> ("Main Home Screen.GUI"=w2350:refnum<vi>)
        n1391 = local write "Analysis Home new"(FALSE ("Analysis Home new")) -> ()
        n1392 = property class="TabCtl (strict)"(reference=w2345, "Value"=T8."  Acquire  ") -> (reference out=w2343:refnum<vi>, error out=w2344:errorcluster)  [unwired: 1 in]
        n1393 = property class="TabCtl (strict)"(reference=w2352, "Value"=T5."HOME") -> (reference out=w2354:refnum<vi>, error out=w2353:errorcluster)  [unwired: 1 in]
        n1394 = property class="TabCtl (strict)"(reference=w2350, "Value"=T4."Setup") -> (reference out=w2348:refnum<vi>, error out=w2349:errorcluster)  [unwired: 1 in]
        n1395 = Close Reference(reference=w2343, error in (no error)=w2344) -> ()  [unwired: 1 out]
        n1396 = Close Reference(reference=w2354, error in (no error)=w2353) -> ()  [unwired: 1 out]
        n1397 = Close Reference(reference=w2348, error in (no error)=w2349) -> ()  [unwired: 1 out]
        n1398 = call "DATA ENCRYPT STRING FILE WRITE.vi"("error in (no error)"=w2357, "User Action"="User Pressed Home from AnalysisScreen", "main ref"=w2342) -> ("error out"=w2356:errorcluster)  [unwired: 6 in, 1 out]
      }
      frame "Post Analysis" {
        n1399 = Unbundle By Name(w2360) -> ("Main Screen.Main Screen Tab"=w2363:refnum<vi>)
        n1400 = Unbundle By Name(w2360) -> ("Main Home Screen.MainPage"=w2369:refnum<vi>)
        n1401 = Unbundle By Name(w2360) -> ("Main Home Screen.GUI"=w2367:refnum<vi>)
        n1402 = property class="TabCtl (strict)"(reference=w2363, "Value"=T8."Compare Files Rot") -> (reference out=w2361:refnum<vi>, error out=w2362:errorcluster)  [unwired: 1 in]
        n1403 = property class="TabCtl (strict)"(reference=w2369, "Value"=T5."HOME") -> (reference out=w2371:refnum<vi>, error out=w2370:errorcluster)  [unwired: 1 in]
        n1404 = property class="TabCtl (strict)"(reference=w2367, "Value"=T4."Begin") -> (reference out=w2365:refnum<vi>, error out=w2366:errorcluster)  [unwired: 1 in]
        n1405 = local write "Post Analysis"(FALSE ("Post Analysis")) -> ()
        n1406 = Close Reference(reference=w2361, error in (no error)=w2362) -> ()  [unwired: 1 out]
        n1407 = Close Reference(reference=w2371, error in (no error)=w2370) -> ()  [unwired: 1 out]
        n1408 = Close Reference(reference=w2365, error in (no error)=w2366) -> ()  [unwired: 1 out]
        n1409 = call "DATA ENCRYPT STRING FILE WRITE.vi"("error in (no error)"=w2374, "User Action"="User Pressed Post Analysis ", "main ref"=w2360) -> ("error out"=w2373:errorcluster)  [unwired: 6 in, 1 out]
      }
      frame "Edit Gain Constants" {
        n1410 = Unbundle By Name(w2376) -> ("About Screen.Heave and Surge COM Port:"=w2406:refnum<vi>)
        n1411 = Unbundle By Name(w2376) -> ("About Screen.Edit Gain Constants"=w2386:refnum<vi>)
        n1412 = Unbundle By Name(w2376) -> ("About Screen.Sway COM Port:"=w2403:refnum<vi>)
        n1413 = Unbundle By Name(w2376) -> ("About Screen.Ramp Port:"=w2380:refnum<vi>)
        n1414 = Unbundle By Name(w2376) -> ("About Screen.Temp Modbus:"=w2400:refnum<vi>)
        n1415 = Unbundle By Name(w2376) -> ("About Screen.Humidity Port:"=w2399:refnum<vi>)
        n1416 = Unbundle By Name(w2376) -> ("About Screen.Password"=w2394:refnum<vi>)
        n1417 = Unbundle By Name(w2376) -> ("About Screen.ECR Port:"=w2379:refnum<vi>)
        n1418 = property class="VISAName"(reference=w2380, "DisabledEnum"=T16."Enabled" ("Disabled")) -> (reference out=w2382:refnum<vi>, error out=w2381:errorcluster)  [unwired: 1 in]
        n1419 = property class="Bool (strict)"(reference=w2386, "Value"=FALSE) -> (reference out=w2387:refnum<vi>, error out=w2385:errorcluster)  [unwired: 1 in]
        n1420 = property class="VISAName"(reference=w2379, "DisabledEnum"=T16."Enabled" ("Disabled")) -> (reference out=w2375:refnum<vi>, error out=w2378:errorcluster)  [unwired: 1 in]
        n1421 = property class="VISAName"(reference=w2406, "DisabledEnum"=T16."Enabled" ("Disabled")) -> (reference out=w2407:refnum<vi>, error out=w2405:errorcluster)  [unwired: 1 in]
        n1422 = property class="VISAName"(reference=w2403, "DisabledEnum"=T16."Enabled" ("Disabled")) -> (reference out=w2404:refnum<vi>, error out=w2402:errorcluster)  [unwired: 1 in]
        n1423 = property class="VISAName"(reference=w2400, "DisabledEnum"=T16."Enabled" ("Disabled")) -> (reference out=w2388:refnum<vi>, error out=w2401:errorcluster)  [unwired: 1 in]
        n1424 = property class="VISAName"(reference=w2399, "DisabledEnum"=T16."Enabled" ("Disabled")) -> (reference out=w2397:refnum<vi>, error out=w2398:errorcluster)  [unwired: 1 in]
        n1425 = property class="Str"(reference=w2394, "Visible"=FALSE) -> (reference out=w2396:refnum<vi>, error out=w2395:errorcluster)  [unwired: 1 in]
        n1426 = Close Reference(reference=w2382, error in (no error)=w2381) -> ()  [unwired: 1 out]
        n1427 = Close Reference(reference=w2396, error in (no error)=w2395) -> ()  [unwired: 1 out]
        n1428 = Close Reference(reference=w2375, error in (no error)=w2378) -> ()  [unwired: 1 out]
        n1429 = Close Reference(reference=w2387, error in (no error)=w2385) -> ()  [unwired: 1 out]
        n1430 = Close Reference(reference=w2407, error in (no error)=w2405) -> ()  [unwired: 1 out]
        n1431 = Close Reference(reference=w2404, error in (no error)=w2402) -> ()  [unwired: 1 out]
        n1432 = Close Reference(reference=w2388, error in (no error)=w2401) -> ()  [unwired: 1 out]
        n1433 = Close Reference(reference=w2397, error in (no error)=w2398) -> ()  [unwired: 1 out]
        n1434 = call "DATA ENCRYPT STRING FILE WRITE.vi"("error in (no error)"=w2410, "User Action"="User Pressed Home Service from Service Screen", "main ref"=w2376) -> ("error out"=w2409:errorcluster)  [unwired: 6 in, 1 out]
      }
      frame "Advanced Setting" {
        n1435 = Unbundle By Name(w2412) -> ("About Screen.Advanced Setting"=w2414:refnum<vi>)
        n1436 = property class="Bool (strict)"(reference=w2414) -> (reference out=w2415:refnum<vi>, error out=w2413:errorcluster, "Value"=w2411:bool)  [unwired: 1 in]
        n1437 = Close Reference(reference=w2415, error in (no error)=w2413) -> ()  [unwired: 1 out]
        n1438 = case shown="True" w2411 {
          tunnel: w2412 -> [w2420 w2445]
          frame True {
            n1439 = Unbundle By Name(w2420) -> ("About Screen.Heave and Surge COM Port:"=w2442:refnum<vi>)
            n1440 = Unbundle By Name(w2420) -> ("About Screen.Edit Gain Constants"=w2422:refnum<vi>)
            n1441 = Unbundle By Name(w2420) -> ("About Screen.Sway COM Port:"=w2439:refnum<vi>)
            n1442 = Unbundle By Name(w2420) -> ("About Screen.Temp Modbus:"=w2436:refnum<vi>)
            n1443 = Unbundle By Name(w2420) -> ("About Screen.Humidity Port:"=w2435:refnum<vi>)
            n1444 = Unbundle By Name(w2420) -> ("About Screen.Password"=w2430:refnum<vi>)
            n1445 = property class="Bool (strict)"(reference=w2422, "Value"=FALSE) -> (reference out=w2423:refnum<vi>, error out=w2421:errorcluster)  [unwired: 1 in]
            n1446 = property class="VISAName"(reference=w2442, "DisabledEnum"=T16."Disabled and Grayed Out" ("Disabled")) -> (reference out=w2443:refnum<vi>, error out=w2441:errorcluster)  [unwired: 1 in]
            n1447 = property class="VISAName"(reference=w2439, "DisabledEnum"=T16."Disabled and Grayed Out" ("Disabled")) -> (reference out=w2440:refnum<vi>, error out=w2438:errorcluster)  [unwired: 1 in]
            n1448 = property class="VISAName"(reference=w2436, "DisabledEnum"=T16."Disabled and Grayed Out" ("Disabled")) -> (reference out=w2424:refnum<vi>, error out=w2437:errorcluster)  [unwired: 1 in]
            n1449 = property class="VISAName"(reference=w2435, "DisabledEnum"=T16."Disabled and Grayed Out" ("Disabled")) -> (reference out=w2433:refnum<vi>, error out=w2434:errorcluster)  [unwired: 1 in]
            n1450 = property class="Str"(reference=w2430, "Visible"=TRUE) -> (reference out=w2432:refnum<vi>, error out=w2431:errorcluster)  [unwired: 1 in]
            n1451 = Close Reference(reference=w2423, error in (no error)=w2421) -> ()  [unwired: 1 out]
            n1452 = Close Reference(reference=w2443, error in (no error)=w2441) -> ()  [unwired: 1 out]
            n1453 = Close Reference(reference=w2440, error in (no error)=w2438) -> ()  [unwired: 1 out]
            n1454 = Close Reference(reference=w2424, error in (no error)=w2437) -> ()  [unwired: 1 out]
            n1455 = Close Reference(reference=w2433, error in (no error)=w2434) -> ()  [unwired: 1 out]
            n1456 = Close Reference(reference=w2432, error in (no error)=w2431) -> ()  [unwired: 1 out]
          }
          frame False {
            n1457 = Unbundle By Name(w2445) -> ("About Screen.Heave and Surge COM Port:"=w2467:refnum<vi>)
            n1458 = Unbundle By Name(w2445) -> ("About Screen.Edit Gain Constants"=w2447:refnum<vi>)
            n1459 = Unbundle By Name(w2445) -> ("About Screen.Sway COM Port:"=w2464:refnum<vi>)
            n1460 = Unbundle By Name(w2445) -> ("About Screen.Temp Modbus:"=w2461:refnum<vi>)
            n1461 = Unbundle By Name(w2445) -> ("About Screen.Humidity Port:"=w2460:refnum<vi>)
            n1462 = Unbundle By Name(w2445) -> ("About Screen.Password"=w2455:refnum<vi>)
            n1463 = property class="Bool (strict)"(reference=w2447, "Value"=FALSE) -> (reference out=w2448:refnum<vi>, error out=w2446:errorcluster)  [unwired: 1 in]
            n1464 = property class="VISAName"(reference=w2467, "DisabledEnum"=T16."Disabled and Grayed Out" ("Disabled")) -> (reference out=w2468:refnum<vi>, error out=w2466:errorcluster)  [unwired: 1 in]
            n1465 = property class="VISAName"(reference=w2464, "DisabledEnum"=T16."Disabled and Grayed Out" ("Disabled")) -> (reference out=w2465:refnum<vi>, error out=w2463:errorcluster)  [unwired: 1 in]
            n1466 = property class="VISAName"(reference=w2461, "DisabledEnum"=T16."Disabled and Grayed Out" ("Disabled")) -> (reference out=w2449:refnum<vi>, error out=w2462:errorcluster)  [unwired: 1 in]
            n1467 = property class="VISAName"(reference=w2460, "DisabledEnum"=T16."Disabled and Grayed Out" ("Disabled")) -> (reference out=w2458:refnum<vi>, error out=w2459:errorcluster)  [unwired: 1 in]
            n1468 = property class="Str"(reference=w2455, "Visible"=FALSE) -> (reference out=w2457:refnum<vi>, error out=w2456:errorcluster)  [unwired: 1 in]
            n1469 = Close Reference(reference=w2448, error in (no error)=w2446) -> ()  [unwired: 1 out]
            n1470 = Close Reference(reference=w2468, error in (no error)=w2466) -> ()  [unwired: 1 out]
            n1471 = Close Reference(reference=w2465, error in (no error)=w2463) -> ()  [unwired: 1 out]
            n1472 = Close Reference(reference=w2449, error in (no error)=w2462) -> ()  [unwired: 1 out]
            n1473 = Close Reference(reference=w2458, error in (no error)=w2459) -> ()  [unwired: 1 out]
            n1474 = Close Reference(reference=w2457, error in (no error)=w2456) -> ()  [unwired: 1 out]
          }
        }
        n1475 = call "DATA ENCRYPT STRING FILE WRITE.vi"("error in (no error)"=w2418, "User Action"="User Pressed Advance Setting in Service Screen", "main ref"=w2412) -> ("error out"=w2417:errorcluster)  [unwired: 6 in, 1 out]
      }
      frame "Password" {
        n1476 = Unbundle By Name(w2469) -> ("About Screen.Password"=w2475:refnum<vi>)
        n1477 = property class="Str"(reference=w2475) -> (reference out=w2476:refnum<vi>, error out=w2474:errorcluster, "Value"=w2473:string)  [unwired: 1 in]
        n1478 = call <vilib>:"Trim Whitespace.vi"("string"=w2473) -> ("trimmed string"=w2472:string)  [unwired: 1 in]
        n1479 = Close Reference(reference=w2476, error in (no error)=w2474) -> ()  [unwired: 1 out]
        n1480 = Equal?(x=w2472, y="UT150$") -> (x = y?=w2470:bool)
        n1481 = case shown="True" w2470 {
          tunnel: w2469 -> [_ w2479]
          frame False {
          }
          frame True {
            n1482 = Unbundle By Name(w2479) -> ("Main Screen.Main Screen Tab"=w2481:refnum<vi>)
            n1483 = Unbundle By Name(w2479) -> ("Main Home Screen.GUI"=w2485:refnum<vi>)
            n1484 = Unbundle By Name(w2479) -> ("About Screen.Password"=w2489:refnum<vi>)
            n1485 = property class="TabCtl (strict)"(reference=w2485, "Value"=T4."Begin") -> (reference out=w2486:refnum<vi>, error out=w2484:errorcluster)  [unwired: 1 in]
            n1486 = property class="TabCtl (strict)"(reference=w2481, "Value"=T8."Service") -> (reference out=w2480:refnum<vi>, error out=w2482:errorcluster)  [unwired: 1 in]
            n1487 = property class="Str"(reference=w2489, "Value"="") -> (reference out=w2490:refnum<vi>, error out=w2488:errorcluster)  [unwired: 1 in]
            n1488 = Close Reference(reference=w2490, error in (no error)=w2488) -> ()  [unwired: 1 out]
            n1489 = Close Reference(reference=w2486, error in (no error)=w2484) -> ()  [unwired: 1 out]
            n1490 = Close Reference(reference=w2480, error in (no error)=w2482) -> ()  [unwired: 1 out]
          }
        }
      }
      frame "Service About" {
        n1491 = Unbundle By Name(w2492) -> ("Main Screen.Main Screen Tab"=w2495:refnum<vi>)
        n1492 = Unbundle By Name(w2492) -> ("Main Home Screen.GUI"=w2499:refnum<vi>)
        n1493 = local write "Service About"(FALSE ("Service About")) -> ()
        n1494 = property class="TabCtl (strict)"(reference=w2499, "Value"=T4."Begin") -> (reference out=w2500:refnum<vi>, error out=w2498:errorcluster)  [unwired: 1 in]
        n1495 = property class="TabCtl (strict)"(reference=w2495, "Value"=T8."About") -> (reference out=w2494:refnum<vi>, error out=w2496:errorcluster)  [unwired: 1 in]
        n1496 = Close Reference(reference=w2500, error in (no error)=w2498) -> ()  [unwired: 1 out]
        n1497 = Close Reference(reference=w2494, error in (no error)=w2496) -> ()  [unwired: 1 out]
      }
      frame "OPEN 1" {
        n1498 = Unbundle By Name(w2504) -> ("Analysis Screen.File 1 Discription"=w2513:refnum<vi>)
        n1499 = property class="Str"(reference=w2513, error in=w2511, "Value"="") -> (reference out=w2514:refnum<vi>, error out=w2512:errorcluster)
        n1500 = Close Reference(reference=w2514, error in (no error)=w2512) -> (error out=w2510:errorcluster)
        n1501 = call <vilib>:"Application Directory.vi"() -> ("Application Directory"=w2518:path)
        n1502 = Unbundle By Name(w2504) -> ("Analysis Screen.OPEN 1"=w2506:refnum<vi>)
        n1503 = Build Path(base path=w2518, name or relative path="data") -> (appended path=w2516:path)
        n1504 = property class="Bool (strict)"(reference=w2506, "Value"=FALSE) -> (reference out=w2507:refnum<vi>, error out=w2505:errorcluster)  [unwired: 1 in]
        n1505 = call "File Dialog3"("start path"=w2516, "error in"=w2510) -> ("selected path"=w2515:path, "cancelled"=w2502:bool, "error out"=w2519:errorcluster)  [unwired: 10 in, 1 out]
        n1506 = case shown="True" w2502 {
          tunnel: w2519 -> [w2533 _]
          tunnel: w2515 -> [w2529 _]
          tunnel: [w2521 _] -> w2508
          tunnel: w2504 -> [w2520 w2535]
          frame False {
            n1507 = Path To String(path=w2529) -> (string=w2528:string)
            n1508 = Unbundle By Name(w2520) -> ("Analysis Screen.File Name 1"=w2531:refnum<vi>)
            n1509 = call <vilib>:"Clear Errors.vi"("error in (no error)"=w2533) -> ("error out"=w2527:errorcluster)  [unwired: 5 in, 1 out]
            n1510 = property class="Str"(reference=w2531, "Value"=w2528) -> (reference out=w2532:refnum<vi>, error out=w2530:errorcluster)  [unwired: 1 in]
            n1511 = call "INI FILE READ.vi"("error in (no error)"=w2527, "File Path"=w2528) -> ("error out"=w2523:errorcluster, "concatenated string"=w2522:string)  [unwired: 8 in]
            n1512 = Unbundle By Name(w2520) -> ("Analysis Screen.File 1 Discription"=w2525:refnum<vi>)
            n1513 = Close Reference(reference=w2532, error in (no error)=w2530) -> ()  [unwired: 1 out]
            n1514 = property class="Str"(reference=w2525, error in=w2523, "Value"=w2522) -> (reference out=w2526:refnum<vi>, error out=w2524:errorcluster)
            n1515 = Close Reference(reference=w2526, error in (no error)=w2524) -> (error out=w2521:errorcluster)
          }
          frame True {
            n1516 = Unbundle By Name(w2535) -> ("Analysis Screen.File 1 Discription"=w2537:refnum<vi>)
            n1517 = Unbundle By Name(w2535) -> ("Analysis Screen.File Name 1"=w2541:refnum<vi>)
            n1518 = property class="Str"(reference=w2537, "Value"="") -> (reference out=w2538:refnum<vi>, error out=w2536:errorcluster)  [unwired: 1 in]
            n1519 = property class="Str"(reference=w2541, "Value"="") -> (reference out=w2542:refnum<vi>, error out=w2540:errorcluster)  [unwired: 1 in]
            n1520 = Close Reference(reference=w2538, error in (no error)=w2536) -> ()  [unwired: 1 out]
            n1521 = Close Reference(reference=w2542, error in (no error)=w2540) -> ()  [unwired: 1 out]
          }
        }
        n1522 = Close Reference(reference=w2507, error in (no error)=w2505) -> ()  [unwired: 1 out]
      }
      frame "OPEN 2" {
        n1523 = Unbundle By Name(w2545) -> ("Analysis Screen.File 2 Discription"=w2554:refnum<vi>)
        n1524 = property class="Str"(reference=w2554, error in=w2552, "Value"="") -> (reference out=w2555:refnum<vi>, error out=w2553:errorcluster)
        n1525 = Close Reference(reference=w2555, error in (no error)=w2553) -> (error out=w2551:errorcluster)
        n1526 = call <vilib>:"Application Directory.vi"() -> ("Application Directory"=w2559:path)
        n1527 = Unbundle By Name(w2545) -> ("Analysis Screen.OPEN 2"=w2547:refnum<vi>)
        n1528 = Build Path(base path=w2559, name or relative path="data") -> (appended path=w2557:path)
        n1529 = property class="Bool (strict)"(reference=w2547, "Value"=FALSE) -> (reference out=w2548:refnum<vi>, error out=w2546:errorcluster)  [unwired: 1 in]
        n1530 = call "File Dialog4"("start path"=w2557, "error in"=w2551) -> ("selected path"=w2556:path, "cancelled"=w2543:bool, "error out"=w2560:errorcluster)  [unwired: 10 in, 1 out]
        n1531 = case shown="True" w2543 {
          tunnel: w2560 -> [w2574 w2576]
          tunnel: w2556 -> [w2570 _]
          tunnel: [w2562 w2575] -> w2549
          tunnel: w2545 -> [w2561 w2578]
          frame False {
            n1532 = Path To String(path=w2570) -> (string=w2569:string)
            n1533 = Unbundle By Name(w2561) -> ("Analysis Screen.File Name 2"=w2572:refnum<vi>)
            n1534 = call <vilib>:"Clear Errors.vi"("error in (no error)"=w2574) -> ("error out"=w2568:errorcluster)  [unwired: 5 in, 1 out]
            n1535 = property class="Str"(reference=w2572, "Value"=w2569) -> (reference out=w2573:refnum<vi>, error out=w2571:errorcluster)  [unwired: 1 in]
            n1536 = call "INI FILE READ.vi"("error in (no error)"=w2568, "File Path"=w2569) -> ("error out"=w2564:errorcluster, "concatenated string"=w2563:string)  [unwired: 8 in]
            n1537 = Unbundle By Name(w2561) -> ("Analysis Screen.File 2 Discription"=w2566:refnum<vi>)
            n1538 = Close Reference(reference=w2573, error in (no error)=w2571) -> ()  [unwired: 1 out]
            n1539 = property class="Str"(reference=w2566, error in=w2564, "Value"=w2563) -> (reference out=w2567:refnum<vi>, error out=w2565:errorcluster)
            n1540 = Close Reference(reference=w2567, error in (no error)=w2565) -> (error out=w2562:errorcluster)
          }
          frame True {
            n1541 = Unbundle By Name(w2578) -> ("Analysis Screen.File Name 2"=w2584:refnum<vi>)
            n1542 = Unbundle By Name(w2578) -> ("Analysis Screen.File 2 Discription"=w2580:refnum<vi>)
            n1543 = property class="Str"(reference=w2584, "Value"="") -> (reference out=w2585:refnum<vi>, error out=w2583:errorcluster)  [unwired: 1 in]
            n1544 = property class="Str"(reference=w2580, "Value"="") -> (reference out=w2579:refnum<vi>, error out=w2581:errorcluster)  [unwired: 1 in]
            n1545 = call <vilib>:"Clear Errors.vi"("error in (no error)"=w2576) -> ("error out"=w2575:errorcluster)  [unwired: 5 in, 1 out]
            n1546 = Close Reference(reference=w2579, error in (no error)=w2581) -> ()  [unwired: 1 out]
            n1547 = Close Reference(reference=w2585, error in (no error)=w2583) -> ()  [unwired: 1 out]
          }
        }
        n1548 = Close Reference(reference=w2548, error in (no error)=w2546) -> ()  [unwired: 1 out]
      }
      frame "OPEN 3" {
        # "3416\n4017\n4554"
        n1549 = Unbundle By Name(w2588) -> ("Analysis Screen.File 3 Discription"=w2597:refnum<vi>)
        n1550 = property class="Str"(reference=w2597, error in=w2595, "Value"="") -> (reference out=w2598:refnum<vi>, error out=w2596:errorcluster)
        n1551 = Close Reference(reference=w2598, error in (no error)=w2596) -> (error out=w2594:errorcluster)
        n1552 = call <vilib>:"Application Directory.vi"() -> ("Application Directory"=w2602:path)
        n1553 = Unbundle By Name(w2588) -> ("Analysis Screen.OPEN 3"=w2590:refnum<vi>)
        n1554 = Build Path(base path=w2602, name or relative path="data") -> (appended path=w2600:path)
        n1555 = property class="Bool (strict)"(reference=w2590, "Value"=FALSE) -> (reference out=w2591:refnum<vi>, error out=w2589:errorcluster)  [unwired: 1 in]
        n1556 = call "File Dialog5"("start path"=w2600, "error in"=w2594) -> ("selected path"=w2599:path, "cancelled"=w2586:bool, "error out"=w2603:errorcluster)  [unwired: 10 in, 1 out]
        n1557 = case shown="True" w2586 {
          tunnel: w2603 -> [w2617 w2619]
          tunnel: w2599 -> [w2613 _]
          tunnel: [w2605 w2618] -> w2592
          tunnel: w2588 -> [w2604 w2621]
          frame False {
            n1558 = Path To String(path=w2613) -> (string=w2612:string)
            n1559 = Unbundle By Name(w2604) -> ("Analysis Screen.File Name 3"=w2615:refnum<vi>)
            n1560 = call <vilib>:"Clear Errors.vi"("error in (no error)"=w2617) -> ("error out"=w2611:errorcluster)  [unwired: 5 in, 1 out]
            n1561 = property class="Str"(reference=w2615, "Value"=w2612) -> (reference out=w2616:refnum<vi>, error out=w2614:errorcluster)  [unwired: 1 in]
            n1562 = call "INI FILE READ.vi"("error in (no error)"=w2611, "File Path"=w2612) -> ("error out"=w2607:errorcluster, "concatenated string"=w2606:string)  [unwired: 8 in]
            n1563 = Unbundle By Name(w2604) -> ("Analysis Screen.File 3 Discription"=w2609:refnum<vi>)
            n1564 = Close Reference(reference=w2616, error in (no error)=w2614) -> ()  [unwired: 1 out]
            n1565 = property class="Str"(reference=w2609, error in=w2607, "Value"=w2606) -> (reference out=w2610:refnum<vi>, error out=w2608:errorcluster)
            n1566 = Close Reference(reference=w2610, error in (no error)=w2608) -> (error out=w2605:errorcluster)
          }
          frame True {
            n1567 = Unbundle By Name(w2621) -> ("Analysis Screen.File Name 3"=w2627:refnum<vi>)
            n1568 = Unbundle By Name(w2621) -> ("Analysis Screen.File 3 Discription"=w2623:refnum<vi>)
            n1569 = property class="Str"(reference=w2627, "Value"="") -> (reference out=w2628:refnum<vi>, error out=w2626:errorcluster)  [unwired: 1 in]
            n1570 = property class="Str"(reference=w2623, "Value"="") -> (reference out=w2622:refnum<vi>, error out=w2624:errorcluster)  [unwired: 1 in]
            n1571 = Close Reference(reference=w2622, error in (no error)=w2624) -> ()  [unwired: 1 out]
            n1572 = Close Reference(reference=w2628, error in (no error)=w2626) -> ()  [unwired: 1 out]
            n1573 = call <vilib>:"Clear Errors.vi"("error in (no error)"=w2619) -> ("error out"=w2618:errorcluster)  [unwired: 5 in, 1 out]
          }
        }
        n1574 = Close Reference(reference=w2591, error in (no error)=w2589) -> ()  [unwired: 1 out]
      }
      frame "OPEN 4" {
        n1575 = Unbundle By Name(w2631) -> ("Analysis Screen.File 4 Discription"=w2640:refnum<vi>)
        n1576 = property class="Str"(reference=w2640, error in=w2638, "Value"="") -> (reference out=w2641:refnum<vi>, error out=w2639:errorcluster)
        n1577 = Close Reference(reference=w2641, error in (no error)=w2639) -> (error out=w2637:errorcluster)
        n1578 = call <vilib>:"Application Directory.vi"() -> ("Application Directory"=w2645:path)
        n1579 = Unbundle By Name(w2631) -> ("Analysis Screen.OPEN 4"=w2633:refnum<vi>)
        n1580 = Build Path(base path=w2645, name or relative path="data") -> (appended path=w2643:path)
        n1581 = property class="Bool (strict)"(reference=w2633, "Value"=FALSE) -> (reference out=w2634:refnum<vi>, error out=w2632:errorcluster)  [unwired: 1 in]
        n1582 = call "File Dialog6"("start path"=w2643, "error in"=w2637) -> ("selected path"=w2642:path, "cancelled"=w2629:bool, "error out"=w2646:errorcluster)  [unwired: 10 in, 1 out]
        n1583 = case shown="True" w2629 {
          tunnel: w2646 -> [w2660 w2662]
          tunnel: w2642 -> [w2656 _]
          tunnel: [w2648 w2661] -> w2635
          tunnel: w2631 -> [w2647 w2664]
          frame False {
            n1584 = Path To String(path=w2656) -> (string=w2655:string)
            n1585 = Unbundle By Name(w2647) -> ("Analysis Screen.File Name 4"=w2658:refnum<vi>)
            n1586 = call <vilib>:"Clear Errors.vi"("error in (no error)"=w2660) -> ("error out"=w2654:errorcluster)  [unwired: 5 in, 1 out]
            n1587 = property class="Str"(reference=w2658, "Value"=w2655) -> (reference out=w2659:refnum<vi>, error out=w2657:errorcluster)  [unwired: 1 in]
            n1588 = call "INI FILE READ.vi"("error in (no error)"=w2654, "File Path"=w2655) -> ("error out"=w2650:errorcluster, "concatenated string"=w2649:string)  [unwired: 8 in]
            n1589 = Unbundle By Name(w2647) -> ("Analysis Screen.File 4 Discription"=w2652:refnum<vi>)
            n1590 = Close Reference(reference=w2659, error in (no error)=w2657) -> ()  [unwired: 1 out]
            n1591 = property class="Str"(reference=w2652, error in=w2650, "Value"=w2649) -> (reference out=w2653:refnum<vi>, error out=w2651:errorcluster)
            n1592 = Close Reference(reference=w2653, error in (no error)=w2651) -> (error out=w2648:errorcluster)
          }
          frame True {
            n1593 = Unbundle By Name(w2664) -> ("Analysis Screen.File Name 4"=w2670:refnum<vi>)
            n1594 = Unbundle By Name(w2664) -> ("Analysis Screen.File 4 Discription"=w2666:refnum<vi>)
            n1595 = property class="Str"(reference=w2670, "Value"="") -> (reference out=w2671:refnum<vi>, error out=w2669:errorcluster)  [unwired: 1 in]
            n1596 = property class="Str"(reference=w2666, "Value"="") -> (reference out=w2665:refnum<vi>, error out=w2667:errorcluster)  [unwired: 1 in]
            n1597 = Close Reference(reference=w2665, error in (no error)=w2667) -> ()  [unwired: 1 out]
            n1598 = Close Reference(reference=w2671, error in (no error)=w2669) -> ()  [unwired: 1 out]
            n1599 = call <vilib>:"Clear Errors.vi"("error in (no error)"=w2662) -> ("error out"=w2661:errorcluster)  [unwired: 5 in, 1 out]
          }
        }
        n1600 = Close Reference(reference=w2634, error in (no error)=w2632) -> ()  [unwired: 1 out]
      }
      frame "Refresh 2" {
        n1601 = call "Data Log Refresh.vi"("error in (no error)"=w2674, "Data Cluster"=w2673) -> ("error out"=w2675:errorcluster)  [unwired: 9 in]
        n1602 = local write "Refresh 2"(FALSE ("Refresh 2")) -> ()
      }
      frame "Scratch Mode" {
        n1603 = Unbundle By Name(w2676) -> ("Motion Module.Scratch Mode"=w2679:refnum<vi>)
        n1604 = property class="Ring (strict)"(reference=w2679) -> (reference out=w2680:refnum<vi>, error out=w2678:errorcluster, "Value"=w2677:u16)  [unwired: 1 in]
        n1605 = Close Reference(reference=w2680, error in (no error)=w2678) -> ()  [unwired: 1 out]
        n1606 = case shown="2" w2677 {
          tunnel: w2676 -> [w2683 w2687]
          frame 0, Default {
            n1607 = Unbundle By Name(w2683) -> ("Motion Module.No of Scratch"=w2685:refnum<vi>)
            n1608 = property class="DigNum (strict)"(reference=w2685, "Visible"=FALSE) -> (reference out=w2686:refnum<vi>, error out=w2684:errorcluster)  [unwired: 1 in]
            n1609 = Close Reference(reference=w2686, error in (no error)=w2684) -> ()  [unwired: 1 out]
          }
          frame 2 {
            n1610 = Unbundle By Name(w2687) -> ("Motion Module.No of Scratch"=w2690:refnum<vi>)
            n1611 = property class="DigNum (strict)"(reference=w2690, "Visible"=TRUE) -> (reference out=w2691:refnum<vi>, error out=w2689:errorcluster)  [unwired: 1 in]
            n1612 = Close Reference(reference=w2691, error in (no error)=w2689) -> ()  [unwired: 1 out]
          }
        }
      }
      frame "Export" {
        n1613 = call "Export file.vi"("error in (no error)"=w2700, "Data Cluster"=w2693) -> ("error out"=w2695:errorcluster)  [unwired: 9 in]
        n1614 = call "DATA ENCRYPT STRING FILE WRITE.vi"("error in (no error)"=w2695, "User Action"="User Pressed  Export ", "main ref"=w2693) -> ("error out"=w2694:errorcluster)  [unwired: 6 in, 1 out]
        n1615 = Unbundle By Name(w2693) -> ("Analysis Screen.Export"=w2698:refnum<vi>)
        n1616 = property class="Bool (strict)"(reference=w2698, "Value"=FALSE) -> (reference out=w2699:refnum<vi>, error out=w2697:errorcluster)  [unwired: 1 in]
        n1617 = Close Reference(reference=w2699, error in (no error)=w2697) -> ()  [unwired: 1 out]
      }
      frame "Error" {
        # "#CodeRecommended - If you ever change the name of this \"Error\" message, you'll need to update the name in the Check Loop Error.vi as well."
        # "#CodeRecommended - Consider creating a system for logging errors in some way. These errors are for notification purposes only. Handling of specific errors should be performed in the message frames that generated the error."
        # "Error - Display an error dialog. This message is sent by the \"Error Handler\" VIs at the end of other loops in this application."
        n1618 = Variant To Data(error in=w2707, type=errorcluster {"status"=FALSE, "code"=0, "source"=""} ("error constant"), Variant=w2705) -> (data=w2703:errorcluster, error out=w2702:errorcluster)
        n1619 = call <vilib>:"Simple Error Handler.vi"("error in (no error)"=w2703) -> ()  [unwired: 4 in, 5 out]
        n1620 = Merge Errors(w2702) -> (w2701:errorcluster)
      }
      frame "Confirm Quit" {
        # "#CodeNeeded - If you want to provide an \"Are you sure\" dialog (or some other notification) before the application exits, place that code here. This message is typically sent from a Panel Close? event."
        # "Confirm Quit - Message that can confirm whether or not the user wants to exit the application."
        n1621 = call-poly "Enqueue Message.vi"("Priority Message? (F)"=TRUE, "error in (no error)"=w2714, "Message"="Exit", "Message Queue"=w2711) -> ("error out"=w2712:errorcluster)  [unwired: 6 in, 1 out]
        n1622 = Merge Errors(w2712) -> (w2713:errorcluster)
      }
      frame "Exit" {
        # "Stop the VI"
        # "Release the message queue reference"
        # "#CodeNeeded - Add any required cleanup code here. Note that if 'Exit' was called as a result of an error, an error dialog will be displayed. Add any custom error handling for an 'Exit' condition here as well."
        # "Exit - Exit the application."
        n1623 = call "Fire User Event - Stop.vi"("User Event - Stop"=w2717) -> ("error out"=w2716:errorcluster)  [unwired: 10 in]
        n1624 = Release Queue(queue=w2722, error in (no error)=w2715) -> (error out=w2719:errorcluster)  [unwired: 1 in, 2 out]
        n1625 = Merge Errors(w2716, w2719) -> (w2718:errorcluster)
      }
      frame Default {
        # "'Default' case only runs if there is a message that isn't defined in any of the other cases.  Output a programming error."
        n1626 = xnode "Error Ring"("parameter 0"=w2723) -> ("error out"=w2724:errorcluster)
      }
    }
    n1627 = call "LAB-IQ Error Handler - Message Handling Loop.vi"("error in (no error)"=w1407, "Message Queue"=w1409) -> ("dup error in"=w1408:errorcluster)  [unwired: 8 in, 1 out]
  }
  n1628 = timed-loop {
    shift-right: [w2743] -> _
    shift-left: w28 -> [w2744]
    tunnel: [w2737] -> w38
    tunnel: w37 -> [w2735]
    tunnel: w18 -> [w2734]
    tunnel: w27 -> [w2733]
    timing: w5 -> [_]
    timing-out: [_] -> w4
    stop <- w2742 stop-if-true
    # "Load  Handling Loop"
    n1629 = node-c288() -> ()  [unwired: 1 in, 1 out]
    n1630 = call "Dequeue Message.vi"("error in (no error)"=w2734, "Message Queue"=w2735) -> ("error out"=w2741:errorcluster, "Message Data"=w2739:variant, "Message"=w2740:string, "dup Message Queue"=w2738:refnum<queue>)  [unwired: 6 in]
    n1631 = case "Message Cases" shown="\"Load Main\"" w2740 {
      selector: w2740 -> [_ _ _ _ _ w2800]
      tunnel: w2738 -> [w2747 w2760 _ w2789 w2799 _]
      tunnel: w2741 -> [w2750 w2758 w2776 w2791 w2793 _]
      tunnel: [w2751 w2761 w2770 w2777 w2795 w2801] -> w2736
      tunnel: w2744 -> [w2749 w2753 w2775 w2786 w2798 w2802]
      tunnel: [w2749 w2753 w2775 w2786 w2798 w2802] -> w2743
      tunnel: [_ _ _ _ TRUE _] -> w2742
      tunnel: w2739 -> [_ _ w2774 _ _ _]
      tunnel: w2733 -> [_ _ _ _ w2792 _]
      frame "init" {
        # "Bundle control references and a sample string value."
        # "Initialize - All initialization work should take place in this message, since other loops can potentially enqueue messages that execute immediately after this one."
        n1632 = call-poly "Enqueue Message.vi"("error in (no error)"=w2750, "Message"="Load Main", "Message Queue"=w2747) -> ("error out"=w2751:errorcluster)  [unwired: 7 in, 1 out]
      }
      frame "Load Main" {
        n1633 = call "LOAD CELL READ.vi"("error in (no error)"=w2758, "main ref"=w2753) -> ("error out"=w2754:errorcluster)  [unwired: 9 in]
        n1634 = call <vilib>:"Clear Errors.vi"("error in (no error)"=w2754) -> ("error out"=w2752:errorcluster)  [unwired: 5 in, 1 out]
        n1635 = Unbundle By Name(w2753) -> ("Main Home Screen.EXIT"=w2759:refnum<vi>)
        n1636 = property class="Bool (strict)"(reference=w2759) -> (reference out=w2756:refnum<vi>, error out=w2757:errorcluster, "Value"=w2755:bool)  [unwired: 1 in]
        n1637 = Close Reference(reference=w2756, error in (no error)=w2757) -> ()  [unwired: 1 out]
        n1638 = case shown="False" w2755 {
          tunnel: [w2764 w2768] -> w2761
          tunnel: w2760 -> [w2763 w2767]
          tunnel: w2752 -> [w2762 w2766]
          frame True {
            n1639 = call-poly "Enqueue Message.vi"("error in (no error)"=w2762, "Message"="Confirm Quit", "Message Queue"=w2763) -> ("error out"=w2764:errorcluster)  [unwired: 7 in, 1 out]
          }
          frame False {
            n1640 = call-poly "Enqueue Message.vi"("error in (no error)"=w2766, "Message"="Load Main", "Message Queue"=w2767) -> ("error out"=w2768:errorcluster)  [unwired: 7 in, 1 out]
          }
        }
      }
      frame "Error" {
        # "#CodeRecommended - If you ever change the name of this \"Error\" message, you'll need to update the name in the Check Loop Error.vi as well."
        # "#CodeRecommended - Consider creating a system for logging errors in some way. These errors are for notification purposes only. Handling of specific errors should be performed in the message frames that generated the error."
        # "Error - Display an error dialog. This message is sent by the \"Error Handler\" VIs at the end of other loops in this application."
        n1641 = Variant To Data(error in=w2776, type=errorcluster {"status"=FALSE, "code"=0, "source"=""} ("error constant"), Variant=w2774) -> (data=w2772:errorcluster, error out=w2771:errorcluster)
        n1642 = call <vilib>:"Simple Error Handler.vi"("error in (no error)"=w2772) -> ()  [unwired: 4 in, 5 out]
        n1643 = Merge Errors(w2771) -> (w2770:errorcluster)
      }
      frame "Confirm Quit" {
        # "#CodeNeeded - If you want to provide an \"Are you sure\" dialog (or some other notification) before the application exits, place that code here. This message is typically sent from a Panel Close? event."
        # "Confirm Quit - Message that can confirm whether or not the user wants to exit the application."
        n1644 = call-poly "Enqueue Message.vi"("Priority Message? (F)"=TRUE, "error in (no error)"=w2791, "Message"="Exit", "Message Queue"=w2789) -> ("error out"=w2790:errorcluster)  [unwired: 6 in, 1 out]
        n1645 = Merge Errors(w2790) -> (w2782:errorcluster)
        n1646 = call <vilib>:"Clear Errors.vi"("error in (no error)"=w2782) -> ("error out"=w2778:errorcluster)  [unwired: 5 in, 1 out]
        n1647 = call "LOAD CELL FGV MAIN.vi"("Enum"=T17."UNINITIAL", "error in (no error)"=w2778, "main ref"=w2786) -> ("error IO"=w2785:errorcluster)  [unwired: 8 in]
        n1648 = call "Stall Data Flow.vim"("value in"=w2785, "milliseconds to wait"=u32 1000) -> ("value out"=w2780:errorcluster)  [unwired: 1 out]
        n1649 = call "LOAD CELL FGV MAIN.vi"("Enum"=T17."DELETEHANDLE", "error in (no error)"=w2780, "main ref"=w2786) -> ("error IO"=w2781:errorcluster)  [unwired: 8 in]
        n1650 = call <vilib>:"Clear Errors.vi"("error in (no error)"=w2781) -> ("error out"=w2777:errorcluster)  [unwired: 5 in, 1 out]
      }
      frame "Exit" {
        # "Stop the VI"
        # "Release the message queue reference"
        # "#CodeNeeded - Add any required cleanup code here. Note that if 'Exit' was called as a result of an error, an error dialog will be displayed. Add any custom error handling for an 'Exit' condition here as well."
        # "Exit - Exit the application."
        n1651 = call "Fire User Event - Stop.vi"("User Event - Stop"=w2792) -> ("error out"=w2794:errorcluster)  [unwired: 10 in]
        n1652 = Release Queue(queue=w2799, error in (no error)=w2793) -> (error out=w2796:errorcluster)  [unwired: 1 in, 2 out]
        n1653 = Merge Errors(w2794, w2796) -> (w2795:errorcluster)
      }
      frame Default {
        # "'Default' case only runs if there is a message that isn't defined in any of the other cases.  Output a programming error."
        n1654 = xnode "Error Ring"("parameter 0"=w2800) -> ("error out"=w2801:errorcluster)
      }
    }
    n1655 = node-c288() -> ()  [unwired: 1 in, 1 out]
    n1656 = call "LAB-IQ Error Handler - Message Handling Loop.vi"("error in (no error)"=w2736, "Message Queue"=w2738) -> ("dup error in"=w2737:errorcluster)  [unwired: 8 in, 1 out]
  }
  n1657 = timed-loop {
    shift-right: [w2820] -> _
    shift-left: w28 -> [w2821]
    tunnel: [w2814] -> w35
    tunnel: w36 -> [w2812]
    tunnel: w18 -> [w2811]
    tunnel: w27 -> [w2810]
    timing: w7 -> [_]
    timing-out: [_] -> w6
    stop <- w2819 stop-if-true
    # "Sway Motor  Handling Loop"
    n1658 = node-c288() -> ()  [unwired: 1 in, 1 out]
    n1659 = call "Dequeue Message.vi"("error in (no error)"=w2811, "Message Queue"=w2812) -> ("error out"=w2818:errorcluster, "Message Data"=w2816:variant, "Message"=w2817:string, "dup Message Queue"=w2815:refnum<queue>)  [unwired: 6 in]
    n1660 = case "Message Cases" shown="\"Sway Main\"" w2817 {
      selector: w2817 -> [_ _ _ _ _ w2907]
      tunnel: w2815 -> [w2835 w2864 _ w2894 w2906 _]
      tunnel: w2818 -> [w2837 w2845 w2891 w2898 w2900 _]
      tunnel: [w2838 w2865 w2885 w2896 w2902 w2908] -> w2813
      tunnel: w2821 -> [w2826 w2839 w2890 w2897 w2905 w2909]
      tunnel: [w2826 w2839 w2890 w2897 w2905 w2909] -> w2820
      tunnel: [_ _ _ _ TRUE _] -> w2819
      tunnel: w2816 -> [_ _ w2889 _ _ _]
      tunnel: w2810 -> [_ _ _ _ w2899 _]
      frame "init" {
        # "Initialize - All initialization work should take place in this message, since other loops can potentially enqueue messages that execute immediately after this one."
        n1661 = call "SWAY WRITE FGV.vi"("Enum - Menu"=Sway_Write_enum."INIT", "error in (no error)"=w2837, "main ref"=w2826) -> ("error out"=w2834:errorcluster)  [unwired: 8 in]
        n1662 = call <vilib>:"Clear Errors.vi"("error in (no error)"=w2834) -> ("error out"=w2825:errorcluster)  [unwired: 5 in, 1 out]
        n1663 = call "Stall Data Flow.vim"("value in"=w2825, "milliseconds to wait"=u32 1000) -> ("value out"=w2832:errorcluster)  [unwired: 1 out]
        n1664 = call "Sway Init.vi"("error in (no error)"=w2832, "main ref"=w2826) -> ("error out"=w2827:errorcluster)  [unwired: 9 in]
        n1665 = call <vilib>:"Clear Errors.vi"("error in (no error)"=w2827) -> ("error out"=w2824:errorcluster)  [unwired: 5 in, 1 out]
        n1666 = call "SWAY READ FGV.vi"("Enum - Menu"=Sway_Right_enum."INIT", "error in (no error)"=w2824, "main ref"=w2826) -> ("error out"=w2830:errorcluster)  [unwired: 7 in, 1 out]
        n1667 = call <vilib>:"Clear Errors.vi"("error in (no error)"=w2830) -> ("error out"=w2829:errorcluster)  [unwired: 5 in, 1 out]
        n1668 = call-poly "Enqueue Message.vi"("error in (no error)"=w2829, "Message"="Sway Main", "Message Queue"=w2835) -> ("error out"=w2838:errorcluster)  [unwired: 7 in, 1 out]
      }
      frame "Sway Main" {
        n1669 = Unbundle By Name(w2839) -> ("Heave AND Surge.SURGE POSE"=w2850:refnum<vi>)
        n1670 = Unbundle By Name(w2839) -> ("SWAY.Read SWAY Temp"=w2859:refnum<vi>)
        n1671 = local read "HEAVE ENABLE"() -> (w2854:bool)
        n1672 = property class="DigNum (strict)"(reference=w2850) -> (reference out=w2852:refnum<vi>, error out=w2851:errorcluster, "Value"=w2849:sgl)  [unwired: 1 in]
        n1673 = property class="Bool (strict)"(reference=w2859) -> (reference out=w2857:refnum<vi>, error out=w2858:errorcluster, "Value"=w2856:bool)  [unwired: 1 in]
        n1674 = Equal?(x=w2854, y=TRUE) -> (x = y?=w2848:bool)
        n1675 = Close Reference(reference=w2852, error in (no error)=w2851) -> ()  [unwired: 1 out]
        n1676 = Equal?(x=w2849, y=sgl 25000.0) -> (x = y?=w2847:bool)
        n1677 = Close Reference(reference=w2857, error in (no error)=w2858) -> ()  [unwired: 1 out]
        n1678 = And(x=w2848, y=w2847) -> (x .and. y?=w2846:bool)
        n1679 = case shown="True" w2846 {
          tunnel: w2839 -> [_ w2871]
          tunnel: w2845 -> [w2866 w2870]
          tunnel: [w2866 w2867] -> w2843
          frame False {
          }
          frame True {
            n1680 = call "SWAY HOME.vi"("error in (no error)"=w2870, "Data Cluster"=w2871) -> ("error out"=w2868:errorcluster)  [unwired: 9 in]
            n1681 = local write "HEAVE ENABLE"(FALSE ("HEAVE ENABLE")) -> ()
            n1682 = call <vilib>:"Clear Errors.vi"("error in (no error)"=w2868) -> ("error out"=w2867:errorcluster)  [unwired: 5 in, 1 out]
          }
        }
        n1683 = case shown="True" w2856 {
          tunnel: w2845 -> [w2872 w2876]
          tunnel: [w2872 w2875] -> w2841
          tunnel: w2839 -> [_ w2874]
          frame False {
          }
          frame True {
            n1684 = call "SWAY READ FGV.vi"("Enum - Menu"=Sway_Right_enum."READ", "error in (no error)"=w2876, "main ref"=w2874) -> ("error out"=w2875:errorcluster)  [unwired: 7 in, 1 out]
          }
        }
        n1685 = call "Sway Reinitize.vi"("error in (no error)"=w2841, "Data Cluster"=w2839) -> ("error out"=w2840:errorcluster)  [unwired: 9 in]
        n1686 = Unbundle By Name(w2839) -> ("Main Home Screen.EXIT"=w2863:refnum<vi>)
        n1687 = property class="Bool (strict)"(reference=w2863) -> (reference out=w2861:refnum<vi>, error out=w2862:errorcluster, "Value"=w2860:bool)  [unwired: 1 in]
        n1688 = call <vilib>:"Clear Errors.vi"("error in (no error)"=w2840) -> ("error out"=w2855:errorcluster)  [unwired: 5 in, 1 out]
        n1689 = Merge Errors(w2855, w2843) -> (w2844:errorcluster)
        n1690 = Close Reference(reference=w2861, error in (no error)=w2862) -> ()  [unwired: 1 out]
        n1691 = case shown="False" w2860 {
          tunnel: [w2879 w2883] -> w2865
          tunnel: w2864 -> [w2878 w2882]
          tunnel: w2844 -> [w2877 w2881]
          frame True {
            n1692 = call-poly "Enqueue Message.vi"("error in (no error)"=w2877, "Message"="Confirm Quit", "Message Queue"=w2878) -> ("error out"=w2879:errorcluster)  [unwired: 7 in, 1 out]
          }
          frame False {
            n1693 = call-poly "Enqueue Message.vi"("error in (no error)"=w2881, "Message"="Sway Main", "Message Queue"=w2882) -> ("error out"=w2883:errorcluster)  [unwired: 7 in, 1 out]
          }
        }
      }
      frame "Error" {
        # "#CodeRecommended - If you ever change the name of this \"Error\" message, you'll need to update the name in the Check Loop Error.vi as well."
        # "#CodeRecommended - Consider creating a system for logging errors in some way. These errors are for notification purposes only. Handling of specific errors should be performed in the message frames that generated the error."
        # "Error - Display an error dialog. This message is sent by the \"Error Handler\" VIs at the end of other loops in this application."
        n1694 = Variant To Data(error in=w2891, type=errorcluster {"status"=FALSE, "code"=0, "source"=""} ("error constant"), Variant=w2889) -> (data=w2887:errorcluster, error out=w2886:errorcluster)
        n1695 = call <vilib>:"Simple Error Handler.vi"("error in (no error)"=w2887) -> ()  [unwired: 4 in, 5 out]
        n1696 = Merge Errors(w2886) -> (w2885:errorcluster)
      }
      frame "Confirm Quit" {
        # "#CodeNeeded - If you want to provide an \"Are you sure\" dialog (or some other notification) before the application exits, place that code here. This message is typically sent from a Panel Close? event."
        # "Confirm Quit - Message that can confirm whether or not the user wants to exit the application."
        n1697 = call-poly "Enqueue Message.vi"("Priority Message? (F)"=TRUE, "error in (no error)"=w2898, "Message"="Exit", "Message Queue"=w2894) -> ("error out"=w2895:errorcluster)  [unwired: 6 in, 1 out]
        n1698 = Merge Errors(w2895) -> (w2896:errorcluster)
      }
      frame "Exit" {
        # "Stop the VI"
        # "Release the message queue reference"
        # "#CodeNeeded - Add any required cleanup code here. Note that if 'Exit' was called as a result of an error, an error dialog will be displayed. Add any custom error handling for an 'Exit' condition here as well."
        # "Exit - Exit the application."
        n1699 = call "Fire User Event - Stop.vi"("User Event - Stop"=w2899) -> ("error out"=w2901:errorcluster)  [unwired: 10 in]
        n1700 = Release Queue(queue=w2906, error in (no error)=w2900) -> (error out=w2903:errorcluster)  [unwired: 1 in, 2 out]
        n1701 = Merge Errors(w2901, w2903) -> (w2902:errorcluster)
      }
      frame Default {
        # "'Default' case only runs if there is a message that isn't defined in any of the other cases.  Output a programming error."
        n1702 = xnode "Error Ring"("parameter 0"=w2907) -> ("error out"=w2908:errorcluster)
      }
    }
    n1703 = node-c288() -> ()  [unwired: 1 in, 1 out]
    n1704 = call "LAB-IQ Error Handler - Message Handling Loop.vi"("error in (no error)"=w2813, "Message Queue"=w2815) -> ("dup error in"=w2814:errorcluster)  [unwired: 8 in, 1 out]
  }
  n1705 = timed-loop {
    shift-right: [w2927] -> _
    shift-left: w28 -> [w2928]
    tunnel: [w2921] -> w33
    tunnel: w19 -> [w2919]
    tunnel: w18 -> [w2918]
    tunnel: w27 -> [w2917]
    timing: w9 -> [_]
    timing-out: [_] -> w8
    stop <- w2926 stop-if-true
    # "Heave Motor  Handling Loop"
    n1706 = node-c288() -> ()  [unwired: 1 in, 1 out]
    n1707 = call "Dequeue Message.vi"("error in (no error)"=w2918, "Message Queue"=w2919) -> ("error out"=w2925:errorcluster, "Message Data"=w2923:variant, "Message"=w2924:string, "dup Message Queue"=w2922:refnum<queue>)  [unwired: 6 in]
    n1708 = case "Message Cases" shown="\"Heave Main\"" w2924 {
      selector: w2924 -> [_ _ _ _ _ w3001]
      tunnel: w2922 -> [w2943 w2958 _ w2989 w3000 _]
      tunnel: w2925 -> [w2940 w2956 w2979 w2992 w2994 _]
      tunnel: [w2941 w2959 w2973 w2980 w2996 w3002] -> w2920
      tunnel: w2928 -> [w2939 w2946 w2978 w2983 w2999 w3003]
      tunnel: [w2939 w2946 w2978 w2983 w2999 w3003] -> w2927
      tunnel: [_ _ _ _ TRUE _] -> w2926
      tunnel: w2923 -> [_ _ w2977 _ _ _]
      tunnel: w2917 -> [_ _ _ _ w2993 _]
      frame "init" {
        # "Initialize - All initialization work should take place in this message, since other loops can potentially enqueue messages that execute immediately after this one."
        n1709 = call "HEAVE WRITE FGV.vi"("Enum - Menu"=Heave_Write_enum."INIT", "error in (no error)"=w2940, "main ref"=w2939) -> ("error out"=w2938:errorcluster)  [unwired: 8 in]
        n1710 = call <vilib>:"Clear Errors.vi"("error in (no error)"=w2938) -> ("error out"=w2932:errorcluster)  [unwired: 5 in, 1 out]
        n1711 = call "Stall Data Flow.vim"("value in"=w2932, "milliseconds to wait"=u32 1000) -> ("value out"=w2936:errorcluster)  [unwired: 1 out]
        n1712 = call "Heave Init.vi"("error in (no error)"=w2936, "main ref"=w2939) -> ("error out"=w2933:errorcluster)  [unwired: 9 in]
        n1713 = call "HEAVE READ FGV.vi"("Enum - Menu"=Heave_Right_enum."INIT", "error in (no error)"=w2933, "main ref"=w2939) -> ("error out"=w2934:errorcluster)  [unwired: 7 in, 1 out]
        n1714 = call <vilib>:"Clear Errors.vi"("error in (no error)"=w2934) -> ("error out"=w2942:errorcluster)  [unwired: 5 in, 1 out]
        n1715 = call-poly "Enqueue Message.vi"("error in (no error)"=w2942, "Message"="Heave Main", "Message Queue"=w2943) -> ("error out"=w2941:errorcluster)  [unwired: 7 in, 1 out]
      }
      frame "Heave Main" {
        n1716 = Unbundle By Name(w2946) -> ("Heave AND Surge.Read Heave Temp"=w2952:refnum<vi>)
        n1717 = property class="Bool (strict)"(reference=w2952) -> (reference out=w2950:refnum<vi>, error out=w2951:errorcluster, "Value"=w2949:bool)  [unwired: 1 in]
        n1718 = Close Reference(reference=w2950, error in (no error)=w2951) -> ()  [unwired: 1 out]
        n1719 = case shown="True" w2949 {
          tunnel: w2956 -> [w2960 w2964]
          tunnel: [w2960 w2963] -> w2947
          tunnel: w2946 -> [_ w2962]
          frame False {
          }
          frame True {
            n1720 = call "HEAVE READ FGV.vi"("Enum - Menu"=Heave_Right_enum."READ", "error in (no error)"=w2964, "main ref"=w2962) -> ("error out"=w2963:errorcluster)  [unwired: 7 in, 1 out]
          }
        }
        n1721 = call "Heave Reinitial.vi"("error in (no error)"=w2947, "Data Cluster"=w2946) -> ("error out"=w2945:errorcluster)  [unwired: 9 in]
        n1722 = Unbundle By Name(w2946) -> ("Main Home Screen.EXIT"=w2957:refnum<vi>)
        n1723 = property class="Bool (strict)"(reference=w2957) -> (reference out=w2954:refnum<vi>, error out=w2955:errorcluster, "Value"=w2953:bool)  [unwired: 1 in]
        n1724 = call <vilib>:"Clear Errors.vi"("error in (no error)"=w2945) -> ("error out"=w2948:errorcluster)  [unwired: 5 in, 1 out]
        n1725 = Close Reference(reference=w2954, error in (no error)=w2955) -> ()  [unwired: 1 out]
        n1726 = case shown="False" w2953 {
          tunnel: [w2967 w2971] -> w2959
          tunnel: w2958 -> [w2966 w2970]
          tunnel: w2948 -> [w2965 w2969]
          frame True {
            n1727 = call-poly "Enqueue Message.vi"("error in (no error)"=w2965, "Message"="Confirm Quit", "Message Queue"=w2966) -> ("error out"=w2967:errorcluster)  [unwired: 7 in, 1 out]
          }
          frame False {
            n1728 = call-poly "Enqueue Message.vi"("error in (no error)"=w2969, "Message"="Heave Main", "Message Queue"=w2970) -> ("error out"=w2971:errorcluster)  [unwired: 7 in, 1 out]
          }
        }
      }
      frame "Error" {
        # "#CodeRecommended - If you ever change the name of this \"Error\" message, you'll need to update the name in the Check Loop Error.vi as well."
        # "#CodeRecommended - Consider creating a system for logging errors in some way. These errors are for notification purposes only. Handling of specific errors should be performed in the message frames that generated the error."
        # "Error - Display an error dialog. This message is sent by the \"Error Handler\" VIs at the end of other loops in this application."
        n1729 = Variant To Data(error in=w2979, type=errorcluster {"status"=FALSE, "code"=0, "source"=""} ("error constant"), Variant=w2977) -> (data=w2975:errorcluster, error out=w2974:errorcluster)
        n1730 = call <vilib>:"Simple Error Handler.vi"("error in (no error)"=w2975) -> ()  [unwired: 4 in, 5 out]
        n1731 = Merge Errors(w2974) -> (w2973:errorcluster)
      }
      frame "Confirm Quit" {
        # "#CodeNeeded - If you want to provide an \"Are you sure\" dialog (or some other notification) before the application exits, place that code here. This message is typically sent from a Panel Close? event."
        # "Confirm Quit - Message that can confirm whether or not the user wants to exit the application."
        n1732 = call-poly "Enqueue Message.vi"("Priority Message? (F)"=TRUE, "error in (no error)"=w2992, "Message"="Exit", "Message Queue"=w2989) -> ("error out"=w2990:errorcluster)  [unwired: 6 in, 1 out]
        n1733 = Merge Errors(w2990) -> (w2991:errorcluster)
        n1734 = call "HEAVE READ FGV.vi"("Enum - Menu"=Heave_Right_enum."CLOSE", "error in (no error)"=w2991, "main ref"=w2983) -> ("error out"=w2986:errorcluster)  [unwired: 7 in, 1 out]
        n1735 = call <vilib>:"Clear Errors.vi"("error in (no error)"=w2986) -> ("error out"=w2981:errorcluster)  [unwired: 5 in, 1 out]
        n1736 = call "HEAVE WRITE FGV.vi"("Enum - Menu"=Heave_Write_enum."CLOSE", "error in (no error)"=w2981, "main ref"=w2983) -> ("error out"=w2984:errorcluster)  [unwired: 8 in]
        n1737 = call <vilib>:"Clear Errors.vi"("error in (no error)"=w2984) -> ("error out"=w2980:errorcluster)  [unwired: 5 in, 1 out]
      }
      frame "Exit" {
        # "Stop the VI"
        # "Release the message queue reference"
        # "#CodeNeeded - Add any required cleanup code here. Note that if 'Exit' was called as a result of an error, an error dialog will be displayed. Add any custom error handling for an 'Exit' condition here as well."
        # "Exit - Exit the application."
        n1738 = call "Fire User Event - Stop.vi"("User Event - Stop"=w2993) -> ("error out"=w2995:errorcluster)  [unwired: 10 in]
        n1739 = Release Queue(queue=w3000, error in (no error)=w2994) -> (error out=w2997:errorcluster)  [unwired: 1 in, 2 out]
        n1740 = Merge Errors(w2995, w2997) -> (w2996:errorcluster)
      }
      frame Default {
        # "'Default' case only runs if there is a message that isn't defined in any of the other cases.  Output a programming error."
        n1741 = xnode "Error Ring"("parameter 0"=w3001) -> ("error out"=w3002:errorcluster)
      }
    }
    n1742 = node-c288() -> ()  [unwired: 1 in, 1 out]
    n1743 = call "LAB-IQ Error Handler - Message Handling Loop.vi"("error in (no error)"=w2920, "Message Queue"=w2922) -> ("dup error in"=w2921:errorcluster)  [unwired: 8 in, 1 out]
  }
  n1744 = while {
    shift-right: [w3021] -> _
    shift-left: w28 -> [w3022]
    tunnel: [w3015] -> _
    tunnel: w29 -> [w3013]
    tunnel: w18 -> [w3012]
    tunnel: w27 -> [w3011]
    stop <- w3020 stop-if-true
    # "Program  Handling Loop"
    n1745 = call "Dequeue Message.vi"("error in (no error)"=w3012, "Message Queue"=w3013) -> ("error out"=w3019:errorcluster, "Message Data"=w3017:variant, "Message"=w3018:string, "dup Message Queue"=w3016:refnum<queue>)  [unwired: 6 in]
    n1746 = case "Message Cases" shown="\"Program Main\"" w3018 {
      selector: w3018 -> [_ _ _ _ _ w3067]
      tunnel: w3016 -> [w3023 w3035 _ w3054 w3066 _]
      tunnel: w3019 -> [w3026 w3029 w3051 w3058 w3060 _]
      tunnel: [w3027 w3036 w3045 w3056 w3062 w3068] -> w3014
      tunnel: w3022 -> [w3025 w3028 w3050 w3057 w3065 w3069]
      tunnel: [w3025 w3028 w3050 w3057 w3065 w3069] -> w3021
      tunnel: [_ _ _ _ TRUE _] -> w3020
      tunnel: w3017 -> [_ _ w3049 _ _ _]
      tunnel: w3011 -> [_ _ _ _ w3059 _]
      frame "init" {
        # "Initialize - All initialization work should take place in this message, since other loops can potentially enqueue messages that execute immediately after this one."
        n1747 = call-poly "Enqueue Message.vi"("error in (no error)"=w3026, "Message"="Program Main", "Message Queue"=w3023) -> ("error out"=w3027:errorcluster)  [unwired: 7 in, 1 out]
      }
      frame "Program Main" {
        n1748 = call "Main Program Loop Vi.vi"("error in (no error)"=w3029, "Data Cluster"=w3028) -> ("error out"=w3030:errorcluster)  [unwired: 9 in]
        n1749 = Unbundle By Name(w3028) -> ("Main Home Screen.EXIT"=w3034:refnum<vi>)
        n1750 = property class="Bool (strict)"(reference=w3034) -> (reference out=w3032:refnum<vi>, error out=w3033:errorcluster, "Value"=w3031:bool)  [unwired: 1 in]
        n1751 = case shown="False" w3031 {
          tunnel: [w3039 w3043] -> w3036
          tunnel: w3035 -> [w3038 w3042]
          tunnel: w3030 -> [w3037 w3041]
          frame True {
            n1752 = call-poly "Enqueue Message.vi"("error in (no error)"=w3037, "Message"="Confirm Quit", "Message Queue"=w3038) -> ("error out"=w3039:errorcluster)  [unwired: 7 in, 1 out]
          }
          frame False {
            n1753 = call-poly "Enqueue Message.vi"("error in (no error)"=w3041, "Message"="Program Main", "Message Queue"=w3042) -> ("error out"=w3043:errorcluster)  [unwired: 7 in, 1 out]
          }
        }
        n1754 = Close Reference(reference=w3032, error in (no error)=w3033) -> ()  [unwired: 1 out]
      }
      frame "Error" {
        # "#CodeRecommended - If you ever change the name of this \"Error\" message, you'll need to update the name in the Check Loop Error.vi as well."
        # "#CodeRecommended - Consider creating a system for logging errors in some way. These errors are for notification purposes only. Handling of specific errors should be performed in the message frames that generated the error."
        # "Error - Display an error dialog. This message is sent by the \"Error Handler\" VIs at the end of other loops in this application."
        n1755 = Variant To Data(error in=w3051, type=errorcluster {"status"=FALSE, "code"=0, "source"=""} ("error constant"), Variant=w3049) -> (data=w3047:errorcluster, error out=w3046:errorcluster)
        n1756 = call <vilib>:"Simple Error Handler.vi"("error in (no error)"=w3047) -> ()  [unwired: 4 in, 5 out]
        n1757 = Merge Errors(w3046) -> (w3045:errorcluster)
      }
      frame "Confirm Quit" {
        # "#CodeNeeded - If you want to provide an \"Are you sure\" dialog (or some other notification) before the application exits, place that code here. This message is typically sent from a Panel Close? event."
        # "Confirm Quit - Message that can confirm whether or not the user wants to exit the application."
        n1758 = call-poly "Enqueue Message.vi"("Priority Message? (F)"=TRUE, "error in (no error)"=w3058, "Message"="Exit", "Message Queue"=w3054) -> ("error out"=w3055:errorcluster)  [unwired: 6 in, 1 out]
        n1759 = Merge Errors(w3055) -> (w3056:errorcluster)
      }
      frame "Exit" {
        # "Stop the VI"
        # "Release the message queue reference"
        # "#CodeNeeded - Add any required cleanup code here. Note that if 'Exit' was called as a result of an error, an error dialog will be displayed. Add any custom error handling for an 'Exit' condition here as well."
        # "Exit - Exit the application."
        n1760 = call "Fire User Event - Stop.vi"("User Event - Stop"=w3059) -> ("error out"=w3061:errorcluster)  [unwired: 10 in]
        n1761 = Release Queue(queue=w3066, error in (no error)=w3060) -> (error out=w3063:errorcluster)  [unwired: 1 in, 2 out]
        n1762 = Merge Errors(w3061, w3063) -> (w3062:errorcluster)
      }
      frame Default {
        # "'Default' case only runs if there is a message that isn't defined in any of the other cases.  Output a programming error."
        n1763 = xnode "Error Ring"("parameter 0"=w3067) -> ("error out"=w3068:errorcluster)
      }
    }
    n1764 = call "LAB-IQ Error Handler - Message Handling Loop.vi"("error in (no error)"=w3014, "Message Queue"=w3016) -> ("dup error in"=w3015:errorcluster)  [unwired: 8 in, 1 out]
  }
  n1765 = timed-loop {
    shift-right: [w3087] -> _
    shift-left: w28 -> [w3088]
    tunnel: [w3081] -> _
    tunnel: w26 -> [w3079]
    tunnel: w18 -> [w3078]
    tunnel: w27 -> [w3077]
    timing: w11 -> [_]
    timing-out: [_] -> w10
    stop <- w3086 stop-if-true
    # "Monitor  Handling Loop"
    n1766 = node-c288() -> ()  [unwired: 1 in, 1 out]
    n1767 = call "Dequeue Message.vi"("error in (no error)"=w3078, "Message Queue"=w3079) -> ("error out"=w3085:errorcluster, "Message Data"=w3083:variant, "Message"=w3084:string, "dup Message Queue"=w3082:refnum<queue>)  [unwired: 6 in]
    n1768 = case "Message Cases" shown="\"Monitor Main\"" w3084 {
      selector: w3084 -> [_ _ _ _ _ w3138]
      tunnel: w3082 -> [w3091 w3106 _ w3125 w3137 _]
      tunnel: w3085 -> [w3094 w3099 w3122 w3129 w3131 _]
      tunnel: [w3095 w3107 w3116 w3127 w3133 w3139] -> w3080
      tunnel: w3088 -> [w3093 w3100 w3121 w3128 w3136 w3140]
      tunnel: [w3093 w3100 w3121 w3128 w3136 w3140] -> w3087
      tunnel: [_ _ _ _ TRUE _] -> w3086
      tunnel: w3083 -> [_ _ w3120 _ _ _]
      tunnel: w3077 -> [_ _ _ _ w3130 _]
      frame "init" {
        # "Initialize - All initialization work should take place in this message, since other loops can potentially enqueue messages that execute immediately after this one."
        n1769 = call-poly "Enqueue Message.vi"("error in (no error)"=w3094, "Message"="Monitor Main", "Message Queue"=w3091) -> ("error out"=w3095:errorcluster)  [unwired: 7 in, 1 out]
      }
      frame "Monitor Main" {
        n1770 = call "Main Monitor Loop.vi"("error in (no error)"=w3099, "main ref"=w3100) -> ("error out"=w3101:errorcluster)  [unwired: 9 in]
        n1771 = call "LOAD SELECTION MAIN CODE.vi"("error in (no error)"=w3099, "main ref"=w3100) -> ("error out"=w3097:errorcluster)  [unwired: 9 in]
        n1772 = call "Trip Log and Trip Monitor.vi"("error in (no error)"=w3099, "main ref"=w3100) -> ("error out"=w3096:errorcluster)  [unwired: 9 in]
        n1773 = Merge Errors(w3101, w3097, w3096) -> (w3098:errorcluster)
        n1774 = Unbundle By Name(w3100) -> ("Main Home Screen.EXIT"=w3105:refnum<vi>)
        n1775 = property class="Bool (strict)"(reference=w3105) -> (reference out=w3103:refnum<vi>, error out=w3104:errorcluster, "Value"=w3102:bool)  [unwired: 1 in]
        n1776 = case shown="False" w3102 {
          tunnel: [w3110 w3114] -> w3107
          tunnel: w3106 -> [w3109 w3113]
          tunnel: w3098 -> [w3108 w3112]
          frame True {
            n1777 = call-poly "Enqueue Message.vi"("error in (no error)"=w3108, "Message"="Confirm Quit", "Message Queue"=w3109) -> ("error out"=w3110:errorcluster)  [unwired: 7 in, 1 out]
          }
          frame False {
            n1778 = call-poly "Enqueue Message.vi"("error in (no error)"=w3112, "Message"="Monitor Main", "Message Queue"=w3113) -> ("error out"=w3114:errorcluster)  [unwired: 7 in, 1 out]
          }
        }
        n1779 = Close Reference(reference=w3103, error in (no error)=w3104) -> ()  [unwired: 1 out]
      }
      frame "Error" {
        # "#CodeRecommended - If you ever change the name of this \"Error\" message, you'll need to update the name in the Check Loop Error.vi as well."
        # "#CodeRecommended - Consider creating a system for logging errors in some way. These errors are for notification purposes only. Handling of specific errors should be performed in the message frames that generated the error."
        # "Error - Display an error dialog. This message is sent by the \"Error Handler\" VIs at the end of other loops in this application."
        n1780 = Variant To Data(error in=w3122, type=errorcluster {"status"=FALSE, "code"=0, "source"=""} ("error constant"), Variant=w3120) -> (data=w3118:errorcluster, error out=w3117:errorcluster)
        n1781 = call <vilib>:"Simple Error Handler.vi"("error in (no error)"=w3118) -> ()  [unwired: 4 in, 5 out]
        n1782 = Merge Errors(w3117) -> (w3116:errorcluster)
      }
      frame "Confirm Quit" {
        # "#CodeNeeded - If you want to provide an \"Are you sure\" dialog (or some other notification) before the application exits, place that code here. This message is typically sent from a Panel Close? event."
        # "Confirm Quit - Message that can confirm whether or not the user wants to exit the application."
        n1783 = call-poly "Enqueue Message.vi"("Priority Message? (F)"=TRUE, "error in (no error)"=w3129, "Message"="Exit", "Message Queue"=w3125) -> ("error out"=w3126:errorcluster)  [unwired: 6 in, 1 out]
        n1784 = Merge Errors(w3126) -> (w3127:errorcluster)
      }
      frame "Exit" {
        # "Stop the VI"
        # "Release the message queue reference"
        # "#CodeNeeded - Add any required cleanup code here. Note that if 'Exit' was called as a result of an error, an error dialog will be displayed. Add any custom error handling for an 'Exit' condition here as well."
        # "Exit - Exit the application."
        n1785 = call "Fire User Event - Stop.vi"("User Event - Stop"=w3130) -> ("error out"=w3132:errorcluster)  [unwired: 10 in]
        n1786 = Release Queue(queue=w3137, error in (no error)=w3131) -> (error out=w3134:errorcluster)  [unwired: 1 in, 2 out]
        n1787 = Merge Errors(w3132, w3134) -> (w3133:errorcluster)
      }
      frame Default {
        # "'Default' case only runs if there is a message that isn't defined in any of the other cases.  Output a programming error."
        n1788 = xnode "Error Ring"("parameter 0"=w3138) -> ("error out"=w3139:errorcluster)
      }
    }
    n1789 = node-c288() -> ()  [unwired: 1 in, 1 out]
    n1790 = call "LAB-IQ Error Handler - Message Handling Loop.vi"("error in (no error)"=w3080, "Message Queue"=w3082) -> ("dup error in"=w3081:errorcluster)  [unwired: 8 in, 1 out]
  }
  n1791 = timed-loop {
    shift-right: [w3158] -> _
    shift-left: w28 -> [w3159]
    tunnel: [w3152] -> _
    tunnel: w24 -> [w3150]
    tunnel: w18 -> [w3149]
    tunnel: w27 -> [w3148]
    timing: w13 -> [_]
    timing-out: [_] -> w12
    stop <- w3157 stop-if-true
    # "Report  Handling Loop"
    n1792 = node-c288() -> ()  [unwired: 1 in, 1 out]
    n1793 = call "Dequeue Message.vi"("error in (no error)"=w3149, "Message Queue"=w3150) -> ("error out"=w3156:errorcluster, "Message Data"=w3154:variant, "Message"=w3155:string, "dup Message Queue"=w3153:refnum<queue>)  [unwired: 6 in]
    n1794 = case "Message Cases" shown="\"Report Main\"" w3155 {
      selector: w3155 -> [_ _ _ _ _ w3206]
      tunnel: w3153 -> [w3162 w3174 _ w3193 w3205 _]
      tunnel: w3156 -> [w3165 w3172 w3190 w3197 w3199 _]
      tunnel: [w3166 w3175 w3184 w3195 w3201 w3207] -> w3151
      tunnel: w3159 -> [w3164 w3167 w3189 w3196 w3204 w3208]
      tunnel: [w3164 w3167 w3189 w3196 w3204 w3208] -> w3158
      tunnel: [_ _ _ _ TRUE _] -> w3157
      tunnel: w3154 -> [_ _ w3188 _ _ _]
      tunnel: w3148 -> [_ _ _ _ w3198 _]
      frame "init" {
        # "Initialize - All initialization work should take place in this message, since other loops can potentially enqueue messages that execute immediately after this one."
        n1795 = call-poly "Enqueue Message.vi"("error in (no error)"=w3165, "Message"="Report Main", "Message Queue"=w3162) -> ("error out"=w3166:errorcluster)  [unwired: 7 in, 1 out]
      }
      frame "Report Main" {
        n1796 = call "Main Data Log.vi"("error in (no error)"=w3172, "main ref"=w3167) -> ("error out"=w3168:errorcluster)  [unwired: 9 in]
        n1797 = Unbundle By Name(w3167) -> ("Main Home Screen.EXIT"=w3173:refnum<vi>)
        n1798 = property class="Bool (strict)"(reference=w3173) -> (reference out=w3170:refnum<vi>, error out=w3171:errorcluster, "Value"=w3169:bool)  [unwired: 1 in]
        n1799 = case shown="False" w3169 {
          tunnel: [w3178 w3182] -> w3175
          tunnel: w3174 -> [w3177 w3181]
          tunnel: w3168 -> [w3176 w3180]
          frame True {
            n1800 = call-poly "Enqueue Message.vi"("error in (no error)"=w3176, "Message"="Confirm Quit", "Message Queue"=w3177) -> ("error out"=w3178:errorcluster)  [unwired: 7 in, 1 out]
          }
          frame False {
            n1801 = call-poly "Enqueue Message.vi"("error in (no error)"=w3180, "Message"="Report Main", "Message Queue"=w3181) -> ("error out"=w3182:errorcluster)  [unwired: 7 in, 1 out]
          }
        }
        n1802 = Close Reference(reference=w3170, error in (no error)=w3171) -> ()  [unwired: 1 out]
      }
      frame "Error" {
        # "#CodeRecommended - If you ever change the name of this \"Error\" message, you'll need to update the name in the Check Loop Error.vi as well."
        # "#CodeRecommended - Consider creating a system for logging errors in some way. These errors are for notification purposes only. Handling of specific errors should be performed in the message frames that generated the error."
        # "Error - Display an error dialog. This message is sent by the \"Error Handler\" VIs at the end of other loops in this application."
        n1803 = Variant To Data(error in=w3190, type=errorcluster {"status"=FALSE, "code"=0, "source"=""} ("error constant"), Variant=w3188) -> (data=w3186:errorcluster, error out=w3185:errorcluster)
        n1804 = call <vilib>:"Simple Error Handler.vi"("error in (no error)"=w3186) -> ()  [unwired: 4 in, 5 out]
        n1805 = Merge Errors(w3185) -> (w3184:errorcluster)
      }
      frame "Confirm Quit" {
        # "#CodeNeeded - If you want to provide an \"Are you sure\" dialog (or some other notification) before the application exits, place that code here. This message is typically sent from a Panel Close? event."
        # "Confirm Quit - Message that can confirm whether or not the user wants to exit the application."
        n1806 = call-poly "Enqueue Message.vi"("Priority Message? (F)"=TRUE, "error in (no error)"=w3197, "Message"="Exit", "Message Queue"=w3193) -> ("error out"=w3194:errorcluster)  [unwired: 6 in, 1 out]
        n1807 = Merge Errors(w3194) -> (w3195:errorcluster)
      }
      frame "Exit" {
        # "Stop the VI"
        # "Release the message queue reference"
        # "#CodeNeeded - Add any required cleanup code here. Note that if 'Exit' was called as a result of an error, an error dialog will be displayed. Add any custom error handling for an 'Exit' condition here as well."
        # "Exit - Exit the application."
        n1808 = call "Fire User Event - Stop.vi"("User Event - Stop"=w3198) -> ("error out"=w3200:errorcluster)  [unwired: 10 in]
        n1809 = Release Queue(queue=w3205, error in (no error)=w3199) -> (error out=w3202:errorcluster)  [unwired: 1 in, 2 out]
        n1810 = Merge Errors(w3200, w3202) -> (w3201:errorcluster)
      }
      frame Default {
        # "'Default' case only runs if there is a message that isn't defined in any of the other cases.  Output a programming error."
        n1811 = xnode "Error Ring"("parameter 0"=w3206) -> ("error out"=w3207:errorcluster)
      }
    }
    n1812 = node-c288() -> ()  [unwired: 1 in, 1 out]
    n1813 = call "LAB-IQ Error Handler - Message Handling Loop.vi"("error in (no error)"=w3151, "Message Queue"=w3153) -> ("dup error in"=w3152:errorcluster)  [unwired: 8 in, 1 out]
  }
  n1814 = Unregister For Events(event registration refnum=w62, error in=w60) -> (error out=w63:errorcluster)
  n1815 = node-c288(w4) -> ()  [unwired: 1 out]
  n1816 = node-c288(w6) -> ()  [unwired: 1 out]
  n1817 = node-c288(w8) -> ()  [unwired: 1 out]
  n1818 = node-c288(w10) -> ()  [unwired: 1 out]
  n1819 = node-c288(w12) -> ()  [unwired: 1 out]
  n1820 = node-c288(w2) -> ()  [unwired: 1 out]
  n1821 = Merge Errors(w63, w66, w38, w35, w33, w15) -> (w64:errorcluster)
  n1822 = call "Destroy User Event - Stop.vi"("error in (no error)"=w64, "User Event - Stop"=w27) -> ("error out"=w61:errorcluster)  [unwired: 9 in]
  n1823 = disable-structure shown="RUN_TIME_ENGINE==True" {
    disable-tunnel: w61 -> [_ _]
    frame condition #0 (active) {
    }
    frame condition #1 {
      # "Call Quit LabVIEW if running as a built application."
      n1824 = Quit LabVIEW() -> ()  [unwired: 1 in]
    }
  }
